vi "main4Ch v2.0.0 reprocessing.vi"() -> ()   [LabVIEW 2024]
doc: "Main VI for FLS imaging system."
uses:
  <userlib>/_OpenG.lib/file/file.llb/openg_file.lvlib
  <vilib>/event_ctls.llb/usereventprio.ctl
  <instrlib>/niScope/Acquire/Fetch/niScope Multi Fetch Binary 16.vi
  <instrlib>/niScope/Controls/niScope trigger source.ctl
  <userlib>/_OpenG.lib/time/time.llb/openg_time.lvlib
  LaguerreDeconLib/DeconEngineClass/LaguerreDeconEngineClass.lvclass
  SubVI/GlobalVariables.vi
  SubVI/LabJack/LJ Pin Setting.ctl
  <vilib>/Utility/error.llb/DialogType.ctl
  <vilib>/Analysis/NI_AALBase.lvlib
  <vilib>/Utility/miscctls.llb/LVMinMaxIncTypeDef.ctl
  <vilib>/Analysis/baseanly.llb/Mean (DBL).vi
  <vilib>/Utility/miscctls.llb/LVPointTypeDef.ctl
  SubVI/APD/APDClass.lvclass
  ConfigFiles/AimingBeamVideoConfig.ctl
  <vilib>/addons/control/pid/NI_PID_pid.lvlib
  <vilib>/addons/control/pid/pid.llb/PID (DBL).vi
  C:/Users/MarcuLab/Documents/GitHub/NetDeconForLV/Source/DotNETAssembly/output/build/LaguerreDeConNative.dll
  MarcuLab/Documents/GitHub/NetDeconForLV/Source/DotNETAssembly/output/build/LaguerreDeConNative.dll
  <vilib>/Instr/_visa.llb/VISA Configure Serial Port (Instr).vi
  <vilib>/Python/Open Anaconda Python Session.vi
  SubVI/DigitizerConfiguration/FLImDAQ.ctl
panel:
  out "error out":errorcluster
  in  "488nm Power":u16(ring)=32 items=["3.30mW"=60, "2.35mW"=50, "2.00mW"=47, "1.75mW"=44, "1.48mW"=41, "1.16mW"=38, "0.87mW"=35, "0.57mW"=32, "0.28mW"=29]
  out "Decon Loop timing (ms)":dbl
  out "Ch3 Lifetime (ns)":dbl caption="Lifetime (ns)"
  out "Ch2 Lifetime (ns)":dbl caption="Lifetime (ns)"
  out "Ch1 Lifetime (ns)":dbl caption="Lifetime (ns)"
  out "Cancer Prob":dbl
  in  "Overlay selection":u16(ring) items=["Gain", "Lifetime", "CancerProbability"]
  out "Record Backlog 2":i32
  in  "Auto gain ch4":bool=TRUE caption="Auto gain ch3"
  in  "V 4":dbl caption="Gain 3" min=0.0 max=4.67 step=0.1
  out "Gain4":dbl
  out "IntR4":dbl format="%#_2g"
  out "SNR4":dbl format="%#_3g"
  out "Channel 4":dbl[][](graph) caption="Channel 3"
  out "RunStartTime":u32
  out "Dig1 Temp":dbl
  out "Dig2 Temp":dbl
  out "Visualization PC video source":T1
  in  "V target(1.0)":dbl=1.0 caption="V target(1.5)" min=0.3 max=1.5 step=0.1 format="%#_4g"
  out "SNR3":dbl format="%#_3g"
  out "SNR2":dbl format="%#_3g"
  out "SNR1":dbl format="%#_3g"
  in  "Show BG removed?":bool=TRUE
  out "IntR3":dbl format="%#_2g"
  out "IntR2":dbl format="%#_2g"
  out "IntR1":dbl format="%#_2g"
  in  "Video Display":bool
  out "Gain3":dbl
  out "Gain2":dbl
  out "Gain1":dbl
  in  "Skip Data Save?":bool
  out "Aq Loop?":bool
  out "ML?":bool
  out "aquisition loop Error Out":errorcluster
  out "Laser f (Hz)":dbl
  out "Record Backlog":i32
  out "Fetch Record #":i32
  out "Sync Success?":bool
  out "Disclamer":picture
  out "Calibration #":i8
  out "BG #":i8
  in  "TCP Connect":bool
  out "Help":string
  in  "355nm Laser toggle":bool caption="355nm 460Hz"
  in  "Cali&iRF alignment":bool
  in  "Background":bool
  in  "Aiming beam toggle":bool caption="488nm 0Hz"
  in  "Auto gain ch3":bool=TRUE
  in  "Auto gain ch2":bool=TRUE
  in  "Auto gain ch1":bool=TRUE
  out "Run #":i8
  in  "StopButton":bool caption="Stop"
  out "Aquisition Status:":bool
  in  "StartButton":bool caption="Start"
  in  "V 3":dbl caption="Gain 3" min=0.0 max=4.65 step=0.1
  in  "V 2":dbl caption="Gain 2" min=0.0 max=4.59 step=0.1
  in  "V 1":dbl caption="Gain 1" min=0.0 max=4.63 step=0.1 format="%#_4g"
  in  "Video Source":enum32{"Camera", "FrameGrabber"}(radio)
  out "Case #":string
  out "System Hardware Connection Status":T2
  out "Channel 3":dbl[][](graph)
  out "Channel 2":dbl[][](graph)
  out "Channel 1":dbl[][](graph)
  in  "Tab Control":T3(tab)
  out "display loop timing(ms)":u32
  out "Aquisition loop timing(ms)":u32 format="%.2f"
  out "DisplayLoop":i32
  out "PID loop":i32 caption="processing loop"
  out "PID loop timing(ms)":u32 caption="processing loop timing(ms)"
  out "Communication loop(ms)":u32
  out "laser EM lamp V":dbl format="%0.6f"
  out "Auisition Loop idx":i32
  out "LJ process (ms)":u32
  out "LJ time(ms)":u32[](array[numeric])
  out "output variable":i32
  out ".NetInitialized?":bool
  out "BG Graph":dbl[][](graph)
  out "Lifetime (ns)":cluster{dbl, dbl, dbl}(graph)
  out "DeCon Speed(ms)":dbl(graph)
  out "iRF Graph":dbl[][](graph)
  in  "Show BG":bool
  out "iRF length":i32
  out "BG length":i32
  out "data length":i32
  out "WarmupTime(ms)":u32
  out "BGAll":dbl[][](array[numeric])
  out "DeConOut":dbl[](array[numeric])
  in  "Ch1GainLim":dbl=350.0 format="%#_13g"
  in  "Ch2&3GainLim":dbl=1750.0 format="%#_13g"
  out "LJ Pinout":T4={"Ch1 Bias"="DAC0", "Ch2 Bias"="DAC1", "Ch3 Bias"="DAC2", "355 PWM"="FIO0", "AimingBeam PWM"="FIO2", "Laser Ready"="FIO3", "Interlock"="FIO1", "Laser Start/Stop"="FIO1", "Red LED"="FIO1", "Green LED"="DIO3", "Foot Pedal"="DIO15"}
  out "FLImDAQ":T5={"Digitizer 1"="", "Digitizer 2"="", "Channel"=enum."Channel 0", "trigger source"="VAL_EXTERNAL", "trigger level"=0.5, "trigger delay"=1.35e-07, "min sample rate"=12500000000.0, "min record length"=2500, "vertical range"=1.0, "vertical offset"=-0.25, "Waveform to Avg"=2000} caption="FLIm DAQ Configuration" {"trigger delay" format="%^#.4e"; "trigger level" min=0.0 max=3.5 step=0.5 format="%.2f"; "vertical offset" format="%.4f"; "vertical range" format="%.2f"; "min sample rate" format="%#.2p"}
  in  "Sys Reconfig":bool
  out "data out(communcation loop)":string
  out "PID loop error out":errorcluster caption="processing Error Out"
  out "decon error out":errorcluster
  out "Laser Rep Rate":dbl
  out "V4 Size":i32 caption="V3 Size"
  in  "Data Class":enum16{"Data", "BG", "Cali"}(ring)=enum."BG"
  out "V1 Size":i32
  out "V2 Size":i32
  out "V3 Size":i32
  out "data Size":i32[](array[numeric])
  out "State log":string
  out "SysConfigCluster":T7
  in  "Ch4 PID gains":T8={"proportional gain (Kc)"=30.0, "integral time (Ti, min)"=0.0003, "derivative time (Td, min)"=1e-05}
  in  "Ch3 PID gains":T8={"proportional gain (Kc)"=30.0, "integral time (Ti, min)"=0.0003, "derivative time (Td, min)"=1e-05}
  in  "Ch2 PID gains":T8={"proportional gain (Kc)"=30.0, "integral time (Ti, min)"=0.0003, "derivative time (Td, min)"=1e-05}
  in  "Ch1 PID gains":T8={"proportional gain (Kc)"=30.0, "integral time (Ti, min)"=0.0003, "derivative time (Td, min)"=1e-05}
  in  "Brain model path":path=path "C:/Users/MarcuLab/Desktop/V6 APD LV/V6 APD LV/ClassifierFile/Brain_Agnostic_Model.pkl"
  in  "module path":path=path "C:/Users/MarcuLab/Documents/GitHub/NetDeconForLV/Classifier/ClassifierModule.py"
  in  "HN model path":path=path "C:/Users/MarcuLab/Desktop/V6 APD LV/V6 APD LV/ClassifierFile/xgb_model.pkl"
  in  "Env name":string="HNClassifier"
  in  "Python version":string="3.10"
  out "Python session":refnum<k35>
  out "OverlaySelection":T9(ring)=enum."HN Classifier"
  in  "CancerThreshold":dbl=0.15
  in  "Quit":bool
  in  "Radio Buttons":T10(radio)=enum."Ch2" caption="DeCon Chan"
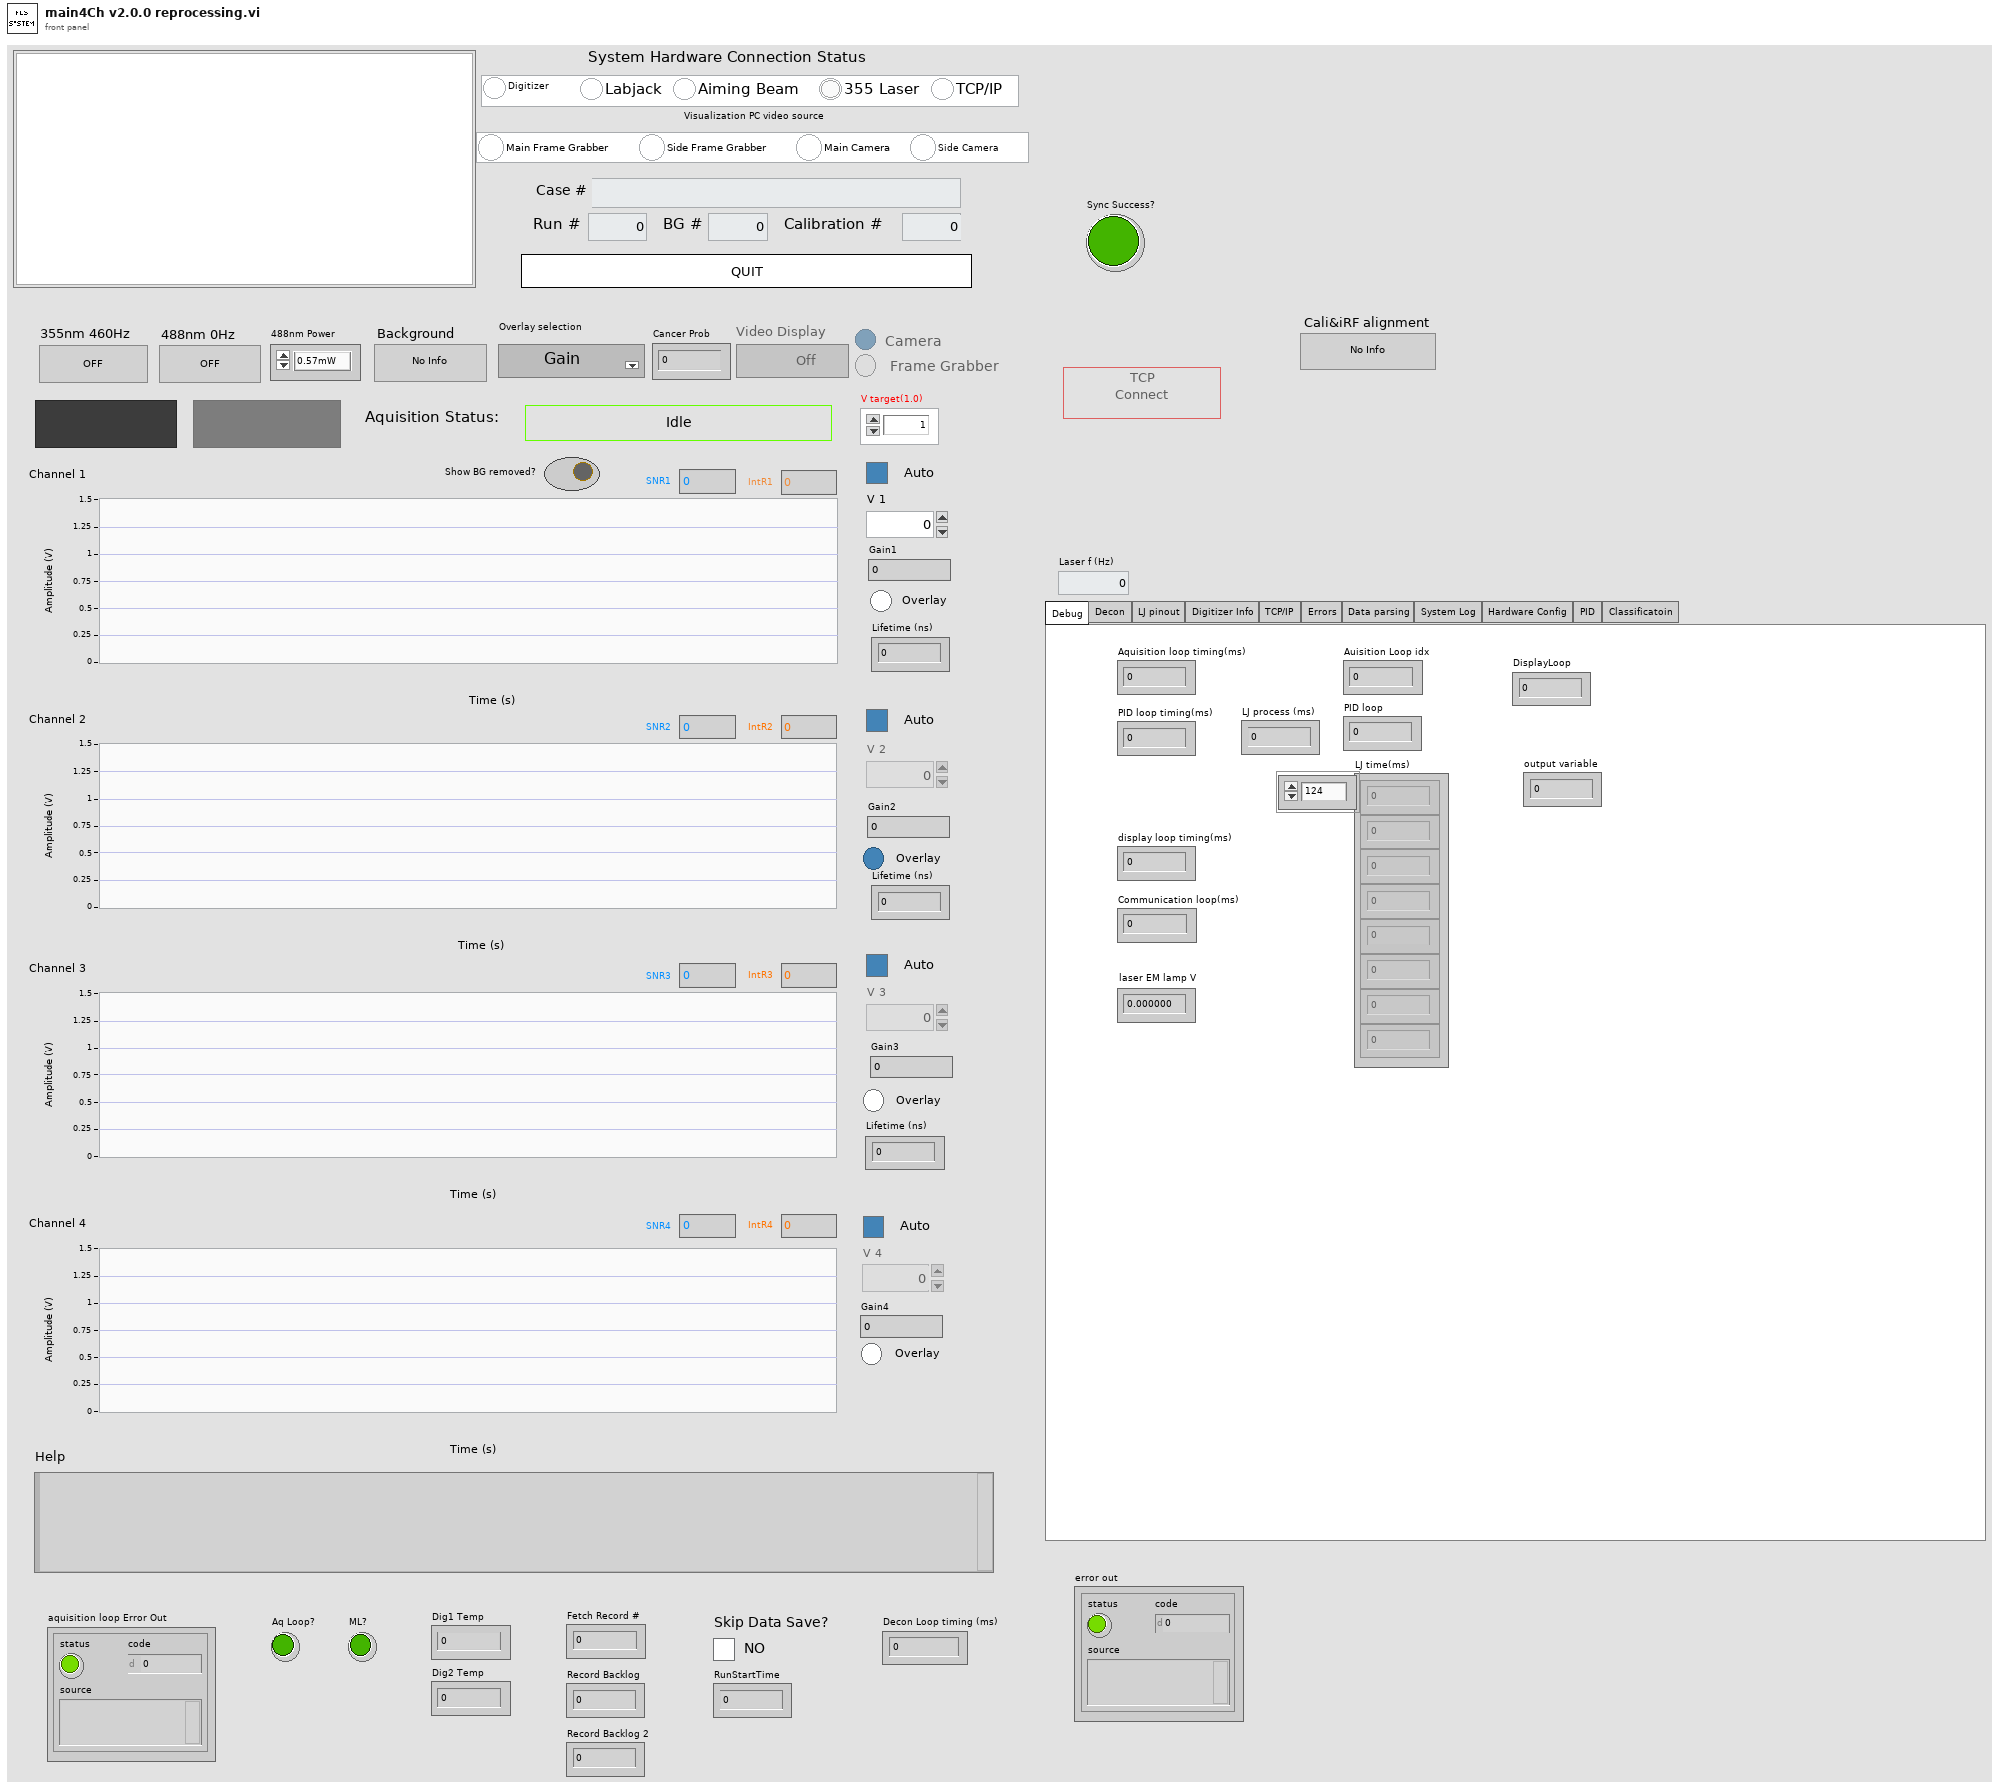
[diagram p1: front panel]
types:
  T1 = cluster{"Main Frame Grabber":bool, "Side Frame Grabber":bool, "Main Camera":bool, "Side Camera":bool}
  T2 = cluster{"Digitizer":bool, "Labjack":bool, "Aiming Beam":bool, "355 Laser":bool, "TCP/IP":bool}
  T3 = enum32{"Debug", "Decon", "LJ pinout", "Digitizer Info", "TCP/IP", "Errors", "Data parsing", "System Log", "Hardware Config", "PID", "Classificatoin"}
  T4 = typedef "LJ Pin Setting.ctl" = cluster{"Ch1 Bias":string, "Ch2 Bias":string, "Ch3 Bias":string, "355 PWM":string, "AimingBeam PWM":string, "Laser Ready":string, "Interlock":string, "Laser Start/Stop":string, "Red LED":string, "Green LED":string, "Foot Pedal":string}
  T5 = typedef "FLImDAQ.ctl" = cluster{"Digitizer 1":refnum<k15>, "Digitizer 2":refnum<k15>, "Channel":enum16{"Channel 0", "Channel 1", "Channel 0&1"}, "trigger source":T6, "trigger level":dbl, "trigger delay":dbl, "min sample rate":dbl, "min record length":i32, "vertical range":dbl, "vertical offset":dbl, "Waveform to Avg":i16}
  T6 = typedef "niScope trigger source.ctl" = string
  T7 = cluster{"Ch1Enable?":bool, "Ch2Enable?":bool, "Ch3Enable?":bool, "Ch1AutoGain?":bool, "Ch2AutoGain?":bool, "Ch3AutoGain?":bool, "AimingBeamEnable?":bool}
  T8 = cluster{"proportional gain (Kc)":dbl, "integral time (Ti, min)":dbl, "derivative time (Td, min)":dbl}
  T9 = enum16{"Gain", "HN Classifier", "Brain Classifier", "Window Close"}
  T10 = enum32{"No Selection", "Ch1", "Ch2", "Ch3", "Ch4"}
  T11 = cluster{"remote start event":refnum<user-event>, "remote stop  event":refnum<user-event>}
  T12 = enum8{"Enabled", "Disabled", "Disabled and Grayed Out"}
  T13 = enum16{"open", "replace", "create", "open or create", "replace or create", "replace or create with confirmation"}
  T14 = cluster{"CH1":dbl[][], "CH2":dbl[][], "CH3":dbl[][], "CH4":dbl[][], "Gain cluster":cluster{"V1":dbl, "V2":dbl, "V3":dbl, "V4":dbl}}
  T15 = cluster{"idx":i32, "CH1&2":dbl[][], "CH3&4":dbl[][], "V cluster":cluster{"V1":dbl, "V2":dbl, "V3":dbl, "V4":dbl}}
  T16 = enum16{"open", "open or create", "create or replace", "create", "open (read-only)"}
  T17 = cluster{"Ch1 iRF":dbl[], "Ch2 iRF":dbl[], "Ch3 iRF":dbl[], "Ch4 iRF":dbl[]}
  T18 = enum32{"Invalid", "Standard", "Closed", "Hidden", "Minimized", "Maximized"}
  T19 = enum32{"invalid app kind", "Development System", "Run Time System", "Student Edition", "Embedded LabVIEW", "Evaluation", "Custom"}
  T20 = typedef "usereventprio.ctl" = enum32{"high priority", "normal priority"}
  T21 = enum32{"Bad", "Idle", "Run top level", "Running"}
  T22 = enum16{"Standard", "Buffered", "CRLF", "Immediate"}
  T23 = typedef "AimingBeamVideoConfig.ctl" = cluster{"DeCon Channel":enum16{"1", "2", "3"}, "Scale Bar":bool, "Scale Low":dbl, "Scale High":dbl, "ANSI":dbl, "Radius":dbl, "3D?":bool, "Firefly?":bool, "Pentero?":bool}
  T24 = cluster{"Core":cluster{"Current VI Reference":refnum<vi>, "Close Panel on Exit?":bool}, "SysConfigCluster":cluster{"Ch1Enable?":bool, "Ch2Enable?":bool, "Ch3Enable?":bool, "Ch1AutoGain?":bool, "Ch2AutoGain?":bool, "Ch3AutoGain?":bool, "AimingBeamEnable?":bool}, "System Status":cluster{"Digitizer":bool, "Labjack":bool, "Aiming Beam":bool, "355 Laser":bool, "TCP/IP":bool}, "IDs":cluster{"RunID":i8, "BG ID":i8, "Cali ID":i8}, "CaseID":string, "DefaultPath":path, "Pathes":cluster{"DataPath":path, "BG Path":path, "iRFPath":path, "CaliPath":path}, "FLImDAQ":cluster{"resource name":refnum<k15>, "resource name 2":refnum<k15>, "Channel":enum16{"Channel 0", "Channel 1", "Channel 0&1"}, "trigger source":T6, "trigger level":dbl, "trigger delay":dbl, "min sample rate":dbl, "min record length":i32, "vertical range":dbl, "vertical offset":dbl, "Waveform to Avg":i32}, "SysRunning?":bool, "AB Cluster":cluster{"Aiming Beam COM Port":refnum<visa-resource-name>, "Min Current":dbl, "Max Current":dbl, "Default Current":dbl, "Freq":i32}, "LJ Pinout":T4, "355 PWM setting":cluster{"DIO_EF_CLOCK1_DIVISOR":i16, "DIO_EF_CLOCK1_ROLL_VALUE":i32, "DIO#_EF_INDEX":i16, "DIO#_EF_OPTIONS":i16, "DIO#_EF_CONFIG_A":i32}, "AB PWM setting":cluster{"DIO_EF_CLOCK1_DIVISOR":i16, "DIO_EF_CLOCK1_ROLL_VALUE":i32, "DIO#_EF_INDEX":i16, "DIO#_EF_OPTIONS":i16, "DIO#_EF_CONFIG_A":i32}, "Last Trigger":u32, "niTClk sessions":refnum<k20>[], "Laser start tic":u32, "TCP attempt count":i32, "Ch1Data":dbl[][], "Ch2Data":dbl[][], "Ch3Data":dbl[][], "Ch4Data":dbl[][], "V1":dbl[], "V2":dbl[], "V3":dbl[], "V4":dbl[], "SlowTimer":u32, "FastTimer":u32, "listener ID":refnum<k5>, "TempPath":path, "CaliPath":path, "LED vi reference":refnum<vi>, "Aquisition Timer":u32, "APDSerialNum":cluster{"Ch1APDSerial#":string, "Ch2APDSerial#":string, "Ch3APDSerial#":string, "Ch4APDSerial#":string}, "VideoConfig":T23, "LED vi ref open?":bool, "video source":cluster{"Main Frame Grabber":bool, "Side Frame Grabber":bool, "Main Camera":bool, "Side Camera":bool}, "bothVidSourceAvail":bool, "OverlaySelection":u16}
  T25 = typedef "LVCursorListTypeDef.ctl" = cluster{"Name":string, "Color":u32, "Style":u8, "Point Style":u8, "Name Visible":bool, "Allow Drag":bool, "Cursor Mode":u32, "Plot":i32, "Index":i32, "Position":cluster{"X":dbl, "Y":dbl}, "X Scale":u32, "Y Scale":u32, "Watch Plots":i32[], "Watch All Plots":bool, "Plot Area":i32, "Label Offset":cluster{"X":dbl, "Y":dbl}}[]
  T26 = cluster{"Name":string, "Color":u32, "Style":u8, "Point Style":u8, "Name Visible":bool, "Allow Drag":bool, "Cursor Mode":u32, "Plot":i32, "Index":i32, "Position":cluster{"X":dbl, "Y":dbl}, "X Scale":u32, "Y Scale":u32, "Watch Plots":i32[], "Watch All Plots":bool, "Plot Area":i32, "Label Offset":cluster{"X":dbl, "Y":dbl}}
  T27 = cluster{"Ch1APDSerial#":string, "Ch2APDSerial#":string, "Ch3APDSerial#":string, "Ch4APDSerial#":string}
  T28 = cluster{"DataPath":path, "BG Path":path, "iRFPath":path, "CaliPath":path}
  T29 = cluster{"DIO_EF_CLOCK1_DIVISOR":i16, "DIO_EF_CLOCK1_ROLL_VALUE":i32, "DIO#_EF_INDEX":i16, "DIO#_EF_OPTIONS":i16, "DIO#_EF_CONFIG_A":i32}
  T30 = cluster{"Aiming Beam COM Port":refnum<visa-resource-name>, "Min Current":dbl, "Max Current":dbl, "Default Current":dbl, "Freq":i32}
  T31 = cluster{"resource name":refnum<k15>, "resource name 2":refnum<k15>, "Channel":enum16{"Channel 0", "Channel 1", "Channel 0&1"}, "trigger source":T6, "trigger level":dbl, "trigger delay":dbl, "min sample rate":dbl, "min record length":i32, "vertical range":dbl, "vertical offset":dbl, "Waveform to Avg":i32}
  T32 = cluster{"Current VI Reference":refnum<vi>, "Close Panel on Exit?":bool}
  T33 = cluster{"Channel 1":dbl[], "Channel 2":dbl[], "Channel 3":dbl[]}
  T34 = cluster{"Ch1 WF":dbl[], "Ch2 WF":dbl[], "Ch3 WF":dbl[], "Ch4 WF":dbl[], "V1":dbl, "V2":dbl, "V3":dbl, "V4":dbl}
  T35 = typedef "iRFData.ctl" = cluster{"dt":dbl, "NumOfWFs":i32, "WFLength":i32, "iRFCtrlV":dbl[], "iRFWFsAvg":dbl[][], "iRFRaw":dbl[][]}
  T36 = cluster{"Ch1 iRF":dbl[], "Ch2 iRF":dbl[], "Ch3 iRF":dbl[]}
  T37 = cluster{"mean":dbl, "mean":dbl, "mean":dbl, "mean":dbl}
  T38 = cluster{"V1":dbl, "V2":dbl, "V3":dbl, "V4":dbl}[]
  T39 = cluster{"DataPath":path, "CaseID":string, "RunID":i16, "Ch1Data":dbl[][], "Ch2Data":dbl[][], "Ch3Data":dbl[][], "Ch4Data":dbl[][], "V1":dbl[], "V2":dbl[], "V3":dbl[], "V4":dbl[], "LaserRepRate":u16, "WFAverage":i16, "RunStartTime":u64}
  T40 = typedef "DialogType.ctl" = u16
  T41 = typedef "APD.ctl" = cluster{"gainV":dbl[], "gain":dbl[], "irfV":dbl[], "irfTNorm":dbl[][]}
  T42 = cluster{"Ch1APDSerial#":string, "Ch2APDSerial#":string, "Ch3APDSerial#":string}
  T43 = typedef "LJ PWM Setting.ctl" = cluster{"DIO_EF_CLOCK1_DIVISOR":i16, "DIO_EF_CLOCK1_ROLL_VALUE":i32, "DIO#_EF_INDEX":i16, "DIO#_EF_OPTIONS":i16, "DIO#_EF_CONFIG_A":i32}
  T44 = typedef "AimingBeam.ctl" = cluster{"Aiming Beam COM Port":refnum<visa-resource-name>, "Min Current":dbl, "Max Current":dbl, "Default Current":dbl, "Frequency(Hz)":u32}
  T45 = cluster{"DC1":i32, "DC2":i32, "BG1":i32, "BG2":i32}
  T46 = typedef "LVMinMaxIncTypeDef.ctl" = cluster{"Minimum":dbl, "Maximum":dbl, "Increment":dbl}
  T47 = typedef "LVBoundsTypeDef.ctl" = cluster{"Width":u32, "Height":u32}
  T48 = typedef "imagedata.ctl" = cluster{"image type":i32, "image depth":i32, "image":u8[], "mask":u8[], "colors":u32[], "Rectangle":cluster{"left":i16, "top":i16, "right":i16, "bottom":i16}}
  T49 = enum16{"Left Button", "Center Button", "Right Button", "Window Close"}
  T50 = cluster{"DC Idx1":i32, "DC Idx2":i32, "BG Idx1":i32, "BG Idx2":i32}
  T51 = cluster{dbl[][], dbl[][], dbl[][], dbl[][], "V cluster":cluster{"V1":dbl, "V2":dbl, "V3":dbl, "V4":dbl}}
  T52 = cluster{"actualSamples":i32, "absoluteInitialX":dbl, "relativeInitialX":dbl, "xIncrement":dbl, "offset":dbl, "gain":dbl, "reserved1":dbl, "reserved2":dbl}[]
  T53 = cluster{"V1 out":dbl, "V2 out":dbl, "V3 out":dbl, "V3 out":dbl}
  T54 = cluster{i32, dbl[][], dbl[][], cluster{"V1 out":dbl, "V2 out":dbl, "V3 out":dbl, "V3 out":dbl}}
  T55 = typedef "LVPointTypeDef.ctl" = cluster{"Horizontal":i16, "Vertical":i16}
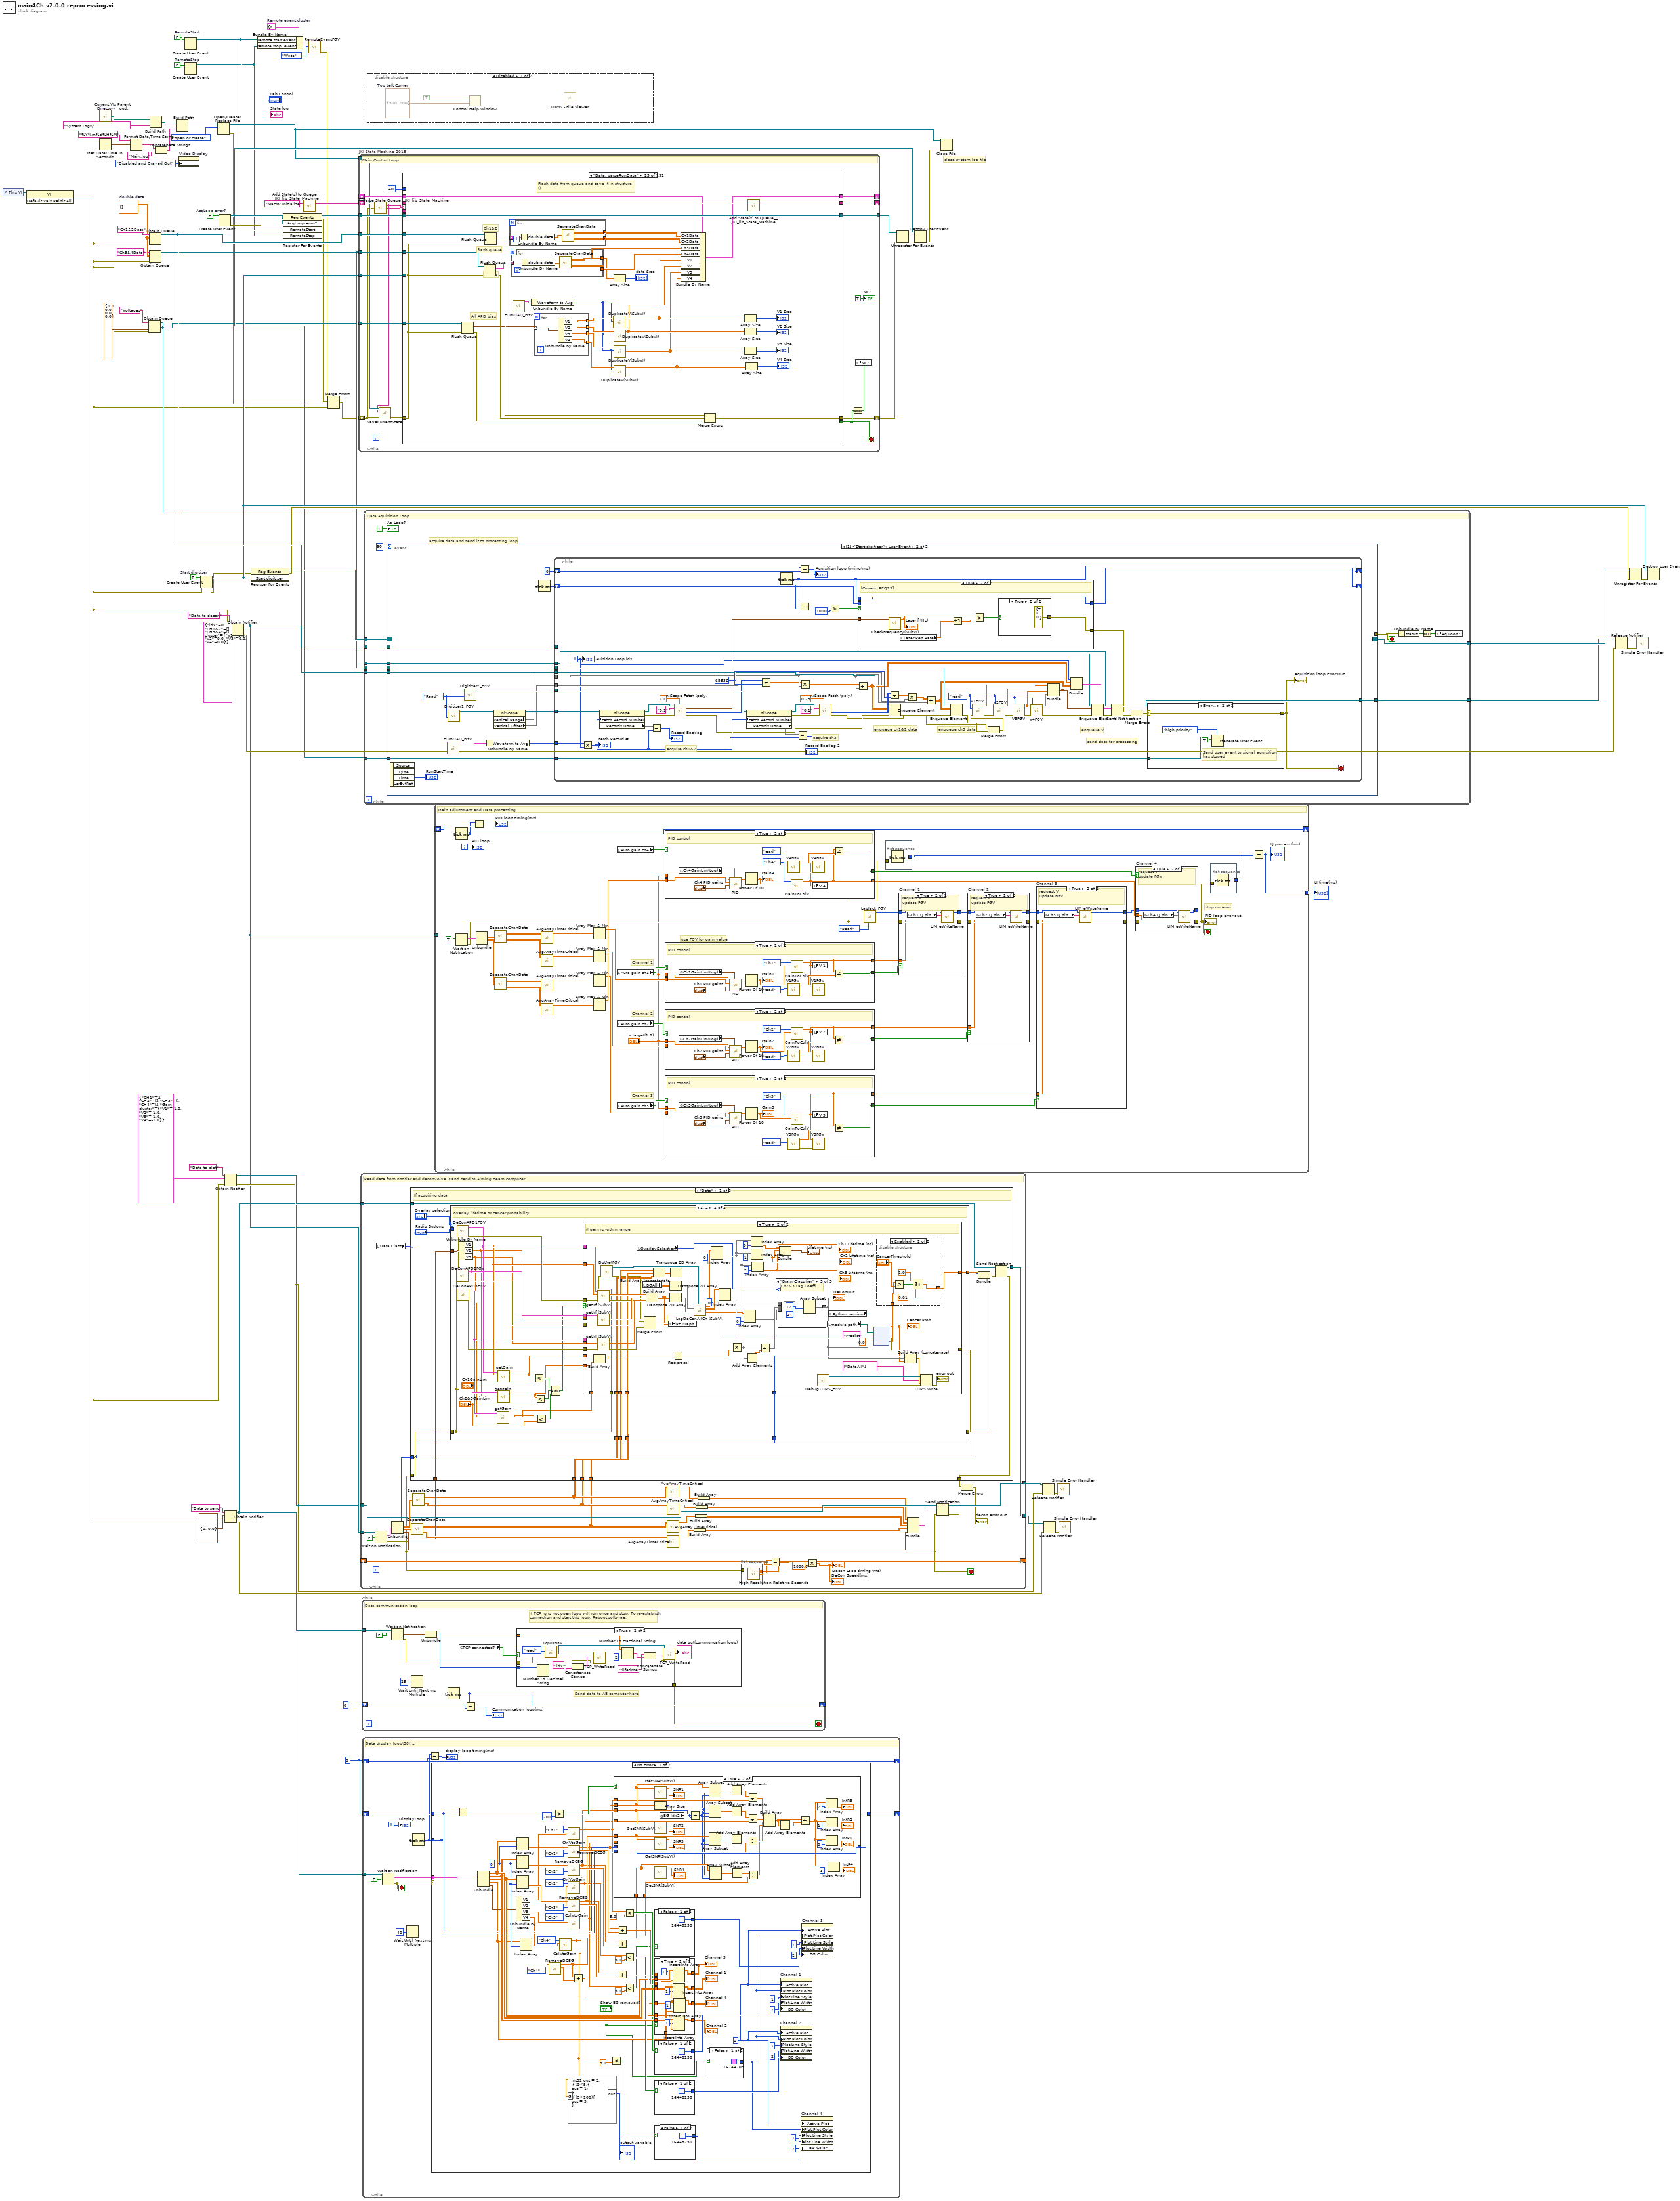
[diagram p0: block diagram]
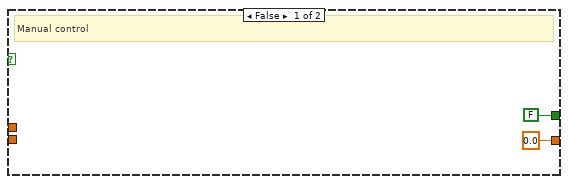
[diagram p6: hidden frame]
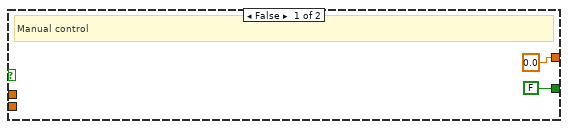
[diagram p7: hidden frame]
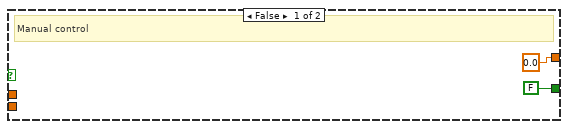
[diagram p8: hidden frame]
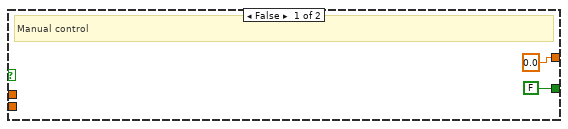
[diagram p9: hidden frame]
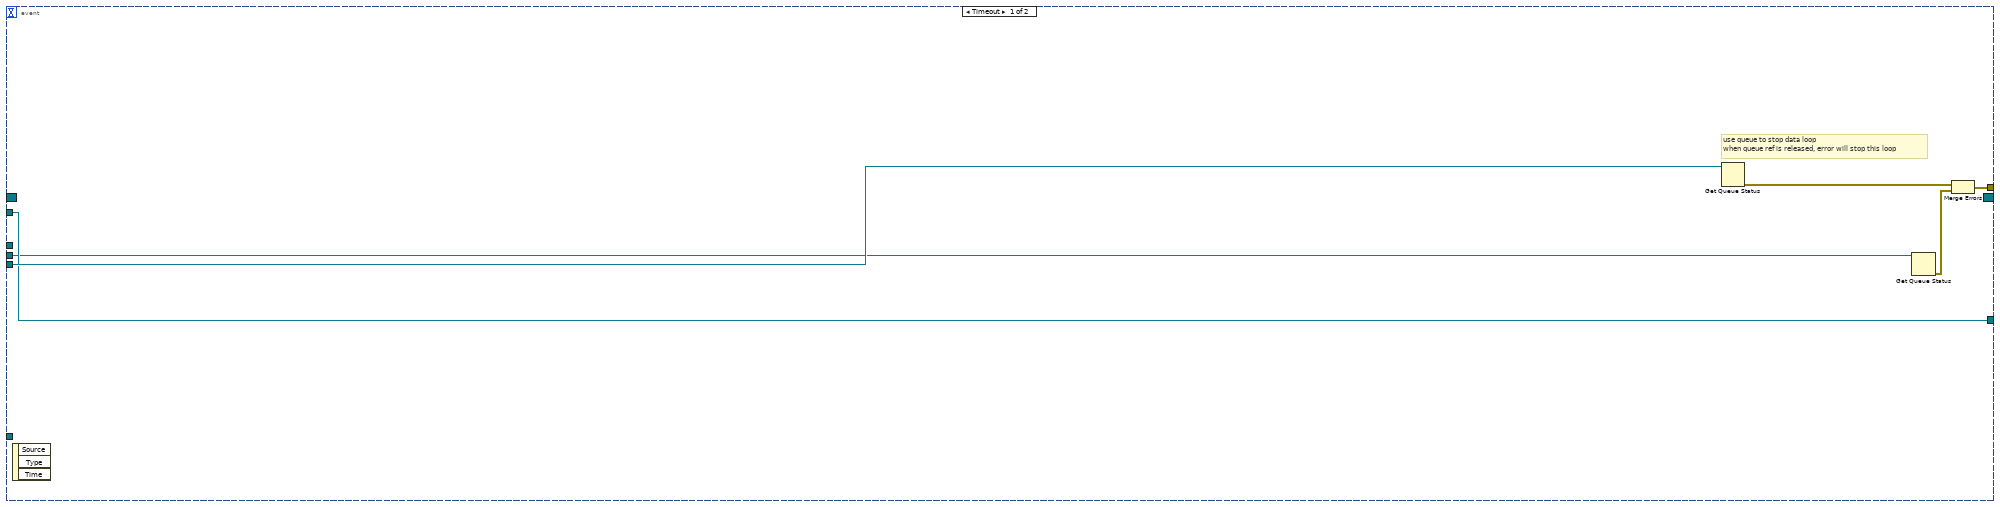
[diagram p10: hidden frame]
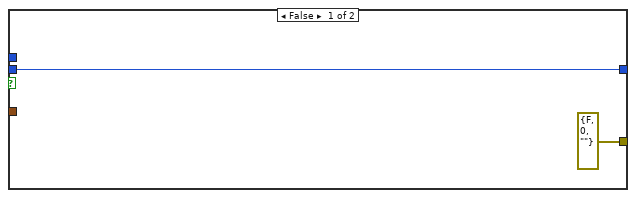
[diagram p11: hidden frame]
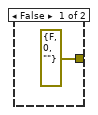
[diagram p12: hidden frame]
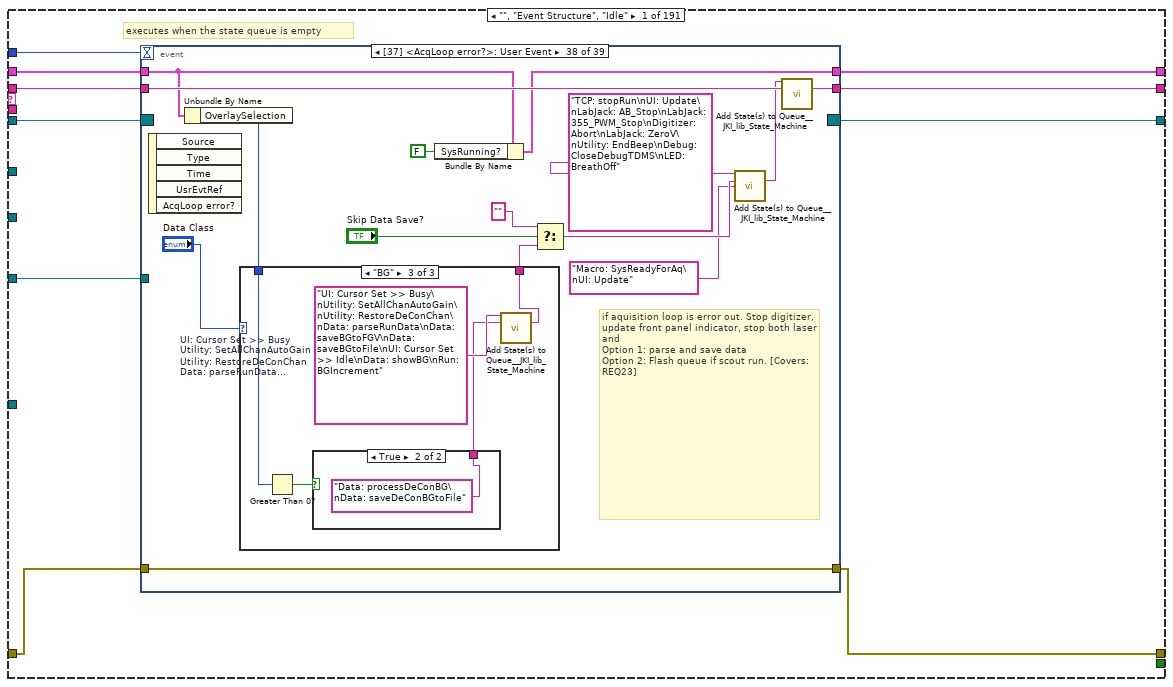
[diagram p14: hidden frame]
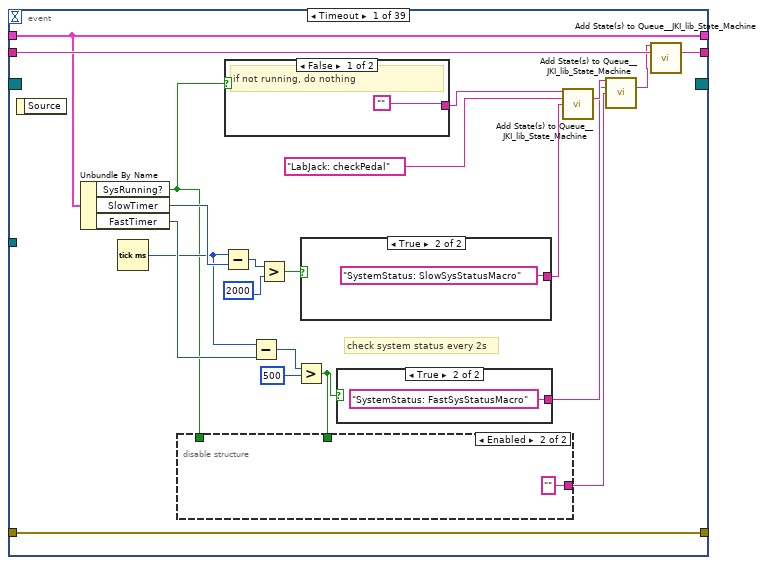
[diagram p15: hidden frame]
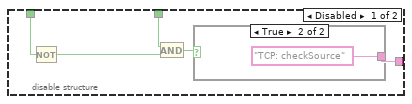
[diagram p16: hidden frame]
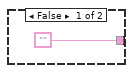
[diagram p17: hidden frame]
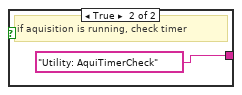
[diagram p18: hidden frame]
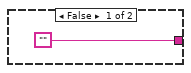
[diagram p19: hidden frame]
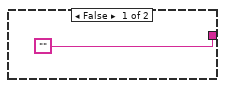
[diagram p20: hidden frame]
diagram:
  w8 = T11 {"remote start event"=refnum, "remote stop  event"=refnum}  # Remote event cluster
  w11 = FALSE  # RemoteStop
  w12 = FALSE  # RemoteStart
  w15 = u32 0 ("millisecond timer value")
  w54 = FALSE  # AcqLoop error?
  w64 = TRUE  # Start digitizer
  w67 = dbl[][] []  # double data
  # "close system log file"
  n1 = control-ref of="This VI"() -> (w69:refnum<vi>)
  n2 = invoke on="Invoke Node" class="VI" method="Default Vals.Reinit All"(reference=w69) -> (error out=w23:errorcluster)  [unwired: 2 in, 2 out]
  n3 = call <userlib>:"Current VIs Parent Directory__ogtk.vi"() -> ("Parent Directory (+ Relative)"=w34:path)  [unwired: 5 in]
  n4 = Get Date/Time In Seconds() -> (seconds since 1Jan1904=w32:timestamp)
  n5 = Format Date/Time String(time format string (%c)="%Y%m%d%H%M", seconds (now)=w32) -> (date/time string=w29:string)  [unwired: 1 in]
  n6 = Obtain Queue(name (unnamed)="Voltages", element data type=cluster{"V1":dbl, "V2":dbl, "V3":dbl, "V4":dbl} {"V1"=0.0, "V2"=0.0, "V3"=0.0, "V4"=0.0}, error in (no error)=w23) -> (queue out=w35:refnum<queue>)  [unwired: 2 in, 2 out]
  n7 = Obtain Queue(name (unnamed)="Ch3&4Data", element data type=w67, error in (no error)=w23) -> (queue out=w48:refnum<queue>)  [unwired: 2 in, 2 out]
  n8 = Obtain Queue(name (unnamed)="Ch1&2Data", element data type=w67, error in (no error)=w23) -> (queue out=w65:refnum<queue>)  [unwired: 2 in, 2 out]
  n9 = Build Path(base path=w34, name or relative path="System Log\\") -> (appended path=w25:path)
  n10 = Concatenate Strings(w29, "Main.log" ("string")) -> (w27:string)
  n11 = Build Path(base path=w25, name or relative path=w27) -> (appended path=w30:path)
  n12 = property on="Video Display" class="Bool (strict)"("DisabledEnum"=T12."Disabled and Grayed Out" ("Disabled")) -> ()  [unwired: 2 in, 2 out]
  n13 = Create User Event(user event datatype=w12) -> (user event=w10:refnum<user-event>)  [unwired: 1 in, 1 out]
  n14 = Create User Event(user event datatype=w11) -> (user event=w9:refnum<user-event>)  [unwired: 1 in, 1 out]
  n15 = Create User Event(user event datatype=w64, error in=w23) -> (user event=w53:refnum<user-event>, error out=w40:errorcluster)
  n16 = Open/Create/Replace File(file path (use dialog)=w30, operation (0:open)=T13."open or create") -> (refnum out=w21:refnum<file>, error out=w22:errorcluster)  [unwired: 4 in, 1 out]
  n17 = Create User Event(user event datatype=w54) -> (user event=w39:refnum<user-event>, error out=w41:errorcluster)  [unwired: 1 in]
  n18 = Obtain Notifier(name (unnamed)="Data to plot", notification data type=T14 {"CH1"=[], "CH2"=[], "CH3"=[], "CH4"=[], "Gain cluster"={"V1"=-1.0, "V2"=-1.0, "V3"=-1.0, "V4"=-1.0}}, error in (no error)=w23) -> (notifier out=w13:refnum<notifier>, error out=w49:errorcluster)  [unwired: 1 in, 1 out]
  n19 = Obtain Notifier(name (unnamed)="Data to send", notification data type=cluster{"idx":i32, "lifetime":dbl} {"idx"=0, "lifetime"=0.0}, error in (no error)=w23) -> (notifier out=w18:refnum<notifier>, error out=w38:errorcluster)  [unwired: 1 in, 1 out]
  n20 = Obtain Notifier(name (unnamed)="Data to decon", notification data type=T15 {"idx"=0, "CH1&2"=[], "CH3&4"=[], "V cluster"={"V1"=0.0, "V2"=0.0, "V3"=0.0, "V4"=0.0}}, error in (no error)=w23) -> (notifier out=w19:refnum<notifier>, error out=w58:errorcluster)  [unwired: 1 in, 1 out]
  n21 = register-events(error in=w40, w53) -> (reference out=w55:refnum<event-registration>, error out=w61:errorcluster)  [unwired: 1 in]
  n22 = Bundle By Name(cluster=w8, "remote start event"=w10, "remote stop  event"=w9) -> (w6:T11)
  n23 = register-events(error in=w41, w39, w10, w9) -> (reference out=w47:refnum<event-registration>, error out=w5:errorcluster)  [unwired: 1 in]
  n24 = call <vilib>:"Add State(s) to Queue__JKI_lib_State_Machine.vi"("State(s) in (\"\")"="Macro: Initialize") -> ("States Out"=w71:string)  [unwired: 14 in]
  n25 = call "RemoteEventFGV.vi"("Operation (Read)"=enum16{"Read", "Write"}."Write", "Remote Event in"=w6) -> ("Error Out"=w2:errorcluster)  [unwired: 8 in, 1 out]
  n26 = Merge Errors(w2, w5, w22, w23) -> (w24:errorcluster)
  n27 = while "JKI State Machine 2018" {
    shift-right: [w88] -> _
    shift-left: _ -> [w87]
    shift-right: [w72] -> w4
    shift-left: w24 -> [w74]
    shift-right: [w89] -> _
    shift-left: w71 -> [w90]
    tunnel: w65 -> [w85]
    tunnel: w48 -> [w84]
    tunnel: w53 -> [w83]
    tunnel: w47 -> [w82]
    tunnel: [w81] -> w46
    tunnel: w35 -> [w77]
    tunnel: w21 -> [w76]
    stop <- w80 stop-if-true
    # "Main Control Loop"
    n28 = call <vilib>:"Parse State Queue__JKI_lib_State_Machine.vi"("State Queue"=w90, "Error In (no error)"=w74) -> ("Remaining States"=w92:string, "Current State"=w75:string, "Arguments"=w91:string)  [unwired: 11 in]
    n29 = call "SaveCurrentState.vi"("error in (no error)"=w74, "Current State"=w75, "Byte Stream File in"=w76) -> ("error out"=w73:errorcluster)  [unwired: 8 in]
    n30 = case shown="\"Data: parseRunData\"" w75 {
      selector: w75 -> [_ _ _ _ _ _ _ _ _ _ _ _ _ _ _ _ _ _ _ _ _ _ _ _ _ _ _ _ w1162 _ _ _ _ _ _ _ _ _ _ _ _ _ _ _ _ _ _ _ _ _ _ _ _ _ _ _ _ _ _ _ _ _ _ _ _ _ _ _ _ _ _ _ _ _ _ _ _ _ _ _ _ _ _ _ _ _ _ _ _ _ _ _ _ _ _ _ _ _ _ _ _ _ _ _ _ _ _ _ _ _ _ _ _ _ _ _ _ _ _ _ _ _ _ _ _ _ _ _ _ _ _ _ _ _ _ _ _ _ _ _ _ _ _ _ _ _ _ _ _ _ _ _ _ _ _ _ _ _ _ _ _ _ _ _ _ _ _ _ _ _ _ _ _ _ _ _ _ _ _ _ _ _ _ _ _ _ _ _ _ _ _]
      tunnel: w92 -> [w102 w522 w531 w537 w544 w552 w577 w592 w635 w641 w668 w693 w705 w776 w791 w822 w849 w881 w900 w929 w959 w976 w981 w1066 w1103 w1142 w1155 w1160 w1166 w1194 w1202 w1225 w1230 w1243 w1262 w1290 w1318 w1356 w1361 w1370 w1382 w1412 w1420 w1426 w1450 w1474 w1498 w1522 w1527 w1544 w1591 w1613 w1629 w1644 w1664 w1669 w1681 w1710 w1736 w1748 w1786 w1799 w1805 w1816 w1828 w1859 w1872 w1886 w1901 w1920 w1955 w1960 w1974 w1984 w2000 w2012 w2024 w2052 w2067 w2072 w2084 w2096 w2101 w2109 w2117 w2126 w2135 w2140 w2148 w2157 w2175 w2192 w2212 w2223 w2241 w2256 w2273 w2278 w2286 w2294 w2299 w2307 w2314 w2322 w2329 w2339 w2367 w2375 w2382 w2390 w2395 w2403 w2410 w2416 w2425 w2441 w2446 w2453 w2471 w2482 w2552 w2564 w2573 w2587 w2596 w2613 w2636 w2653 w2664 w2677 w2702 w2725 w2731 w2747 w2769 w2777 w2783 w2788 w2795 w2805 w2817 w2826 w2831 w2843 w2848 w2858 w2864 w2870 w2875 w2880 w2885 w2895 w2919 w2940 w2945 w2956 w2981 w3008 w3031 w3036 w3051 w3102 w3148 w3193 w3204 w3222 w3242 w3256 w3269 w3277 w3294 w3316 w3340 w3359 w3377 w3395 w3413 w3427 w3441 w3460 w3474 w3489 w3504 w3513 w3518 w3535 w3545 w3552 w3571 w3579 w3584]
      tunnel: w91 -> [_ _ _ _ _ _ _ _ _ _ _ _ _ _ _ _ _ _ _ _ _ _ _ _ _ _ _ _ _ _ _ _ _ _ _ _ _ _ _ _ _ _ _ _ _ _ _ _ _ _ _ _ _ _ _ _ _ _ _ _ _ _ _ _ w1826 _ _ _ _ _ _ _ _ _ _ _ _ _ _ _ _ _ _ _ _ _ _ _ _ _ _ _ _ _ _ _ _ _ _ _ _ _ _ _ _ w2330 _ _ _ _ _ _ _ _ _ _ _ w2448 _ w2476 _ _ _ _ w2593 w2610 _ _ _ _ _ w2721 _ _ _ _ _ _ w2790 _ _ _ _ _ _ w2854 _ _ _ _ _ _ _ _ _ _ _ _ _ _ _ _ _ _ _ _ _ _ _ _ _ _ _ _ _ _ _ _ _ _ _ _ _ _ _ _ _ _ _ _ _]
      tunnel: w87 -> [w100 w519 w527 w534 w539 w549 w574 w589 _ w637 w664 w690 w701 w773 w782 w819 w841 w872 w897 w926 w956 w973 w978 w1027 w1095 w1130 w1150 w1157 w1164 w1187 w1199 w1223 w1227 w1231 w1252 w1282 w1310 w1352 w1358 w1368 w1380 w1410 w1418 w1423 w1431 w1455 w1480 w1504 w1524 w1537 w1581 w1610 w1614 w1641 w1661 w1666 w1670 w1699 w1726 w1741 w1769 w1797 w1802 w1809 w1824 w1842 w1867 w1878 w1896 w1913 w1938 w1957 w1970 w1978 w1997 w2009 w2021 w2040 w2056 w2069 w2082 w2094 w2098 w2103 w2110 w2122 w2131 w2137 w2144 w2154 w2162 w2179 w2207 w2213 w2238 w2249 w2271 w2275 w2279 w2287 w2296 w2305 w2311 w2319 w2326 w2336 w2364 w2372 w2379 w2387 w2392 w2397 w2408 w2413 w2419 w2438 w2443 w2451 w2462 w2478 w2549 w2554 w2567 w2585 w2594 w2611 w2626 w2650 w2661 w2671 w2695 w2722 w2728 w2740 w2765 w2774 w2780 w2785 w2792 w2799 w2813 w2823 w2828 w2840 w2845 w2851 w2861 w2867 w2872 w2877 w2882 w2892 w2917 w2938 w2942 w2954 w2979 w3006 w3029 w3033 w3044 w3096 w3144 w3190 w3200 w3217 w3237 w3251 w3265 w3271 w3289 w3311 w3335 w3354 w3372 w3390 w3408 w3422 w3436 w3455 w3469 w3484 w3501 w3511 w3515 w3520 w3543 w3549 w3568 w3577 w3581]
      tunnel: [w93 w520 w529 w535 w542 w550 w575 w590 w633 w639 w660 w678 w697 w750 w778 w820 w829 w861 w891 w917 w949 w960 w979 w1003 w1092 w1129 w1151 w1158 w1168 w1191 errorcluster {"status"=FALSE, "code"=0, "source"=""} ("error out") w1222 w1228 w1241 w1260 w1274 w1297 w1354 w1359 w1362 w1375 w1385 w1414 w1424 w1432 w1456 w1481 w1505 w1525 w1528 w1573 w1604 w1618 w1642 w1652 w1667 w1673 w1697 w1725 w1740 w1756 w1791 w1803 w1814 w1818 w1833 w1862 w1874 w1892 w1912 w1929 w1958 w1962 w1980 w1995 w2007 w2019 w2042 w2057 w2070 w2074 w2091 w2099 w2107 w2115 w2119 w2128 w2138 w2141 w2150 w2165 w2187 w2206 w2217 w2231 w2253 w2269 w2276 w2284 w2292 w2297 w2304 w2312 w2320 w2327 w2337 w2365 w2373 w2380 w2388 w2393 w2401 w2407 w2414 w2422 w2439 w2444 w2449 w2470 w2479 w2550 w2558 w2570 w2577 w2590 w2607 w2627 w2651 w2660 w2673 w2697 w2723 w2729 w2737 w2759 w2775 w2781 w2786 w2793 w2803 w2815 w2824 w2829 w2841 w2846 w2856 w2862 w2868 w2873 w2878 w2883 w2893 w2907 w2931 w2943 w2947 w2966 w2998 w3023 w3034 w3038 w3097 w3145 w3191 w3199 w3219 w3239 w3253 w3267 w3273 w3291 w3313 w3337 w3356 w3374 w3392 w3410 w3424 w3438 w3457 w3471 w3485 w3502 w3509 w3516 w3524 w3538 w3550 w3553 w3573 w3582] -> w72
      tunnel: w73 -> [w99 w520 w529 w535 w542 w550 w575 w590 w633 w639 w661 w685 w695 w750 w777 w820 w830 w868 w882 w907 w950 w968 w979 w1003 w1093 w1132 w1152 w1158 w1167 w1191 w1195 w1222 w1228 w1241 w1260 w1273 w1309 w1354 w1359 w1363 w1376 w1390 w1413 w1424 w1436 w1460 w1485 w1509 w1525 w1535 w1576 w1603 w1617 w1642 w1654 w1667 w1672 w1698 w1716 w1746 w1767 w1790 w1803 w1811 w1821 w1832 w1861 w1877 w1891 w1911 w1928 w1958 w1968 w1981 w1994 w2006 w2018 w2041 w2058 w2070 w2073 w2086 w2099 w2107 w2115 w2118 w2127 w2138 w2142 w2151 w2170 w2186 w2205 w2216 w2237 w2252 w2268 w2276 w2284 w2292 w2297 w2304 w2312 w2320 w2327 w2337 w2365 w2373 w2380 w2388 w2393 w2401 w2407 w2414 w2422 w2439 w2444 w2450 w2470 w2480 w2550 w2559 w2569 w2576 w2589 w2606 w2628 w2651 w2660 w2668 w2700 w2723 w2729 w2742 w2758 w2775 w2781 w2786 w2793 w2803 w2815 w2824 w2829 w2841 w2846 w2856 w2862 w2868 w2873 w2878 w2883 w2893 w2906 w2930 w2943 w2946 w2965 w2988 w3014 w3034 _ w3098 w3145 w3191 w3198 w3218 w3238 w3252 w3267 w3272 w3290 w3312 w3336 w3355 w3373 w3391 w3409 w3423 w3437 w3456 w3470 w3483 w3502 w3508 w3516 w3529 w3540 w3550 w3557 w3572 w3582]
      tunnel: [w101 w521 w530 w536 w543 w551 w576 w591 w634 w640 w667 w692 w704 w775 w790 w821 w848 w880 w899 w928 w958 w975 w980 w1065 w1102 w1141 w1154 w1159 w1165 w1193 w1201 w1224 w1229 w1242 w1261 w1289 w1317 w1355 w1360 w1369 w1381 w1411 w1419 w1425 w1449 w1473 w1497 w1521 w1526 w1543 w1590 w1612 w1628 w1643 w1663 w1668 w1680 w1709 w1735 w1747 w1785 w1798 w1804 w1815 w1827 w1858 w1871 w1885 w1900 w1919 w1954 w1959 w1973 w1983 w1999 w2011 w2023 w2051 w2066 w2071 w2083 w2095 w2100 w2108 w2116 w2125 w2134 w2139 w2147 w2156 w2174 w2191 w2211 w2222 w2240 w2255 w2272 w2277 w2285 w2293 w2298 w2306 w2313 w2321 w2328 w2338 w2366 w2374 w2381 w2389 w2394 w2402 w2409 w2415 w2424 w2440 w2445 w2452 w2471 w2481 w2551 w2563 w2572 w2586 w2595 w2612 w2635 w2652 w2663 w2676 w2701 w2724 w2730 w2746 w2768 w2776 w2782 w2787 w2794 w2804 w2816 w2825 w2830 w2842 w2847 w2857 w2863 w2869 w2874 w2879 w2884 w2894 w2918 w2939 w2944 w2955 w2980 w3007 w3030 w3035 w3050 w3101 w3147 w3192 w3203 w3221 w3241 w3255 w3268 w3276 w3293 w3315 w3339 w3358 w3376 w3394 w3412 w3426 w3440 w3459 w3473 w3488 w3503 w3512 w3517 w3534 w3544 w3551 w3570 w3578 w3583] -> w89
      tunnel: [_ _ _ _ _ _ _ _ _ _ _ _ _ _ _ _ _ _ _ _ _ _ _ _ _ _ _ _ _ _ _ TRUE _ _ _ _ _ _ _ _ _ _ _ _ _ _ _ _ _ _ _ _ _ _ _ _ _ _ _ _ _ _ _ _ _ _ _ _ _ _ _ _ _ _ _ _ _ _ _ _ _ _ _ _ _ _ _ _ _ _ _ _ _ _ _ _ _ _ _ _ _ _ _ _ _ _ _ _ _ _ _ _ _ _ _ _ _ _ _ _ _ _ _ _ _ _ _ _ _ _ _ _ _ _ _ _ _ _ _ _ _ _ _ _ _ _ _ _ _ _ _ _ _ _ _ _ _ _ _ _ _ _ _ _ _ _ _ _ _ _ _ _ _ _ _ _ _ _ _ _ _ _ _ _ _ _ _ _ _ _ _] -> w80
      tunnel: [w98 w519 w527 w534 w539 w549 w574 w589 w608 w637 w664 w690 w701 w773 w782 w819 w841 w872 w897 w926 w956 w973 w978 w1027 w1096 w1131 w1150 w1157 w1164 w1192 w1199 w1223 w1227 w1232 w1253 w1283 w1311 w1353 w1358 w1368 w1380 w1410 w1418 w1423 w1431 w1455 w1480 w1504 w1524 w1537 w1582 w1610 w1615 w1641 w1662 w1666 w1671 w1699 w1726 w1745 w1769 w1797 w1802 w1812 w1824 w1842 w1867 w1878 w1896 w1913 w1938 w1957 w1971 w1978 w1997 w2009 w2021 w2040 w2056 w2069 w2082 w2094 w2098 w2104 w2111 w2123 w2132 w2137 w2145 w2155 w2163 w2185 w2194 w2218 w2239 w2250 w2271 w2275 w2280 w2288 w2296 w2305 w2311 w2319 w2326 w2336 w2364 w2372 w2379 w2387 w2392 w2397 w2408 w2413 w2419 w2438 w2443 w2451 w2461 w2478 w2549 w2555 w2568 w2585 w2594 w2611 w2626 w2650 w2661 w2672 w2696 w2722 w2728 w2741 w2765 w2774 w2780 w2785 w2792 w2800 w2813 w2823 w2828 w2840 w2845 w2851 w2861 w2867 w2872 w2877 w2882 w2892 w2917 w2938 w2942 w2954 w2979 w3006 w3029 w3033 w3049 w3095 w3144 w3190 w3200 w3217 w3237 w3251 w3265 w3271 w3289 w3311 w3335 w3354 w3372 w3390 w3408 w3422 w3436 w3455 w3469 w3486 w3501 w3511 w3515 w3520 w3543 w3549 w3568 w3577 w3581] -> w88
      tunnel: 40 ("Timeout") -> [w97 _ _ _ _ _ _ _ _ _ _ _ _ _ _ _ _ _ _ _ _ _ _ _ _ _ _ _ _ _ _ _ _ _ _ _ _ _ _ _ _ _ _ _ _ _ _ _ _ _ _ _ _ _ _ _ _ _ _ _ _ _ _ _ _ _ _ _ _ _ _ _ _ _ _ _ _ _ _ _ _ _ _ _ _ _ _ _ _ _ _ _ _ _ _ _ _ _ _ _ _ _ _ _ _ _ _ _ _ _ _ _ _ _ _ _ _ _ _ _ _ _ _ _ _ _ _ _ _ _ _ _ _ _ _ _ _ _ _ _ _ _ _ _ _ _ _ _ _ _ _ _ _ _ _ _ _ _ _ _ _ _ _ _ _ _ _ _ _ _ _ _ _ _ _ _ _ _ _ _ _ _ _ _ _ _ _ _ _ _ _]
      tunnel: w85 -> [_ _ _ _ _ _ _ _ _ _ _ _ _ _ _ _ _ _ _ _ _ _ _ _ w1100 _ _ _ _ _ _ _ _ _ _ _ _ _ _ _ _ _ _ _ _ _ _ _ _ _ _ _ _ _ _ _ _ _ _ _ _ _ _ _ _ _ _ _ _ _ _ _ _ _ _ _ _ _ _ _ w2079 w2090 _ _ _ _ _ _ _ _ _ _ _ _ _ _ _ _ _ _ _ _ _ _ _ _ _ _ _ _ _ _ _ _ _ _ _ _ _ _ _ _ _ _ _ _ _ _ _ _ _ _ _ _ _ _ _ _ _ _ _ _ _ _ _ _ _ _ _ _ _ _ _ _ _ _ _ _ _ _ _ _ _ _ _ _ _ _ _ _ _ _ _ _ _ _ _ _ _ _ _ _ _ _ _ _ _ _ _ _ _]
      tunnel: w84 -> [_ _ _ _ _ _ _ _ _ _ _ _ _ _ _ _ _ _ _ _ _ _ _ _ w1099 _ _ _ _ _ _ _ _ _ _ _ _ _ _ _ _ _ _ _ _ _ _ _ _ _ _ _ _ _ _ _ _ _ _ _ _ _ _ _ _ _ _ _ _ _ _ _ _ _ _ _ _ _ _ _ w2080 w2089 _ _ _ _ _ _ _ _ _ _ _ _ _ _ _ _ _ _ _ _ _ _ _ _ _ _ _ _ _ _ _ _ _ _ _ _ _ _ _ _ _ _ _ _ _ _ _ _ _ _ _ _ _ _ _ _ _ _ _ _ _ _ _ _ _ _ _ _ _ _ _ _ _ _ _ _ _ _ _ _ _ _ _ _ _ _ _ _ _ _ _ _ _ _ _ _ _ _ _ _ _ _ _ _ _ _ _ _ _]
      tunnel: w83 -> [w96 _ _ _ _ _ _ _ _ _ _ _ _ _ _ _ _ _ _ _ _ _ _ _ _ _ _ _ _ _ _ _ _ _ _ _ _ _ _ _ _ _ _ _ _ _ _ _ _ _ _ w1606 _ _ _ _ _ _ _ _ _ _ _ _ _ _ _ _ _ _ _ _ _ _ _ _ _ _ _ _ _ _ _ _ _ _ _ _ _ _ _ _ _ _ _ _ _ _ _ _ _ _ _ _ _ _ _ _ _ _ _ _ _ _ _ _ _ _ _ _ _ _ _ _ _ _ _ _ _ _ _ _ _ _ _ _ _ _ _ _ _ _ _ _ _ _ _ _ _ _ _ _ _ _ _ _ _ _ _ _ _ _ _ _ _ _ _ _ _ _ _ _ _ _ _ _ _ _ _ _ _ _ _ _ _ _ _ _ _ _ _]
      tunnel: w82 -> [w95 w518 w528 w533 w541 w548 w566 w588 w618 w638 w666 w691 w703 w774 w789 w818 w847 w879 w898 w927 w957 w974 w977 w1064 w1101 w1140 w1149 w1156 w1161 w1179 w1198 w1221 w1226 w1240 w1259 w1288 w1308 w1351 w1357 w1367 w1379 w1409 w1417 w1422 w1430 w1454 w1479 w1503 w1523 w1532 w1556 w1611 w1627 w1640 w1649 w1665 w1679 w1708 w1734 w1739 w1784 w1789 w1801 w1808 w1817 w1829 w1860 w1876 w1890 w1910 w1925 w1956 w1972 w1982 w1998 w2010 w2022 w2050 w2053 w2068 w2081 w2088 w2097 w2106 w2114 w2121 w2130 w2136 w2146 w2149 w2161 w2180 w2195 w2214 w2236 w2254 w2270 w2274 w2282 w2290 w2295 w2303 w2310 w2318 w2325 w2335 w2363 w2371 w2378 w2383 w2391 w2400 w2406 w2412 w2421 w2433 w2442 w2447 w2469 w2475 w2548 w2553 w2565 w2575 w2588 w2605 w2634 w2649 w2662 w2674 w2698 w2718 w2726 w2739 w2767 w2772 w2778 w2784 w2791 w2802 w2814 w2822 w2827 w2839 w2844 w2855 w2860 w2866 w2871 w2876 w2881 w2891 w2916 w2937 w2941 w2953 w2978 w3005 w3028 w3032 w3048 w3100 w3146 w3187 w3202 w3220 w3240 w3254 w3266 w3275 w3292 w3314 w3338 w3357 w3375 w3393 w3411 w3425 w3439 w3458 w3472 w3487 w3500 w3510 w3514 w3533 w3542 w3548 w3569 w3576 w3580]
      tunnel: [w94 w518 w528 w533 w541 w548 w566 w588 w618 w638 w666 w691 w703 w774 w789 w818 w847 w879 w898 w927 w957 w974 w977 w1064 w1101 w1140 w1149 w1156 w1161 w1179 w1198 w1221 w1226 w1240 w1259 w1288 w1308 w1351 w1357 w1367 w1379 w1409 w1417 w1422 w1430 w1454 w1479 w1503 w1523 w1532 w1556 w1611 w1627 w1640 w1649 w1665 w1679 w1708 w1734 w1739 w1784 w1789 w1801 w1808 w1817 w1829 w1860 w1876 w1890 w1910 w1925 w1956 w1972 w1982 w1998 w2010 w2022 w2050 w2053 w2068 w2081 w2088 w2097 w2106 w2114 w2121 w2130 w2136 w2146 w2149 w2161 w2180 w2195 w2214 w2236 w2254 w2270 w2274 w2282 w2290 w2295 w2303 w2310 w2318 w2325 w2335 w2363 w2371 w2378 w2383 w2391 w2400 w2406 w2412 w2421 w2433 w2442 w2447 w2469 w2475 w2548 w2553 w2565 w2575 w2588 w2605 w2634 w2649 w2662 w2674 w2698 w2718 w2726 w2739 w2767 w2772 w2778 w2784 w2791 w2802 w2814 w2822 w2827 w2839 w2844 w2855 w2860 w2866 w2871 w2876 w2881 w2891 w2916 w2937 w2941 w2953 w2978 w3005 w3028 w3032 w3048 w3100 w3146 w3187 w3202 w3220 w3240 w3254 w3266 w3275 w3292 w3314 w3338 w3357 w3375 w3393 w3411 w3425 w3439 w3458 w3472 w3487 w3500 w3510 w3514 w3533 w3542 w3548 w3569 w3576 w3580] -> w81
      tunnel: w77 -> [_ _ _ _ _ _ _ _ _ _ _ _ _ _ _ _ _ _ _ _ _ _ _ _ w1094 _ _ _ _ _ _ _ _ _ _ _ _ _ _ _ _ _ _ _ _ _ _ _ _ _ _ _ _ _ _ _ _ _ _ _ _ _ _ _ _ _ _ _ _ _ _ _ _ _ _ _ _ _ _ _ w2078 w2087 _ _ _ _ _ _ _ _ _ _ _ _ _ _ _ _ _ _ _ _ _ _ _ _ _ _ _ _ _ _ _ _ _ _ _ _ _ _ _ _ _ _ _ _ _ _ _ _ _ _ _ _ _ _ _ _ _ _ _ _ _ _ _ _ _ _ _ _ _ _ _ _ _ _ _ _ _ _ _ _ _ _ _ _ _ _ _ _ _ _ _ _ _ _ _ _ _ _ _ _ _ _ _ _ _ _ _ _ _]
      frame "", "Event Structure", "Idle" {
        # "executes when the state queue is empty"
        n31 = event shown="[37] <AcqLoop error?>: User Event" {
          selector: w95 -> [_ _ _ _ _ _ _ _ _ _ _ _ _ _ _ _ _ _ _ _ _ _ _ _ _ _ _ _ _ _ _ _ _ _ _ _ _ _ _]
          dyn-events: [_ _ _ _ _ _ _ _ _ _ _ _ _ _ _ _ _ _ _ _ _ _ _ _ _ _ _ _ _ _ _ _ _ _ _ _ _ _ _] -> w94
          timeout: w97 -> [_ _ _ _ _ _ _ _ _ _ _ _ _ _ _ _ _ _ _ _ _ _ _ _ _ _ _ _ _ _ _ _ _ _ _ _ _ _ _]
          tunnel: w102 -> [w122 w141 w149 w153 w157 w165 w171 w179 w187 w197 w204 w233 w253 w273 w293 w297 w304 w327 w341 w355 w369 w374 w377 w383 w390 w397 w403 w409 w415 w422 w435 w446 w458 w465 w469 w473 w480 w495 w517]
          tunnel: [w123 w141 w148 w153 w156 w165 w171 w179 w187 w197 w203 w233 w253 w273 w293 w297 w303 w327 w341 w355 w369 w373 w376 w383 w391 w398 w402 w408 w415 w423 w436 w446 w459 w465 w469 w472 w479 w496 w516] -> w101
          tunnel: w100 -> [w106 w139 w143 w151 w158 w164 w172 w180 w188 w195 w199 w231 w251 w271 w291 w295 w299 w326 w340 w354 w368 w370 w378 w381 w386 w393 w405 w410 w413 w417 w430 w444 w454 w463 w467 w474 w481 w484 w514]
          tunnel: [w121 w140 w144 w152 w159 w163 w170 w178 w186 w196 w205 w232 w252 w272 w292 w296 w305 w324 w328 w351 w366 w372 w379 w382 w387 w394 w406 w411 w414 w421 w434 w445 w455 w464 w468 w475 w482 w497 w515] -> w93
          tunnel: w99 -> [w121 w140 w144 w152 w159 w163 w170 w178 w186 w196 w205 w232 w252 w272 w292 w296 w305 w321 w330 w342 w358 w372 w379 w382 w387 w394 w406 w411 w414 w421 w434 w445 w457 w464 w468 w475 w482 w497 w515]
          tunnel: [w106 w139 w143 w151 w158 w164 w172 w180 w188 w195 w200 w231 w251 w271 w291 w295 w300 w326 w340 w354 w368 w370 w378 w381 w388 w395 w405 w410 w413 w418 w431 w444 w460 w463 w467 w474 w481 w494 w514] -> w98
          tunnel: w96 -> [_ _ _ _ _ _ _ _ _ _ _ _ _ _ _ _ _ _ _ _ _ _ _ _ _ _ _ _ _ _ _ _ _ _ _ _ _ _ _]
          event Timeout {
            # "check system status every 2s"
            n32 = event-data() -> ()  [unwired: 1 in, 1 out]
            n33 = Unbundle By Name(w106) -> ("SysRunning?"=w104:bool, "SlowTimer"=w120:u32, "FastTimer"=w114:u32)
            n34 = Tick Count (ms)() -> (millisecond timer value=w107:u32)
            n35 = Subtract(x=w107, y=w120) -> (x-y=w117:u32)
            n36 = case shown="False" w104 {
              tunnel: ["" "Utility: AquiTimerCheck" ("State(s) in Front (\"\")")] -> w112
              frame False {
                # "if not running, do nothing"
              }
              frame True {
                # "if aquisition is running, check timer"
              }
            }
            n37 = Subtract(x=w107, y=w114) -> (x-y=w115:u32)
            n38 = Greater?(x=w117, y=u32 2000) -> (0:w118:bool)
            n39 = Greater?(x=w115, y=u32 500) -> (0:w105:bool)
            n40 = disable-structure shown="Enabled" {
              disable-tunnel: w105 -> [w128 _]
              disable-tunnel: w104 -> [w127 _]
              disable-tunnel: [w124 "" ("State(s) at Back (\"\")")] -> w103
              frame Disabled {
                n41 = Not(x=w127) -> (.not. x?=w126:bool)
                n42 = And(x=w128, y=w126) -> (x .and. y?=w125:bool)
                n43 = case shown="True" w125 {
                  tunnel: ["" ("Empty String Constant") "TCP: checkSource" ("State(s) in Front (\"\")")] -> w124
                  frame False {
                  }
                  frame True {
                  }
                }
              }
              frame Enabled {
              }
            }
            n44 = case shown="True" w118 {
              tunnel: ["" ("Empty String Constant") "SystemStatus: SlowSysStatusMacro" ("State(s) in Front (\"\")")] -> w110
              frame False {
              }
              frame True {
              }
            }
            n45 = case shown="True" w105 {
              tunnel: ["" ("Empty String Constant") "SystemStatus: FastSysStatusMacro" ("State(s) in Front (\"\")")] -> w108
              frame False {
              }
              frame True {
              }
            }
            n46 = call <vilib>:"Add State(s) to Queue__JKI_lib_State_Machine.vi"("State(s) in Front (\"\")"=w112, "State(s) in (\"\")"="LabJack: checkPedal" ("State(s) in Front (\"\")"), "State(s) at Back (\"\")"=w110) -> ("States Out"=w109:string)  [unwired: 12 in]
            n47 = call <vilib>:"Add State(s) to Queue__JKI_lib_State_Machine.vi"("State(s) in Front (\"\")"=w109, "State(s) in (\"\")"=w108, "State(s) at Back (\"\")"=w103) -> ("States Out"=w113:string)  [unwired: 12 in]
            n48 = call <vilib>:"Add State(s) to Queue__JKI_lib_State_Machine.vi"("State(s) in Front (\"\")"=w113, "State(s) in (\"\")"=w122) -> ("States Out"=w123:string)  [unwired: 13 in]
          }
          event "355nm Laser toggle": Mouse Enter {
            n49 = event-data() -> ()  [unwired: 1 in, 4 out]
            n50 = local write "Help"("Toggle 355nm laser." ("Help")) -> ()
          }
          event "355nm Laser toggle": Value Change {
            # "[Covers: REQ34]"
            n51 = event-data() -> ()  [unwired: 1 in, 6 out]
            n52 = Select(t="LabJack: 355_PWM_Start\nLabJack: AB_Start", s="355nm Laser toggle", f="LabJack: 355_PWM_Stop\nLabJack: AB_Stop") -> (s? t:f=w146:string)
            n53 = call <vilib>:"Add State(s) to Queue__JKI_lib_State_Machine.vi"("State(s) in Front (\"\")"=w146, "State(s) in (\"\")"=w149) -> ("States Out"=w148:string)  [unwired: 13 in]
          }
          event "Aiming beam toggle": Mouse Enter {
            n54 = event-data() -> ()  [unwired: 1 in, 4 out]
            n55 = local write "Help"("Toggle aiming beam laser." ("Help")) -> ()
          }
          event "Aiming beam toggle": Value Change {
            # "[Covers: REQ33]"
            n56 = event-data() -> ()  [unwired: 1 in, 6 out]
            n57 = case shown="True" "Aiming beam toggle" {
              tunnel: ["LabJack: AB_Stop" ("State(s) in Front (\"\")") "LabJack: AB_Start" ("State(s) in Front (\"\")")] -> w155
              frame False {
              }
              frame True {
              }
            }
            n58 = call <vilib>:"Add State(s) to Queue__JKI_lib_State_Machine.vi"("State(s) in Front (\"\")"=w155, "State(s) in (\"\")"=w157) -> ("States Out"=w156:string)  [unwired: 13 in]
          }
          event "Auto gain ch1": Value Change {
            n59 = event-data() -> ("NewVal"=w162:bool)  [unwired: 1 in, 5 out]
            n60 = case shown="True" w162 {
              frame False {
                n61 = local read "V 1"() -> (w166:dbl)
                n62 = call "V1FGV.vi"("action (write)"=enum16{"write", "read"}."write" ("action"), "V1 in"=w166) -> ()  [unwired: 8 in, 2 out]
                n63 = property on="V 1" class="DigNum (strict)"("DisabledEnum"=T12."Enabled" ("Disabled")) -> ()  [unwired: 2 in, 2 out]
              }
              frame True {
                n64 = property on="V 1" class="DigNum (strict)"("DisabledEnum"=T12."Disabled and Grayed Out" ("Disabled")) -> ()  [unwired: 2 in, 2 out]
              }
            }
          }
          event "Auto gain ch2": Value Change {
            n65 = event-data() -> ("NewVal"=w173:bool)  [unwired: 1 in, 5 out]
            n66 = case shown="False" w173 {
              frame False {
                n67 = local read "V 2"() -> (w174:dbl)
                n68 = property on="V 2" class="DigNum (strict)"("DisabledEnum"=T12."Enabled" ("Disabled")) -> ()  [unwired: 2 in, 2 out]
                n69 = call "V2FGV.vi"("action(write)"=enum16{"write", "read"}."write" ("action"), "V2 in"=w174) -> ()  [unwired: 8 in, 2 out]
              }
              frame True {
                n70 = property on="V 2" class="DigNum (strict)"("DisabledEnum"=T12."Disabled and Grayed Out" ("Disabled")) -> ()  [unwired: 2 in, 2 out]
              }
            }
          }
          event "Auto gain ch3": Value Change {
            n71 = event-data() -> ("NewVal"=w181:bool)  [unwired: 1 in, 5 out]
            n72 = case shown="False" w181 {
              frame False {
                n73 = local read "V 3"() -> (w182:dbl)
                n74 = property on="V 3" class="DigNum (strict)"("DisabledEnum"=T12."Enabled" ("Disabled")) -> ()  [unwired: 2 in, 2 out]
                n75 = call "V3FGV.vi"("action(write)"=enum16{"write", "read"}."write" ("action"), "V3 in"=w182) -> ()  [unwired: 8 in, 2 out]
              }
              frame True {
                n76 = property on="V 3" class="DigNum (strict)"("DisabledEnum"=T12."Disabled and Grayed Out" ("Disabled")) -> ()  [unwired: 2 in, 2 out]
              }
            }
          }
          event "Auto gain ch4": Value Change {
            n77 = event-data() -> ("NewVal"=w189:bool)  [unwired: 1 in, 5 out]
            n78 = case shown="False" w189 {
              frame False {
                n79 = local read "V 4"() -> (w190:dbl)
                n80 = property on="V 4" class="DigNum (strict)"("DisabledEnum"=T12."Enabled" ("Disabled")) -> ()  [unwired: 2 in, 2 out]
                n81 = call "V4FGV.vi"("action(write)"=enum16{"write", "read"}."write" ("action"), "V3 in"=w190) -> ()  [unwired: 8 in, 2 out]
              }
              frame True {
                n82 = property on="V 4" class="DigNum (strict)"("DisabledEnum"=T12."Disabled and Grayed Out" ("Disabled")) -> ()  [unwired: 2 in, 2 out]
              }
            }
          }
          event "Background": Mouse Enter {
            n83 = event-data() -> ()  [unwired: 1 in, 4 out]
            n84 = local write "Help"("Click to record a background." ("Help")) -> ()
          }
          event "Background": Value Change {
            n85 = event-data() -> ("NewVal"=w201:bool)  [unwired: 1 in, 5 out]
            n86 = case shown="True" w201 {
              tunnel: ["Utility: SetAllChanManualGain\nQueue: Flash\nUtility: Dewelling >> 2500\nLabJack: 355_PWM_Stop\nLabJack: AB_Stop" "Utility: SetDataClass >> Bg\nUI: Update\nLabJack: 355_PWM_Start\nLabJack: AB_Start\nUtility: SaveDeconChan\nUtility: Dewelling >> 50\nLabJack: SetV\nDigitizer: Start\nUtility: AquiTimerReset\nLED: BreathGreen\nUI: duringBGAcquire"] -> w202
              tunnel: [FALSE TRUE] -> w198
              frame False {
                n87 = local read "Skip Data Save?"() -> (w206:bool)
                n88 = case shown="False" w206 {
                  frame False {
                    n89 = property on="Background" class="Bool (strict)"("BoolText.Text"="Done!" ("Boolean Text.Text")) -> ()  [unwired: 2 in, 2 out]
                  }
                  frame True {
                  }
                }
              }
              frame True {
                # "[Covers: REQ6]"
                n90 = property on="Background" class="Bool (strict)"("BoolText.Text"="Running" ("Boolean Text.Text"), "Colors [4]"=cluster{u32, u32}[] [{6618880, 6618880}, {16711680, 16711680}]) -> ()  [unwired: 2 in, 2 out]
              }
            }
            n91 = Bundle By Name(cluster=w199, "SysRunning?"=w198) -> (w200:T24)
            n92 = call <vilib>:"Add State(s) to Queue__JKI_lib_State_Machine.vi"("State(s) in Front (\"\")"=w202, "State(s) in (\"\")"=w204) -> ("States Out"=w203:string)  [unwired: 13 in]
          }
          event "Channel 1": Cursor Move {
            n93 = event-data() -> ("CursIdx"=w217:i32, "CursLoc"=w229:cluster{"X":dbl, "Y":dbl})  [unwired: 1 in, 7 out]
            n94 = property on="Channel 3" class="WFGraph (strict)"() -> ("CrsrList"=w224:T25)  [unwired: 2 in, 2 out]
            n95 = property on="Channel 4" class="WFGraph (strict)"() -> ("CrsrList"=w216:T25)  [unwired: 2 in, 2 out]
            n96 = property on="Channel 2" class="WFGraph (strict)"() -> ("CrsrList"=w227:T25)  [unwired: 2 in, 2 out]
            n97 = Index Array(array=w224, index=w217) -> (element=w228:T26)
            n98 = Index Array(array=w216, index=w217) -> (element=w219:T26)
            n99 = Unbundle By Name(w229) -> ("X"=w218:dbl)
            n100 = Index Array(array=w227, index=w217) -> (element=w230:T26)
            n101 = Bundle By Name(cluster=w228, "Position.X"=w218) -> (w223:T26)
            n102 = Bundle By Name(cluster=w219, "Position.X"=w218) -> (w215:T26)
            n103 = Bundle By Name(cluster=w230, "Position.X"=w218) -> (w226:T26)
            n104 = control-ref of="Channel 1"() -> (w220:refnum<vi>)
            n105 = Replace Array Subset(array=w224, new element=w223, index=w217) -> (w222:T25)
            n106 = Replace Array Subset(array=w216, new element=w215, index=w217) -> (w214:T25)
            n107 = Replace Array Subset(array=w227, new element=w226, index=w217) -> (w225:T25)
            n108 = property on="Channel 3" class="WFGraph (strict)"("CrsrList"=w222) -> (error out=w221:errorcluster)  [unwired: 2 in, 1 out]
            n109 = property on="Channel 4" class="WFGraph (strict)"("CrsrList"=w214) -> ()  [unwired: 2 in, 2 out]
            n110 = property on="Channel 2" class="WFGraph (strict)"("CrsrList"=w225) -> ()  [unwired: 2 in, 2 out]
            n111 = call "UpdateCurserIdx(SubVI).vi"("error in (no error)"=w221, "WaveformGraph in"=w220) -> ()  [unwired: 9 in, 1 out]
          }
          event "Channel 2": Cursor Move {
            n112 = event-data() -> ("CursIdx"=w236:i32, "CursLoc"=w250:cluster{"X":dbl, "Y":dbl})  [unwired: 1 in, 7 out]
            n113 = Unbundle By Name(w250) -> ("X"=w238:dbl)
            n114 = property on="Channel 1" class="WFGraph (strict)"() -> ("CrsrList"=w244:T25)  [unwired: 2 in, 2 out]
            n115 = property on="Channel 3" class="WFGraph (strict)"() -> ("CrsrList"=w246:T25)  [unwired: 2 in, 2 out]
            n116 = property on="Channel 4" class="WFGraph (strict)"() -> ("CrsrList"=w237:T25)  [unwired: 2 in, 2 out]
            n117 = Index Array(array=w244, index=w236) -> (element=w249:T26)
            n118 = Index Array(array=w246, index=w236) -> (element=w248:T26)
            n119 = Index Array(array=w237, index=w236) -> (element=w239:T26)
            n120 = Bundle By Name(cluster=w239, "Position.X"=w238) -> (w235:T26)
            n121 = Bundle By Name(cluster=w249, "Position.X"=w238) -> (w247:T26)
            n122 = Bundle By Name(cluster=w248, "Position.X"=w238) -> (w245:T26)
            n123 = Replace Array Subset(array=w244, new element=w247, index=w236) -> (w243:T25)
            n124 = Replace Array Subset(array=w246, new element=w245, index=w236) -> (w242:T25)
            n125 = Replace Array Subset(array=w237, new element=w235, index=w236) -> (w234:T25)
            n126 = control-ref of="Channel 1"() -> (w241:refnum<vi>)
            n127 = property on="Channel 1" class="WFGraph (strict)"("CrsrList"=w243) -> ()  [unwired: 2 in, 2 out]
            n128 = property on="Channel 3" class="WFGraph (strict)"("CrsrList"=w242) -> (error out=w240:errorcluster)  [unwired: 2 in, 1 out]
            n129 = property on="Channel 4" class="WFGraph (strict)"("CrsrList"=w234) -> ()  [unwired: 2 in, 2 out]
            n130 = call "UpdateCurserIdx(SubVI).vi"("error in (no error)"=w240, "WaveformGraph in"=w241) -> ()  [unwired: 9 in, 1 out]
          }
          event "Channel 3": Cursor Move {
            n131 = event-data() -> ("CursIdx"=w256:i32, "CursLoc"=w270:cluster{"X":dbl, "Y":dbl})  [unwired: 1 in, 7 out]
            n132 = Unbundle By Name(w270) -> ("X"=w258:dbl)
            n133 = property on="Channel 4" class="WFGraph (strict)"() -> ("CrsrList"=w257:T25)  [unwired: 2 in, 2 out]
            n134 = property on="Channel 1" class="WFGraph (strict)"() -> ("CrsrList"=w267:T25)  [unwired: 2 in, 2 out]
            n135 = property on="Channel 2" class="WFGraph (strict)"() -> ("CrsrList"=w265:T25)  [unwired: 2 in, 2 out]
            n136 = Index Array(array=w257, index=w256) -> (element=w259:T26)
            n137 = Index Array(array=w267, index=w256) -> (element=w269:T26)
            n138 = Index Array(array=w265, index=w256) -> (element=w268:T26)
            n139 = Bundle By Name(cluster=w259, "Position.X"=w258) -> (w255:T26)
            n140 = Bundle By Name(cluster=w269, "Position.X"=w258) -> (w266:T26)
            n141 = Bundle By Name(cluster=w268, "Position.X"=w258) -> (w264:T26)
            n142 = Replace Array Subset(array=w257, new element=w255, index=w256) -> (w254:T25)
            n143 = Replace Array Subset(array=w267, new element=w266, index=w256) -> (w263:T25)
            n144 = Replace Array Subset(array=w265, new element=w264, index=w256) -> (w262:T25)
            n145 = control-ref of="Channel 1"() -> (w260:refnum<vi>)
            n146 = property on="Channel 4" class="WFGraph (strict)"("CrsrList"=w254) -> ()  [unwired: 2 in, 2 out]
            n147 = property on="Channel 1" class="WFGraph (strict)"("CrsrList"=w263) -> ()  [unwired: 2 in, 2 out]
            n148 = property on="Channel 2" class="WFGraph (strict)"("CrsrList"=w262) -> (error out=w261:errorcluster)  [unwired: 2 in, 1 out]
            n149 = call "UpdateCurserIdx(SubVI).vi"("error in (no error)"=w261, "WaveformGraph in"=w260) -> ()  [unwired: 9 in, 1 out]
          }
          event "Channel 4": Cursor Move {
            n150 = event-data() -> ("CursIdx"=w278:i32, "CursLoc"=w290:cluster{"X":dbl, "Y":dbl})  [unwired: 1 in, 7 out]
            n151 = Unbundle By Name(w290) -> ("X"=w276:dbl)
            n152 = property on="Channel 1" class="WFGraph (strict)"() -> ("CrsrList"=w288:T25)  [unwired: 2 in, 2 out]
            n153 = property on="Channel 2" class="WFGraph (strict)"() -> ("CrsrList"=w284:T25)  [unwired: 2 in, 2 out]
            n154 = property on="Channel 3" class="WFGraph (strict)"() -> ("CrsrList"=w279:T25)  [unwired: 2 in, 2 out]
            n155 = Index Array(array=w288, index=w278) -> (element=w289:T26)
            n156 = Index Array(array=w284, index=w278) -> (element=w285:T26)
            n157 = Index Array(array=w279, index=w278) -> (element=w281:T26)
            n158 = Bundle By Name(cluster=w289, "Position.X"=w276) -> (w287:T26)
            n159 = Bundle By Name(cluster=w285, "Position.X"=w276) -> (w283:T26)
            n160 = Bundle By Name(cluster=w281, "Position.X"=w276) -> (w280:T26)
            n161 = Replace Array Subset(array=w288, new element=w287, index=w278) -> (w286:T25)
            n162 = Replace Array Subset(array=w284, new element=w283, index=w278) -> (w282:T25)
            n163 = Replace Array Subset(array=w279, new element=w280, index=w278) -> (w277:T25)
            n164 = control-ref of="Channel 1"() -> (w274:refnum<vi>)
            n165 = call "UpdateCurserIdx(SubVI).vi"() -> ()  [unwired: 11 in, 1 out]
            n166 = call "UpdateCurserIdx(SubVI).vi"() -> ()  [unwired: 11 in, 1 out]
            n167 = property on="Channel 1" class="WFGraph (strict)"("CrsrList"=w286) -> ()  [unwired: 2 in, 2 out]
            n168 = property on="Channel 2" class="WFGraph (strict)"("CrsrList"=w282) -> ()  [unwired: 2 in, 2 out]
            n169 = property on="Channel 3" class="WFGraph (strict)"("CrsrList"=w277) -> (error out=w275:errorcluster)  [unwired: 2 in, 1 out]
            n170 = call "UpdateCurserIdx(SubVI).vi"("error in (no error)"=w275, "WaveformGraph in"=w274) -> ()  [unwired: 9 in, 1 out]
          }
          event "Cali&iRF alignment": Mouse Enter {
            n171 = event-data() -> ()  [unwired: 1 in, 4 out]
            n172 = local write "Help"("Click to run system intensity calibration and irf alignment" ("Help")) -> ()
          }
          event "Cali&iRF alignment": Value Change {
            n173 = event-data() -> ("NewVal"=w301:bool)  [unwired: 1 in, 5 out]
            n174 = case shown="False" w301 {
              tunnel: ["Utility: SetAllChanManualGain\nQueue: Flash\nUtility: Dewelling >> 2500\nLabJack: 355_PWM_Stop\nLabJack: AB_Stop" "Utility: SetDataClass >> Cali\nUI: Update\nUtility: SaveDeconChan\nLabJack: 355_PWM_Start\nLabJack: AB_Start\nLabJack: SetV\nDigitizer: Start\nUtility: AquiTimerReset\nLED: BreathGreen\nUI: duringIRFAlign"] -> w302
              tunnel: [FALSE TRUE] -> w298
              frame False {
                n175 = local read "Skip Data Save?"() -> (w306:bool)
                n176 = case shown="False" w306 {
                  frame False {
                    n177 = property on="Cali&iRF alignment" class="Bool (strict)"("BoolText.Text"="Done!" ("Boolean Text.Text")) -> ()  [unwired: 2 in, 2 out]
                  }
                  frame True {
                  }
                }
              }
              frame True {
                n178 = property on="Cali&iRF alignment" class="Bool (strict)"("BoolText.Text"="Running" ("Boolean Text.Text"), "Colors [4]"=cluster{u32, u32}[] [{6618880, 6618880}, {16711680, 16711680}]) -> ()  [unwired: 2 in, 2 out]
              }
            }
            n179 = Bundle By Name(cluster=w299, "SysRunning?"=w298) -> (w300:T24)
            n180 = call <vilib>:"Add State(s) to Queue__JKI_lib_State_Machine.vi"("State(s) in Front (\"\")"=w302, "State(s) in (\"\")"=w304) -> ("States Out"=w303:string)  [unwired: 13 in]
          }
          event "V 1": Value Change {
            n181 = event-data() -> ()  [unwired: 1 in, 6 out]
            n182 = call "LabJack_FGV.vi"("Operation(Read)"=enum16{"Write", "Read"}."Read" ("Operation"), "error in (no error)"=w321) -> ("error out"=w318:errorcluster, "Read data"=w319:i32)  [unwired: 8 in]
            n183 = global read "GlobalVariables.vi" "Ch1 LJ pin"() -> (w317:string)
            n184 = call "LJM_eWriteName.vi"("Handle In"=w319, "Name"=w317, "Value"="V 1", "error in"=w318) -> ("error out"=w315:errorcluster)  [unwired: 10 in, 1 out]
            n185 = call "V1FGV.vi"("Error In"=w315, "action (write)"=enum16{"write", "read"}."write" ("action"), "V1 in"="V 1") -> ("Error Out"=w314:errorcluster)  [unwired: 7 in, 1 out]
            n186 = call "CtrlVtoGain.vi"("error in (no error)"=w314, "CtrlV(V)"="V 1", "Channel"=enum16{"Ch1", "Ch2", "Ch3"}."Ch1" ("Enum")) -> ("error out"=w324:errorcluster, "Gain"=w323:dbl)  [unwired: 7 in]
            n187 = local write "Gain1"(w323) -> ()
          }
          event "V 2": Value Change {
            n188 = event-data() -> ()  [unwired: 1 in, 6 out]
            n189 = call "LabJack_FGV.vi"("Operation(Read)"=enum16{"Write", "Read"}."Read" ("Operation"), "error in (no error)"=w330) -> ("error out"=w335:errorcluster, "Read data"=w336:i32)  [unwired: 8 in]
            n190 = global read "GlobalVariables.vi" "Ch2 LJ pin"() -> (w334:string)
            n191 = call "LJM_eWriteName.vi"("Handle In"=w336, "Name"=w334, "Value"="V 2", "error in"=w335) -> ("error out"=w333:errorcluster)  [unwired: 10 in, 1 out]
            n192 = call "V2FGV.vi"("Error In"=w333, "action(write)"=enum16{"write", "read"}."write" ("action"), "V2 in"="V 2") -> ("Error Out"=w332:errorcluster)  [unwired: 7 in, 1 out]
            n193 = call "CtrlVtoGain.vi"("error in (no error)"=w332, "CtrlV(V)"="V 2", "Channel"=enum16{"Ch1", "Ch2", "Ch3"}."Ch2" ("Enum")) -> ("error out"=w328:errorcluster, "Gain"=w329:dbl)  [unwired: 7 in]
            n194 = local write "Gain2"(w329) -> ()
          }
          event "V 3": Value Change {
            n195 = event-data() -> ()  [unwired: 1 in, 6 out]
            n196 = call "LabJack_FGV.vi"("Operation(Read)"=enum16{"Write", "Read"}."Read" ("Operation"), "error in (no error)"=w342) -> ("error out"=w347:errorcluster, "Read data"=w348:i32)  [unwired: 8 in]
            n197 = global read "GlobalVariables.vi" "Ch3 LJ pin"() -> (w346:string)
            n198 = call "LJM_eWriteName.vi"("Handle In"=w348, "Name"=w346, "Value"="V 3", "error in"=w347) -> ("error out"=w344:errorcluster)  [unwired: 10 in, 1 out]
            n199 = call "V3FGV.vi"("Error In"=w344, "action(write)"=enum16{"write", "read"}."write" ("action"), "V3 in"="V 3") -> ("Error Out"=w343:errorcluster)  [unwired: 7 in, 1 out]
            n200 = call "CtrlVtoGain.vi"("error in (no error)"=w343, "CtrlV(V)"="V 3", "Channel"=enum16{"Ch1", "Ch2", "Ch3"}."Ch3" ("Enum")) -> ("error out"=w351:errorcluster, "Gain"=w350:dbl)  [unwired: 7 in]
            n201 = local write "Gain3"(w350) -> ()
          }
          event "V 4": Value Change {
            n202 = event-data() -> ()  [unwired: 1 in, 6 out]
            n203 = call "LabJack_FGV.vi"("Operation(Read)"=enum16{"Write", "Read"}."Read" ("Operation"), "error in (no error)"=w358) -> ("error out"=w362:errorcluster, "Read data"=w363:i32)  [unwired: 8 in]
            n204 = global read "GlobalVariables.vi" "Ch4 LJ pin"() -> (w361)
            n205 = call "LJM_eWriteName.vi"("Handle In"=w363, "Name"=w361, "Value"="V 4", "error in"=w362) -> ("error out"=w360:errorcluster)  [unwired: 10 in, 1 out]
            n206 = call "V4FGV.vi"("Error In"=w360, "action(write)"=enum16{"write", "read"}."write" ("action"), "V3 in"="V 4") -> ("Error Out"=w359:errorcluster)  [unwired: 7 in, 1 out]
            n207 = call "CtrlVtoGain.vi"("error in (no error)"=w359, "CtrlV(V)"="V 4", "Channel"=enum16{"Ch1", "Ch2", "Ch3", "Ch4"}."Ch4") -> ("error out"=w366:errorcluster, "Gain"=w365:dbl)  [unwired: 7 in]
            n208 = local write "Gain4"(w365) -> ()
          }
          event "Quit": Value Change {
            # "Exit Button Value Change (pressed) Event\n(when pressed.  quite)"
            n209 = event-data() -> ()  [unwired: 1 in, 1 out]
            n210 = call <vilib>:"Add State(s) to Queue__JKI_lib_State_Machine.vi"("State(s) in Front (\"\")"="LED: Off\nMacro: Exit", "State(s) in (\"\")"=w374) -> ("States Out"=w373:string)  [unwired: 13 in]
          }
          event "Show BG": Value Change {
            n211 = event-data() -> ()  [unwired: 1 in, 6 out]
            n212 = call <vilib>:"Add State(s) to Queue__JKI_lib_State_Machine.vi"("State(s) in Front (\"\")"="Data: showBG" ("State(s) in Front (\"\")"), "State(s) in (\"\")"=w377) -> ("States Out"=w376:string)  [unwired: 13 in]
          }
          event "StartButton": Mouse Enter {
            n213 = event-data() -> ()  [unwired: 1 in, 4 out]
            n214 = local write "Help"("Press to start aquisition." ("Help")) -> ()
          }
          event "StartButton": Value Change {
            # "[Covers: REQ32]"
            # "start PWM before acquisition"
            # "Initialize both digitizer aquisition and\n send user event to trigger aquisition loop"
            n215 = event-data() -> ()  [unwired: 1 in, 6 out]
            n216 = local write "StartButton"(FALSE ("StartButton")) -> ()
            n217 = Bundle By Name(cluster=w386, "SysRunning?"=TRUE) -> (w388:T24)
            n218 = call <vilib>:"Add State(s) to Queue__JKI_lib_State_Machine.vi"("State(s) in Front (\"\")"="TCP: stopCam\nUtility: SetDataClass >> Data\nQueue: Flash\nUI: Update\nDebug: OpenDebugTDMS\nUtility: StartBeep\nLabJack: 355_PWM_Start\nLabJack: AB_Start\nLabJack: SetV\nDigitizer: Start\nUtility: AquiTimerReset\nUI: DuringAquisition\nLED: BreathGreen\nTCP: sendRunNum\nTCP: sendVideoSource\nTCP: sendChannel\nTCP: startRun", "State(s) in (\"\")"=w390) -> ("States Out"=w391:string)  [unwired: 13 in]
          }
          event User Event {
            # "[Covers: REQ32]"
            # "start PWM before acquisition"
            # "Initialize both digitizer aquisition and\n send user event to trigger aquisition loop"
            n219 = event-data() -> ()  [unwired: 1 in, 5 out]
            n220 = Bundle By Name(cluster=w393, "SysRunning?"=TRUE) -> (w395:T24)
            n221 = call <vilib>:"Add State(s) to Queue__JKI_lib_State_Machine.vi"("State(s) in Front (\"\")"="TCP: stopCam\nUtility: SetDataClass >> Data\nQueue: Flash\nUI: Update\nUtility: StartBeep\nLabJack: 355_PWM_Start\nLabJack: AB_Start\nLabJack: SetV\nDigitizer: Start\nUtility: AquiTimerReset\nUI: DuringAquisition\nLED: BreathGreen\nTCP: sendRunNum\nTCP: sendVideoSource\nTCP: sendChannel\nTCP: startRun", "State(s) in (\"\")"=w397) -> ("States Out"=w398:string)  [unwired: 13 in]
          }
          event "Video Display": Value Change {
            n222 = event-data() -> ("NewVal"=w404:bool)  [unwired: 1 in, 5 out]
            n223 = Select(t="TCP: startCam", s=w404, f="TCP: stopCam") -> (s? t:f=w401:string)
            n224 = call <vilib>:"Add State(s) to Queue__JKI_lib_State_Machine.vi"("State(s) in (\"\")"=w403, "State(s) at Back (\"\")"=w401) -> ("States Out"=w402:string)  [unwired: 13 in]
          }
          event "Video Source": Value Change {
            n225 = event-data() -> ()  [unwired: 1 in, 6 out]
            n226 = call <vilib>:"Add State(s) to Queue__JKI_lib_State_Machine.vi"("State(s) in Front (\"\")"="TCP: sendVideoSource" ("State(s) in Front (\"\")"), "State(s) in (\"\")"=w409) -> ("States Out"=w408:string)  [unwired: 13 in]
          }
          event "StopButton": Mouse Enter {
            n227 = event-data() -> ()  [unwired: 1 in, 4 out]
            n228 = local write "Help"("Press to stop data aquisition." ("Help")) -> ()
          }
          event "StopButton": Value Change {
            # "if system is running, send stop command, if not do nothing."
            # "stop aquisition\nupdate UI"
            n229 = event-data() -> ()  [unwired: 1 in, 6 out]
            n230 = Unbundle By Name(w417) -> ("SysRunning?"=w419:bool)
            n231 = case shown="True" w419 {
              tunnel: ["" ("Empty String Constant") "LabJack: AB_Stop\nLabJack: 355_PWM_Stop\n/*Digitizer: Abort"] -> w420
              tunnel: w417 -> [w424 w428]
              tunnel: [w424 w427] -> w418
              frame False {
              }
              frame True {
                n232 = Bundle By Name(cluster=w428, "SysRunning?"=FALSE) -> (w427:T24)
              }
            }
            n233 = call <vilib>:"Add State(s) to Queue__JKI_lib_State_Machine.vi"("State(s) in Front (\"\")"=w420, "State(s) in (\"\")"=w422) -> ("States Out"=w423:string)  [unwired: 13 in]
            n234 = local write "StopButton"(FALSE ("StopButton")) -> ()
          }
          event User Event {
            # "if system is running, send stop command, if not do nothing."
            # "stop aquisition\nupdate UI"
            n235 = event-data() -> ()  [unwired: 1 in, 5 out]
            n236 = Unbundle By Name(w430) -> ("SysRunning?"=w432:bool)
            n237 = case shown="True" w432 {
              tunnel: ["" ("Empty String Constant") "LabJack: AB_Stop\nLabJack: 355_PWM_Stop\n/*Digitizer: Abort"] -> w433
              tunnel: w430 -> [w437 w441]
              tunnel: [w437 w440] -> w431
              frame False {
              }
              frame True {
                n238 = Bundle By Name(cluster=w441, "SysRunning?"=FALSE) -> (w440:T24)
              }
            }
            n239 = call <vilib>:"Add State(s) to Queue__JKI_lib_State_Machine.vi"("State(s) in Front (\"\")"=w433, "State(s) in (\"\")"=w435) -> ("States Out"=w436:string)  [unwired: 13 in]
          }
          event "Sys Reconfig": Mouse Enter {
            n240 = event-data() -> ()  [unwired: 1 in, 4 out]
            n241 = local write "Help"("Click to reconfig digitizer settings." ("Help")) -> ()
          }
          event "Sys Reconfig": Value Change {
            # "everytime the user change data aquisition setting, need to reinitilize decon engine and realign iRF.\ncheck whether data length has changed, if changed, reinitialize Decon engine\nreset BG ready, need a new BG"
            # "update DAQ FGV"
            n242 = event-data() -> ()  [unwired: 1 in, 6 out]
            n243 = call "SystemConfigEditorV6.vi"("error in"=w457) -> ("error out"=w456:errorcluster, "FLImDAQ out"=w451:T5)  [unwired: 1 in]
            n244 = Unbundle By Name(w454) -> ("FLImDAQ.min record length"=w453:i32)
            n245 = Unbundle By Name(w451) -> ("min record length"=w452:i32)
            n246 = call "FLImDAQ_FGV.vi"("error in (no error)"=w456, "Operation (Read)"=enum16{"Write", "Read"}."Write" ("Operation"), "Write data"=w451) -> ("error out"=w455:errorcluster, "Read data"=w450:T5)  [unwired: 7 in]
            n247 = Equal?(x=w453, y=w452) -> (x = y?=w449:bool)
            n248 = case shown="False" w449 {
              tunnel: ["UI: Cursor Set >> Busy\nDigitizer: Config\nDeconEngine: InitializeCh1\nDeconEngine: InitializeCh2\nDeconEngine: InitializeCh3\nUI: CaliAndiRFNotReady\n/*UI iRF not ready\nUI: Update\nUI: Cursor Set >> Idle" "UI: Cursor Set >> Busy\nDigitizer: Config\nUI: Update\nUI: Cursor Set >> Idle"] -> w448
              frame False {
              }
              frame True {
              }
            }
            n249 = Bundle By Name(cluster=w454, "FLImDAQ"=w450) -> (w460:T24)
            n250 = call <vilib>:"Add State(s) to Queue__JKI_lib_State_Machine.vi"("State(s) in Front (\"\")"=w448, "State(s) in (\"\")"=w458) -> ("States Out"=w459:string)  [unwired: 13 in]
          }
          event "System Hardware Connection Status", "StartButton", "StopButton", "355nm Laser toggle", "Aiming beam toggle", "Cali&iRF alignment", "Background", "Sys Reconfig": Mouse Leave {
            n251 = event-data() -> ()  [unwired: 1 in, 4 out]
            n252 = invoke on="Help" class="Str" method="Reinit To Default"() -> ()  [unwired: 3 in, 3 out]
          }
          event "System Hardware Connection Status.Digitizer": Mouse Enter {
            n253 = event-data() -> ()  [unwired: 1 in, 4 out]
            n254 = local write "Help"("Status of hardware connections. TCP/IP is optional." ("Help")) -> ()
          }
          event "TCP Connect": Value Change {
            n255 = event-data() -> ("NewVal"=w470:bool)  [unwired: 1 in, 5 out]
            n256 = case shown="True" w470 {
              tunnel: ["TCP: Close\nUI: Update" ("State(s) in Front (\"\")") "TCP: SendSettingMacro\nUI: Update" ("State(s) in Front (\"\")")] -> w471
              frame False {
              }
              frame True {
              }
            }
            n257 = call <vilib>:"Add State(s) to Queue__JKI_lib_State_Machine.vi"("State(s) in Front (\"\")"=w471, "State(s) in (\"\")"=w473) -> ("States Out"=w472:string)  [unwired: 13 in]
          }
          event "488nm Power": Value Change {
            n258 = event-data() -> ()  [unwired: 1 in, 6 out]
            n259 = call <vilib>:"Add State(s) to Queue__JKI_lib_State_Machine.vi"("State(s) in Front (\"\")"="AimingBeam: Set Current" ("State(s) in Front (\"\")"), "State(s) in (\"\")"=w480) -> ("States Out"=w479:string)  [unwired: 13 in]
          }
          event User Event {
            # "if aquisition loop is error out. Stop digitizer, update front panel indicator, stop both laser and \nOption 1: parse and save data\nOption 2: Flash queue if scout run. [Covers: REQ23]"
            n260 = event-data() -> ()  [unwired: 1 in, 5 out]
            n261 = Unbundle By Name(w484) -> ("OverlaySelection"=w483:u16)
            n262 = case shown="\"BG\"" "Data Class" {
              tunnel: [w501 "UI: Cursor Set >> Busy\nUtility: SetAllChanAutoGain\nUtility: RestoreDeConChan\nData: parseRunData\nData: irfAlignment\nUI: Cursor Set >> Idle" w505] -> w492
              tunnel: w483 -> [_ _ w508]
              frame "Data", Default {
                n263 = local read "Video Display"() -> (w503:bool)
                n264 = Select(t="TCP: startCam", s=w503, f="") -> (s? t:f=w499:string)
                n265 = call <vilib>:"Add State(s) to Queue__JKI_lib_State_Machine.vi"("State(s) in Front (\"\")"="UI: Cursor Set >> Busy\nData: parseRunData\nData: saveRunData\nUI: Cursor Set>>Idle" ("State(s) in Front (\"\")"), "State(s) in (\"\")"=w499) -> ("States Out"=w501:string)  [unwired: 13 in]
              }
              frame "Cali" {
              }
              frame "BG" {
                w509 = "UI: Cursor Set >> Busy\nUtility: SetAllChanAutoGain\nUtility: RestoreDeConChan\nData: parseRunData\nData: saveBGtoFGV\nData: saveBGtoFile\nUI: Cursor Set >> Idle\nData: showBG\nRun: BGIncrement"  # UI: Cursor Set >> Busy Utility: SetAllChanAutoGain Utility: RestoreDeConChan Data: parseRunData Data: saveBGtoFGV Data: saveBGtoFile UI: Cursor Set >> Idle Data: showBG Run: BGIncrement
                n266 = Greater Than 0?(x=w508) -> (x > 0?=w507:bool)
                n267 = case shown="True" w507 {
                  tunnel: ["" ("State(s) in (\"\")") "Data: processDeConBG\nData: saveDeConBGtoFile" ("State(s) in (\"\")")] -> w506
                  frame False {
                  }
                  frame True {
                  }
                }
                n268 = call <vilib>:"Add State(s) to Queue__JKI_lib_State_Machine.vi"("State(s) in Front (\"\")"=w509, "State(s) in (\"\")"=w506) -> ("States Out"=w505:string)  [unwired: 13 in]
              }
            }
            n269 = Bundle By Name(cluster=w484, "SysRunning?"=FALSE) -> (w494:T24)
            n270 = Select(t="" ("State(s) in Front (\"\")"), s="Skip Data Save?", f=w492) -> (s? t:f=w489:string)
            n271 = call <vilib>:"Add State(s) to Queue__JKI_lib_State_Machine.vi"("State(s) in Front (\"\")"="TCP: stopRun\nUI: Update\nLabJack: AB_Stop\nLabJack: 355_PWM_Stop\nDigitizer: Abort\nLabJack: ZeroV\nUtility: EndBeep\nDebug: CloseDebugTDMS\nLED: BreathOff" ("State(s) in Front (\"\")"), "State(s) in (\"\")"=w489, "State(s) at Back (\"\")"="Macro: SysReadyForAq\nUI: Update" ("State(s) in Front (\"\")")) -> ("States Out"=w487:string)  [unwired: 12 in]
            n272 = call <vilib>:"Add State(s) to Queue__JKI_lib_State_Machine.vi"("State(s) in Front (\"\")"=w487, "State(s) in (\"\")"=w495) -> ("States Out"=w496:string)  [unwired: 13 in]
          }
          event Panel Close? {
            # "Discard the event because we'll close the front panel ourselves in Macro: Exit"
            # "Close Panel button (pressed) Event\n(this executes Macro: Exit to terminate the VI)"
            n273 = event-data() -> ()  [unwired: 1 in, 1 out]
            n274 = event-data ("Event Filter Node")("Discard?"=TRUE) -> ()  [unwired: 1 in, 1 out]
            n275 = call <vilib>:"Add State(s) to Queue__JKI_lib_State_Machine.vi"("State(s) in Front (\"\")"="Macro: Exit", "State(s) in (\"\")"=w517) -> ("States Out"=w516:string)  [unwired: 13 in]
          }
        }
      }
      frame "---------- Macro ----------" {
        # "Do not put any code in this frame.\n(It is a separator no-op. You can make a copy of this frame to create a new Macro frame)"
        n276 = call <vilib>:"Add State(s) to Queue__JKI_lib_State_Machine.vi"("State(s) in (\"\")"=w522) -> ("States Out"=w521:string)  [unwired: 14 in]
      }
      frame "Macro: Initialize" {
        # "load Labjack setting 1st as it contaisn laser pin infortmation"
        # "start laser 1st, need 7.5s for laser to get ready"
        # "Initialization Macro\n(This is called once, when the VI starts)"
        n277 = call <vilib>:"Add State(s) to Queue__JKI_lib_State_Machine.vi"("State(s) in Front (\"\")"="UI: showDisclaimer\nData: Initialize\nInitialize Core Data\nUI: OverlayDialog\nUI: Cursor Set >> Busy\nUI: Initialize\nUI: Front Panel State >> Open\nMacro: LoadSysConfig\nTCP: InitializeNew\nTCP: checkSource\nUI: Update\nLabJack: Open\nLabJack: SetDefaultSub\nLED: OpenVIRef\nLED: BreathOrange\nUI: Update\n355 Laser: CheckControllerStatus\n355 Laser: Laser enable\n355 Laser: Dewelling>>500\n355 Laser: CheckControllerStatus\nUI: Update\nLabJack: 355_PWM_Config\nLabJack: AB_PWM_Config", "State(s) in (\"\")"="Digitizer: Initialize\nDigitizer: Config\nUI: Update\nAimingBeam: Initialize\nAimingBeam: Set APC Status>>Disable\nAimingBeam: Set ACC Status>>Enable\nAimingBeam: Set Current\nUI: Update\n355 Laser: Check Dewelling\nUI: Cursor Set >> Idle\nCase: GetID\nUI: Update\nTCP: SendSettingMacro\nCase: CreatFileStruct\nUI: Update\nData: loadLastUseMacro\nGraph: SetXMultiplier\nGraph: AddCursors\nAPD: Initialize\nAPD: LoadFromSerial\nAPD: UpdateCtrlVLimit\nAPD: GetGainLimits\nPID: loadPID\nMacro: InitDeConAndClassifier\nLED: BreathOff\nMacro: SysReadyForAq") -> ("States Out"=w523:string)  [unwired: 13 in]
        n278 = call <vilib>:"Add State(s) to Queue__JKI_lib_State_Machine.vi"("State(s) in Front (\"\")"=w523, "State(s) in (\"\")"=w531) -> ("States Out"=w530:string)  [unwired: 13 in]
        "Help" <- "Hover over controls to see help!" ("Help")
      }
      frame "Macro: LoadSysConfig" {
        # "System configuration Macro. [Covers: REQ15]\n(Load configurations for different component of the system)"
        n279 = call <vilib>:"Add State(s) to Queue__JKI_lib_State_Machine.vi"("State(s) in Front (\"\")"="SysConfig: Load Sys Config\nSysConfig: Load Digitizer Setting\nSysConfig: Load AB setting\nSysConfig: Load LJ Pinout\nSysConfig: Load 355 PWM\nSysConfig: LoadAPDSerialNumber\nSysConfig: LoadABVideoSetting\nSysConfig: LoadCursorLocation", "State(s) in (\"\")"=w537) -> ("States Out"=w536:string)  [unwired: 13 in]
      }
      frame "Macro: InitDeConAndClassifier" {
        # "Initilized realtime Decon and classifier if needed"
        n280 = Unbundle By Name(w539) -> ("OverlaySelection"=w538:u16)
        n281 = case shown="1, 2" w538 {
          tunnel: ["" ("State(s) in Front (\"\")") "DeconEngine: InitDotNet\nDeconEngine: loadIRF\nDeconEngine: Warmup\nClassifier: Init" ("State(s) in Front (\"\")")] -> w540
          frame 0, Default {
          }
          frame 1, 2 {
          }
        }
        n282 = call <vilib>:"Add State(s) to Queue__JKI_lib_State_Machine.vi"("State(s) in Front (\"\")"=w540, "State(s) in (\"\")"=w544) -> ("States Out"=w543:string)  [unwired: 13 in]
      }
      frame "Macro: SysReadyForAq" {
        # "Macro for system ready\n(It is a separator no-op. You can make a copy of this frame to create a new Macro frame)"
        n283 = call <vilib>:"Add State(s) to Queue__JKI_lib_State_Machine.vi"("State(s) in Front (\"\")"="UI: ReadyForAquisition\nLED: Green" ("State(s) in Front (\"\")"), "State(s) in (\"\")"=w552) -> ("States Out"=w551:string)  [unwired: 13 in]
      }
      frame "Macro: Exit" {
        # "close LJ last"
        # "check whether hardware is initilized, if so close, if not do nothing"
        # "Exit Macro, close all hardware\n(This is called once, when the VI exits)"
        n284 = Unbundle By Name(w574) -> ("System Status.Digitizer"=w570:bool, "System Status.Aiming Beam"=w569:bool, "System Status.355 Laser"=w568:bool, "System Status.Labjack"=w560:bool, "Core.Close Panel on Exit?"=w564:bool)
        n285 = local read ".NetInitialized?"() -> (w553:bool)
        n286 = case shown="True" w553 {
          tunnel: ["" "DeconEngine: CloseNetRef\nClassifier: Close"] -> w555
          frame False {
          }
          frame True {
          }
        }
        n287 = case shown="True" w560 {
          tunnel: ["" ("Empty String Constant") "LabJack: SetDefaultAndClose"] -> w557
          frame False {
          }
          frame True {
          }
        }
        n288 = case shown="True" w569 {
          tunnel: ["" ("Empty String Constant") "AimingBeam: Set ACC Status >> Disable\nAimingBeam: Close"] -> w559
          frame False {
          }
          frame True {
          }
        }
        n289 = case shown="True" w568 {
          tunnel: ["" ("Empty String Constant") "355 Laser: Close\n355 Laser: CheckControllerStatus"] -> w558
          frame False {
          }
          frame True {
          }
        }
        n290 = case shown="True" w570 {
          tunnel: ["" ("Empty String Constant") "Digitizer: Close"] -> w565
          frame False {
          }
          frame True {
          }
        }
        n291 = call <vilib>:"Add State(s) to Queue__JKI_lib_State_Machine.vi"("State(s) in Front (\"\")"="TCP: Close", "State(s) in (\"\")"=w555) -> ("States Out"=w554:string)  [unwired: 13 in]
        n292 = Select(t="UI: Front Panel State >> Close", s=w564, f="" ("Empty String Constant")) -> (s? t:f=w561:string)
        n293 = call <vilib>:"Add State(s) to Queue__JKI_lib_State_Machine.vi"("State(s) in Front (\"\")"=w554, "State(s) in (\"\")"=w565, "State(s) at Back (\"\")"=w559) -> ("States Out"=w567:string)  [unwired: 12 in]
        n294 = call <vilib>:"Add State(s) to Queue__JKI_lib_State_Machine.vi"("State(s) in Front (\"\")"=w567, "State(s) in (\"\")"=w558, "State(s) at Back (\"\")"=w557) -> ("States Out"=w563:string)  [unwired: 12 in]
        n295 = call <vilib>:"Add State(s) to Queue__JKI_lib_State_Machine.vi"("State(s) in Front (\"\")"=w563, "State(s) in (\"\")"="UI: Update\nUI: Reset\nGraph: SaveCursorLoc\nLED: CloseVIRef\nQueue: Destory\nData: Cleanup\nExit", "State(s) at Back (\"\")"=w561) -> ("States Out"=w571:string)  [unwired: 12 in]
        n296 = call <vilib>:"Add State(s) to Queue__JKI_lib_State_Machine.vi"("State(s) in Front (\"\")"=w571, "State(s) in (\"\")"=w577) -> ("States Out"=w576:string)  [unwired: 13 in]
      }
      frame "---------- Data ----------" {
        # "Do not put any code in this frame.\n(It is a separator no-op. You can make a copy of this frame to create a new Data frame)"
        n297 = call <vilib>:"Add State(s) to Queue__JKI_lib_State_Machine.vi"("State(s) in (\"\")"=w592) -> ("States Out"=w591:string)  [unwired: 14 in]
      }
      frame "Data: Initialize" {
        w593 = u16 0  # OverlaySelection
        w594 = path ""  # CaliPath
        w595 = dbl[] []  # V4
        w596 = dbl[][] []  # Ch4Data
        w597 = FALSE  # bothVidSourceAvail
        w598 = T1 {"Main Frame Grabber"=FALSE, "Side Frame Grabber"=FALSE, "Main Camera"=FALSE, "Side Camera"=FALSE}  # video source
        w599 = FALSE  # LED vi ref open?
        w601 = T23 {"DeCon Channel"=enum."1", "Scale Bar"=FALSE, "Scale Low"=3.0, "Scale High"=8.0, "ANSI"=20.0, "Radius"=1.0, "3D?"=FALSE, "Firefly?"=FALSE, "Pentero?"=FALSE}  # VideoConfig
        w602 = T27 {"Ch1APDSerial#"="", "Ch2APDSerial#"="", "Ch3APDSerial#"="", "Ch4APDSerial#"=""}  # APDSerialNum
        w603 = u32 0  # Aquisition Timer
        w604 = cluster{"RunID":i8, "BG ID":i8, "Cali ID":i8} {"RunID"=1, "BG ID"=1, "Cali ID"=1}  # IDs
        w605 = refnum<vi> refnum  # LED vi reference
        w606 = path ""  # TempPath
        w607 = T28 {"DataPath"=path "", "BG Path"=path "", "iRFPath"=path "", "CaliPath"=path ""}  # Pathes
        w609 = dbl[] []  # V3
        w610 = dbl[] []  # V2
        w611 = dbl[] []  # V1
        w613 = u32 0  # FastTimer
        w614 = u32 0  # SlowTimer
        w615 = dbl[][] []  # Ch3Data
        w616 = dbl[][] []  # Ch2Data
        w600 = dbl[][] []  # Ch1Data
        w619 = T2 {"Digitizer"=FALSE, "Labjack"=FALSE, "Aiming Beam"=FALSE, "355 Laser"=FALSE, "TCP/IP"=FALSE}  # System Status
        w620 = T29 {"DIO_EF_CLOCK1_DIVISOR"=16, "DIO_EF_CLOCK1_ROLL_VALUE"=25000, "DIO#_EF_INDEX"=0, "DIO#_EF_OPTIONS"=1, "DIO#_EF_CONFIG_A"=6250}  # AB PWM setting
        w621 = T4 {"Ch1 Bias"="TDA11", "Ch2 Bias"="DAC10", "Ch3 Bias"="DAC0", "355 PWM"="FIO0", "AimingBeam PWM"="FIO2", "Laser Ready"="FIO3", "Interlock"="FIO1", "Laser Start/Stop"="FIO1", "Red LED"="FIO1", "Green LED"="FIO1", "Foot Pedal"="DIO15"}  # LJ Pinout
        w622 = 0  # TCP attempt count
        w623 = u32 0  # Laser start tic
        w624 = refnum<k20>[] []  # niTClk sessions
        w625 = u32 0  # Last Trigger
        w626 = T29 {"DIO_EF_CLOCK1_DIVISOR"=16, "DIO_EF_CLOCK1_ROLL_VALUE"=25000, "DIO#_EF_INDEX"=0, "DIO#_EF_OPTIONS"=1, "DIO#_EF_CONFIG_A"=6250}  # 355 PWM setting
        w627 = T30 {"Aiming Beam COM Port"="COM3", "Min Current"=0.0, "Max Current"=63.0, "Default Current"=20.0, "Freq"=0}  # AB Cluster
        w628 = T31 {"resource name"="", "resource name 2"="", "Channel"=enum."Channel 0", "trigger source"="VAL_EXTERNAL", "trigger level"=0.5, "trigger delay"=1.35e-07, "min sample rate"=12500000000.0, "min record length"=2500, "vertical range"=1.0, "vertical offset"=-0.25, "Waveform to Avg"=2000}  # FLImDAQ
        w629 = FALSE  # SysRunning?
        w617 = path ""  # DefaultPath
        w630 = ""  # CaseID
        w631 = T7 {"Ch1Enable?"=FALSE, "Ch2Enable?"=FALSE, "Ch3Enable?"=FALSE, "Ch1AutoGain?"=FALSE, "Ch2AutoGain?"=FALSE, "Ch3AutoGain?"=FALSE, "AimingBeamEnable?"=FALSE}  # SysConfigCluster
        w632 = T32 {"Current VI Reference"=refnum, "Close Panel on Exit?"=FALSE}  # Core
        # "Initialize the shift-register data, here.\n(data names are defined by what you wire into the bundle function)"
        n298 = Bundle("Core"=w632, "SysConfigCluster"=w631, "System Status"=w619, "IDs"=w604, "CaseID"=w630, "DefaultPath"=w617, "Pathes"=w607, "FLImDAQ"=w628, "SysRunning?"=w629, "AB Cluster"=w627, "LJ Pinout"=w621, "355 PWM setting"=w626, "AB PWM setting"=w620, "Last Trigger"=w625, "niTClk sessions"=w624, "Laser start tic"=w623, "TCP attempt count"=w622, "Ch1Data"=w600, "Ch2Data"=w616, "Ch3Data"=w615, "Ch4Data"=w596, "V1"=w611, "V2"=w610, "V3"=w609, "V4"=w595, "SlowTimer"=w614, "FastTimer"=w613, "listener ID"=refnum<k5> refnum, "TempPath"=w606, "CaliPath"=w594, "LED vi reference"=w605, "Aquisition Timer"=w603, "APDSerialNum"=w602, "VideoConfig"=w601, "LED vi ref open?"=w599, "video source"=w598, "bothVidSourceAvail"=w597, "OverlaySelection"=w593) -> (w608:T24)  [unwired: 1 in]
        n299 = call <vilib>:"Add State(s) to Queue__JKI_lib_State_Machine.vi"("State(s) in (\"\")"=w635) -> ("States Out"=w634:string)  [unwired: 14 in]
      }
      frame "Data: loadLastUseMacro" {
        # "Load last use BG and Cali and iRF.\n(It is a separator no-op. You can make a copy of this frame to create a new Data frame)"
        n300 = call <vilib>:"Add State(s) to Queue__JKI_lib_State_Machine.vi"("State(s) in Front (\"\")"="Data: loadLastUseBG\nData: LoadRealtimeDeConBG\nData: loadSystemCali\nData: loadLastUseiRF\n/*Data: LoadiRFFromAPDFile\nUI: CaliAndiRFLoaded\nData: ShowiRF" ("State(s) in Front (\"\")"), "State(s) in (\"\")"=w641) -> ("States Out"=w640:string)  [unwired: 13 in]
      }
      frame "Data: loadLastUseBG" {
        w645 = enum16{"write", "read"}."write" ("action")
        # "Load last use BG.\n()"
        n301 = Unbundle By Name(w664) -> ("TempPath"=w663:path)
        n302 = call "FLImDAQ_FGV.vi"() -> ("Read data"=w659:T5)  [unwired: 10 in, 1 out]
        n303 = Build Path(base path=w663, name or relative path="Background.tdms") -> (appended path=w662:path)
        n304 = call "ReadBGorCali (SubVI).vi"("DataType"=enum16{"BG", "Cali"}."BG", "error in (no error)"=w661, "file path in"=w662) -> ("error out"=w660:errorcluster, "AvgDataCluster"=w655:T33)  [unwired: 6 in, 1 out]
        n305 = Unbundle By Name(w655) -> ("Channel 1"=w642:dbl[], "Channel 2"=w654:dbl[], "Channel 3"=w647:dbl[], "Channel 4"=w644:dbl[])
        n306 = Unbundle By Name(w659) -> ("min record length"=w651:i32)
        n307 = Array Size(array=w642) -> (size(s)=w653:i32)
        "BG length" <- w653
        n308 = Equal?(x=w653, y=w651) -> (x = y?=w652:bool)
        n309 = Select(t="UI: BGLoaded" ("State(s) in Front (\"\")"), s=w652, f="UI: BGSizeError" ("State(s) in Front (\"\")")) -> (s? t:f=w656:string)
        n310 = case shown="True" w652 {
          tunnel: w642 -> [_ w675]
          tunnel: w654 -> [_ w674]
          tunnel: w647 -> [_ w673]
          tunnel: w651 -> [w670 _]
          tunnel: [w669 w675] -> w650
          tunnel: [w669 w674] -> w649
          tunnel: [w669 w673] -> w648
          tunnel: w644 -> [_ w672]
          tunnel: [w669 w672] -> w643
          frame False {
            # "If error set BG all 0, update UI"
            n311 = for {
              N: w670 -> [_]
              tunnel: [0.0] -> w669 mode=indexing
            }
          }
          frame True {
            # "If no error, check size match"
          }
        }
        n312 = call "BG4FGV.vi"("action"=w645, "BG4 in"=w643) -> ()  [unwired: 8 in, 2 out]
        n313 = call "BG3FGV.vi"("action"=w645, "BG1 in"=w648) -> ()  [unwired: 8 in, 2 out]
        n314 = call "BG1FGV.vi"("action"=w645, "BG1 in"=w650) -> ()  [unwired: 8 in, 2 out]
        n315 = call "BG2FGV.vi"("action"=w645, "BG1 in"=w649) -> ()  [unwired: 8 in, 2 out]
        n316 = call <vilib>:"Add State(s) to Queue__JKI_lib_State_Machine.vi"("State(s) in Front (\"\")"=w656, "State(s) in (\"\")"=w668) -> ("States Out"=w667:string)  [unwired: 13 in]
      }
      frame "Data: LoadRealtimeDeConBG" {
        # "Load saved realtime DeCon BG from Temp file"
        n317 = Unbundle By Name(w690) -> ("TempPath"=w689:path)
        n318 = Build Path(base path=w689, name or relative path="RealTimeDeConBGTemp.tdms") -> (appended path=w687:path)
        n319 = TDMS Open(8:w685, 10:T16."open" ("operation (0:open)"), 11:w687) -> (0:w682:errorcluster, 3:w684:refnum<k34>)  [unwired: 4 in]
        n320 = TDMS Read(0:w684, 5:"Realtime DeCon BG" ("group name in (Untitled)"), 7:string[] ["Ch1", "Ch2", "Ch3"], 11:w682, 12:dbl[][] [] ("BGAll")) -> (4:w680:refnum<k34>, 10:w676:dbl[][], 15:w679:errorcluster)  [unwired: 3 in, 3 out]
        n321 = local write "BGAll"(w676) -> ()
        n322 = TDMS Close(8:w679, 11:w680) -> (0:w678:errorcluster)  [unwired: 1 out]
        n323 = local write "BG Graph"(w676) -> ()
        n324 = call <vilib>:"Add State(s) to Queue__JKI_lib_State_Machine.vi"("State(s) in (\"\")"=w693) -> ("States Out"=w692:string)  [unwired: 14 in]
      }
      frame "Data: loadSystemCali" {
        # "Load last use calibration.\n()"
        n325 = Unbundle By Name(w701) -> ("CaliPath"=w700:path)
        n326 = Build Path(base path=w700, name or relative path="Calibration.tdms") -> (appended path=w696:path)
        n327 = call "ReadBGorCali (SubVI).vi"("DataType"=enum16{"BG", "Cali"}."Cali", "error in (no error)"=w695, "file path in"=w696) -> ("error out"=w697:errorcluster, "CtrlVCluster"=w699:cluster{"V 1":dbl[], "V 2":dbl[], "V 3":dbl[]}, "AvgDataCluster"=w698:T33)  [unwired: 6 in]
        n328 = case shown="No Error" w697 {
          tunnel: w699 -> [w720 _]
          tunnel: w698 -> [w719 _]
          frame No Error {
            w710 = T34 {"Ch1 WF"=[], "Ch2 WF"=[], "Ch3 WF"=[], "Ch4 WF"=[], "V1"=0.0, "V2"=0.0, "V3"=0.0, "V4"=0.0}  # SysCaliData
            n329 = Unbundle By Name(w719) -> ("Channel 1"=w718:dbl[], "Channel 2"=w717:dbl[], "Channel 3"=w716:dbl[], "Channel 4"=w709:dbl[])
            n330 = Unbundle By Name(w720) -> ("V 1"=w715:dbl[], "V 2"=w714:dbl[], "V 3"=w708:dbl[], "V 4"=w706:dbl[])
            n331 = Index Array(array=w715) -> (element=w713:dbl)  [unwired: 1 in]
            n332 = Index Array(array=w714) -> (element=w712:dbl)  [unwired: 1 in]
            n333 = Index Array(array=w708) -> (element=w711:dbl)  [unwired: 1 in]
            n334 = Index Array(array=w706) -> (element=w707:dbl)  [unwired: 1 in]
            n335 = Bundle By Name(cluster=w710, "Ch1 WF"=w718, "Ch2 WF"=w717, "Ch3 WF"=w716, "Ch4 WF"=w709, "V1"=w713, "V2"=w712, "V3"=w711, "V4"=w707) -> (w721:T34)
            n336 = global write "GlobalVariables.vi" "SysCaliData"(w721) -> ()
          }
          frame Error {
          }
        }
        n337 = call <vilib>:"Add State(s) to Queue__JKI_lib_State_Machine.vi"("State(s) in (\"\")"=w705) -> ("States Out"=w704:string)  [unwired: 14 in]
      }
      frame "Data: LoadiRFFromAPDFile" {
        w751 = T17 {"Ch1 iRF"=[], "Ch2 iRF"=[], "Ch3 iRF"=[], "Ch4 iRF"=[]}  # LastUseiRF
        # "only load the last 5th  iRF for the moment"
        # "Load APD detector data\n(It is a separator no-op. You can make a copy of this frame to create a new Data frame)"
        n338 = Unbundle By Name(w773) -> ("APDSerialNum.Ch1APDSerial#"=w772:string, "APDSerialNum.Ch2APDSerial#"=w753:string, "APDSerialNum.Ch3APDSerial#"=w752:string, "APDSerialNum.Ch4APDSerial#"=w749:string)
        n339 = call "CreatFromSerialNumNoRaw.vi"("error in (no error)"=w750, "APD Serial #"=w772) -> ("error out"=w770:errorcluster, "APDClass out"=w771:refnum<class "APDClass.lvclass">)  [unwired: 8 in]
        n340 = call "CreatFromSerialNumNoRaw.vi"("error in (no error)"=w750, "APD Serial #"=w753) -> ("error out"=w761:errorcluster, "APDClass out"=w762:refnum<class "APDClass.lvclass">)  [unwired: 8 in]
        n341 = call "CreatFromSerialNumNoRaw.vi"("error in (no error)"=w750, "APD Serial #"=w752) -> ("error out"=w755:errorcluster, "APDClass out"=w756:refnum<class "APDClass.lvclass">)  [unwired: 8 in]
        n342 = call "CreatFromSerialNumNoRaw.vi"("error in (no error)"=w750, "APD Serial #"=w749) -> ("error out"=w747:errorcluster, "APDClass out"=w748:refnum<class "APDClass.lvclass">)  [unwired: 8 in]
        n343 = call-dynamic "Read iRFData.vi"("error in (no error)"=w770, "APDClass in"=w771) -> ("iRFData"=w769:T35)  [unwired: 7 in, 2 out]
        n344 = call-dynamic "Read iRFData.vi"("error in (no error)"=w761, "APDClass in"=w762) -> ("iRFData"=w765:T35)  [unwired: 7 in, 2 out]
        n345 = call-dynamic "Read iRFData.vi"("error in (no error)"=w755, "APDClass in"=w756) -> ("iRFData"=w759:T35)  [unwired: 7 in, 2 out]
        n346 = call-dynamic "Read iRFData.vi"("error in (no error)"=w747, "APDClass in"=w748) -> ("iRFData"=w746:T35)  [unwired: 7 in, 2 out]
        n347 = Unbundle By Name(w769) -> ("iRFWFsAvg"=w768:dbl[][])
        n348 = Unbundle By Name(w765) -> ("iRFWFsAvg"=w764:dbl[][])
        n349 = Unbundle By Name(w759) -> ("iRFWFsAvg"=w758:dbl[][])
        n350 = Unbundle By Name(w746) -> ("iRFWFsAvg"=w743:dbl[][])
        n351 = Array Size(array=w768) -> (size(s)=w767:i32[])
        n352 = Array Size(array=w764) -> (size(s)=w760:i32[])
        n353 = Array Size(array=w758) -> (size(s)=w754:i32[])
        n354 = Array Size(array=w743) -> (size(s)=w744:i32[])
        n355 = Index Array(array=w767, index=0) -> (element=w742:i32)
        n356 = Index Array(array=w760, index=0) -> (element=w738:i32)
        n357 = Index Array(array=w754, index=0) -> (element=w735:i32)
        n358 = Index Array(array=w744, index=0) -> (element=w732:i32)
        n359 = Subtract(x=w742, y=5) -> (x-y=w740:i32)
        n360 = Subtract(x=w738, y=5) -> (x-y=w737:i32)
        n361 = Subtract(x=w735, y=5) -> (x-y=w734:i32)
        n362 = Subtract(x=w732, y=5) -> (x-y=w731:i32)
        n363 = Index Array(array=w768, index (row)=w740) -> (element=w730:dbl[])  [unwired: 1 in]
        n364 = Index Array(array=w764, index (row)=w737) -> (element=w729:dbl[])  [unwired: 1 in]
        n365 = Index Array(array=w758, index (row)=w734) -> (element=w728:dbl[])  [unwired: 1 in]
        n366 = Index Array(array=w743, index (row)=w731) -> (element=w727:dbl[])  [unwired: 1 in]
        n367 = call "DownSampleAndShiftiRF (SubVI).vi"("ArrayIn"=w730) -> ("ArrayOut"=w726:dbl[])  [unwired: 10 in]
        n368 = call "DownSampleAndShiftiRF (SubVI).vi"("ArrayIn"=w729) -> ("ArrayOut"=w722:dbl[])  [unwired: 10 in]
        n369 = call "DownSampleAndShiftiRF (SubVI).vi"("ArrayIn"=w728) -> ("ArrayOut"=w723:dbl[])  [unwired: 10 in]
        n370 = call "DownSampleAndShiftiRF (SubVI).vi"("ArrayIn"=w727) -> ("ArrayOut"=w725:dbl[])  [unwired: 10 in]
        n371 = call <vilib>:"Add State(s) to Queue__JKI_lib_State_Machine.vi"("State(s) in (\"\")"=w776) -> ("States Out"=w775:string)  [unwired: 14 in]
        n372 = Bundle(cluster=w751, "Ch1 iRF"=w726, "Ch2 iRF"=w722, "Ch3 iRF"=w723, "Ch4 iRF"=w725) -> (w724:T17)
        n373 = global write "GlobalVariables.vi" "LastUseiRF"(w724) -> ()
      }
      frame "Data: loadLastUseiRF" {
        # "Load last use iRF.\n()"
        n374 = Unbundle By Name(w782) -> ("TempPath"=w781:path)
        n375 = Build Path(base path=w781, name or relative path="iRF.tdms") -> (appended path=w787:path)
        n376 = TDMS Open(8:w777, 11:w787) -> (0:w785:errorcluster, 3:w786:refnum<k34>)  [unwired: 5 in]
        n377 = TDMS Read(0:w786, 11:w785, 12:dbl[][] []) -> (4:w780:refnum<k34>, 10:w783:dbl[][], 15:w779:errorcluster)  [unwired: 5 in, 3 out]
        n378 = TDMS Close(8:w779, 11:w780) -> (0:w778:errorcluster)  [unwired: 1 out]
        n379 = case shown="No Error" w779 {
          tunnel: w783 -> [w797 _]
          frame No Error {
            w800 = T17 {"Ch1 iRF"=[], "Ch2 iRF"=[], "Ch3 iRF"=[], "Ch4 iRF"=[]}  # LastUseiRF
            n380 = Index Array(array=w797, index (row)=0) -> (element=w792:dbl[])  [unwired: 1 in]
            n381 = Index Array(array=w797, index (row)=1) -> (element=w793:dbl[])  [unwired: 1 in]
            n382 = Index Array(array=w797, index (row)=2) -> (element=w794:dbl[])  [unwired: 1 in]
            n383 = Index Array(array=w797, index (row)=3) -> (element=w795:dbl[])  [unwired: 1 in]
            n384 = Add Array Elements(numeric array=w792) -> (sum=w806:dbl)
            n385 = Add Array Elements(numeric array=w793) -> (sum=w804:dbl)
            n386 = Add Array Elements(numeric array=w794) -> (sum=w802:dbl)
            n387 = Add Array Elements(numeric array=w795) -> (sum=w798:dbl)
            n388 = Divide(x=w792, y=w806) -> (x/y=w805:dbl[])
            n389 = Divide(x=w793, y=w804) -> (x/y=w803:dbl[])
            n390 = Divide(x=w794, y=w802) -> (x/y=w801:dbl[])
            n391 = Divide(x=w795, y=w798) -> (x/y=w796:dbl[])
            n392 = Bundle(cluster=w800, "Ch1 iRF"=w805, "Ch2 iRF"=w803, "Ch3 iRF"=w801, "Ch4 iRF"=w796) -> (w808:T17)
            n393 = Array Size(array=w792) -> (size(s)=→"iRF length":i32)
            n394 = global write "GlobalVariables.vi" "LastUseiRF"(w808) -> ()
          }
          frame Error {
          }
        }
        n395 = call <vilib>:"Add State(s) to Queue__JKI_lib_State_Machine.vi"("State(s) in (\"\")"=w791) -> ("States Out"=w790:string)  [unwired: 14 in]
      }
      frame "Data: ShowiRF" {
        # "Show loaded iRF.\n(It is a separator no-op. You can make a copy of this frame to create a new Data frame)"
        n396 = global read "GlobalVariables.vi" "LastUseiRF"() -> (w817:T36)
        n397 = Unbundle By Name(w817) -> ("Ch1 iRF"=w816:dbl[], "Ch2 iRF"=w815:dbl[], "Ch3 iRF"=w814:dbl[], "Ch4 iRF"=w813:dbl[])
        n398 = Build Array(w816, w815, w814, w813) -> (→"iRF Graph":dbl[][])
        n399 = call <vilib>:"Add State(s) to Queue__JKI_lib_State_Machine.vi"("State(s) in (\"\")"=w822) -> ("States Out"=w821:string)  [unwired: 14 in]
      }
      frame "Data: saveCalibration" {
        # "Average data and save calibration file. [Covers: REQ11]\n(It is a separator no-op. You can make a copy of this frame to create a new Data frame)"
        n400 = Unbundle By Name(w841) -> ("Ch1Data"=w840:dbl[][], "V1"=w839:dbl[], "Ch2Data"=w838:dbl[][], "V2"=w837:dbl[], "Ch3Data"=w836:dbl[][], "V3"=w835:dbl[], "Ch4Data"=w826:dbl[][], "V4"=w825:dbl[], "Pathes.CaliPath"=w844:path, "IDs.Cali ID"=w843:i8)
        n401 = Increment(x=w843) -> (x+1=w827:i8)
        n402 = Bundle("Ch1Data"=w840, "V1"=w839) -> (w834:cluster{"Ch1Data":dbl[][], "V1":dbl[]})  [unwired: 1 in]
        n403 = Bundle("Ch4Data"=w826, "V4"=w825) -> (w824:cluster{"Ch4Data":dbl[][], "V4":dbl[]})  [unwired: 1 in]
        n404 = Bundle("Ch2Data"=w838, "V2"=w837) -> (w833:cluster{"Ch2Data":dbl[][], "V2":dbl[]})  [unwired: 1 in]
        n405 = Bundle("Ch3Data"=w836, "V3"=w835) -> (w832:cluster{"Ch3Data":dbl[][], "V3":dbl[]})  [unwired: 1 in]
        n406 = Format Value(string ("")="Calibration" ("default name"), format string="%02d", value (0)=w827) -> (output string=w846:string)
        n407 = Build Path(base path=w844, name or relative path=w846) -> (appended path=w831:path)
        n408 = call "SaveBGorCali(SubVI).vi"("Channel1"=w834, "BG path"=w831, "DataType"=enum16{"BG", "Cali"}."Cali", "Channel 2"=w833, "Channel 3"=w832, "Channel 4"=w824, "error in (no error)"=w830, "SytemID"="UCDVetMed") -> ("error out"=w829:errorcluster)  [unwired: 7 in]
        n409 = call <vilib>:"Add State(s) to Queue__JKI_lib_State_Machine.vi"("State(s) in (\"\")"=w849) -> ("States Out"=w848:string)  [unwired: 14 in]
      }
      frame "Data: saveiRF" {
        w855 = enum16{"write", "read"}."read" ("action")
        # "Get iRF from decon stracture and save it on disk.\n(It is a separator no-op. You can make a copy of this frame to create a new Data frame)"
        n410 = Unbundle By Name(w872) -> ("TempPath"=w871:path)
        n411 = call "Ch1DeconEngineFGV.vi"("action(read)"=w855) -> ("Error Out"=w877:errorcluster, "Ch1DeconEngine out"=w878:refnum<class "LaguerreDeconEngineClass.lvclass">)  [unwired: 9 in]
        n412 = call "Ch2DeconEngineFGV.vi"("action(read)"=w855) -> ("Error Out"=w875:errorcluster, "Ch2DeconEngine out"=w876:refnum<class "LaguerreDeconEngineClass.lvclass">)  [unwired: 9 in]
        n413 = call "Ch3DeconEngineFGV.vi"("action(read)"=w855) -> ("Error Out"=w873:errorcluster, "Ch3DeconEngine out"=w874:refnum<class "LaguerreDeconEngineClass.lvclass">)  [unwired: 9 in]
        n414 = call "Ch4DeconEngineFGV.vi"("action(read)"=w855) -> ("Error Out"=w854:errorcluster, "Ch3DeconEngine out"=w853:refnum<class "LaguerreDeconEngineClass.lvclass">)  [unwired: 9 in]
        n415 = Build Path(base path=w871, name or relative path="iRF" ("default name")) -> (appended path=w869:path)
        n416 = call "getIRF.vi"("error in (no error)"=w854, "LaguerreDeconEngineClass in"=w853) -> ("iRF"=w852:dbl[])  [unwired: 7 in, 2 out]
        n417 = call "getIRF.vi"("error in (no error)"=w877, "LaguerreDeconEngineClass in"=w878) -> ("iRF"=w860:dbl[])  [unwired: 7 in, 2 out]
        n418 = call "getIRF.vi"("error in (no error)"=w875, "LaguerreDeconEngineClass in"=w876) -> ("iRF"=w859:dbl[])  [unwired: 7 in, 2 out]
        n419 = call "getIRF.vi"("error in (no error)"=w873, "LaguerreDeconEngineClass in"=w874) -> ("iRF"=w858:dbl[])  [unwired: 7 in, 2 out]
        n420 = TDMS Open(8:w868, 10:T16."create or replace" ("operation (0:open)"), 11:w869) -> (0:w865:errorcluster, 3:w866:refnum<k34>)  [unwired: 4 in]
        n421 = Bundle(cluster=T17 {"Ch1 iRF"=[], "Ch2 iRF"=[], "Ch3 iRF"=[], "Ch4 iRF"=[]} ("LastUseiRF"), "Ch1 iRF"=w860, "Ch2 iRF"=w859, "Ch3 iRF"=w858, "Ch4 iRF"=w852) -> (w856:T17)
        n422 = Build Array(w860, w859, w858, w852) -> (w864:dbl[][])
        n423 = global write "GlobalVariables.vi" "LastUseiRF"(w856) -> ()
        n424 = TDMS Write(0:w866, 5:"iRF" ("group name in (Untitled)"), 7:string[] ["Ch1", "Ch2", "Ch3", "Ch4"] ("channel name(s) in (Untitled)"), 9:w864, 11:w865) -> (4:w863:refnum<k34>, 15:w862:errorcluster)  [unwired: 1 in, 2 out]
        n425 = TDMS Close(8:w862, 11:w863) -> (0:w861:errorcluster)  [unwired: 1 out]
        n426 = call <vilib>:"Add State(s) to Queue__JKI_lib_State_Machine.vi"("State(s) in (\"\")"=w881) -> ("States Out"=w880:string)  [unwired: 14 in]
      }
      frame "Data: saveBGtoFGV" {
        w896 = enum16{"write", "read"}."write" ("action")
        # "Save BG and pass it to FGV.\n(save BG to disk and set it to FGV)"
        n427 = Unbundle By Name(w897) -> ("Ch1Data"=w890:dbl[][], "Ch2Data"=w888:dbl[][], "Ch3Data"=w886:dbl[][], "Ch4Data"=w884:dbl[][])
        n428 = call "AvgArrayTimeCritical.vi"("2D array"=w888) -> ("1D Avg"=w887:dbl[])  [unwired: 10 in]
        n429 = call "AvgArrayTimeCritical.vi"("2D array"=w886) -> ("1D Avg"=w885:dbl[])  [unwired: 10 in]
        n430 = call "AvgArrayTimeCritical.vi"("2D array"=w890) -> ("1D Avg"=w889:dbl[])  [unwired: 10 in]
        n431 = call "AvgArrayTimeCritical.vi"("2D array"=w884) -> ("1D Avg"=w883:dbl[])  [unwired: 10 in]
        n432 = call "BG1FGV.vi"("Error In"=w882, "action"=w896, "BG1 in"=w889) -> ("Error Out"=w895:errorcluster)  [unwired: 7 in, 1 out]
        n433 = call "BG2FGV.vi"("Error In"=w882, "action"=w896, "BG1 in"=w887) -> ("Error Out"=w894:errorcluster)  [unwired: 7 in, 1 out]
        n434 = call "BG3FGV.vi"("Error In"=w882, "action"=w896, "BG1 in"=w885) -> ("Error Out"=w893:errorcluster)  [unwired: 7 in, 1 out]
        n435 = call "BG4FGV.vi"("Error In"=w882, "action"=w896, "BG4 in"=w883) -> ("Error Out"=w892:errorcluster)  [unwired: 7 in, 1 out]
        n436 = Merge Errors(w895, w894, w893, w892) -> (w891:errorcluster)
        n437 = call <vilib>:"Add State(s) to Queue__JKI_lib_State_Machine.vi"("State(s) in (\"\")"=w900) -> ("States Out"=w899:string)  [unwired: 14 in]
      }
      frame "Data: saveBGtoFile" {
        w922 = "Background" ("name or relative path")
        # "Save BG to file.\n(save BG to disk both data folder and temp folder)"
        n438 = Unbundle By Name(w926) -> ("Pathes.BG Path"=w919:path, "IDs.BG ID"=w918:i8, "Ch1Data"=w916:dbl[][], "V1"=w915:dbl[], "Ch2Data"=w914:dbl[][], "V2"=w913:dbl[], "Ch3Data"=w912:dbl[][], "V3"=w911:dbl[], "Ch4Data"=w903:dbl[][], "V4"=w902:dbl[], "TempPath"=w924:path)
        n439 = Increment(x=w918) -> (x+1=w923:i8)
        n440 = Format Value(string ("")=w922, format string="%02d", value (0)=w923) -> (output string=w921:string)
        n441 = Build Path(base path=w924, name or relative path=w922) -> (appended path=w905:path)
        n442 = call "File Dialog2"("start path"=w919, "prompt"="Please select BG name, DO NOT CANCEL!", "default name"=w921) -> ("selected path"=w906:path)  [unwired: 9 in, 3 out]
        n443 = Bundle("Ch1Data"=w916, "V1"=w915) -> (w910:cluster{"Ch1Data":dbl[][], "V1":dbl[]})  [unwired: 1 in]
        n444 = Bundle("Ch4Data"=w903, "V4"=w902) -> (w901:cluster{"Ch4Data":dbl[][], "V4":dbl[]})  [unwired: 1 in]
        n445 = Bundle("Ch2Data"=w914, "V2"=w913) -> (w909:cluster{"Ch2Data":dbl[][], "V2":dbl[]})  [unwired: 1 in]
        n446 = Bundle("Ch3Data"=w912, "V3"=w911) -> (w908:cluster{"Ch3Data":dbl[][], "V3":dbl[]})  [unwired: 1 in]
        n447 = Build Array(w906, w905) -> (w904:path[])
        n448 = for {
          tunnel: w910 -> [w937]
          tunnel: w909 -> [w936]
          tunnel: w908 -> [w935]
          shift-right: [w938] -> w917
          shift-left: w907 -> [w934]
          tunnel: w904 -> [w933] mode=indexing
          tunnel: w901 -> [w931]
          n449 = call "SaveBGorCali(SubVI).vi"("Channel1"=w937, "BG path"=w933, "DataType"=enum16{"BG", "Cali"}."BG", "Channel 2"=w936, "Channel 3"=w935, "Channel 4"=w931, "error in (no error)"=w934, "SytemID"="UCDMC") -> ("error out"=w938:errorcluster)  [unwired: 7 in]
        }
        n450 = call <vilib>:"Add State(s) to Queue__JKI_lib_State_Machine.vi"("State(s) in (\"\")"=w929) -> ("States Out"=w928:string)  [unwired: 14 in]
      }
      frame "Data: processDeConBG" {
        # "Save BG and pass it to FGV.\n(save BG to disk and set it to FGV)"
        n451 = call "DotNetFGV.vi"("Error In"=w950) -> ("Error Out"=w951:errorcluster, "reference out"=w952:refnum<k24>)  [unwired: 9 in]
        n452 = Unbundle By Name(w956) -> ("Ch1Data"=w945:dbl[][], "Ch2Data"=w943:dbl[][], "Ch3Data"=w944:dbl[][])  [unwired: 1 out]
        n453 = Transpose 2D Array(2D array=w945) -> (transposed array=w955:dbl[][])
        n454 = Transpose 2D Array(2D array=w943) -> (transposed array=w954:dbl[][])
        n455 = Transpose 2D Array(2D array=w944) -> (transposed array=w953:dbl[][])
        n456 = call "WaveformTUA(SubVI).vi"("error in (no error)"=w951, "WF in"=w955, "new reference"=w952) -> ("error out"=w942:errorcluster, "WF out"=w946:dbl[])  [unwired: 6 in, 1 out]
        n457 = call "WaveformTUA(SubVI).vi"("error in (no error)"=w951, "WF in"=w954, "new reference"=w952) -> ("error out"=w941:errorcluster, "WF out"=w948:dbl[])  [unwired: 6 in, 1 out]
        n458 = call "WaveformTUA(SubVI).vi"("error in (no error)"=w951, "WF in"=w953, "new reference"=w952) -> ("error out"=w940:errorcluster, "WF out"=w947:dbl[])  [unwired: 6 in, 1 out]
        n459 = Build Array(w946, w948, w947) -> (→"BGAll" →"BG Graph":dbl[][])
        n460 = Merge Errors(w942, w941, w940) -> (w949:errorcluster)
        n461 = call <vilib>:"Add State(s) to Queue__JKI_lib_State_Machine.vi"("State(s) in (\"\")"=w959) -> ("States Out"=w958:string)  [unwired: 14 in]
      }
      frame "Data: saveDeConBGtoFile" {
        # "Save realtime DeCon BG to temp file.\n(It is a separator no-op. You can make a copy of this frame to create a new Data frame)"
        n462 = Unbundle By Name(w973) -> ("TempPath"=w972:path)
        n463 = Build Path(base path=w972, name or relative path="RealTimeDeConBGTemp") -> (appended path=w970:path)
        n464 = local read "BGAll"() -> (w966:dbl[][])
        n465 = TDMS Open(8:w968, 10:T16."create or replace" ("operation (0:open)"), 11:w970) -> (0:w965:errorcluster, 3:w967:refnum<k34>)  [unwired: 4 in]
        n466 = TDMS Write(0:w967, 5:"Realtime DeCon BG" ("group name in (Untitled)"), 7:string[] ["Ch1", "Ch2", "Ch3"], 9:w966, 11:w965) -> (4:w962:refnum<k34>, 15:w961:errorcluster)  [unwired: 1 in, 2 out]
        n467 = TDMS Close(8:w961, 11:w962) -> (0:w960:errorcluster)  [unwired: 1 out]
        n468 = call <vilib>:"Add State(s) to Queue__JKI_lib_State_Machine.vi"("State(s) in (\"\")"=w976) -> ("States Out"=w975:string)  [unwired: 14 in]
      }
      frame "Data: showBG" {
        # "Show BG in seperate window.\n()"
        n469 = call "showBG.vi"() -> ()  [unwired: 12 in]
        n470 = call <vilib>:"Add State(s) to Queue__JKI_lib_State_Machine.vi"("State(s) in (\"\")"=w981) -> ("States Out"=w980:string)  [unwired: 14 in]
      }
      frame "Data: irfAlignment" {
        w982 = enum16{"write", "read"}."write" ("action")
        # "do iRF alignment in this state\n(It is a separator no-op. You can make a copy of this frame to create a new Data frame)"
        n471 = Unbundle By Name(w1027) -> ("Ch1Data"=w1063:dbl[][], "Ch2Data"=w1062:dbl[][], "Ch3Data"=w1061:dbl[][], "Ch4Data"=w1004:dbl[][])
        n472 = call "Ch1DeconEngineFGV.vi"("Error In"=w1003) -> ("Error Out"=w1059:errorcluster, "Ch1DeconEngine out"=w1060:refnum<class "LaguerreDeconEngineClass.lvclass">)  [unwired: 9 in]
        n473 = call "Ch2DeconEngineFGV.vi"("Error In"=w1003) -> ("Error Out"=w1057:errorcluster, "Ch2DeconEngine out"=w1058:refnum<class "LaguerreDeconEngineClass.lvclass">)  [unwired: 9 in]
        n474 = call "Ch3DeconEngineFGV.vi"("Error In"=w1003) -> ("Error Out"=w1055:errorcluster, "Ch3DeconEngine out"=w1056:refnum<class "LaguerreDeconEngineClass.lvclass">)  [unwired: 9 in]
        n475 = call "Ch4DeconEngineFGV.vi"("Error In"=w1003) -> ("Error Out"=w994:errorcluster, "Ch3DeconEngine out"=w993:refnum<class "LaguerreDeconEngineClass.lvclass">)  [unwired: 9 in]
        n476 = call "AvgArray.vi"("2D array in"=w1062) -> ("1D Avg out"=w1009:dbl[])  [unwired: 10 in]
        n477 = call "AvgArray.vi"("2D array in"=w1061) -> ("1D Avg out"=w1008:dbl[])  [unwired: 10 in]
        n478 = call "AvgArray.vi"("2D array in"=w1004) -> ("1D Avg out"=w983:dbl[])  [unwired: 10 in]
        n479 = call "AvgArray.vi"("2D array in"=w1063) -> ("1D Avg out"=w1010:dbl[])  [unwired: 10 in]
        n480 = call "RemoveDCBG.vi"("WF in"=w1010) -> ("DC"=w1017:dbl, "WF out"=w1007:dbl[])  [unwired: 8 in, 1 out]
        n481 = call "RemoveDCBG.vi"("WF in"=w1009) -> ("DC"=w1014:dbl, "WF out"=w1020:dbl[])  [unwired: 8 in, 1 out]
        n482 = call "RemoveDCBG.vi"("WF in"=w1008) -> ("DC"=w1012:dbl, "WF out"=w1019:dbl[])  [unwired: 8 in, 1 out]
        n483 = call "RemoveDCBG.vi"("WF in"=w983) -> ("DC"=w987:dbl, "WF out"=w985:dbl[])  [unwired: 8 in, 1 out]
        n484 = call "computeIRFAlignment.vi"("error in (no error)"=w1059, "fIRF temp"=w1007, "LaguerreDeconEngineClass in"=w1060) -> ("error out"=w1051:errorcluster, "LaguerreDeconEngineClass out"=w1052:refnum<class "LaguerreDeconEngineClass.lvclass">)  [unwired: 6 in, 1 out]
        n485 = call "computeIRFAlignment.vi"("error in (no error)"=w1057, "fIRF temp"=w1020, "LaguerreDeconEngineClass in"=w1058) -> ("error out"=w1049:errorcluster, "LaguerreDeconEngineClass out"=w1050:refnum<class "LaguerreDeconEngineClass.lvclass">)  [unwired: 6 in, 1 out]
        n486 = call "computeIRFAlignment.vi"("error in (no error)"=w1055, "fIRF temp"=w1019, "LaguerreDeconEngineClass in"=w1056) -> ("error out"=w1053:errorcluster, "LaguerreDeconEngineClass out"=w1054:refnum<class "LaguerreDeconEngineClass.lvclass">)  [unwired: 6 in, 1 out]
        n487 = call "computeIRFAlignment.vi"("error in (no error)"=w994, "fIRF temp"=w985, "LaguerreDeconEngineClass in"=w993) -> ("error out"=w1001:errorcluster, "LaguerreDeconEngineClass out"=w1002:refnum<class "LaguerreDeconEngineClass.lvclass">)  [unwired: 6 in, 1 out]
        n488 = call "Ch1DeconEngineFGV.vi"("Error In"=w1051, "action(read)"=w982, "Ch1DeconEngine in"=w1052) -> ("Error Out"=w1047:errorcluster, "Ch1DeconEngine out"=w1048:refnum<class "LaguerreDeconEngineClass.lvclass">)  [unwired: 7 in]
        n489 = call "Ch2DeconEngineFGV.vi"("Error In"=w1049, "action(read)"=w982, "Ch2DeconEngine in"=w1050) -> ("Error Out"=w1037:errorcluster, "Ch2DeconEngine out"=w1038:refnum<class "LaguerreDeconEngineClass.lvclass">)  [unwired: 7 in]
        n490 = call "Ch3DeconEngineFGV.vi"("Error In"=w1053, "action(read)"=w982, "Ch3DeconEngine in"=w1054) -> ("Error Out"=w1031:errorcluster, "Ch3DeconEngine out"=w1032:refnum<class "LaguerreDeconEngineClass.lvclass">)  [unwired: 7 in]
        n491 = call "Ch4DeconEngineFGV.vi"("Error In"=w1001, "action(read)"=w982, "Ch3DeconEngine in"=w1002) -> ("Error Out"=w995:errorcluster, "Ch3DeconEngine out"=w996:refnum<class "LaguerreDeconEngineClass.lvclass">)  [unwired: 7 in]
        n492 = call "setfIRF.vi"("error in (no error)"=w1031, "fIRF"=w1019, "LaguerreDeconEngineClass in"=w1032) -> ("error out"=w1035:errorcluster, "LaguerreDeconEngineClass out"=w1036:refnum<class "LaguerreDeconEngineClass.lvclass">)  [unwired: 7 in]
        n493 = call "setfIRF.vi"("error in (no error)"=w995, "fIRF"=w985, "LaguerreDeconEngineClass in"=w996) -> ("error out"=w999:errorcluster, "LaguerreDeconEngineClass out"=w1000:refnum<class "LaguerreDeconEngineClass.lvclass">)  [unwired: 7 in]
        n494 = call "setfIRF.vi"("error in (no error)"=w1037, "fIRF"=w1020, "LaguerreDeconEngineClass in"=w1038) -> ("error out"=w1041:errorcluster, "LaguerreDeconEngineClass out"=w1042:refnum<class "LaguerreDeconEngineClass.lvclass">)  [unwired: 7 in]
        n495 = call "setfIRF.vi"("error in (no error)"=w1047, "fIRF"=w1007, "LaguerreDeconEngineClass in"=w1048) -> ("error out"=w1045:errorcluster, "LaguerreDeconEngineClass out"=w1046:refnum<class "LaguerreDeconEngineClass.lvclass">)  [unwired: 7 in]
        n496 = Unbundle By Name(w1027) -> ("V1"=w1006:dbl[], "V2"=w1026:dbl[], "V3"=w1025:dbl[], "V4"=w992:dbl[])
        n497 = call "computeLCs.vi"("error in (no error)"=w1045, "LaguerreDeconClass in"=w1046) -> ("error out"=w1043:errorcluster, "LaguerreDeconClass out"=w1044:refnum<class "LaguerreDeconEngineClass.lvclass">)  [unwired: 8 in]
        n498 = call "computeLCs.vi"("error in (no error)"=w1041, "LaguerreDeconClass in"=w1042) -> ("error out"=w1039:errorcluster, "LaguerreDeconClass out"=w1040:refnum<class "LaguerreDeconEngineClass.lvclass">)  [unwired: 8 in]
        n499 = call "computeLCs.vi"("error in (no error)"=w1035, "LaguerreDeconClass in"=w1036) -> ("error out"=w1033:errorcluster, "LaguerreDeconClass out"=w1034:refnum<class "LaguerreDeconEngineClass.lvclass">)  [unwired: 8 in]
        n500 = call "computeLCs.vi"("error in (no error)"=w999, "LaguerreDeconClass in"=w1000) -> ("error out"=w997:errorcluster, "LaguerreDeconClass out"=w998:refnum<class "LaguerreDeconEngineClass.lvclass">)  [unwired: 8 in]
        n501 = call-poly <vilib>:"Mean.vi"("X"=w1006) -> ("mean"=w1005:dbl)  [unwired: 1 out]
        n502 = call-poly <vilib>:"Mean.vi"("X"=w992) -> ("mean"=w991:dbl)  [unwired: 1 out]
        n503 = call-poly <vilib>:"Mean.vi"("X"=w1026) -> ("mean"=w1024:dbl)  [unwired: 1 out]
        n504 = call "getFitting.vi"("error in (no error)"=w1043, "LaguerreDeconEngineClass in"=w1044) -> ("Fitting"=w1016:dbl[])  [unwired: 7 in, 2 out]
        n505 = call "getFitting.vi"("error in (no error)"=w1039, "LaguerreDeconEngineClass in"=w1040) -> ("Fitting"=w1013:dbl[])  [unwired: 7 in, 2 out]
        n506 = call "getFitting.vi"("error in (no error)"=w1033, "LaguerreDeconEngineClass in"=w1034) -> ("Fitting"=w989:dbl[])  [unwired: 7 in, 2 out]
        n507 = call "getFitting.vi"("error in (no error)"=w997, "LaguerreDeconEngineClass in"=w998) -> ("Fitting"=w988:dbl[])  [unwired: 7 in, 2 out]
        n508 = Add(x=w1017, y=w1016) -> (x+y=w1018:dbl[])
        n509 = Add(x=w1014, y=w1013) -> (x+y=w1015:dbl[])
        n510 = call-poly <vilib>:"Mean.vi"("X"=w1025) -> ("mean"=w1023:dbl)  [unwired: 1 out]
        n511 = Add(x=w1012, y=w989) -> (x+y=w1011:dbl[])
        n512 = Build Array(w1010, w1018) -> (w1030:dbl[][])
        n513 = Build Array(w1009, w1015) -> (w1029:dbl[][])
        n514 = Build Array(w1008, w1011) -> (w1028:dbl[][])
        n515 = Add(x=w987, y=w988) -> (x+y=w986:dbl[])
        n516 = Bundle("mean"=w1005, "mean"=w1024, "mean"=w1023, "mean"=w991) -> (w990:T37)  [unwired: 1 in]
        n517 = Build Array(w983, w986) -> (w984:dbl[][])
        n518 = call "Calib_and_iRFAlign_confirm.vi"(6:w990, "Current V"=w984, "Ch3 Data"=w1028, "Ch2 Data"=w1029, "Ch1 Data"=w1030) -> ("Save?"=w1022:bool)  [unwired: 6 in]
        n519 = case shown="True" w1022 {
          tunnel: ["" ("Empty String Constant") "Data: saveCalibration\nData: saveiRF\nRun: CaliIncrement"] -> w1021
          frame False {
          }
          frame True {
            # "[Covers: REQ2]"
          }
        }
        n520 = call <vilib>:"Add State(s) to Queue__JKI_lib_State_Machine.vi"("State(s) in Front (\"\")"=w1021, "State(s) in (\"\")"=w1066) -> ("States Out"=w1065:string)  [unwired: 13 in]
      }
      frame "Data: parseRunData" {
        # "All APD bias"
        # "flash queue"
        # "Ch3&4"
        # "Ch1&2"
        # "Flash data from queue and save it in structure\n()"
        n521 = Flush Queue(queue=w1094, error in (no error)=w1093) -> (remaining elements=w1088:T38, error out=w1089:errorcluster)  [unwired: 1 out]
        n522 = Flush Queue(queue=w1099, error in (no error)=w1093) -> (remaining elements=w1097:cluster{"double data":dbl[][]}[], error out=w1090:errorcluster)  [unwired: 1 out]
        n523 = Flush Queue(queue=w1100, error in (no error)=w1093) -> (remaining elements=w1098:cluster{"double data":dbl[][]}[], error out=w1091:errorcluster)  [unwired: 1 out]
        n524 = for {
          tunnel: w1098 -> [w1116] mode=indexing
          tunnel: [w1114] -> w1083 mode=concatenating
          tunnel: [w1113] -> w1084 mode=concatenating
          n525 = Unbundle By Name(w1116) -> ("double data"=w1115:dbl[][])
          n526 = call "SeperateChanData.vi"("Input (Ch1&2)"=w1115) -> ("Ch1"=w1114:dbl[][], "Ch2"=w1113:dbl[][])
        }
        n527 = for {
          tunnel: w1097 -> [w1112] mode=indexing
          tunnel: [w1111] -> w1073 mode=concatenating
          tunnel: [w1109] -> w1074 mode=concatenating
          n528 = Unbundle By Name(w1112) -> ("double data"=w1110:dbl[][])
          n529 = call "SeperateChanData.vi"("Input (Ch1&2)"=w1110) -> ("Ch1"=w1111:dbl[][], "Ch2"=w1109:dbl[][])
        }
        n530 = call "FLImDAQ_FGV.vi"() -> ("Read data"=w1081:T5)  [unwired: 10 in, 1 out]
        n531 = Unbundle By Name(w1081) -> ("Waveform to Avg"=w1071:i16)
        n532 = for {
          tunnel: w1088 -> [w1108] mode=indexing
          tunnel: [w1107] -> w1080 mode=indexing
          tunnel: [w1106] -> w1078 mode=indexing
          tunnel: [w1105] -> w1076 mode=indexing
          tunnel: [w1104] -> w1072 mode=indexing
          n533 = Unbundle By Name(w1108) -> ("V1"=w1107:dbl, "V2"=w1106:dbl, "V3"=w1105:dbl, "V4"=w1104:dbl)
        }
        n534 = call "DuplicateV(SubVI).vi"("Averaging"=w1071, "V in"=w1080) -> ("V out"=w1079:dbl[])  [unwired: 9 in]
        n535 = Array Size(array=w1073) -> (size(s)=→"data Size":i32[])
        n536 = call "DuplicateV(SubVI).vi"("Averaging"=w1071, "V in"=w1078) -> ("V out"=w1077:dbl[])  [unwired: 9 in]
        n537 = call "DuplicateV(SubVI).vi"("Averaging"=w1071, "V in"=w1076) -> ("V out"=w1075:dbl[])  [unwired: 9 in]
        n538 = call "DuplicateV(SubVI).vi"("Averaging"=w1071, "V in"=w1072) -> ("V out"=w1069:dbl[])  [unwired: 9 in]
        n539 = Bundle By Name(cluster=w1095, "Ch1Data"=w1083, "Ch2Data"=w1084, "Ch3Data"=w1073, "Ch4Data"=w1074, "V1"=w1079, "V2"=w1077, "V3"=w1075, "V4"=w1069) -> (w1096:T24)
        n540 = Merge Errors(w1091, w1090, w1089) -> (w1092:errorcluster)
        n541 = Array Size(array=w1079) -> (size(s)=→"V1 Size":i32)
        n542 = Array Size(array=w1077) -> (size(s)=→"V2 Size":i32)
        n543 = Array Size(array=w1075) -> (size(s)=→"V3 Size":i32)
        n544 = Array Size(array=w1069) -> (size(s)=→"V4 Size":i32)
        n545 = call <vilib>:"Add State(s) to Queue__JKI_lib_State_Machine.vi"("State(s) in (\"\")"=w1103) -> ("States Out"=w1102:string)  [unwired: 14 in]
      }
      frame "Data: saveRunData" {
        w1119 = T39 {"DataPath"=path "", "CaseID"="", "RunID"=0, "Ch1Data"=[], "Ch2Data"=[], "Ch3Data"=[], "Ch4Data"=[], "V1"=[], "V2"=[], "V3"=[], "V4"=[], "LaserRepRate"=0, "WFAverage"=0, "RunStartTime"=0}  # Data cluster
        # "Save FLIm data to disk.\n(Save to LV tdms file format)"
        n546 = Unbundle By Name(w1130) -> ("Pathes.DataPath"=w1126:path, "CaseID"=w1138:string, "IDs.RunID"=w1128:i8, "Ch1Data"=w1137:dbl[][], "Ch2Data"=w1136:dbl[][], "Ch3Data"=w1125:dbl[][], "Ch4Data"=w1118:dbl[][], "V1"=w1120:dbl[], "V2"=w1135:dbl[], "V3"=w1134:dbl[], "V4"=w1117:dbl[])
        n547 = call "FLImDAQ_FGV.vi"() -> ("Read data"=w1123:T5)  [unwired: 10 in, 1 out]
        n548 = Unbundle By Name(w1123) -> ("Waveform to Avg"=w1122:i16)
        n549 = local read "RunStartTime"() -> (w1121:u32)
        n550 = local read "Laser Rep Rate"() -> (w1124:dbl)
        n551 = Increment(x=w1128) -> (x+1=w1127:i8)
        n552 = Bundle By Name(cluster=w1119, "DataPath"=w1126, "CaseID"=w1138, "RunID"=w1127, "Ch1Data"=w1137, "Ch2Data"=w1136, "Ch3Data"=w1125, "Ch4Data"=w1118, "V1"=w1120, "V2"=w1135, "V3"=w1134, "V4"=w1117, "LaserRepRate"=w1124, "WFAverage"=w1122, "RunStartTime"=w1121) -> (w1133:T39)
        n553 = call "SaveRunData(SubVI).vi"("Data cluster"=w1133, "error in (no error)"=w1132) -> ("error out"=w1129:errorcluster)  [unwired: 13 in]
        n554 = flat-sequence {
          tunnel: w1130 -> [w1146]
          tunnel: [w1145] -> w1131
          tunnel: w1129 -> [_]
          frame #0 {
            w1143 = dbl[][] [] ("Ch1Data")
            w1144 = dbl[] [] ("V1")
            # "reset local data"
            n555 = Bundle By Name(cluster=w1146, "Ch1Data"=w1143, "Ch2Data"=w1143, "Ch3Data"=w1143, "Ch4Data"=w1143, "V1"=w1144, "V2"=w1144, "V3"=w1144, "V4"=w1144) -> (w1145:T24)
          }
        }
        n556 = case shown="No Error" w1129 {
          tunnel: ["Run: Increment" "" ("Empty String Constant")] -> w1139
          frame No Error {
          }
          frame Error {
          }
        }
        n557 = call <vilib>:"Add State(s) to Queue__JKI_lib_State_Machine.vi"("State(s) in Front (\"\")"=w1139, "State(s) in (\"\")"=w1142) -> ("States Out"=w1141:string)  [unwired: 13 in]
      }
      frame "Data: Cleanup" {
        # "Cleanup any data and references, here.\n(this is called automatically, by the Macro: Exit)"
        n558 = Unbundle By Name(w1150) -> ("Core.Current VI Reference"=w1153:refnum<vi>)
        n559 = Close Reference(reference=w1153, error in (no error)=w1152) -> (error out=w1151:errorcluster)
        n560 = call <vilib>:"Add State(s) to Queue__JKI_lib_State_Machine.vi"("State(s) in (\"\")"=w1155) -> ("States Out"=w1154:string)  [unwired: 14 in]
      }
      frame "---------- Core ----------" {
        # "Do not put any code in this frame.\n(it is a separator no-op)"
        n561 = call <vilib>:"Add State(s) to Queue__JKI_lib_State_Machine.vi"("State(s) in (\"\")"=w1160) -> ("States Out"=w1159:string)  [unwired: 14 in]
      }
      frame Default {
        w1171 = 42 items=["No error", "Argument error", "Memory is full", "Out of zone", "End of file", "File already open", "Generic file I/O error", "File not found", "File permission error", "Disk is full", "Duplicate path", "Too many files open", "System feature not enabled", "Resource file not found", "Cannot add resource", "Resource not found", "Image not found", "Image memory error", "Pen does not exist", "Config type invalid", "Config token not found", "Config parse error", "Config memory error", "Bad external code format", "Bad external code offset", "External code not present", "Null window", "Destroy window error", "Null menu", "Print aborted", "Bad print record", "Print driver error", "Windows error during printing", "Memory error during printing", "Print dialog error", "Generic print error", "Invalid device refnum", "Device not found", "Device parameter error", "Device unit error", "Cannot open device", "Device call aborted", "Generic error", "Cancelled by user", "Object ID too low", "Object ID too high", "Object not in heap", "Unknown heap", "Unknown object (invalid DefProc)", "Unknown object (DefProc not in table)", "Message out of range", "Invalid (null) method", "Unknown message", "Manager call not supported", "Bad address", "Network operation in progress", "Network operation timed out", "Connection is busy", "Network attribute not supported", "Network error", "Address in use", "System out of memory", "Connection aborted", "Connection refused", "Not connected", "Already connected", "Connection closed", "Initialization error (interapplication manager)", "Bad occurrence", "Wait on unbound occurrence handler", "Occurrence queue overflow", "Datalog type conflict", "Unused", "Unrecognized type (interapplication manager)", "Memory corrupt", "Failed to make temporary DLL", "Old CIN version", "Drag socket not found", "Failed to load drop-object", "Failed to register OLE object", "Failed to release OLE object", "Format specifier type mismatch", "Unknown format specifier", "Too few format specifiers", "Too many format specifiers", "Scan failed", "Newer CIN version", "Error converting to variant", "Runtime menu error", "Password tampered", "Variant attribute not found", "Incompatible variant data type", "Event data is not available", "Event Store is not present", "Occurrence is not found", "Event Queue is not created", "Event info is not available", "Refnum passed is NULL", "Error retrieving Class GUID", "Error retrieving CoClass GUID", "Error retrieving TypeLib GUID.", "Bad built application magic bytes.", "Specific driver is different from the specific driver associated with the Logical Name.", "There is no session opened to the class driver.", "Max Error", "MAX - Error with config objects", "MAX - Error loading configuration", "MAX - Group not supported"]
        # "Current State"
        # "Do not delete, rename, or modify this frame.\n(this is used to capture unhandled states and typos)"
        # "Handle mistyped state name (developer tool)"
        n562 = Format Into String(format string="Software Exception: Unhandled State \"%s\"." ("message"), error in=w1167, w1162) -> (resulting string=w1170:string, error out=w1169:errorcluster)  [unwired: 1 in]
        n563 = call <vilib>:"Error Cluster From Error Code.vi"("show call chain? (False)"=TRUE, "error in (no error)"=w1169, "error message (\"\")"=w1170, "error code (0)"=w1171) -> ("error out"=w1168:errorcluster)  [unwired: 5 in]
        n564 = call <vilib>:"Add State(s) to Queue__JKI_lib_State_Machine.vi"("State(s) in (\"\")"=w1166) -> ("States Out"=w1165:string)  [unwired: 14 in]
      }
      frame "Initialize Core Data" {
        # "Build default path based on the location of project"
        # "Do not delete, rename, or modify this frame.\n(this is used to determine panel behavior on exit)"
        # "originally closed?"
        # "exe?"
        # "If panel starts closed or is an EXE, then close it when we exit"
        n565 = call <vilib>:"Application Directory.vi"() -> ("Application Directory"=w1174:path)
        n566 = property on="Property Node" class="App"() -> ("App.Kind"=w1190:T19)  [unwired: 2 in, 2 out]
        n567 = property on="Property Node" class="VI"() -> ("FP.State"=w1184:T18)  [unwired: 2 in, 2 out]
        n568 = control-ref of="Current VI Reference"() -> (w1185:refnum<vi>)
        n569 = Equal?(x=w1184, y=T18."Closed" ("Front Panel Window:State")) -> (x = y?=w1182:bool)
        n570 = Strip Path(path=w1174) -> (stripped path=w1173:path)  [unwired: 1 out]
        n571 = Equal?(x=w1190, y=T19."Run Time System" ("Application:Kind")) -> (x = y?=w1188:bool)
        n572 = Build Path(base path=w1173, name or relative path="Data") -> (appended path=w1180:path)
        n573 = Build Path(base path=w1174, name or relative path="SystemTemp") -> (appended path=w1177:path)
        n574 = Build Path(base path=w1174, name or relative path="SystemCalibrationFile") -> (appended path=w1175:path)
        n575 = Or(x=w1182, y=w1188) -> (x .or. y?=w1186:bool)
        n576 = Bundle By Name(cluster=w1187, "Core.Current VI Reference"=w1185, "Core.Close Panel on Exit?"=w1186, "DefaultPath"=w1180, "TempPath"=w1177, "CaliPath"=w1175) -> (w1192:T24)
        n577 = call <vilib>:"Add State(s) to Queue__JKI_lib_State_Machine.vi"("State(s) in (\"\")"=w1194) -> ("States Out"=w1193:string)  [unwired: 14 in]
      }
      frame "Error Handler" {
        # "Unhandled Error -- Display it"
        # "Handle any errors here.\nYou can also output any states to clean-up after errors occur"
        # "Clear error"
        n578 = Unbundle By Name(w1195) -> ("code"=w1197:i32)
        n579 = case shown="Default" w1197 {
          tunnel: ["Macro: Exit" w1207 w1213] -> w1196
          tunnel: w1195 -> [w1203 _ _]
          frame Default {
            w1205 = T40 1 items=["no dialog", "OK message", "continue or stop message", "OK message + warnings", "continue/stop + warnings"] ("type of dialog (OK msg:1)")
            n580 = call <vilib>:"General Error Handler.vi"("type of dialog (OK msg:1)"=w1205, "error in (no error)"=w1203) -> ()  [unwired: 9 in, 5 out]
          }
          frame 5002 {
            n581 = Two Button Dialog(message="Laser interlock open! Please close interlock and try again! ", 1:"Safely Shutdown" ("F button name (\"Cancel\")"), 2:"OK" ("T button name (\"OK\")")) -> (T button?=w1208:bool)
            n582 = case shown="True" w1208 {
              tunnel: ["Macro: Exit" "355 Laser: CheckControllerStatus"] -> w1207
              frame False {
              }
              frame True {
              }
            }
          }
          frame 5001 {
            n583 = Two Button Dialog(message="Unable to connect to imaging computer, do you want to run data aquisiton alone? ", 1:"No" ("F button name (\"Cancel\")"), 2:"Yes" ("T button name (\"OK\")")) -> (T button?=w1214:bool)
            n584 = case shown="False" w1214 {
              tunnel: ["Macro: Exit" "" ("Empty String Constant")] -> w1213
              frame False {
              }
              frame True {
              }
            }
          }
        }
        n585 = call <vilib>:"Add State(s) to Queue__JKI_lib_State_Machine.vi"("State(s) in Front (\"\")"=w1196, "State(s) in (\"\")"=w1202) -> ("States Out"=w1201:string)  [unwired: 13 in]
      }
      frame "Exit" {
        # "Do not put any code in this frame.\n(No errors that occur here will be handled.)"
        n586 = call <vilib>:"Add State(s) to Queue__JKI_lib_State_Machine.vi"("State(s) in (\"\")"=w1225) -> ("States Out"=w1224:string)  [unwired: 14 in]
      }
      frame "---------- Case ----------" {
        # "Template Separator\n(You can make a copy of, or modify, this frame)"
        n587 = call <vilib>:"Add State(s) to Queue__JKI_lib_State_Machine.vi"("State(s) in (\"\")"=w1230) -> ("States Out"=w1229:string)  [unwired: 14 in]
      }
      frame "Case: getCaliID" {
        # "Get Calibration file #\n(You can make a copy of, or modify, this frame)"
        n588 = Unbundle By Name(w1231) -> ("Pathes.CaliPath"=w1234:path)
        n589 = call <vilib>:"Recursive File List.vi"("pattern"="*.tdms", "Treat LLBs as Folders?"=FALSE, "Folder Path"=w1234) -> ("All Files in Dir"=w1239:path[])  [unwired: 4 in, 4 out]
        n590 = for {
          tunnel: w1239 -> [w1249] mode=indexing
          tunnel: [w1248] -> w1238 mode=indexing
          tunnel: "Calibration" -> [w1245]
          n591 = Strip Path(path=w1249) -> (name=w1246:string)  [unwired: 1 out]
          n592 = Search and Replace String(input string=w1246, search string=w1245) -> (result string=w1244:string)  [unwired: 6 in, 3 out]
          n593 = Scan From String(format string="%d" ("string"), input string=w1244) -> (output 1=w1248:i32)  [unwired: 3 in, 3 out]
        }
        n594 = Array Max & Min(array=w1238) -> (max value=w1237:i32)  [unwired: 3 out]
        n595 = Bundle By Name(cluster=w1231, "IDs.Cali ID"=w1237) -> (w1232:T24)
        n596 = call <vilib>:"Add State(s) to Queue__JKI_lib_State_Machine.vi"("State(s) in (\"\")"=w1243) -> ("States Out"=w1242:string)  [unwired: 14 in]
      }
      frame "Case: getBGID" {
        # "Get background #\n(You can make a copy of, or modify, this frame)"
        n597 = Unbundle By Name(w1252) -> ("Pathes.BG Path"=w1257:path)
        n598 = call <vilib>:"Recursive File List.vi"("pattern"="*.tdms", "Treat LLBs as Folders?"=FALSE, "Folder Path"=w1257) -> ("All Files in Dir"=w1255:path[])  [unwired: 4 in, 4 out]
        n599 = for {
          tunnel: w1255 -> [w1272] mode=indexing
          tunnel: "Background" ("name or relative path") -> [w1270]
          shift-right: [w1263] -> w1250
          shift-left: 0 -> [w1267]
          n600 = Strip Path(path=w1272) -> (name=w1271:string)  [unwired: 1 out]
          n601 = Search and Replace String(input string=w1271, search string=w1270) -> (number of replacements=w1269:i32)  [unwired: 6 in, 3 out]
          n602 = Greater Than 0?(x=w1269) -> (x > 0?=w1268:bool)
          n603 = Select(t=1, s=w1268, f=0) -> (s? t:f=w1266:i32)
          n604 = Add(x=w1266, y=w1267) -> (x+y=w1263:i32)
        }
        n605 = Bundle By Name(cluster=w1252, "IDs.BG ID"=w1250) -> (w1253:T24)
        n606 = call <vilib>:"Add State(s) to Queue__JKI_lib_State_Machine.vi"("State(s) in (\"\")"=w1262) -> ("States Out"=w1261:string)  [unwired: 14 in]
      }
      frame "Case: getRunID" {
        # "Check folder for run ID\n(You can make a copy of, or modify, this frame)"
        n607 = Unbundle By Name(w1282) -> ("Pathes.DataPath"=w1281:path, "CaseID"=w1277:string)
        n608 = Build Array("Background" ("name or relative path"), "Calibration", "3DScanData" ("element")) -> (w1287:string[])
        n609 = call <vilib>:"Recursive File List.vi"("Folders to Exclude"=w1287, "pattern"="*.tdms", "Treat LLBs as Folders?"=FALSE, "Folder Path"=w1281) -> ("All Files in Dir"=w1278:path[])  [unwired: 3 in, 4 out]
        n610 = for {
          tunnel: w1278 -> [w1296] mode=indexing
          tunnel: [w1295] -> w1284 mode=indexing
          tunnel: w1277 -> [w1292]
          n611 = Strip Path(path=w1296) -> (name=w1293:string)  [unwired: 1 out]
          n612 = Search and Replace String(input string=w1293, search string=w1292) -> (result string=w1291:string)  [unwired: 6 in, 3 out]
          n613 = Scan From String(format string="_%d" ("string"), input string=w1291) -> (output 1=w1295:i32)  [unwired: 3 in, 3 out]
        }
        n614 = Array Max & Min(array=w1284) -> (max value=w1275:i32)  [unwired: 3 out]
        n615 = Bundle By Name(cluster=w1282, "IDs.RunID"=w1275) -> (w1283:T24)
        n616 = call "RunIDFGV.vi"("Error In"=w1273, "RunID in"=w1275) -> ("Error Out"=w1274:errorcluster)  [unwired: 8 in, 1 out]
        n617 = call <vilib>:"Add State(s) to Queue__JKI_lib_State_Machine.vi"("State(s) in (\"\")"=w1290) -> ("States Out"=w1289:string)  [unwired: 14 in]
      }
      frame "Case: CreatFileStruct" {
        # "Creat case file structure"
        n618 = Unbundle By Name(w1310) -> ("DefaultPath"=w1316:path, "CaseID"=w1303:string)
        n619 = Build Path(base path=w1316, name or relative path=w1303) -> (appended path=w1315:path)
        n620 = call <vilib>:"Check if File or Folder Exists.vi"("error in (no error)"=w1309, "path"=w1315) -> ("error out"=w1312:errorcluster, "file or folder exists?"=w1314:bool, "dup path"=w1313:path)  [unwired: 7 in]
        n621 = case shown="True" w1314 {
          tunnel: w1313 -> [w1333 w1341]
          tunnel: w1312 -> [w1331 w1336]
          tunnel: [w1325 w1341] -> w1301
          tunnel: [w1329 w1343] -> w1300
          tunnel: [u32 0 u32 0] -> w1299
          tunnel: [w1327 w1346] -> w1307
          tunnel: "Background" ("name or relative path") -> [w1326 w1338]
          tunnel: "Calibration" -> [w1324 w1337]
          tunnel: [w1320 w1339] -> w1304
          tunnel: w1303 -> [_ _]
          tunnel: ["" ("Empty String Constant") "Case: getRunID\nCase: getBGID\nCase: getCaliID\nUI: Update"] -> w1302
          frame False {
            # "Folder not exist. Creat folders."
            n622 = Create Folder(path (use dialog)=w1333, error in=w1331) -> (created path=w1325:path, error out=w1322:errorcluster)  [unwired: 1 in, 1 out]
            n623 = Build Path(base path=w1325, name or relative path=w1324) -> (appended path=w1323:path)
            n624 = Build Path(base path=w1325, name or relative path=w1326) -> (appended path=w1332:path)
            n625 = Create Folder(path (use dialog)=w1332, error in=w1322) -> (created path=w1327:path, error out=w1328:errorcluster)  [unwired: 1 in, 1 out]
            n626 = Create Folder(path (use dialog)=w1323, error in=w1322) -> (created path=w1320:path, error out=w1321:errorcluster)  [unwired: 1 in, 1 out]
            n627 = Merge Errors(w1328, w1321) -> (w1329:errorcluster)
          }
          frame True {
            # "Folder exsit, check file #"
            n628 = Build Path(base path=w1341, name or relative path=w1337) -> (appended path=w1342:path)
            n629 = Build Path(base path=w1341, name or relative path=w1338) -> (appended path=w1347:path)
            n630 = call <vilib>:"Check if File or Folder Exists.vi"("path"=w1342) -> ("file or folder exists?"=w1340:bool, "dup path"=w1339:path)  [unwired: 8 in, 1 out]
            n631 = call <vilib>:"Check if File or Folder Exists.vi"("path"=w1347) -> ("file or folder exists?"=w1345:bool, "dup path"=w1346:path)  [unwired: 8 in, 1 out]
            n632 = And(x=w1345, y=w1340) -> (x .and. y?=w1344:bool)
            n633 = case shown="False" w1344 {
              tunnel: w1336 -> [_ w1349]
              tunnel: [errorcluster {"status"=TRUE, "code"=5003, "source"="File structure error."} ("error out") w1349] -> w1343
              frame False {
              }
              frame True {
              }
            }
          }
        }
        n634 = Bundle By Name(cluster=w1310, "Pathes.DataPath"=w1301, "Pathes.BG Path"=w1307, "Pathes.CaliPath"=w1304, "IDs.RunID"=w1299, "IDs.BG ID"=w1299, "IDs.Cali ID"=w1299) -> (w1311:T24)
        n635 = call "DataRootPathFGV.vi"("Error In"=w1300, "PathIn"=w1301) -> ("Error Out"=w1298:errorcluster)  [unwired: 8 in, 1 out]
        n636 = call "RunIDFGV.vi"("Error In"=w1298, "RunID in"=w1299) -> ("Error Out"=w1297:errorcluster)  [unwired: 8 in, 1 out]
        n637 = call <vilib>:"Add State(s) to Queue__JKI_lib_State_Machine.vi"("State(s) in Front (\"\")"=w1302, "State(s) in (\"\")"=w1318) -> ("States Out"=w1317:string)  [unwired: 13 in]
      }
      frame "Case: GetID" {
        # "Template Separator\n(You can make a copy of, or modify, this frame)"
        n638 = call "set_subjectID.vi"() -> ("subject_id"=w1350:string)  [unwired: 10 in]
        n639 = Bundle By Name(cluster=w1352, "CaseID"=w1350) -> (w1353:T24)
        n640 = call <vilib>:"Add State(s) to Queue__JKI_lib_State_Machine.vi"("State(s) in (\"\")"=w1356) -> ("States Out"=w1355:string)  [unwired: 14 in]
      }
      frame "---------- DeconEngine ----------" {
        # "start data aquisition and then set irfAligh to ture and decon channel to 1,2 and 3."
        # "Template Separator\n(You can make a copy of, or modify, this frame)"
        n641 = call <vilib>:"Add State(s) to Queue__JKI_lib_State_Machine.vi"("State(s) in (\"\")"=w1361) -> ("States Out"=w1360:string)  [unwired: 14 in]
      }
      frame "DeconEngine: InitDotNet" {
        # "Initialize Dot Net Decon and save the FGV"
        # "Initilize Dot Net \n(You can make a copy of, or modify, this frame)"
        n642 = constructor on="Constructor Node" class="LaguerreDeCon"(error in=w1363) -> (reference out=w1365:refnum<k24>, error out=w1364:errorcluster)  [unwired: 2 in, 1 out]
        n643 = call "DotNetFGV.vi"("Error In"=w1364, "Operation (Read)"=enum16{"Read", "Write"}."Write", "reference in"=w1365) -> ("Error Out"=w1362:errorcluster)  [unwired: 7 in, 1 out]
        n644 = case shown="No Error" w1362 {
          frame No Error {
            ".NetInitialized?" <- TRUE (".NetInitialized?")
          }
          frame Error {
          }
        }
        n645 = call <vilib>:"Add State(s) to Queue__JKI_lib_State_Machine.vi"("State(s) in (\"\")"=w1370) -> ("States Out"=w1369:string)  [unwired: 14 in]
      }
      frame "DeconEngine: Warmup" {
        # "Warm up parpool\n(You can make a copy of, or modify, this frame)"
        n646 = call "DotNetFGV.vi"("Error In"=w1376) -> ("Error Out"=w1377:errorcluster, "reference out"=w1378:refnum<k24>)  [unwired: 9 in]
        n647 = flat-sequence {
          tunnel: w1376 -> [_]
          tunnel: [w1384] -> w1373
          frame #0 {
            n648 = Tick Count (ms)() -> (millisecond timer value=w1384:u32)
          }
        }
        n649 = invoke class="LaguerreDeCon" method="init_parpool"(reference=w1378, error in=w1377) -> (error out=w1375:errorcluster)  [unwired: 1 in, 2 out]
        n650 = flat-sequence {
          tunnel: w1375 -> [_]
          tunnel: [w1383] -> w1374
          frame #0 {
            n651 = Tick Count (ms)() -> (millisecond timer value=w1383:u32)
          }
        }
        n652 = Subtract(x=w1374, y=w1373) -> (x-y=→"WarmupTime(ms)":u32)
        n653 = call <vilib>:"Add State(s) to Queue__JKI_lib_State_Machine.vi"("State(s) in (\"\")"=w1382) -> ("States Out"=w1381:string)  [unwired: 14 in]
      }
      frame "DeconEngine: loadIRF" {
        # "Load IRF for decon and save to FGV\n(You can make a copy of, or modify, this frame)"
        n654 = Current VI's Path() -> (path=w1402:path)
        n655 = Strip Path(path=w1402) -> (stripped path=w1401:path)  [unwired: 1 out]
        n656 = Build Path(base path=w1401, name or relative path="DotNetDecon") -> (appended path=w1389:path)
        n657 = Build Path(base path=w1389, name or relative path="Channel1.tdms") -> (appended path=w1406:path)
        n658 = Build Path(base path=w1389, name or relative path="Channel3.tdms") -> (appended path=w1391:path)
        n659 = Build Path(base path=w1389, name or relative path="Channel2.tdms") -> (appended path=w1392:path)
        n660 = call "LoadIRF.vi"("error in (no error)"=w1390, "file path"=w1406) -> ("error out"=w1404:errorcluster, "APD"=w1405:T41)  [unwired: 8 in]
        n661 = call "LoadIRF.vi"("error in (no error)"=w1390, "file path"=w1392) -> ("error out"=w1397:errorcluster, "APD"=w1398:T41)  [unwired: 8 in]
        n662 = call "LoadIRF.vi"("error in (no error)"=w1390, "file path"=w1391) -> ("error out"=w1394:errorcluster, "APD"=w1395:T41)  [unwired: 8 in]
        n663 = call "DeConAPD1FGV.vi"("Error In"=w1404, "Operation (Read)"=enum16{"Read", "Write"}."Write", "APDClass in"=w1405) -> ("Error Out"=w1388:errorcluster)  [unwired: 7 in, 1 out]
        n664 = call "DeConAPD2FGV.vi"("Error In"=w1397, "Operation (Read)"=enum16{"Read", "Write"}."Write", "APDClass in"=w1398) -> ("Error Out"=w1387:errorcluster)  [unwired: 7 in, 1 out]
        n665 = call "DeConAPD3FGV.vi"("Error In"=w1394, "Operation (Read)"=enum16{"Read", "Write"}."Write", "APDClass in"=w1395) -> ("Error Out"=w1386:errorcluster)  [unwired: 7 in, 1 out]
        n666 = Merge Errors(w1388, w1387, w1386) -> (w1385:errorcluster)
        n667 = call <vilib>:"Add State(s) to Queue__JKI_lib_State_Machine.vi"("State(s) in (\"\")"=w1412) -> ("States Out"=w1411:string)  [unwired: 14 in]
      }
      frame "DeconEngine: CloseNetRef" {
        # "Template Separator\n(You can make a copy of, or modify, this frame)"
        n668 = call "DotNetFGV.vi"("Error In"=w1413) -> ("Error Out"=w1415:errorcluster, "reference out"=w1416:refnum<k24>)  [unwired: 9 in]
        n669 = Close Reference(reference=w1416, error in (no error)=w1415) -> (error out=w1414:errorcluster)
        n670 = call <vilib>:"Add State(s) to Queue__JKI_lib_State_Machine.vi"("State(s) in (\"\")"=w1420) -> ("States Out"=w1419:string)  [unwired: 14 in]
      }
      frame "DeconEngine: InitilizeMacro" {
        # "start data aquisition and then set irfAligh to ture and decon channel to 1,2 and 3."
        # "Initilize Decon Engine for all channel\n(You can make a copy of, or modify, this frame)"
        n671 = call <vilib>:"Add State(s) to Queue__JKI_lib_State_Machine.vi"("State(s) in Front (\"\")"="DeconEngine: InitializeCh1\nDeconEngine: InitializeCh2\nDeconEngine: InitializeCh3\nDeconEngine: InitializeCh4" ("State(s) in Front (\"\")"), "State(s) in (\"\")"=w1426) -> ("States Out"=w1425:string)  [unwired: 13 in]
      }
      frame "DeconEngine: InitializeCh1" {
        w1448 = refnum<class "LaguerreDeconEngineClass.lvclass"> refnum  # Ch1DeconObj
        # "Initilize Laguerre Deconvolution engine Object\n(You can make a copy of, or modify, this frame)"
        n672 = global read "GlobalVariables.vi" "LastUseiRF"() -> (w1429:T36)
        n673 = call "setLaguerreOrder.vi"("error in (no error)"=w1436, "LaguerreOrder"=u32 12, "LaguerreDeconClass in"=w1448) -> ("error out"=w1445:errorcluster, "LaguerreDeconClass out"=w1446:refnum<class "LaguerreDeconEngineClass.lvclass">)  [unwired: 7 in]
        n674 = Unbundle By Name(w1429) -> ("Ch1 iRF"=w1428:dbl[])
        n675 = call "setDataLength.vi"("error in (no error)"=w1445, "dataLength"=u32 600, "LaguerreDeconClass in"=w1446) -> ("error out"=w1444:errorcluster, "LaguerreDeconClass out"=w1443:refnum<class "LaguerreDeconEngineClass.lvclass">)  [unwired: 7 in]
        n676 = call "setIRF.vi"("error in (no error)"=w1444, "iRF"=w1428, "LaguerreDeconClass in"=w1443) -> ("error out"=w1441:errorcluster, "LaguerreDeconClass out"=w1442:refnum<class "LaguerreDeconEngineClass.lvclass">)  [unwired: 7 in]
        n677 = call "computeAlpha.vi"("error in (no error)"=w1441, "LaguerreDeconClass in"=w1442) -> ("error out"=w1439:errorcluster, "LaguerreDeconClass out"=w1440:refnum<class "LaguerreDeconEngineClass.lvclass">)  [unwired: 8 in]
        n678 = call "dataInitilize.vi"("error in (no error)"=w1439, "LaguerreDeconClass in"=w1440) -> ("error out"=w1437:errorcluster, "LaguerreDeconClass out"=w1438:refnum<class "LaguerreDeconEngineClass.lvclass">)  [unwired: 8 in]
        n679 = call "computeDeconMatrix.vi"("error in (no error)"=w1437, "LaguerreDeconClass in"=w1438) -> ("error out"=w1433:errorcluster, "LaguerreDeconClass out"=w1435:refnum<class "LaguerreDeconEngineClass.lvclass">)  [unwired: 8 in]
        n680 = call "Ch1DeconEngineFGV.vi"("Error In"=w1433, "action(read)"=enum16{"write", "read"}."write" ("action"), "Ch1DeconEngine in"=w1435) -> ("Error Out"=w1432:errorcluster)  [unwired: 7 in, 1 out]
        n681 = call <vilib>:"Add State(s) to Queue__JKI_lib_State_Machine.vi"("State(s) in (\"\")"=w1450) -> ("States Out"=w1449:string)  [unwired: 14 in]
      }
      frame "DeconEngine: InitializeCh2" {
        w1472 = refnum<class "LaguerreDeconEngineClass.lvclass"> refnum  # Ch2DeconObj
        # "Initilize Laguerre Deconvolution engine Object\n(You can make a copy of, or modify, this frame)"
        n682 = global read "GlobalVariables.vi" "LastUseiRF"() -> (w1453:T36)
        n683 = call "setLaguerreOrder.vi"("error in (no error)"=w1460, "LaguerreOrder"=u32 12, "LaguerreDeconClass in"=w1472) -> ("error out"=w1469:errorcluster, "LaguerreDeconClass out"=w1470:refnum<class "LaguerreDeconEngineClass.lvclass">)  [unwired: 7 in]
        n684 = Unbundle By Name(w1453) -> ("Ch2 iRF"=w1452:dbl[])
        n685 = call "setDataLength.vi"("error in (no error)"=w1469, "dataLength"=u32 600, "LaguerreDeconClass in"=w1470) -> ("error out"=w1468:errorcluster, "LaguerreDeconClass out"=w1467:refnum<class "LaguerreDeconEngineClass.lvclass">)  [unwired: 7 in]
        n686 = call "setIRF.vi"("error in (no error)"=w1468, "iRF"=w1452, "LaguerreDeconClass in"=w1467) -> ("error out"=w1465:errorcluster, "LaguerreDeconClass out"=w1466:refnum<class "LaguerreDeconEngineClass.lvclass">)  [unwired: 7 in]
        n687 = call "computeAlpha.vi"("error in (no error)"=w1465, "LaguerreDeconClass in"=w1466) -> ("error out"=w1463:errorcluster, "LaguerreDeconClass out"=w1464:refnum<class "LaguerreDeconEngineClass.lvclass">)  [unwired: 8 in]
        n688 = call "dataInitilize.vi"("error in (no error)"=w1463, "LaguerreDeconClass in"=w1464) -> ("error out"=w1461:errorcluster, "LaguerreDeconClass out"=w1462:refnum<class "LaguerreDeconEngineClass.lvclass">)  [unwired: 8 in]
        n689 = call "computeDeconMatrix.vi"("error in (no error)"=w1461, "LaguerreDeconClass in"=w1462) -> ("error out"=w1457:errorcluster, "LaguerreDeconClass out"=w1459:refnum<class "LaguerreDeconEngineClass.lvclass">)  [unwired: 8 in]
        n690 = call "Ch2DeconEngineFGV.vi"("Error In"=w1457, "action(read)"=enum16{"write", "read"}."write" ("action"), "Ch2DeconEngine in"=w1459) -> ("Error Out"=w1456:errorcluster)  [unwired: 7 in, 1 out]
        n691 = call <vilib>:"Add State(s) to Queue__JKI_lib_State_Machine.vi"("State(s) in (\"\")"=w1474) -> ("States Out"=w1473:string)  [unwired: 14 in]
      }
      frame "DeconEngine: InitializeCh3" {
        w1476 = refnum<class "LaguerreDeconEngineClass.lvclass"> refnum  # Ch3DeconObj
        # "Initilize Laguerre Deconvolution engine Object\n(You can make a copy of, or modify, this frame)"
        n692 = global read "GlobalVariables.vi" "LastUseiRF"() -> (w1478:T36)
        n693 = call "setLaguerreOrder.vi"("error in (no error)"=w1485, "LaguerreOrder"=u32 12, "LaguerreDeconClass in"=w1476) -> ("error out"=w1494:errorcluster, "LaguerreDeconClass out"=w1495:refnum<class "LaguerreDeconEngineClass.lvclass">)  [unwired: 7 in]
        n694 = Unbundle By Name(w1478) -> ("Ch3 iRF"=w1477:dbl[])
        n695 = call "setDataLength.vi"("error in (no error)"=w1494, "dataLength"=600, "LaguerreDeconClass in"=w1495) -> ("error out"=w1493:errorcluster, "LaguerreDeconClass out"=w1492:refnum<class "LaguerreDeconEngineClass.lvclass">)  [unwired: 7 in]
        n696 = call "setIRF.vi"("error in (no error)"=w1493, "iRF"=w1477, "LaguerreDeconClass in"=w1492) -> ("error out"=w1490:errorcluster, "LaguerreDeconClass out"=w1491:refnum<class "LaguerreDeconEngineClass.lvclass">)  [unwired: 7 in]
        n697 = call "computeAlpha.vi"("error in (no error)"=w1490, "LaguerreDeconClass in"=w1491) -> ("error out"=w1488:errorcluster, "LaguerreDeconClass out"=w1489:refnum<class "LaguerreDeconEngineClass.lvclass">)  [unwired: 8 in]
        n698 = call "dataInitilize.vi"("error in (no error)"=w1488, "LaguerreDeconClass in"=w1489) -> ("error out"=w1486:errorcluster, "LaguerreDeconClass out"=w1487:refnum<class "LaguerreDeconEngineClass.lvclass">)  [unwired: 8 in]
        n699 = call "computeDeconMatrix.vi"("error in (no error)"=w1486, "LaguerreDeconClass in"=w1487) -> ("error out"=w1482:errorcluster, "LaguerreDeconClass out"=w1484:refnum<class "LaguerreDeconEngineClass.lvclass">)  [unwired: 8 in]
        n700 = call "Ch3DeconEngineFGV.vi"("Error In"=w1482, "action(read)"=enum16{"write", "read"}."write" ("action"), "Ch3DeconEngine in"=w1484) -> ("Error Out"=w1481:errorcluster)  [unwired: 7 in, 1 out]
        n701 = call <vilib>:"Add State(s) to Queue__JKI_lib_State_Machine.vi"("State(s) in (\"\")"=w1498) -> ("States Out"=w1497:string)  [unwired: 14 in]
      }
      frame "DeconEngine: InitializeCh4" {
        w1500 = refnum<class "LaguerreDeconEngineClass.lvclass"> refnum  # Ch3DeconObj
        # "Initilize Laguerre Deconvolution engine Object\n(You can make a copy of, or modify, this frame)"
        n702 = global read "GlobalVariables.vi" "LastUseiRF"() -> (w1502:T36)
        n703 = call "setLaguerreOrder.vi"("error in (no error)"=w1509, "LaguerreOrder"=u32 12, "LaguerreDeconClass in"=w1500) -> ("error out"=w1518:errorcluster, "LaguerreDeconClass out"=w1519:refnum<class "LaguerreDeconEngineClass.lvclass">)  [unwired: 7 in]
        n704 = Unbundle By Name(w1502) -> ("Ch4 iRF"=w1501:dbl[])
        n705 = call "setDataLength.vi"("error in (no error)"=w1518, "dataLength"=u32 600, "LaguerreDeconClass in"=w1519) -> ("error out"=w1517:errorcluster, "LaguerreDeconClass out"=w1516:refnum<class "LaguerreDeconEngineClass.lvclass">)  [unwired: 7 in]
        n706 = call "setIRF.vi"("error in (no error)"=w1517, "iRF"=w1501, "LaguerreDeconClass in"=w1516) -> ("error out"=w1514:errorcluster, "LaguerreDeconClass out"=w1515:refnum<class "LaguerreDeconEngineClass.lvclass">)  [unwired: 7 in]
        n707 = call "computeAlpha.vi"("error in (no error)"=w1514, "LaguerreDeconClass in"=w1515) -> ("error out"=w1512:errorcluster, "LaguerreDeconClass out"=w1513:refnum<class "LaguerreDeconEngineClass.lvclass">)  [unwired: 8 in]
        n708 = call "dataInitilize.vi"("error in (no error)"=w1512, "LaguerreDeconClass in"=w1513) -> ("error out"=w1510:errorcluster, "LaguerreDeconClass out"=w1511:refnum<class "LaguerreDeconEngineClass.lvclass">)  [unwired: 8 in]
        n709 = call "computeDeconMatrix.vi"("error in (no error)"=w1510, "LaguerreDeconClass in"=w1511) -> ("error out"=w1506:errorcluster, "LaguerreDeconClass out"=w1508:refnum<class "LaguerreDeconEngineClass.lvclass">)  [unwired: 8 in]
        n710 = call "Ch4DeconEngineFGV.vi"("Error In"=w1506, "action(read)"=enum16{"write", "read"}."write" ("action"), "Ch3DeconEngine in"=w1508) -> ("Error Out"=w1505:errorcluster)  [unwired: 7 in, 1 out]
        n711 = call <vilib>:"Add State(s) to Queue__JKI_lib_State_Machine.vi"("State(s) in (\"\")"=w1522) -> ("States Out"=w1521:string)  [unwired: 14 in]
      }
      frame "---------- Digitizer ----------" {
        # "Template Separator\n(You can make a copy of, or modify, this frame)"
        n712 = call <vilib>:"Add State(s) to Queue__JKI_lib_State_Machine.vi"("State(s) in (\"\")"=w1527) -> ("States Out"=w1526:string)  [unwired: 14 in]
      }
      frame "Digitizer: Initialize" {
        # "reset digitizer to everytime the system runs"
        # "reset digitizer to everytime the system runs"
        # "Initialize digitizer.\nInitialize both digitizer and update status."
        n713 = call "FLImDAQ_FGV.vi"("error in (no error)"=w1535) -> ("error out"=w1529:errorcluster, "Read data"=w1534:T5)  [unwired: 9 in]
        n714 = Unbundle By Name(w1537) -> ("SysConfigCluster.Ch1Enable?"=w1542:bool, "SysConfigCluster.Ch2Enable?"=w1541:bool, "SysConfigCluster.Ch3Enable?"=w1539:bool)
        n715 = Unbundle By Name(w1534) -> ("Digitizer 1"=w1530:refnum<k15>, "Digitizer 2"=w1533:refnum<k15>)
        n716 = property on="Digitizer" class="Bool (strict)"("Blinking"=TRUE) -> ()  [unwired: 2 in, 2 out]
        n717 = Or(x=w1542, y=w1541) -> (x .or. y?=w1540:bool)
        n718 = case shown="True" w1540 {
          tunnel: w1529 -> [w1550 w1553]
          tunnel: [w1550 w1552] -> w1531
          tunnel: w1530 -> [_ w1554]
          frame False {
          }
          frame True {
            n719 = call <instrlib>:"niScope Initialize.vi"("resource name"=w1554, "reset device"=TRUE, "error in"=w1553) -> ("error out"=w1552:errorcluster)  [unwired: 11 in, 1 out]
          }
        }
        n720 = case shown="True" w1539 {
          tunnel: w1529 -> [w1545 w1547]
          tunnel: [w1545 w1549] -> w1536
          tunnel: w1533 -> [_ w1548]
          frame False {
          }
          frame True {
            n721 = call <instrlib>:"niScope Initialize.vi"("resource name"=w1548, "reset device"=TRUE, "error in"=w1547) -> ("error out"=w1549:errorcluster)  [unwired: 11 in, 1 out]
          }
        }
        n722 = Merge Errors(w1531, w1536) -> (w1528:errorcluster)
        n723 = call <vilib>:"Add State(s) to Queue__JKI_lib_State_Machine.vi"("State(s) in (\"\")"=w1544) -> ("States Out"=w1543:string)  [unwired: 14 in]
      }
      frame "Digitizer: Config" {
        # "Synchronize is taking time ~3s."
        # "Config  digitizer\nCall subVi to config digitizer"
        n724 = call "FLImDAQ_FGV.vi"() -> ("Read data"=w1572:T5)  [unwired: 10 in, 1 out]
        n725 = Unbundle By Name(w1581) -> ("SysConfigCluster.Ch1Enable?"=w1589:bool, "SysConfigCluster.Ch2Enable?"=w1588:bool, "SysConfigCluster.Ch3Enable?"=w1586:bool, "FLImDAQ"=w1583:T31)
        n726 = Unbundle By Name(w1572) -> ("Digitizer 1"=w1575:refnum<k15>, "Digitizer 2"=w1574:refnum<k15>)
        n727 = property on="Digitizer" class="Bool (strict)"(error in=w1576, "Blinking"=TRUE) -> (error out=w1577:errorcluster)  [unwired: 1 in, 1 out]
        n728 = Or(x=w1589, y=w1588) -> (x .or. y?=w1587:bool)
        n729 = case shown="True" w1587 {
          tunnel: w1583 -> [_ w1602]
          tunnel: w1577 -> [w1598 w1601]
          tunnel: [w1598 w1600] -> w1584
          tunnel: w1575 -> [_ w1599]
          frame False {
          }
          frame True {
            n730 = call "DigitizerConfig.vi"("error in (no error)"=w1601, "FLImDAQ"=w1602, "IVI Refnum in"=w1599) -> ("error out"=w1600:errorcluster)  [unwired: 7 in, 1 out]
          }
        }
        n731 = case shown="True" w1586 {
          tunnel: w1583 -> [_ w1597]
          tunnel: w1584 -> [w1592 w1596]
          tunnel: [w1592 w1595] -> w1560
          tunnel: w1574 -> [_ w1593]
          frame False {
          }
          frame True {
            n732 = call "DigitizerConfig.vi"("Config Trigge(T)r:"=FALSE, "error in (no error)"=w1596, "FLImDAQ"=w1597, "IVI Refnum in"=w1593) -> ("error out"=w1595:errorcluster)  [unwired: 6 in, 1 out]
          }
        }
        n733 = call "Digitizer1_FGV.vi"("error in (no error)"=w1560) -> ("error out"=w1570:errorcluster, "Read data"=w1571:refnum<k15>)  [unwired: 9 in]
        n734 = call <instrlib>:"niScope Get Session Reference.vi"("instrument handle"=w1571, "error in"=w1570) -> ("session reference"=w1564:refnum<k20>, "error out"=w1562:errorcluster)  [unwired: 11 in, 1 out]
        n735 = call "Digitizer2_FGV.vi"("error in (no error)"=w1562) -> ("error out"=w1568:errorcluster, "Read data"=w1569:refnum<k15>)  [unwired: 9 in]
        n736 = call <instrlib>:"niScope Get Session Reference.vi"("instrument handle"=w1569, "error in"=w1568) -> ("session reference"=w1563:refnum<k20>, "error out"=w1561:errorcluster)  [unwired: 11 in, 1 out]
        n737 = Build Array(w1564, w1563) -> (w1567:refnum<k20>[])
        n738 = call <instrlib>:"niTClk Configure For Homogeneous Triggers.vi"("error in (no error)"=w1561, "sessions"=w1567) -> ("error out"=w1566:errorcluster, "sessions out"=w1565:refnum<k20>[])  [unwired: 8 in]
        n739 = call <instrlib>:"niTClk Synchronize.vi"("error in (no error)"=w1566, "sessions"=w1565) -> ("error out"=w1559:errorcluster, "sessions out"=w1557:refnum<k20>[])  [unwired: 8 in]
        n740 = call <userlib>:"Wait (ms)__ogtk.vi"("error in (no error)"=w1559, "milliseconds to wait"=u32 1500) -> ("error out"=w1555:errorcluster)  [unwired: 8 in, 1 out]
        n741 = Unbundle By Name(w1555) -> ("status"=w1580:bool)
        n742 = Not(x=w1580) -> (.not. x?=w1579:bool)
        n743 = Bundle By Name(cluster=w1581, "System Status.Digitizer"=w1579, "niTClk sessions"=w1557) -> (w1582:T24)
        n744 = property on="Digitizer" class="Bool (strict)"(error in=w1555, "Blinking"=FALSE) -> (error out=w1573:errorcluster)  [unwired: 1 in, 1 out]
        n745 = call <vilib>:"Add State(s) to Queue__JKI_lib_State_Machine.vi"("State(s) in (\"\")"=w1591) -> ("States Out"=w1590:string)  [unwired: 14 in]
      }
      frame "Digitizer: Start" {
        # "send trigger to start acquisition loop"
        # "initilize aquisition"
        # "Start Digitizer\n(TClk start)"
        n746 = Unbundle By Name(w1610) -> ("niTClk sessions"=w1609:refnum<k20>[])
        n747 = call <instrlib>:"niTClk Initiate.vi"("error in (no error)"=w1603, "sessions"=w1609) -> ("error out"=w1605:errorcluster)  [unwired: 8 in, 1 out]
        n748 = Generate User Event(priority (normal)=usereventprio."high priority", user event=w1606, event data cluster=TRUE ("event data"), error in=w1605) -> (error out=w1604:errorcluster)  [unwired: 1 out]
        n749 = call <vilib>:"Add State(s) to Queue__JKI_lib_State_Machine.vi"("State(s) in (\"\")"=w1613) -> ("States Out"=w1612:string)  [unwired: 14 in]
      }
      frame "Digitizer: Abort" {
        # "Template Separator\n(You can make a copy of, or modify, this frame)"
        n750 = call "Digitizer1_FGV.vi"("error in (no error)"=w1617, "Operation (Read)"=enum16{"Write", "Read"}."Read" ("Operation")) -> ("error out"=w1624:errorcluster, "Read data"=w1621:refnum<k15>)  [unwired: 8 in]
        n751 = call "Digitizer2_FGV.vi"("error in (no error)"=w1617, "Operation (Read)"=enum16{"Write", "Read"}."Read" ("Operation")) -> ("error out"=w1620:errorcluster, "Read data"=w1622:refnum<k15>)  [unwired: 8 in]
        n752 = Bundle By Name(cluster=w1614, "SysRunning?"=FALSE ("System Status")) -> (w1615:T24)
        n753 = call <instrlib>:"niScope Abort.vi"("instrument handle"=w1621, "error in"=w1624) -> ("error out"=w1626:errorcluster)  [unwired: 12 in, 1 out]
        n754 = call <instrlib>:"niScope Abort.vi"("instrument handle"=w1622, "error in"=w1620) -> ("error out"=w1625:errorcluster)  [unwired: 12 in, 1 out]
        n755 = Merge Errors(w1626, w1625) -> (w1618:errorcluster)
        n756 = call <vilib>:"Add State(s) to Queue__JKI_lib_State_Machine.vi"("State(s) in (\"\")"=w1629) -> ("States Out"=w1628:string)  [unwired: 14 in]
      }
      frame "Digitizer: checkTemp" {
        w1632 = 65.0 ("y")
        w1637 = enum16{"Write", "Read"}."Read" ("Operation")
        # "Template Separator\n(You can make a copy of, or modify, this frame)"
        n757 = call "Digitizer1_FGV.vi"("Operation (Read)"=w1637) -> ("error out"=w1638:errorcluster, "Read data"=w1639:refnum<k15>)  [unwired: 9 in]
        n758 = call "Digitizer2_FGV.vi"("Operation (Read)"=w1637) -> ("error out"=w1635:errorcluster, "Read data"=w1636:refnum<k15>)  [unwired: 9 in]
        n759 = property on="Property Node" class="niScope"(reference=w1636, error in=w1635) -> ("Device Temperature"=w1633)  [unwired: 2 out]
        "Dig2 Temp" <- w1633
        n760 = property on="Property Node" class="niScope"(reference=w1639, error in=w1638) -> ("Device Temperature"=w1634)  [unwired: 2 out]
        "Dig1 Temp" <- w1634
        n761 = Greater?(x=w1634, y=w1632) -> (0:w1631:bool)
        n762 = Greater?(x=w1633, y=w1632) -> (0:w1630:bool)
        n763 = case shown="True" w1631 {
          frame False {
          }
          frame True {
            n764 = One Button Dialog(message="Digitizer 1 over heating!", button name ("OK")="OK") -> ()  [unwired: 1 out]
          }
        }
        n765 = case shown="True" w1630 {
          frame False {
          }
          frame True {
            n766 = One Button Dialog(message="Digitizer 2 over heating!", button name ("OK")="OK") -> ()  [unwired: 1 out]
          }
        }
        n767 = call <vilib>:"Add State(s) to Queue__JKI_lib_State_Machine.vi"("State(s) in (\"\")"=w1644) -> ("States Out"=w1643:string)  [unwired: 14 in]
      }
      frame "Digitizer: Close" {
        # "Close Digitizer"
        n768 = call "Digitizer1_FGV.vi"("error in (no error)"=w1654, "Operation (Read)"=enum16{"Write", "Read"}."Read" ("Operation")) -> ("error out"=w1656:errorcluster, "Read data"=w1660:refnum<k15>)  [unwired: 8 in]
        n769 = call "Digitizer2_FGV.vi"("error in (no error)"=w1654, "Operation (Read)"=enum16{"Write", "Read"}."Read" ("Operation")) -> ("error out"=w1655:errorcluster, "Read data"=w1658:refnum<k15>)  [unwired: 8 in]
        n770 = call <instrlib>:"niScope Close.vi"("instrument handle"=w1660, "error in"=w1656) -> ("error out"=w1653:errorcluster)  [unwired: 13 in]
        n771 = call <instrlib>:"niScope Close.vi"("instrument handle"=w1658, "error in"=w1655) -> ("error out"=w1652:errorcluster)  [unwired: 13 in]
        n772 = Merge Errors(w1653, w1652) -> (w1651:errorcluster)
        n773 = Unbundle By Name(w1651) -> ("status"=w1650:bool)
        n774 = Bundle By Name(cluster=w1661, "System Status.Digitizer"=w1650) -> (w1662:T24)
        n775 = call <vilib>:"Add State(s) to Queue__JKI_lib_State_Machine.vi"("State(s) in (\"\")"=w1664) -> ("States Out"=w1663:string)  [unwired: 14 in]
      }
      frame "---------- LabJack ----------" {
        # "Template Separator\n(You can make a copy of, or modify, this frame)"
        n776 = call <vilib>:"Add State(s) to Queue__JKI_lib_State_Machine.vi"("State(s) in (\"\")"=w1669) -> ("States Out"=w1668:string)  [unwired: 14 in]
      }
      frame "LabJack: checkPedal" {
        # "Template Separator\n(You can make a copy of, or modify, this frame)"
        n777 = Unbundle By Name(w1670) -> ("LJ Pinout.Foot Pedal"=w1674:string)
        n778 = call "LabJack_FGV.vi"("Operation(Read)"=enum16{"Write", "Read"}."Read" ("Operation"), "error in (no error)"=w1672) -> ("error out"=w1676:errorcluster, "Read data"=w1677:i32)  [unwired: 8 in]
        n779 = call "LJM_eReadName.vi"("Handle In"=w1677, "Name"=w1674, "error in"=w1676) -> ("Value"=w1675:dbl, "error out"=w1673:errorcluster)  [unwired: 10 in, 1 out]
        n780 = case shown="1" w1675 {
          tunnel: w1670 -> [w1682 w1685]
          tunnel: [w1682 w1683] -> w1671
          frame 0, Default {
          }
          frame 1 {
            # "If Pedal pressed"
            n781 = Tick Count (ms)() -> (millisecond timer value=w1689:u32)
            n782 = Unbundle By Name(w1685) -> ("Last Trigger"=w1684:u32)
            n783 = Subtract(x=w1689, y=w1684) -> (x-y=w1688:u32)
            n784 = Greater Or Equal?(x=w1688, y=u32 2000) -> (x >= y?=w1686:bool)
            n785 = case shown="True" w1686 {
              tunnel: w1685 -> [w1690 w1691]
              tunnel: w1684 -> [_ _]
              tunnel: [w1690 w1692] -> w1683
              frame False {
              }
              frame True {
                n786 = Tick Count (ms)() -> (millisecond timer value=w1693:u32)
                n787 = Unbundle By Name(w1691) -> ("SysRunning?"=w1694:bool)
                n788 = case shown="False" w1694 {
                  frame False {
                    n789 = property on="StartButton" class="Bool (strict)"("Val(Sgnl)"=TRUE ("Value (Signaling)")) -> ()  [unwired: 2 in, 2 out]
                  }
                  frame True {
                    n790 = property on="StopButton" class="Bool (strict)"("Val(Sgnl)"=TRUE ("Value (Signaling)")) -> ()  [unwired: 2 in, 2 out]
                  }
                }
                n791 = Bundle By Name(cluster=w1691, "Last Trigger"=w1693) -> (w1692:T24)
              }
            }
          }
        }
        n792 = call <vilib>:"Add State(s) to Queue__JKI_lib_State_Machine.vi"("State(s) in (\"\")"=w1681) -> ("States Out"=w1680:string)  [unwired: 14 in]
      }
      frame "LabJack: ZeroV" {
        # "Just Zero V\nDO not update FGV and front panel\nWIll resume from last V"
        # "set bias to 0"
        # "Zero APD bias\n(You can make a copy of, or modify, this frame)"
        n793 = Unbundle By Name(w1699) -> ("LJ Pinout.Ch1 Bias"=w1704:string, "LJ Pinout.Ch2 Bias"=w1703:string, "LJ Pinout.Ch3 Bias"=w1702:string)
        n794 = Build Array(w1704, w1703, w1702) -> (w1701:string[])
        n795 = call "LabJack_FGV.vi"("Operation(Read)"=enum16{"Write", "Read"}."Read" ("Operation"), "error in (no error)"=w1698) -> ("error out"=w1705:errorcluster, "Read data"=w1706:i32)  [unwired: 8 in]
        n796 = call "LJM_eWriteNames.vi"("Handle In"=w1706, "aNames"=w1701, "aValuesIn"=dbl[] [0.0, 0.0, 0.0], "error in"=w1705) -> ("error out"=w1697:errorcluster)  [unwired: 9 in, 2 out]
        n797 = call <vilib>:"Add State(s) to Queue__JKI_lib_State_Machine.vi"("State(s) in (\"\")"=w1710) -> ("States Out"=w1709:string)  [unwired: 14 in]
      }
      frame "LabJack: SetV" {
        w1717 = enum16{"write", "read"}."read" ("action (write)")
        # "set bias to user specifid"
        # "Set APD bias\n(You can make a copy of, or modify, this frame)"
        n798 = Unbundle By Name(w1726) -> ("LJ Pinout.Ch1 Bias"=w1730:string, "LJ Pinout.Ch2 Bias"=w1729:string, "LJ Pinout.Ch3 Bias"=w1728:string, "Ch4 Bias"=w1720)
        n799 = call "V2FGV.vi"("Error In"=w1716, "action(write)"=w1717) -> ("Error Out"=w1714:errorcluster, "V2 out"=w1722:dbl)  [unwired: 8 in]
        n800 = call "V4FGV.vi"("Error In"=w1716, "action(write)"=w1717) -> ("Error Out"=w1712:errorcluster, "V3 out"=w1718:dbl)  [unwired: 8 in]
        n801 = call "V1FGV.vi"("Error In"=w1716, "action (write)"=w1717) -> ("Error Out"=w1715:errorcluster, "V1 out"=w1719:dbl)  [unwired: 8 in]
        n802 = call "V3FGV.vi"("Error In"=w1716, "action(write)"=w1717) -> ("Error Out"=w1713:errorcluster, "V3 out"=w1721:dbl)  [unwired: 8 in]
        n803 = local write "V 3"(w1721) -> ()
        n804 = local write "V 2"(w1722) -> ()
        n805 = local write "V 4"(w1718) -> ()
        n806 = local write "V 1"(w1719) -> ()
        n807 = Build Array(w1730, w1729, w1728, w1720) -> (w1727:string[])
        n808 = call "LabJack_FGV.vi"("Operation(Read)"=enum16{"Write", "Read"}."Read" ("Operation"), "error in (no error)"=w1716) -> ("error out"=w1731:errorcluster, "Read data"=w1732:i32)  [unwired: 8 in]
        n809 = Build Array(w1719, w1722, w1721, w1718) -> (w1723:dbl[])
        n810 = call "LJM_eWriteNames.vi"("Handle In"=w1732, "aNames"=w1727, "aValuesIn"=w1723, "error in"=w1731) -> ("error out"=w1724:errorcluster)  [unwired: 9 in, 2 out]
        n811 = Merge Errors(w1715, w1714, w1713, w1712) -> (w1711:errorcluster)
        n812 = call <vilib>:"Add State(s) to Queue__JKI_lib_State_Machine.vi"("State(s) in (\"\")"=w1736) -> ("States Out"=w1735:string)  [unwired: 14 in]
        n813 = Merge Errors(w1711, w1724) -> (w1725:errorcluster)
      }
      frame "LabJack: Open" {
        # "Initialize LabJack T7\nEstablish connection and initialize pins"
        n814 = call "LJ_Open.vi"("error in"=w1746, 11:"LJM_dtT7" ("DeviceType")) -> ("error out"=w1743:errorcluster, "Success?"=w1744:bool, "Handle Out"=w1738:i32)  [unwired: 7 in]
        n815 = call "LabJack_FGV.vi"("Operation(Read)"=enum16{"Write", "Read"}."Write" ("Operation"), "error in (no error)"=w1743, "Write data"=w1738) -> ("error out"=w1740:errorcluster)  [unwired: 7 in, 1 out]
        n816 = Bundle By Name(cluster=w1741, "System Status.Labjack"=w1744) -> (w1745:T24)
        n817 = call <vilib>:"Add State(s) to Queue__JKI_lib_State_Machine.vi"("State(s) in (\"\")"=w1748) -> ("States Out"=w1747:string)  [unwired: 14 in]
      }
      frame "LabJack: SetDefaultSub" {
        w1758 = enum16{"write", "read"}."write" ("action")
        w1759 = 0.0 ("V1 in")
        w1772 = "_EF_ENABLE" ("string")
        # "1. Disable PWM\n2. Set all V to 0\n3. Set 355 relay to open\n4. Set LED to off"
        # "read once to set DIO to input"
        # "set all initila V to 0. Set footpedal to input. Set PWM to low. Set laser relay to open. Set LEDs to yellow."
        # "Set Labjack to correct input and output state and initial values"
        n818 = disable-structure shown="Disabled" {
          frame Disabled {
            (unwired) dbl[] [0.0, 0.0, 0.0, 0.0, 0.0, 0.0, 0.0, 0.0, 0.0] ("aValuesIn")
          }
          frame Enabled {
          }
        }
        n819 = Unbundle By Name(w1769) -> ("LJ Pinout.355 PWM"=w1774:string, "LJ Pinout.AimingBeam PWM"=w1773:string, "LJ Pinout.Ch1 Bias"=w1779:string, "LJ Pinout.Ch2 Bias"=w1749:string, "LJ Pinout.Ch3 Bias"=w1783:string, "Ch4 Bias"=w1763, "LJ Pinout.Laser Start/Stop"=w1782:string, "LJ Pinout.Red LED"=w1781:string, "LJ Pinout.Green LED"=w1780:string)
        n820 = call "V1FGV.vi"("Error In"=w1767, "action (write)"=w1758, "V1 in"=w1759) -> ("Error Out"=w1762:errorcluster, "V1 out"=w1766:dbl)  [unwired: 7 in]
        n821 = local write "V 1"(w1766) -> ()
        n822 = call "V2FGV.vi"("Error In"=w1762, "action(write)"=w1758, "V2 in"=w1759) -> ("Error Out"=w1761:errorcluster, "V2 out"=w1765:dbl)  [unwired: 7 in]
        n823 = call "LabJack_FGV.vi"("Operation(Read)"=enum16{"Write", "Read"}."Read" ("Operation"), "error in (no error)"=w1767) -> ("error out"=w1755:errorcluster, "Read data"=w1777:i32)  [unwired: 8 in]
        n824 = Concatenate Strings(w1774, w1772) -> (w1771:string)
        n825 = Concatenate Strings(w1773, w1772) -> (w1770:string)
        n826 = local write "V 2"(w1765) -> ()
        n827 = call "V3FGV.vi"("Error In"=w1761, "action(write)"=w1758, "V3 in"=w1759) -> ("Error Out"=w1760:errorcluster, "V3 out"=w1764:dbl)  [unwired: 7 in]
        n828 = Build Array(w1771, w1770, w1779, w1749, w1783, w1763, w1782, w1781, w1780) -> (w1753:string[])
        n829 = local write "V 3"(w1764) -> ()
        n830 = call "V4FGV.vi"("Error In"=w1760, "action(write)"=w1758, "V3 in"=w1759) -> ("Error Out"=w1756:errorcluster, "V3 out"=w1757:dbl)  [unwired: 7 in]
        n831 = Array Size(array=w1753) -> (size(s)=w1752:i32)
        n832 = local write "V 4"(w1757) -> ()
        n833 = Initialize Array(0.0 ("element"), w1752) -> (w1750:dbl[])
        n834 = Unbundle By Name(w1769) -> ("LJ Pinout.Foot Pedal"=w1768:string)
        n835 = call "LJM_eWriteNames.vi"("Handle In"=w1777, "aNames"=w1753, "aValuesIn"=w1750, "error in"=w1755) -> ("Handle Out"=w1776:i32, "error out"=w1775:errorcluster)  [unwired: 9 in, 1 out]
        n836 = call "LJM_eReadName.vi"("Handle In"=w1776, "Name"=w1768, "error in"=w1775) -> ("error out"=w1754:errorcluster)  [unwired: 10 in, 2 out]
        n837 = case shown="Error .." w1754 {
          frame No Error {
            # "no error"
          }
          frame Error {
            # "handle error"
            n838 = One Button Dialog(message="Labjack error! The pin assignment is likely wrong. Please check pin setting of Labjack. Program will terminate.", button name ("OK")="OK") -> ()  [unwired: 1 out]
          }
        }
        n839 = call <vilib>:"Add State(s) to Queue__JKI_lib_State_Machine.vi"("State(s) in (\"\")"=w1786) -> ("States Out"=w1785:string)  [unwired: 14 in]
      }
      frame "LabJack: FootPedalConfig" {
        # "Setup footPedal\n(You can make a copy of, or modify, this frame)"
        n840 = call "LabJack_FGV.vi"("Operation(Read)"=enum16{"Write", "Read"}."Read" ("Operation"), "error in (no error)"=w1790) -> ("error out"=w1794:errorcluster, "Read data"=w1795:i32)  [unwired: 8 in]
        n841 = call "LJM_eWriteName.vi"("Handle In"=w1795, "Name"="DIO15", "Value"=1.0, "error in"=w1794) -> ("error out"=w1791:errorcluster)  [unwired: 10 in, 1 out]
        n842 = call <vilib>:"Add State(s) to Queue__JKI_lib_State_Machine.vi"("State(s) in (\"\")"=w1799) -> ("States Out"=w1798:string)  [unwired: 14 in]
      }
      frame "LabJack: SetDefaultAndClose" {
        # "Template Separator\n(You can make a copy of, or modify, this frame)"
        n843 = call <vilib>:"Add State(s) to Queue__JKI_lib_State_Machine.vi"("State(s) in Front (\"\")"="LabJack: SetDefaultSub\nLabJack: Close" ("State(s) in Front (\"\")"), "State(s) in (\"\")"=w1805) -> ("States Out"=w1804:string)  [unwired: 13 in]
      }
      frame "LabJack: Close" {
        # "Close LabJack Refnum"
        n844 = call "LabJack_FGV.vi"("Operation(Read)"=enum16{"Write", "Read"}."Read" ("Operation"), "error in (no error)"=w1811) -> ("error out"=w1806:errorcluster, "Read data"=w1807:i32)  [unwired: 8 in]
        n845 = Bundle By Name(cluster=w1809, "System Status.Labjack"=FALSE ("System Status.Gain Control")) -> (w1812:T24)
        n846 = call "LJM_Close.vi"("error in"=w1806, "Handle"=w1807) -> ("error out"=w1814:errorcluster)  [unwired: 9 in]
        n847 = call <vilib>:"Add State(s) to Queue__JKI_lib_State_Machine.vi"("State(s) in (\"\")"=w1816) -> ("States Out"=w1815:string)  [unwired: 14 in]
      }
      frame "LabJack: Interlock enable/disable" {
        w1825 = i8 0  # int8
        # "[Covers: REQ8]"
        # "Interlock enable/disable\n(Usage: \"LabJack: Interlock enable/disable >> 1|0\")"
        n848 = Fract/Exp String To Number(string=w1826, default (0 dbl)=w1825) -> (number=w1822:i8)  [unwired: 2 in, 1 out]
        n849 = Unbundle By Name(w1824) -> ("LJ Pinout.Interlock"=w1823:string)
        n850 = call "LabJack_FGV.vi"("Operation(Read)"=enum16{"Write", "Read"}."Read" ("Operation")) -> ("Read data"=w1820:i32)  [unwired: 9 in, 1 out]
        n851 = call "LJM_eWriteName.vi"("Handle In"=w1820, "Name"=w1823, "Value"=w1822, "error in"=w1821) -> ("error out"=w1818:errorcluster)  [unwired: 10 in, 1 out]
        n852 = call <vilib>:"Add State(s) to Queue__JKI_lib_State_Machine.vi"("State(s) in (\"\")"=w1828) -> ("States Out"=w1827:string)  [unwired: 14 in]
      }
      frame "LabJack: 355_PWM_Config" {
        w1830 = 0.0 ("element")
        w1850 = "DIO_EF_CLOCK1_ENABLE"
        # "Config PWM frequency"
        n853 = Unbundle By Name(w1842) -> ("LJ Pinout.355 PWM"=w1849:string)
        n854 = Unbundle By Name(w1842) -> ("355 PWM setting.DIO_EF_CLOCK1_DIVISOR"=w1841:i16, "355 PWM setting.DIO_EF_CLOCK1_ROLL_VALUE"=w1840:i32, "355 PWM setting.DIO#_EF_INDEX"=w1837:i16, "355 PWM setting.DIO#_EF_OPTIONS"=w1836:i16, "355 PWM setting.DIO#_EF_CONFIG_A"=w1835:i32)
        n855 = Concatenate Strings(w1849, "_EF_ENABLE" ("string")) -> (w1845:string)
        n856 = Concatenate Strings(w1849, "_EF_INDEX") -> (w1848:string)
        n857 = Concatenate Strings(w1849, "_EF_OPTIONS") -> (w1847:string)
        n858 = Concatenate Strings(w1849, "_EF_CONFIG_A") -> (w1846:string)
        n859 = call "LabJack_FGV.vi"("Operation(Read)"=enum16{"Write", "Read"}."Read" ("Operation")) -> ("Read data"=w1843:i32)  [unwired: 9 in, 1 out]
        n860 = Build Array(w1830, w1830, w1841, w1840, 1.0 ("element"), 0.0 ("element"), w1837, w1836, w1835) -> (w1834:dbl[])
        n861 = Build Array("DIO_EF_CLOCK0_ENABLE", w1850, "DIO_EF_CLOCK1_DIVISOR", "DIO_EF_CLOCK1_ROLL_VALUE", w1850, w1845, w1848, w1847, w1846) -> (w1844:string[])
        n862 = call "LJM_eWriteNames.vi"("Handle In"=w1843, "aNames"=w1844, "aValuesIn"=w1834, "error in"=w1832) -> ("error out"=w1833:errorcluster)  [unwired: 9 in, 2 out]
        n863 = call <vilib>:"Add State(s) to Queue__JKI_lib_State_Machine.vi"("State(s) in (\"\")"=w1859) -> ("States Out"=w1858:string)  [unwired: 14 in]
      }
      frame "LabJack: 355_PWM_Start" {
        # "Template Separator\n(You can make a copy of, or modify, this frame)"
        n864 = Unbundle By Name(w1867) -> ("LJ Pinout.355 PWM"=w1866:string)
        n865 = call "LabJack_FGV.vi"("Operation(Read)"=enum16{"Write", "Read"}."Read" ("Operation"), "error in (no error)"=w1861) -> ("error out"=w1868:errorcluster, "Read data"=w1869:i32)  [unwired: 8 in]
        n866 = Concatenate Strings(w1866, "_EF_ENABLE" ("string")) -> (w1864:string)
        n867 = call "LJM_eWriteName.vi"("Handle In"=w1869, "Name"=w1864, "Value"=1.0, "error in"=w1868) -> ("error out"=w1862:errorcluster)  [unwired: 10 in, 1 out]
        n868 = call <vilib>:"Add State(s) to Queue__JKI_lib_State_Machine.vi"("State(s) in (\"\")"=w1872) -> ("States Out"=w1871:string)  [unwired: 14 in]
      }
      frame "LabJack: 355_PWM_Stop" {
        # "Template Separator\n(You can make a copy of, or modify, this frame)"
        n869 = Unbundle By Name(w1878) -> ("LJ Pinout.355 PWM"=w1882:string)
        n870 = call "LabJack_FGV.vi"("Operation(Read)"=enum16{"Write", "Read"}."Read" ("Operation"), "error in (no error)"=w1877) -> ("error out"=w1883:errorcluster, "Read data"=w1875:i32)  [unwired: 8 in]
        n871 = Concatenate Strings(w1882, "_EF_ENABLE" ("string")) -> (w1880:string)
        n872 = call "LJM_eWriteName.vi"("Handle In"=w1875, "Name"=w1880, "Value"=0.0, "error in"=w1883) -> ("error out"=w1874:errorcluster)  [unwired: 10 in, 1 out]
        n873 = local write "355nm Laser toggle"(FALSE ("355nm Laser toggle")) -> ()
        n874 = call <vilib>:"Add State(s) to Queue__JKI_lib_State_Machine.vi"("State(s) in (\"\")"=w1886) -> ("States Out"=w1885:string)  [unwired: 14 in]
      }
      frame "LabJack: AB_Start" {
        # "Aiming Beam Start\n(Based on aimging beam frequency, set LabJack pin)"
        n875 = Unbundle By Name(w1896) -> ("AB Cluster.Freq"=w1888:i32, "LJ Pinout.AimingBeam PWM"=w1895:string)
        n876 = Greater Than 0?(x=w1888) -> (x > 0?=w1887:bool)
        n877 = case shown="False" w1887 {
          tunnel: w1895 -> [w1902 w1905]
          tunnel: [w1902 w1903] -> w1894
          frame False {
            # "if 0 freq, set PWM pin"
          }
          frame True {
            # "if non zero freq, set PWM enable"
            n878 = Concatenate Strings(w1905, "_EF_ENABLE" ("string")) -> (w1903:string)
          }
        }
        n879 = call "LabJack_FGV.vi"("Operation(Read)"=enum16{"Write", "Read"}."Read" ("Operation"), "error in (no error)"=w1891) -> ("error out"=w1897:errorcluster, "Read data"=w1898:i32)  [unwired: 8 in]
        n880 = call "LJM_eWriteName.vi"("Handle In"=w1898, "Name"=w1894, "Value"=1.0, "error in"=w1897) -> ("error out"=w1892:errorcluster)  [unwired: 10 in, 1 out]
        n881 = local write "Aiming beam toggle"(TRUE ("Aiming beam toggle")) -> ()
        n882 = call <vilib>:"Add State(s) to Queue__JKI_lib_State_Machine.vi"("State(s) in (\"\")"=w1901) -> ("States Out"=w1900:string)  [unwired: 14 in]
      }
      frame "LabJack: AB_Stop" {
        # "Aiming Beam Stop\n(Based on aiming beam frequency, set LabJack pin low)"
        n883 = Unbundle By Name(w1913) -> ("AB Cluster.Freq"=w1908:i32, "LJ Pinout.AimingBeam PWM"=w1915:string)
        n884 = Greater Than 0?(x=w1908) -> (x > 0?=w1907:bool)
        n885 = case shown="False" w1907 {
          tunnel: w1915 -> [w1921 w1924]
          tunnel: [w1921 w1922] -> w1906
          frame False {
          }
          frame True {
            n886 = Concatenate Strings(w1924, "_EF_ENABLE" ("string")) -> (w1922:string)
          }
        }
        n887 = call "LabJack_FGV.vi"("Operation(Read)"=enum16{"Write", "Read"}."Read" ("Operation"), "error in (no error)"=w1911) -> ("error out"=w1916:errorcluster, "Read data"=w1917:i32)  [unwired: 8 in]
        n888 = call "LJM_eWriteName.vi"("Handle In"=w1917, "Name"=w1906, "Value"=0.0, "error in"=w1916) -> ("error out"=w1912:errorcluster)  [unwired: 10 in, 1 out]
        n889 = local write "Aiming beam toggle"(FALSE ("Aiming beam toggle")) -> ()
        n890 = call <vilib>:"Add State(s) to Queue__JKI_lib_State_Machine.vi"("State(s) in (\"\")"=w1920) -> ("States Out"=w1919:string)  [unwired: 14 in]
      }
      frame "LabJack: AB_PWM_Config" {
        w1926 = 0.0 ("element")
        w1946 = "DIO_EF_CLOCK2_ENABLE"
        # "Config PWM frequency"
        n891 = Unbundle By Name(w1938) -> ("LJ Pinout.AimingBeam PWM"=w1945:string)
        n892 = Unbundle By Name(w1938) -> ("AB PWM setting.DIO_EF_CLOCK1_DIVISOR"=w1937:i16, "AB PWM setting.DIO_EF_CLOCK1_ROLL_VALUE"=w1936:i32, "AB PWM setting.DIO#_EF_INDEX"=w1933:i16, "AB PWM setting.DIO#_EF_OPTIONS"=w1932:i16, "AB PWM setting.DIO#_EF_CONFIG_A"=w1931:i32)
        n893 = Concatenate Strings(w1945, "_EF_ENABLE" ("string")) -> (w1941:string)
        n894 = Concatenate Strings(w1945, "_EF_INDEX") -> (w1944:string)
        n895 = Concatenate Strings(w1945, "_EF_OPTIONS") -> (w1943:string)
        n896 = Concatenate Strings(w1945, "_EF_CONFIG_A") -> (w1942:string)
        n897 = call "LabJack_FGV.vi"("Operation(Read)"=enum16{"Write", "Read"}."Read" ("Operation")) -> ("Read data"=w1939:i32)  [unwired: 9 in, 1 out]
        n898 = Build Array(w1926, w1926, w1937, w1936, 1.0 ("element"), 0.0 ("element"), w1933, w1932, w1931) -> (w1930:dbl[])
        n899 = Build Array("DIO_EF_CLOCK0_ENABLE", w1946, "DIO_EF_CLOCK2_DIVISOR", "DIO_EF_CLOCK2_ROLL_VALUE", w1946, w1941, w1944, w1943, w1942) -> (w1940:string[])
        n900 = call "LJM_eWriteNames.vi"("Handle In"=w1939, "aNames"=w1940, "aValuesIn"=w1930, "error in"=w1928) -> ("error out"=w1929:errorcluster)  [unwired: 9 in, 2 out]
        n901 = call <vilib>:"Add State(s) to Queue__JKI_lib_State_Machine.vi"("State(s) in (\"\")"=w1955) -> ("States Out"=w1954:string)  [unwired: 14 in]
      }
      frame "---------- LED ----------" {
        # "Template Separator\n(You can make a copy of, or modify, this frame)"
        n902 = call <vilib>:"Add State(s) to Queue__JKI_lib_State_Machine.vi"("State(s) in (\"\")"=w1960) -> ("States Out"=w1959:string)  [unwired: 14 in]
      }
      frame "LED: OpenVIRef" {
        # "Template Separator\n(You can make a copy of, or modify, this frame)"
        n903 = call <vilib>:"Application Directory.vi"() -> ("Application Directory"=w1967:path)
        n904 = Build Path(base path=w1967, name or relative path="SubVI") -> (appended path=w1965:path)
        n905 = Build Path(base path=w1965, name or relative path="LEDBreath.vi") -> (appended path=w1963:path)
        n906 = Open VI Reference(vi path=w1963, error in (no error)=w1968) -> (vi reference=w1969:refnum<vi>, error out=w1962:errorcluster)  [unwired: 4 in]
        n907 = case shown="Error .." w1962 {
          tunnel: [TRUE FALSE] -> w1961
          frame No Error {
          }
          frame Error {
          }
        }
        n908 = Bundle By Name(cluster=w1970, "LED vi reference"=w1969, "LED vi ref open?"=w1961) -> (w1971:T24)
        n909 = call <vilib>:"Add State(s) to Queue__JKI_lib_State_Machine.vi"("State(s) in (\"\")"=w1974) -> ("States Out"=w1973:string)  [unwired: 14 in]
      }
      frame "LED: CloseVIRef" {
        # "Template Separator\n(You can make a copy of, or modify, this frame)"
        n910 = Unbundle By Name(w1978) -> ("LED vi reference"=w1979:refnum<vi>, "LED vi ref open?"=w1977:bool)
        n911 = case shown="True" w1977 {
          tunnel: w1981 -> [w1985 w1988]
          tunnel: [w1985 w1987] -> w1980
          tunnel: w1979 -> [_ w1986]
          frame False {
          }
          frame True {
            n912 = Close Reference(reference=w1986, error in (no error)=w1988) -> (error out=w1987:errorcluster)
          }
        }
        n913 = call <vilib>:"Add State(s) to Queue__JKI_lib_State_Machine.vi"("State(s) in (\"\")"=w1984) -> ("States Out"=w1983:string)  [unwired: 14 in]
      }
      frame "LED: BreathGreen" {
        w1989 = FALSE ("Wait Until Done")
        # "Breath system LED\n(LED: Breath >> True/False)"
        n914 = Unbundle By Name(w1997) -> ("LED vi reference"=w1996:refnum<vi>)
        n915 = invoke class="VI" method="Ctrl Val.Set"(reference=w1996, error in=w1994, "Control Name"="Color", "Value"=0) -> (reference out=w1993:refnum<vi>, error out=w1992:errorcluster)  [unwired: 1 in, 3 out]
        n916 = invoke on="Invoke Node" class="VI" method="Run VI"(reference=w1993, error in=w1992, "Wait until done"=w1989, "Auto Dispose Ref"=w1989) -> (error out=w1995:errorcluster)  [unwired: 1 in, 4 out]
        n917 = call <vilib>:"Add State(s) to Queue__JKI_lib_State_Machine.vi"("State(s) in (\"\")"=w2000) -> ("States Out"=w1999:string)  [unwired: 14 in]
      }
      frame "LED: BreathOrange" {
        w2001 = FALSE ("Wait Until Done")
        # "Breath system LED\n(LED: Breath >> True/False)"
        n918 = Unbundle By Name(w2009) -> ("LED vi reference"=w2008:refnum<vi>)
        n919 = invoke class="VI" method="Ctrl Val.Set"(reference=w2008, error in=w2006, "Control Name"="Color", "Value"=1) -> (reference out=w2005:refnum<vi>, error out=w2004:errorcluster)  [unwired: 1 in, 3 out]
        n920 = invoke on="Invoke Node" class="VI" method="Run VI"(reference=w2005, error in=w2004, "Wait until done"=w2001, "Auto Dispose Ref"=w2001) -> (error out=w2007:errorcluster)  [unwired: 1 in, 4 out]
        n921 = call <vilib>:"Add State(s) to Queue__JKI_lib_State_Machine.vi"("State(s) in (\"\")"=w2012) -> ("States Out"=w2011:string)  [unwired: 14 in]
      }
      frame "LED: BreathOff" {
        # "System LED Breath Off\n(Breath off, check VI status to make sure it is off)"
        n922 = Unbundle By Name(w2021) -> ("LED vi reference"=w2020:refnum<vi>)
        n923 = invoke on="Invoke Node" class="VI" method="Ctrl Val.Set"(reference=w2020, error in=w2018, "Control Name"="Stop", "Value"=TRUE) -> (reference out=w2013:refnum<vi>, error out=w2014:errorcluster)  [unwired: 1 in, 3 out]
        n924 = case shown="No Error" w2014 {
          selector: w2014 -> [w2026 _]
          tunnel: [w2025 errorcluster {"status"=FALSE, "code"=0, "source"=""} ("error IO")] -> w2019
          tunnel: ["" ("State(s) in Front (\"\")") "LED: BreathOff" ("State(s) in Front (\"\")")] -> w2017
          tunnel: w2013 -> [w2027 _]
          frame No Error {
            # "No error, wait for VI to stop"
            n925 = while {
              tunnel: w2027 -> [w2035]
              shift-right: [w2029] -> w2025
              shift-left: w2026 -> [w2034]
              stop <- w2031 stop-if-true
              # "continue check whether vi is running"
              n926 = property class="VI"(reference=w2035, error in=w2034) -> (error out=w2029:errorcluster, "Exec.State"=w2033:T21)  [unwired: 1 out]
              n927 = Wait (ms)(milliseconds to wait=u32 50) -> ()  [unwired: 1 out]
              n928 = Equal?(x=w2033, y=T21."Idle") -> (x = y?=w2031:bool)
            }
          }
          frame Error {
            # "try again when error"
          }
        }
        n929 = call <vilib>:"Add State(s) to Queue__JKI_lib_State_Machine.vi"("State(s) in Front (\"\")"=w2017, "State(s) in (\"\")"=w2024) -> ("States Out"=w2023:string)  [unwired: 13 in]
      }
      frame "LED: Off" {
        # "set LED to red"
        # "Template Separator\n(You can make a copy of, or modify, this frame)"
        n930 = Unbundle By Name(w2040) -> ("LJ Pinout.Red LED"=w2039:string, "LJ Pinout.Green LED"=w2038:string)
        n931 = call "LabJack_FGV.vi"("Operation(Read)"=enum16{"Write", "Read"}."Read" ("Operation"), "error in (no error)"=w2041) -> ("error out"=w2048:errorcluster, "Read data"=w2047:i32)  [unwired: 8 in]
        n932 = call "LJM_eWriteName.vi"("Handle In"=w2047, "Name"=w2039, "Value"=0.0, "error in"=w2048) -> ("Handle Out"=w2045:i32, "error out"=w2044:errorcluster)  [unwired: 10 in]
        n933 = call "LJM_eWriteName.vi"("Handle In"=w2045, "Name"=w2038, "Value"=0.0, "error in"=w2044) -> ("error out"=w2042:errorcluster)  [unwired: 10 in, 1 out]
        n934 = call <vilib>:"Add State(s) to Queue__JKI_lib_State_Machine.vi"("State(s) in (\"\")"=w2052) -> ("States Out"=w2051:string)  [unwired: 14 in]
      }
      frame "LED: Green" {
        # "set LED to green"
        # "Template Separator\n(You can make a copy of, or modify, this frame)"
        n935 = Unbundle By Name(w2056) -> ("LJ Pinout.Red LED"=w2054:string, "LJ Pinout.Green LED"=w2055:string)
        n936 = call "LabJack_FGV.vi"("Operation(Read)"=enum16{"Write", "Read"}."Read" ("Operation"), "error in (no error)"=w2058) -> ("error out"=w2064:errorcluster, "Read data"=w2063:i32)  [unwired: 8 in]
        n937 = call "LJM_eWriteName.vi"("Handle In"=w2063, "Name"=w2054, "Value"=0.0, "error in"=w2064) -> ("Handle Out"=w2061:i32, "error out"=w2060:errorcluster)  [unwired: 10 in]
        n938 = call "LJM_eWriteName.vi"("Handle In"=w2061, "Name"=w2055, "Value"=9.0, "error in"=w2060) -> ("error out"=w2057:errorcluster)  [unwired: 10 in, 1 out]
        n939 = call <vilib>:"Add State(s) to Queue__JKI_lib_State_Machine.vi"("State(s) in (\"\")"=w2067) -> ("States Out"=w2066:string)  [unwired: 14 in]
      }
      frame "---------- Queue ----------" {
        # "Template Separator\n(You can make a copy of, or modify, this frame)"
        n940 = call <vilib>:"Add State(s) to Queue__JKI_lib_State_Machine.vi"("State(s) in (\"\")"=w2072) -> ("States Out"=w2071:string)  [unwired: 14 in]
      }
      frame "Queue: Flash" {
        # "Clear queue contnet\n(clear queue content by flash it)"
        n941 = Flush Queue(queue=w2079, error in (no error)=w2073) -> (error out=w2077:errorcluster)  [unwired: 2 out]
        n942 = Flush Queue(queue=w2080, error in (no error)=w2073) -> (error out=w2076:errorcluster)  [unwired: 2 out]
        n943 = Flush Queue(queue=w2078, error in (no error)=w2073) -> (error out=w2075:errorcluster)  [unwired: 2 out]
        n944 = Merge Errors(w2077, w2076, w2075) -> (w2074:errorcluster)
        n945 = call <vilib>:"Add State(s) to Queue__JKI_lib_State_Machine.vi"("State(s) in (\"\")"=w2084) -> ("States Out"=w2083:string)  [unwired: 14 in]
      }
      frame "Queue: Destory" {
        # "Destory Data Queue\nDistory data queue ref so the aquisition loop stop"
        n946 = Release Queue(queue=w2090, error in (no error)=w2086) -> (error out=w2093:errorcluster)  [unwired: 1 in, 2 out]
        n947 = Release Queue(queue=w2089, error in (no error)=w2086) -> (error out=w2092:errorcluster)  [unwired: 1 in, 2 out]
        n948 = Release Queue(queue=w2087, error in (no error)=w2086) -> (error out=w2085:errorcluster)  [unwired: 1 in, 2 out]
        n949 = Merge Errors(w2093, w2092, w2085) -> (w2091:errorcluster)
        n950 = call <vilib>:"Simple Error Handler.vi"("error in (no error)"=w2091) -> ()  [unwired: 4 in, 5 out]
        n951 = call <vilib>:"Add State(s) to Queue__JKI_lib_State_Machine.vi"("State(s) in (\"\")"=w2096) -> ("States Out"=w2095:string)  [unwired: 14 in]
      }
      frame "---------- Run ----------" {
        # "Template Separator\n(You can make a copy of, or modify, this frame)"
        n952 = call <vilib>:"Add State(s) to Queue__JKI_lib_State_Machine.vi"("State(s) in (\"\")"=w2101) -> ("States Out"=w2100:string)  [unwired: 14 in]
      }
      frame "Run: CaliIncrement" {
        # "Increment Calibration #\n(You can make a copy of, or modify, this frame)"
        n953 = Unbundle By Name(w2103) -> ("IDs.Cali ID"=w2105:i8)
        n954 = Increment(x=w2105) -> (x+1=w2102:i8)
        n955 = Bundle By Name(cluster=w2103, "IDs.Cali ID"=w2102) -> (w2104:T24)
        n956 = call <vilib>:"Add State(s) to Queue__JKI_lib_State_Machine.vi"("State(s) in (\"\")"=w2109) -> ("States Out"=w2108:string)  [unwired: 14 in]
      }
      frame "Run: BGIncrement" {
        # "Increment BG #\n(You can make a copy of, or modify, this frame)"
        n957 = Unbundle By Name(w2110) -> ("IDs.BG ID"=w2113:i8)
        n958 = Increment(x=w2113) -> (x+1=w2112:i8)
        n959 = Bundle By Name(cluster=w2110, "IDs.BG ID"=w2112) -> (w2111:T24)
        n960 = call <vilib>:"Add State(s) to Queue__JKI_lib_State_Machine.vi"("State(s) in (\"\")"=w2117) -> ("States Out"=w2116:string)  [unwired: 14 in]
      }
      frame "Run: Increment" {
        # "Increase Run# by 1"
        n961 = Unbundle By Name(w2122) -> ("IDs.RunID"=w2124:i8)
        n962 = Increment(x=w2124) -> (x+1=w2120:i8)
        n963 = Bundle By Name(cluster=w2122, "IDs.RunID"=w2120) -> (w2123:T24)
        n964 = call "RunIDFGV.vi"("Error In"=w2118, "RunID in"=w2120) -> ("Error Out"=w2119:errorcluster)  [unwired: 8 in, 1 out]
        n965 = call <vilib>:"Add State(s) to Queue__JKI_lib_State_Machine.vi"("State(s) in (\"\")"=w2126) -> ("States Out"=w2125:string)  [unwired: 14 in]
      }
      frame "Run: Decrement" {
        # "Increase Run# by 1"
        n966 = Unbundle By Name(w2131) -> ("IDs.RunID"=w2133:i8)
        n967 = Decrement(x=w2133) -> (x-1=w2129:i8)
        n968 = Bundle By Name(cluster=w2131, "IDs.RunID"=w2129) -> (w2132:T24)
        n969 = call "RunIDFGV.vi"("Error In"=w2127, "RunID in"=w2129) -> ("Error Out"=w2128:errorcluster)  [unwired: 8 in, 1 out]
        n970 = call <vilib>:"Add State(s) to Queue__JKI_lib_State_Machine.vi"("State(s) in (\"\")"=w2135) -> ("States Out"=w2134:string)  [unwired: 14 in]
      }
      frame "---------- SysConfig ----------" {
        # "Template Separator\n(You can make a copy of, or modify, this frame)"
        n971 = call <vilib>:"Add State(s) to Queue__JKI_lib_State_Machine.vi"("State(s) in (\"\")"=w2140) -> ("States Out"=w2139:string)  [unwired: 14 in]
      }
      frame "SysConfig: LoadAPDSerialNumber" {
        # "Template Separator\n(You can make a copy of, or modify, this frame)"
        n972 = call "readAPDSerial.vi"("Error In"=w2142) -> ("Error Out"=w2141:errorcluster, "output cluster"=w2143:T42)  [unwired: 9 in]
        n973 = Bundle By Name(cluster=w2144, "APDSerialNum"=w2143) -> (w2145:T24)
        n974 = call <vilib>:"Add State(s) to Queue__JKI_lib_State_Machine.vi"("State(s) in (\"\")"=w2148) -> ("States Out"=w2147:string)  [unwired: 14 in]
      }
      frame "SysConfig: Load Sys Config" {
        # "[Covers: REQ5]"
        # "Load System config"
        # "Load system configuration\n(Load both hardware and DAQ config)"
        n975 = call "LoadSysConfig.vi"("Error In"=w2151, "Enum"=enum16{"LastUse", "Default"}."LastUse") -> ("Error Out"=w2150:errorcluster, "SysConfigCluster"=w2153:T7)  [unwired: 8 in]
        "SysConfigCluster" <- w2153
        n976 = Bundle By Name(cluster=w2154, "SysConfigCluster"=w2153) -> (w2155:T24)
        n977 = call <vilib>:"Add State(s) to Queue__JKI_lib_State_Machine.vi"("State(s) in (\"\")"=w2157) -> ("States Out"=w2156:string)  [unwired: 14 in]
      }
      frame "SysConfig: Load Digitizer Setting" {
        w2158 = enum16{"Write", "Read"}."Write" ("Operation")
        # "Load DAQ config\nSave to FGV"
        # "Template Separator\n(You can make a copy of, or modify, this frame)"
        n978 = call <userlib>:"Current VIs Parent Directory__ogtk.vi"() -> ("Parent Directory (+ Relative)"=w2172:path)  [unwired: 5 in]
        n979 = Build Path(base path=w2172, name or relative path="SubVI\\DigitizerConfiguration\\V6_Scope_last_use.config") -> (appended path=w2173:path)
        n980 = call "ReadDigitizerConfig(SubVI).vi"("error in (no error)"=w2170, "appended path"=w2173) -> ("error out"=w2166:errorcluster, "FLImDAQ"=w2164:T5)  [unwired: 8 in]
        n981 = call "FLImDAQ_FGV.vi"("error in (no error)"=w2166, "Operation (Read)"=w2158, "Write data"=w2164) -> ("error out"=w2168:errorcluster)  [unwired: 7 in, 1 out]
        n982 = Unbundle By Name(w2164) -> ("min record length"=→"data length":i32, "Digitizer 1"=w2160:refnum<k15>, "Digitizer 2"=w2167:refnum<k15>)
        n983 = Bundle By Name(cluster=w2162, "FLImDAQ"=w2164) -> (w2163:T24)
        n984 = call "Digitizer1_FGV.vi"("error in (no error)"=w2168, "Operation (Read)"=w2158, "Write data"=w2160) -> ("error out"=w2169:errorcluster)  [unwired: 7 in, 1 out]
        n985 = call "Digitizer2_FGV.vi"("error in (no error)"=w2169, "Operation (Read)"=w2158, "Write data"=w2167) -> ("error out"=w2165:errorcluster)  [unwired: 7 in, 1 out]
        n986 = call <vilib>:"Add State(s) to Queue__JKI_lib_State_Machine.vi"("State(s) in (\"\")"=w2175) -> ("States Out"=w2174:string)  [unwired: 14 in]
      }
      frame "SysConfig: Load LJ Pinout" {
        # "Template Separator\n(You can make a copy of, or modify, this frame)"
        n987 = call <userlib>:"Current VIs Parent Directory__ogtk.vi"() -> ("Parent Directory (+ Relative)"=w2190:path)  [unwired: 5 in]
        n988 = Build Path(base path=w2190, name or relative path="SubVI\\LabJack\\LJ_pin_setting.config") -> (appended path=w2188:path)
        n989 = call "ReadLabjackConfig(SubVI).vi"("error in (no error)"=w2186, "appended path"=w2188) -> ("error out"=w2187:errorcluster, "Utility"=w2184:T4)  [unwired: 8 in]
        n990 = Unbundle By Name(w2184) -> ("Ch1 Bias"=w2183:string, "Ch2 Bias"=w2182:string, "Ch3 Bias"=w2181:string, "Ch4 Bias"=w2176:string, "Red LED"=w2178:string, "Green LED"=w2177:string)
        n991 = global write "GlobalVariables.vi" "LED Green pin"(w2177) -> ()
        n992 = global write "GlobalVariables.vi" "Ch1 LJ pin"(w2183) -> ()
        n993 = global write "GlobalVariables.vi" "Ch2 LJ pin"(w2182) -> ()
        n994 = global write "GlobalVariables.vi" "Ch3 LJ pin"(w2181) -> ()
        n995 = global write "GlobalVariables.vi" "Ch4 LJ pin"(w2176) -> ()
        n996 = global write "GlobalVariables.vi" "LED Red pin"(w2178) -> ()
        n997 = Bundle By Name(cluster=w2179, "LJ Pinout"=w2184) -> (w2185:T24)
        n998 = call <vilib>:"Add State(s) to Queue__JKI_lib_State_Machine.vi"("State(s) in (\"\")"=w2192) -> ("States Out"=w2191:string)  [unwired: 14 in]
      }
      frame "SysConfig: Load 355 PWM" {
        # "Template Separator\n(You can make a copy of, or modify, this frame)"
        n999 = call <userlib>:"Current VIs Parent Directory__ogtk.vi"() -> ("Parent Directory (+ Relative)"=w2210:path)  [unwired: 5 in]
        n1000 = Build Path(base path=w2210, name or relative path="SubVI\\LabJack\\PWM_setting_355.config") -> (appended path=w2208:path)
        n1001 = call "ReadPWMConfig(SubVI).vi"("error in (no error)"=w2205, "appended path"=w2208) -> ("error out"=w2206:errorcluster, "PWM Setting"=w2204:T43)  [unwired: 8 in]
        n1002 = Unbundle By Name(w2204) -> ("DIO_EF_CLOCK1_DIVISOR"=w2201:i16, "DIO_EF_CLOCK1_ROLL_VALUE"=w2200:i32)
        n1003 = Multiply(x=w2201, y=w2200) -> (x*y=w2202:i32)
        n1004 = Bundle By Name(cluster=w2207, "355 PWM setting"=w2204) -> (w2194:T24)
        n1005 = Divide(x=80000000.0, y=w2202) -> (x/y=w2199:dbl)
        "Laser Rep Rate" <- w2199
        n1006 = Number To Decimal String(number=w2199) -> (decimal integer string=w2198:string)  [unwired: 1 in]
        n1007 = Concatenate Strings("355nm " ("string"), w2198, "Hz" ("string")) -> (w2196:string)
        n1008 = property on="355nm Laser toggle" class="Bool (strict)"("Caption.Text"=w2196) -> ()  [unwired: 2 in, 2 out]
        n1009 = call <vilib>:"Add State(s) to Queue__JKI_lib_State_Machine.vi"("State(s) in (\"\")"=w2212) -> ("States Out"=w2211:string)  [unwired: 14 in]
      }
      frame "SysConfig: Load AB PWM" {
        # "Template Separator\n(You can make a copy of, or modify, this frame)"
        n1010 = call <userlib>:"Current VIs Parent Directory__ogtk.vi"() -> ("Parent Directory (+ Relative)"=w2221:path)  [unwired: 5 in]
        n1011 = Build Path(base path=w2221, name or relative path="SubVI\\LabJack\\PWM_setting_AB.config") -> (appended path=w2219:path)
        n1012 = call "ReadPWMConfig(SubVI).vi"("error in (no error)"=w2216, "appended path"=w2219) -> ("error out"=w2217:errorcluster, "PWM Setting"=w2215:T43)  [unwired: 8 in]
        n1013 = Bundle By Name(cluster=w2213, "AB PWM setting"=w2215) -> (w2218:T24)
        n1014 = call <vilib>:"Add State(s) to Queue__JKI_lib_State_Machine.vi"("State(s) in (\"\")"=w2223) -> ("States Out"=w2222:string)  [unwired: 14 in]
      }
      frame "SysConfig: Load AB setting" {
        # "load aming beam setting\n(check frequency, if 0 do nothing, if not zero, config PWM)"
        n1015 = call "readAimingBeamSetting.vi"("error in (no error)"=w2237) -> ("error out"=w2232:errorcluster, "Aiming Beam Setting"=w2225:T44)  [unwired: 9 in]
        n1016 = Unbundle By Name(w2225) -> ("Frequency(Hz)"=w2224:u32)
        n1017 = Equal To 0?(x=w2224) -> (x = 0?=w2230:bool)
        n1018 = Select(t="", s=w2230, f="SysConfig: Load AB PWM" ("State(s) in Front (\"\")")) -> (s? t:f=w2233:string)
        n1019 = Number To Decimal String(number=w2224) -> (decimal integer string=w2229:string)  [unwired: 1 in]
        n1020 = Concatenate Strings("488nm " ("string"), w2229, "Hz " ("string")) -> (w2228:string)
        n1021 = property on="Aiming beam toggle" class="Bool (strict)"("Caption.Text"=w2228) -> ()  [unwired: 2 in, 2 out]
        n1022 = case shown="False" w2230 {
          tunnel: w2232 -> [w2245 w2248]
          tunnel: [w2244 w2248] -> w2231
          tunnel: w2224 -> [w2243 _]
          frame False {
            n1023 = call "LJ_calculate_PWM_parameters.vi"(7:u32 10 ("Duty Cycle (%)"), "Error In"=w2245, "Show Confirmation"=FALSE, "Laser Rep Rate (Hz)"=w2243, "Laser"=enum16{"355nm", "AimingBeam"}."AimingBeam") -> ("Error Out"=w2244:errorcluster)  [unwired: 5 in, 1 out]
          }
          frame True {
          }
        }
        n1024 = Bundle By Name(cluster=w2238, "AB Cluster"=w2225) -> (w2239:T24)
        n1025 = call <vilib>:"Add State(s) to Queue__JKI_lib_State_Machine.vi"("State(s) in Front (\"\")"=w2233, "State(s) in (\"\")"=w2241) -> ("States Out"=w2240:string)  [unwired: 13 in]
      }
      frame "SysConfig: LoadABVideoSetting" {
        # "Load AB video setting form ini file\n()"
        n1026 = call "readVideoConfig.vi"("error in (no error)"=w2252) -> ("error out"=w2253:errorcluster, "Aiming Beam Config"=w2251:T23)  [unwired: 8 in, 1 out]
        n1027 = Bundle By Name(cluster=w2249, "VideoConfig"=w2251) -> (w2250:T24)
        n1028 = call <vilib>:"Add State(s) to Queue__JKI_lib_State_Machine.vi"("State(s) in (\"\")"=w2256) -> ("States Out"=w2255:string)  [unwired: 14 in]
      }
      frame "SysConfig: LoadCursorLocation" {
        # "Load cursor location from ini file\n(load cursor from system setting ini file)"
        n1029 = call "readCursorConfigMain.vi"("error in (no error)"=w2268) -> ("error out"=w2269:errorcluster, "Cursor Locations"=w2267:T45)  [unwired: 9 in]
        n1030 = Unbundle By Name(w2267) -> ("DC1"=w2266:i32, "DC2"=w2265:i32, "BG1"=w2260:i32, "BG2"=w2259:i32)
        n1031 = Build Array(w2266, w2265) -> (w2264:i32[])
        n1032 = Build Array(w2260, w2259) -> (w2261:i32[])
        n1033 = Array Max & Min(array=w2264) -> (max value=w2263:i32, min value=w2262:i32)  [unwired: 2 out]
        n1034 = Array Max & Min(array=w2261) -> (max value=w2258:i32, min value=w2257:i32)  [unwired: 2 out]
        n1035 = global write "GlobalVariables.vi" "DC Idx2"(w2263) -> ()
        n1036 = global write "GlobalVariables.vi" "DC Idx1"(w2262) -> ()
        n1037 = global write "GlobalVariables.vi" "BG Idx2"(w2258) -> ()
        n1038 = global write "GlobalVariables.vi" "BG Idx1"(w2257) -> ()
        n1039 = call <vilib>:"Add State(s) to Queue__JKI_lib_State_Machine.vi"("State(s) in (\"\")"=w2273) -> ("States Out"=w2272:string)  [unwired: 14 in]
      }
      frame "---------- SystemStatus ----------" {
        # "Template Separator\n(You can make a copy of, or modify, this frame)"
        n1040 = call <vilib>:"Add State(s) to Queue__JKI_lib_State_Machine.vi"("State(s) in (\"\")"=w2278) -> ("States Out"=w2277:string)  [unwired: 14 in]
      }
      frame "SystemStatus: SlowSysStatusMacro" {
        # "store system check time"
        # "Template Separator\n(You can make a copy of, or modify, this frame)"
        n1041 = Tick Count (ms)() -> (millisecond timer value=w2281:u32)
        n1042 = Bundle By Name(cluster=w2279, "SlowTimer"=w2281) -> (w2280:T24)
        n1043 = call <vilib>:"Add State(s) to Queue__JKI_lib_State_Machine.vi"("State(s) in Front (\"\")"="Digitizer: checkTemp\nTCP: CheckConnection" ("State(s) in Front (\"\")"), "State(s) in (\"\")"=w2286) -> ("States Out"=w2285:string)  [unwired: 13 in]
      }
      frame "SystemStatus: FastSysStatusMacro" {
        # "store system check time"
        # "Template Separator\n(You can make a copy of, or modify, this frame)"
        n1044 = Tick Count (ms)() -> (millisecond timer value=w2289:u32)
        n1045 = Bundle By Name(cluster=w2287, "FastTimer"=w2289) -> (w2288:T24)
        n1046 = call <vilib>:"Add State(s) to Queue__JKI_lib_State_Machine.vi"("State(s) in Front (\"\")"="355 Laser: CheckPWMStatus\nAimingBeam: GetPWMStatus\n/*355 Laser: CheckControllerStatus" ("State(s) in Front (\"\")"), "State(s) in (\"\")"=w2294) -> ("States Out"=w2293:string)  [unwired: 13 in]
      }
      frame "---------- UI ----------" {
        # "Do not put any code in this frame.\n(It is a separator no-op. You can make a copy of this frame to create a new UI frame)"
        n1047 = call <vilib>:"Add State(s) to Queue__JKI_lib_State_Machine.vi"("State(s) in (\"\")"=w2299) -> ("States Out"=w2298:string)  [unwired: 14 in]
      }
      frame "UI: Initialize" {
        w2301 = T46 {"Minimum"=0.0, "Maximum"=4.6, "Increment"=0.1} ("Data Entry Limits")
        w2300 = T12."Disabled and Grayed Out" ("Disabled")
        # "Disable all button on startup"
        # "Initialize the User Interface, here.\n(this is called automatically, by the Macro: Init)"
        n1048 = property on="V 1" class="DigNum (strict)"("DisabledEnum"=w2300) -> ()  [unwired: 2 in, 2 out]
        n1049 = property on="V 2" class="DigNum (strict)"("DisabledEnum"=w2300) -> ()  [unwired: 2 in, 2 out]
        n1050 = property on="StopButton" class="Bool (strict)"("DisabledEnum"=w2300) -> ()  [unwired: 2 in, 2 out]
        n1051 = property on="Sys Reconfig" class="Bool"("DisabledEnum"=w2300) -> ()  [unwired: 2 in, 2 out]
        n1052 = property on="StartButton" class="Bool (strict)"("DisabledEnum"=w2300) -> ()  [unwired: 2 in, 2 out]
        n1053 = property on="355nm Laser toggle" class="Bool (strict)"("DisabledEnum"=w2300) -> ()  [unwired: 2 in, 2 out]
        n1054 = property on="Aiming beam toggle" class="Bool (strict)"("DisabledEnum"=w2300) -> ()  [unwired: 2 in, 2 out]
        n1055 = property on="Background" class="Bool (strict)"("DisabledEnum"=w2300) -> ()  [unwired: 2 in, 2 out]
        n1056 = property on="Cali&iRF alignment" class="Bool (strict)"("DisabledEnum"=w2300) -> ()  [unwired: 2 in, 2 out]
        n1057 = property on="V 3" class="DigNum (strict)"("DisabledEnum"=w2300) -> ()  [unwired: 2 in, 2 out]
        n1058 = property on="Video Source" class="RadioBtnsControl (strict)"("DisabledEnum"=w2300) -> ()  [unwired: 2 in, 2 out]
        n1059 = property on="V 1" class="DigNum (strict)"("Data Range"=w2301) -> ()  [unwired: 2 in, 2 out]
        n1060 = property on="V 2" class="DigNum (strict)"("Data Range"=w2301) -> ()  [unwired: 2 in, 2 out]
        n1061 = property on="V 3" class="DigNum (strict)"("Data Range"=w2301) -> ()  [unwired: 2 in, 2 out]
        n1062 = call <vilib>:"Add State(s) to Queue__JKI_lib_State_Machine.vi"("State(s) in Front (\"\")"="UI: CaliAndiRFNotReady" ("State(s) in Front (\"\")"), "State(s) in (\"\")"=w2307) -> ("States Out"=w2306:string)  [unwired: 13 in]
      }
      frame "UI: BGLoaded" {
        # "[Covers: REQ24]"
        # "Do not put any code in this frame.\n(It is a separator no-op. You can make a copy of this frame to create a new UI frame)"
        n1063 = property on="Background" class="Bool (strict)"("BoolText.Text"="Loaded!" ("Boolean Text.Text"), "Colors [4]"=cluster{u32, u32}[] [{15764023, 15764023}, {16711680, 16711680}]) -> ()  [unwired: 2 in, 2 out]
        n1064 = call <vilib>:"Add State(s) to Queue__JKI_lib_State_Machine.vi"("State(s) in (\"\")"=w2314) -> ("States Out"=w2313:string)  [unwired: 14 in]
      }
      frame "UI: BGSizeError" {
        # "[Covers: REQ24]"
        # "Do not put any code in this frame.\n(It is a separator no-op. You can make a copy of this frame to create a new UI frame)"
        n1065 = property on="Background" class="Bool (strict)"("BoolText.Text"="Loaded!" ("Boolean Text.Text"), "Colors [4]"=cluster{u32, u32}[] [{7171459, 7171459}, {16711680, 16711680}]) -> ()  [unwired: 2 in, 2 out]
        n1066 = One Button Dialog(message="Background waveform length and current digitizer setting mismatch! Please take a new background before any aquisition!") -> ()  [unwired: 1 in, 1 out]
        n1067 = call <vilib>:"Add State(s) to Queue__JKI_lib_State_Machine.vi"("State(s) in (\"\")"=w2322) -> ("States Out"=w2321:string)  [unwired: 14 in]
      }
      frame "UI: CaliAndiRFLoaded" {
        # "[Covers: REQ24]"
        # "Do not put any code in this frame.\n(It is a separator no-op. You can make a copy of this frame to create a new UI frame)"
        n1068 = property on="Cali&iRF alignment" class="Bool (strict)"("BoolText.Text"="Loaded!" ("Boolean Text.Text"), "Colors [4]"=cluster{u32, u32}[] [{15764023, 15764023}, {16711680, 16711680}]) -> ()  [unwired: 2 in, 2 out]
        n1069 = call <vilib>:"Add State(s) to Queue__JKI_lib_State_Machine.vi"("State(s) in (\"\")"=w2329) -> ("States Out"=w2328:string)  [unwired: 14 in]
      }
      frame "UI: WFAutoScale" {
        # "Set graph auto scale.\n(UI: WFAutoScale >> T/F)"
        n1070 = Equal?(x=w2330, y="F") -> (x = y?=w2331:bool)
        n1071 = Equal?(x=w2330, y="T") -> (x = y?=w2333:bool)
        n1072 = case shown="True" w2333 {
          frame False {
          }
          frame True {
            w2349 = u8 2 ("Y Scale.Scale Fit")
            n1073 = property on="Channel 1" class="WFGraph (strict)"("YScale.ScaleFit"=w2349) -> ()  [unwired: 2 in, 2 out]
            n1074 = property on="Channel 2" class="WFGraph (strict)"("YScale.ScaleFit"=w2349) -> ()  [unwired: 2 in, 2 out]
            n1075 = property on="Channel 3" class="WFGraph (strict)"("YScale.ScaleFit"=w2349) -> ()  [unwired: 2 in, 2 out]
          }
        }
        n1076 = case shown="True" w2331 {
          frame False {
          }
          frame True {
            w2346 = 0.0 ("Y Scale.Range:Maximum")
            w2347 = 2.0 ("Y Scale.Range:Maximum")
            w2348 = u8 0 ("Y Scale.Scale Fit")
            n1077 = property on="Channel 1" class="WFGraph (strict)"("YScale.ScaleFit"=w2348) -> (error out=w2345:errorcluster)  [unwired: 2 in, 1 out]
            n1078 = property on="Channel 2" class="WFGraph (strict)"("YScale.ScaleFit"=w2348) -> (error out=w2344:errorcluster)  [unwired: 2 in, 1 out]
            n1079 = property on="Channel 3" class="WFGraph (strict)"("YScale.ScaleFit"=w2348) -> (error out=w2343:errorcluster)  [unwired: 2 in, 1 out]
            n1080 = property on="Channel 1" class="WFGraph (strict)"(error in=w2345, "YScale.Maximum"=w2347) -> (error out=w2342:errorcluster)  [unwired: 1 in, 1 out]
            n1081 = property on="Channel 2" class="WFGraph (strict)"(error in=w2344, "YScale.Maximum"=w2347) -> (error out=w2341:errorcluster)  [unwired: 1 in, 1 out]
            n1082 = property on="Channel 3" class="WFGraph (strict)"(error in=w2343, "YScale.Maximum"=w2347) -> (error out=w2340:errorcluster)  [unwired: 1 in, 1 out]
            n1083 = property on="Channel 1" class="WFGraph (strict)"(error in=w2342, "YScale.Minimum"=w2346) -> ()  [unwired: 1 in, 2 out]
            n1084 = property on="Channel 2" class="WFGraph (strict)"(error in=w2341, "YScale.Minimum"=w2346) -> ()  [unwired: 1 in, 2 out]
            n1085 = property on="Channel 3" class="WFGraph (strict)"(error in=w2340, "YScale.Minimum"=w2346) -> ()  [unwired: 1 in, 2 out]
          }
        }
        n1086 = call <vilib>:"Add State(s) to Queue__JKI_lib_State_Machine.vi"("State(s) in (\"\")"=w2339) -> ("States Out"=w2338:string)  [unwired: 14 in]
      }
      frame "UI: showDisclaimer" {
        # "Show disclamer window.\n(It is a separator no-op. You can make a copy of this frame to create a new UI frame)"
        n1087 = call <vilib>:"Application Directory.vi"() -> ("Application Directory"=w2362:path)
        n1088 = Build Path(base path=w2362, name or relative path="Disclamer.png") -> (appended path=w2360:path)
        n1089 = property on="Disclamer" class="Pict"() -> ("Draw Area Size"=w2358:T47)  [unwired: 2 in, 2 out]
        n1090 = disable-structure "Diagram Disable Structure" shown="Disabled" {
          frame Disabled {
            n1091 = flat-sequence {
              frame #0 {
                n1092 = call "disclaimer.vi"() -> ()  [unwired: 12 in]
              }
              frame #1 {
                n1093 = Wait (ms)(milliseconds to wait=u32 250) -> ()  [unwired: 1 out]
              }
              frame #2 {
                n1094 = call "SoftwareNote.vi"() -> ()  [unwired: 12 in]
              }
            }
          }
          frame Enabled {
          }
        }
        n1095 = call <vilib>:"Read PNG File.vi"("path to PNG file"=w2360) -> ("image data"=w2357:T48)  [unwired: 8 in, 2 out]
        n1096 = Unbundle By Name(w2357) -> ("Rectangle.right"=w2355:i16, "Rectangle.bottom"=w2353:i16)
        n1097 = Unbundle By Name(w2358) -> ("Width"=w2356:u32, "Height"=w2354:u32)
        n1098 = call <vilib>:"Draw Flattened Pixmap.vi"("image data"=w2357) -> ("new picture"=→"Disclamer":picture)  [unwired: 8 in]
        n1099 = Divide(x=w2356, y=w2355) -> (x/y=w2352:dbl)
        n1100 = Divide(x=w2354, y=w2353) -> (x/y=w2351:dbl)
        n1101 = Max & Min(x=w2352, y=w2351) -> (min(x,y)=w2350:dbl)  [unwired: 1 out]
        n1102 = property on="Disclamer" class="Pict"("ZoomFactor"=w2350) -> ()  [unwired: 2 in, 2 out]
        n1103 = call <vilib>:"Add State(s) to Queue__JKI_lib_State_Machine.vi"("State(s) in (\"\")"=w2367) -> ("States Out"=w2366:string)  [unwired: 14 in]
      }
      frame "UI: CaliAndiRFNotReady" {
        # "Do not put any code in this frame.\n(It is a separator no-op. You can make a copy of this frame to create a new UI frame)"
        n1104 = property on="Cali&iRF alignment" class="Bool (strict)"("BoolText.Text"="No Info" ("Boolean Text.Text"), "Colors [4]"=cluster{u32, u32}[] [{13816530, 13816530}, {16711680, 16711680}]) -> ()  [unwired: 2 in, 2 out]
        n1105 = call <vilib>:"Add State(s) to Queue__JKI_lib_State_Machine.vi"("State(s) in (\"\")"=w2375) -> ("States Out"=w2374:string)  [unwired: 14 in]
      }
      frame "UI: BGnotReady" {
        # "Do not put any code in this frame.\n(It is a separator no-op. You can make a copy of this frame to create a new UI frame)"
        n1106 = property on="Background" class="Bool (strict)"("BoolText.Text"="No Info" ("Boolean Text.Text"), "Colors [4]"=cluster{u32, u32}[] [{13816530, 13816530}, {16711680, 16711680}]) -> ()  [unwired: 2 in, 2 out]
        n1107 = call <vilib>:"Add State(s) to Queue__JKI_lib_State_Machine.vi"("State(s) in (\"\")"=w2382) -> ("States Out"=w2381:string)  [unwired: 14 in]
      }
      frame "UI: Reset" {
        w2384 = cluster{u32, u32}[] [{13816530, 13816530}, {13816530, 13816530}] ("Colors [4]")
        # "Do not put any code in this frame.\n(It is a separator no-op. You can make a copy of this frame to create a new UI frame)"
        n1108 = property on="Cali&iRF alignment" class="Bool (strict)"("BoolText.Text"="No Info" ("Boolean Text.Text"), "Colors [4]"=w2384) -> ()  [unwired: 2 in, 2 out]
        n1109 = property on="Background" class="Bool (strict)"("BoolText.Text"="No Info" ("Boolean Text.Text"), "Colors [4]"=w2384) -> ()  [unwired: 2 in, 2 out]
        n1110 = call <vilib>:"Add State(s) to Queue__JKI_lib_State_Machine.vi"("State(s) in (\"\")"=w2390) -> ("States Out"=w2389:string)  [unwired: 14 in]
      }
      frame "UI: SetButtonText" {
        # "Set button text of 355nm laser and aiming beam."
        n1111 = call <vilib>:"Add State(s) to Queue__JKI_lib_State_Machine.vi"("State(s) in (\"\")"=w2395) -> ("States Out"=w2394:string)  [unwired: 14 in]
      }
      frame "UI: DuringAquisition" {
        w2398 = T12."Disabled and Grayed Out" ("Disabled")
        # "Do not put any code in this frame.\n(It is a separator no-op. You can make a copy of this frame to create a new UI frame)"
        n1112 = Unbundle By Name(w2397) -> ("bothVidSourceAvail"=w2396:bool)
        n1113 = case shown="True" w2396 {
          tunnel: w2398 -> [_ w2404]
          frame False {
          }
          frame True {
            n1114 = property on="Video Source" class="RadioBtnsControl (strict)"("DisabledEnum"=w2404) -> ()  [unwired: 2 in, 2 out]
          }
        }
        n1115 = property on="StartButton" class="Bool (strict)"("DisabledEnum"=w2398) -> ()  [unwired: 2 in, 2 out]
        n1116 = property on="Sys Reconfig" class="Bool"("DisabledEnum"=w2398) -> ()  [unwired: 2 in, 2 out]
        n1117 = property on="355nm Laser toggle" class="Bool (strict)"("DisabledEnum"=w2398) -> ()  [unwired: 2 in, 2 out]
        n1118 = property on="Aiming beam toggle" class="Bool (strict)"("DisabledEnum"=w2398) -> ()  [unwired: 2 in, 2 out]
        n1119 = property on="Background" class="Bool (strict)"("DisabledEnum"=w2398) -> ()  [unwired: 2 in, 2 out]
        n1120 = property on="Radio Buttons" class="RadioBtnsControl (strict)"("DisabledEnum"=w2398) -> ()  [unwired: 2 in, 2 out]
        n1121 = property on="Cali&iRF alignment" class="Bool (strict)"("DisabledEnum"=w2398) -> ()  [unwired: 2 in, 2 out]
        n1122 = property on="Quit" class="Bool"("DisabledEnum"=w2398) -> ()  [unwired: 2 in, 2 out]
        n1123 = property on="Skip Data Save?" class="Bool (strict)"("DisabledEnum"=w2398) -> ()  [unwired: 2 in, 2 out]
        n1124 = property on="Video Display" class="Bool (strict)"("DisabledEnum"=w2398) -> ()  [unwired: 2 in, 2 out]
        n1125 = property on="StopButton" class="Bool (strict)"("DisabledEnum"=T12."Enabled" ("Disabled")) -> ()  [unwired: 2 in, 2 out]
        n1126 = call <vilib>:"Add State(s) to Queue__JKI_lib_State_Machine.vi"("State(s) in (\"\")"=w2403) -> ("States Out"=w2402:string)  [unwired: 14 in]
      }
      frame "UI: duringIRFAlign" {
        w2405 = T12."Disabled and Grayed Out" ("Disabled")
        # "Set UI to during iRF alignment\n(It is a separator no-op. You can make a copy of this frame to create a new UI frame)"
        n1127 = property on="StartButton" class="Bool (strict)"("DisabledEnum"=w2405) -> ()  [unwired: 2 in, 2 out]
        n1128 = property on="Sys Reconfig" class="Bool"("DisabledEnum"=w2405) -> ()  [unwired: 2 in, 2 out]
        n1129 = property on="355nm Laser toggle" class="Bool (strict)"("DisabledEnum"=w2405) -> ()  [unwired: 2 in, 2 out]
        n1130 = property on="Aiming beam toggle" class="Bool (strict)"("DisabledEnum"=w2405) -> ()  [unwired: 2 in, 2 out]
        n1131 = property on="Background" class="Bool (strict)"("DisabledEnum"=w2405) -> ()  [unwired: 2 in, 2 out]
        n1132 = property on="StopButton" class="Bool (strict)"("DisabledEnum"=w2405) -> ()  [unwired: 2 in, 2 out]
        n1133 = call <vilib>:"Add State(s) to Queue__JKI_lib_State_Machine.vi"("State(s) in (\"\")"=w2410) -> ("States Out"=w2409:string)  [unwired: 14 in]
      }
      frame "UI: duringBGAcquire" {
        w2411 = T12."Disabled and Grayed Out" ("Disabled")
        # "Do not put any code in this frame.\n(It is a separator no-op. You can make a copy of this frame to create a new UI frame)"
        n1134 = property on="StartButton" class="Bool (strict)"("DisabledEnum"=w2411) -> ()  [unwired: 2 in, 2 out]
        n1135 = property on="StopButton" class="Bool (strict)"("DisabledEnum"=w2411) -> ()  [unwired: 2 in, 2 out]
        n1136 = property on="Sys Reconfig" class="Bool"("DisabledEnum"=w2411) -> ()  [unwired: 2 in, 2 out]
        n1137 = property on="355nm Laser toggle" class="Bool (strict)"("DisabledEnum"=w2411) -> ()  [unwired: 2 in, 2 out]
        n1138 = property on="Aiming beam toggle" class="Bool (strict)"("DisabledEnum"=w2411) -> ()  [unwired: 2 in, 2 out]
        n1139 = property on="Cali&iRF alignment" class="Bool (strict)"("DisabledEnum"=w2411) -> ()  [unwired: 2 in, 2 out]
        n1140 = call <vilib>:"Add State(s) to Queue__JKI_lib_State_Machine.vi"("State(s) in (\"\")"=w2416) -> ("States Out"=w2415:string)  [unwired: 14 in]
      }
      frame "UI: ReadyForAquisition" {
        w2420 = T12."Enabled" ("Disabled")
        # "Do not put any code in this frame.\n(It is a separator no-op. You can make a copy of this frame to create a new UI frame)"
        n1141 = Unbundle By Name(w2419) -> ("System Status.TCP/IP"=w2418:bool, "bothVidSourceAvail"=w2417:bool)
        n1142 = property on="StartButton" class="Bool (strict)"("DisabledEnum"=w2420) -> ()  [unwired: 2 in, 2 out]
        n1143 = property on="Sys Reconfig" class="Bool"("DisabledEnum"=w2420) -> ()  [unwired: 2 in, 2 out]
        n1144 = property on="355nm Laser toggle" class="Bool (strict)"("DisabledEnum"=w2420) -> ()  [unwired: 2 in, 2 out]
        n1145 = property on="Aiming beam toggle" class="Bool (strict)"("DisabledEnum"=w2420) -> ()  [unwired: 2 in, 2 out]
        n1146 = property on="Cali&iRF alignment" class="Bool (strict)"("DisabledEnum"=w2420) -> ()  [unwired: 2 in, 2 out]
        n1147 = property on="Background" class="Bool (strict)"("DisabledEnum"=w2420) -> ()  [unwired: 2 in, 2 out]
        n1148 = property on="Quit" class="Bool"("DisabledEnum"=w2420) -> ()  [unwired: 2 in, 2 out]
        n1149 = property on="Radio Buttons" class="RadioBtnsControl (strict)"("DisabledEnum"=w2420) -> ()  [unwired: 2 in, 2 out]
        n1150 = case shown="True" w2417 {
          tunnel: w2420 -> [_ w2426]
          frame False {
          }
          frame True {
            n1151 = property on="Video Source" class="RadioBtnsControl (strict)"("DisabledEnum"=w2426) -> ()  [unwired: 2 in, 2 out]
          }
        }
        n1152 = property on="Skip Data Save?" class="Bool (strict)"("DisabledEnum"=w2420) -> ()  [unwired: 2 in, 2 out]
        n1153 = case shown="True" w2418 {
          tunnel: w2420 -> [_ w2427]
          frame False {
          }
          frame True {
            n1154 = property on="Video Display" class="Bool (strict)"("DisabledEnum"=w2427) -> ()  [unwired: 2 in, 2 out]
          }
        }
        n1155 = property on="StopButton" class="Bool (strict)"("DisabledEnum"=T12."Disabled and Grayed Out" ("Disabled")) -> ()  [unwired: 2 in, 2 out]
        n1156 = call <vilib>:"Add State(s) to Queue__JKI_lib_State_Machine.vi"("State(s) in (\"\")"=w2425) -> ("States Out"=w2424:string)  [unwired: 14 in]
      }
      frame "UI: Update" {
        # "Do not put any code in this frame.\n(It is a separator no-op. You can make a copy of this frame to create a new UI frame)"
        n1157 = Unbundle By Name(w2438) -> ("System Status"=→"System Hardware Connection Status":T2, "IDs.RunID"=→"Run #":i8, "CaseID"=→"Case #":string, "FLImDAQ"=→"FLImDAQ":T31, "SysRunning?"=→"Aquisition Status:":bool, "LJ Pinout"=→"LJ Pinout":T4, "IDs.BG ID"=→"BG #":i8, "IDs.Cali ID"=→"Calibration #":i8, "video source"=→"Visualization PC video source":T1)
        n1158 = call <vilib>:"Add State(s) to Queue__JKI_lib_State_Machine.vi"("State(s) in (\"\")"=w2441) -> ("States Out"=w2440:string)  [unwired: 14 in]
      }
      frame "UI: updateVideoToggle" {
        # "Set video toggle based on visualization PC video source.\n(take )"
        n1159 = call <vilib>:"Add State(s) to Queue__JKI_lib_State_Machine.vi"("State(s) in (\"\")"=w2446) -> ("States Out"=w2445:string)  [unwired: 14 in]
      }
      frame "UI: Cursor Set" {
        # "Argument"
        # "Set and Unset Cursor Busy.\n(Usage: \"UI: Cursor Set >> Busy|Idle\")"
        n1160 = case shown="\"Idle\", Default" w2448 {
          tunnel: w2450 -> [w2455 w2457]
          tunnel: [w2454 w2456] -> w2449
          frame "Idle", Default {
            n1161 = call <vilib>:"Unset Busy.vi"("error in (no error)"=w2455) -> ("error out"=w2454:errorcluster)  [unwired: 10 in]
          }
          frame "Busy" {
            n1162 = call <vilib>:"Set Busy.vi"("error in (no error)"=w2457) -> ("error out"=w2456:errorcluster)  [unwired: 9 in, 1 out]
          }
        }
        n1163 = call <vilib>:"Add State(s) to Queue__JKI_lib_State_Machine.vi"("State(s) in (\"\")"=w2453) -> ("States Out"=w2452:string)  [unwired: 14 in]
      }
      frame "UI: OverlayDialog" {
        # "0: Gain\n1: HN Classifier\n2: Brain Classifier"
        # "Ask user to selection overlay option\n(It is a separator no-op. You can make a copy of this frame to create a new UI frame)"
        n1164 = call <vilib>:"Three Button Dialog.vi"("Allow user to close window? (TRUE)"=FALSE, "Window Title (\"\")"="Overlay selection" ("Window Title (\"\")"), "Right Button Text (\"Cancel\")"="Brain Classifier" ("Right Button Text (\"Cancel\")"), "Center Button Text (\"No\")"="HN Classifier" ("Center Button Text (\"No\")"), "Left Button Text (\"Yes\")"="Gain" ("Left Button Text (\"Yes\")"), "message"="Please comfirm aiming beam colorbar setting and select overlay type! \nUpdate overlay colorbar if needed and restart aiming beam before selection.  ") -> ("Which Button?"=w2460:T49)  [unwired: 5 in]
        n1165 = To Unsigned Word Integer(number=w2460) -> (unsigned 16bit integer=w2459:u16)
        "OverlaySelection" <- w2459
        n1166 = Bundle By Name(cluster=w2462, "OverlaySelection"=w2460) -> (w2461:T24)
        n1167 = case shown="2" w2459 {
          tunnel: [w2472 w2473 w2474] -> w2458
          frame 0, Default {
            w2472 = u16 0 items=["Gain", "Lifetime", "CancerProbability"] ("Overlay selection")
          }
          frame 1 {
            w2473 = u16 2 items=["Gain", "Lifetime", "CancerProbability"] ("Overlay selection")
          }
          frame 2 {
            w2474 = u16 2 items=["Gain", "Lifetime", "CancerProbability"] ("Overlay selection")
          }
        }
        n1168 = local write "Overlay selection"(w2458) -> ()
      }
      frame "UI: Front Panel State" {
        # "Argument"
        # "Set Front Panel Open or Closed\n(Usage: \"UI: Front Panel State >> Open|Close\")"
        n1169 = Unbundle By Name(w2478) -> ("Core.Current VI Reference"=w2477:refnum<vi>)
        n1170 = case shown="\"Open\", \"Standard\", Default" w2476 {
          tunnel: w2480 -> [w2488 w2503 w2514 w2527 w2540]
          tunnel: [w2490 w2504 w2516 w2529 w2542] -> w2479
          tunnel: w2477 -> [w2489 w2501 w2515 w2528 w2541]
          frame "Open", "Standard", Default {
            w2483 = T18."Standard" ("State")
            n1171 = property on="Property Node" class="VI"(reference=w2489, error in=w2488) -> (reference out=w2486:refnum<vi>, error out=w2487:errorcluster, "FP.State"=w2485:T18)
            n1172 = Not Equal?(x=w2485, y=w2483) -> (x != y?=w2484:bool)
            n1173 = case shown="True" w2484 {
              tunnel: [w2494 w2496] -> w2490
              tunnel: w2487 -> [w2493 w2496]
              tunnel: w2486 -> [w2492 _]
              tunnel: w2483 -> [w2491 _]
              frame True {
                n1174 = invoke on="Invoke Node" class="VI" method="FP.Open"(reference=w2492, error in=w2493, "Activate"=TRUE, "State"=w2491) -> (error out=w2494:errorcluster)  [unwired: 1 in, 4 out]
              }
              frame False {
              }
            }
          }
          frame "Close", "Closed" {
            n1175 = property on="Property Node" class="VI"(reference=w2501, error in=w2503) -> (reference out=w2500:refnum<vi>, error out=w2502:errorcluster, "FP.State"=w2498:T18)
            n1176 = Not Equal?(x=w2498, y=T18."Closed" ("Front Panel Window:State")) -> (x != y?=w2497:bool)
            n1177 = case shown="True" w2497 {
              tunnel: [w2505 w2508] -> w2504
              tunnel: w2502 -> [w2505 w2507]
              tunnel: w2500 -> [_ w2506]
              frame False {
              }
              frame True {
                n1178 = invoke on="Invoke Node" class="VI" method="FP.Close"(reference=w2506, error in=w2507) -> (error out=w2508:errorcluster)  [unwired: 1 in, 2 out]
              }
            }
          }
          frame "Hidden", "Hide" {
            w2509 = T18."Hidden" ("State")
            n1179 = property on="Property Node" class="VI"(reference=w2515, error in=w2514) -> (reference out=w2512:refnum<vi>, error out=w2513:errorcluster, "FP.State"=w2511:T18)
            n1180 = Not Equal?(x=w2511, y=w2509) -> (x != y?=w2510:bool)
            n1181 = case shown="True" w2510 {
              tunnel: [w2520 w2521] -> w2516
              tunnel: w2513 -> [w2519 w2521]
              tunnel: w2512 -> [w2518 _]
              tunnel: w2509 -> [w2517 _]
              frame True {
                n1182 = invoke on="Invoke Node" class="VI" method="FP.Open"(reference=w2518, error in=w2519, "State"=w2517) -> (error out=w2520:errorcluster)  [unwired: 2 in, 4 out]
              }
              frame False {
              }
            }
          }
          frame "Minimize", "Minimized" {
            w2522 = T18."Minimized" ("State")
            n1183 = property on="Property Node" class="VI"(reference=w2528, error in=w2527) -> (reference out=w2525:refnum<vi>, error out=w2526:errorcluster, "FP.State"=w2524:T18)
            n1184 = Not Equal?(x=w2524, y=w2522) -> (x != y?=w2523:bool)
            n1185 = case shown="True" w2523 {
              tunnel: [w2533 w2534] -> w2529
              tunnel: w2526 -> [w2532 w2534]
              tunnel: w2525 -> [w2531 _]
              tunnel: w2522 -> [w2530 _]
              frame True {
                n1186 = invoke on="Invoke Node" class="VI" method="FP.Open"(reference=w2531, error in=w2532, "State"=w2530) -> (error out=w2533:errorcluster)  [unwired: 2 in, 4 out]
              }
              frame False {
              }
            }
          }
          frame "Maximize", "Maximized" {
            w2535 = T18."Maximized" ("State")
            n1187 = property on="Property Node" class="VI"(reference=w2541, error in=w2540) -> (reference out=w2538:refnum<vi>, error out=w2539:errorcluster, "FP.State"=w2537:T18)
            n1188 = Not Equal?(x=w2537, y=w2535) -> (x != y?=w2536:bool)
            n1189 = case shown="True" w2536 {
              tunnel: [w2546 w2547] -> w2542
              tunnel: w2539 -> [w2545 w2547]
              tunnel: w2538 -> [w2544 _]
              tunnel: w2535 -> [w2543 _]
              frame True {
                n1190 = invoke on="Invoke Node" class="VI" method="FP.Open"(reference=w2544, error in=w2545, "State"=w2543) -> (error out=w2546:errorcluster)  [unwired: 2 in, 4 out]
              }
              frame False {
              }
            }
          }
        }
        n1191 = call <vilib>:"Add State(s) to Queue__JKI_lib_State_Machine.vi"("State(s) in (\"\")"=w2482) -> ("States Out"=w2481:string)  [unwired: 14 in]
      }
      frame "---------- AimingBeam ----------" {
        # "Template Separator\n(You can make a copy of, or modify, this frame)"
        n1192 = call <vilib>:"Add State(s) to Queue__JKI_lib_State_Machine.vi"("State(s) in (\"\")"=w2552) -> ("States Out"=w2551:string)  [unwired: 14 in]
      }
      frame "AimingBeam: Initialize" {
        # "set aiming beam button color"
        # "Open COM port for Aiming Beam\n(Require USB connection)"
        n1193 = Unbundle By Name(w2554) -> ("AB Cluster.Aiming Beam COM Port"=w2562:refnum<visa-resource-name>)
        n1194 = call-poly "VISA Configure Serial Port"("VISA resource name"=w2562, "Enable Termination\nChar (T)"=TRUE ("Enable Termination\nChar (T)"), "baud rate (9600)"=u32 9600, "error in (no error)"=w2559) -> ("error out"=w2558:errorcluster)  [unwired: 10 in, 1 out]
        n1195 = Unbundle By Name(w2558) -> ("status"=w2557:bool)
        n1196 = Not(x=w2557) -> (.not. x?=w2556:bool)
        n1197 = Bundle By Name(cluster=w2554, "System Status.Aiming Beam"=w2556) -> (w2555:T24)
        n1198 = call <vilib>:"Add State(s) to Queue__JKI_lib_State_Machine.vi"("State(s) in (\"\")"=w2564) -> ("States Out"=w2563:string)  [unwired: 14 in]
      }
      frame "AimingBeam: Close" {
        # "Close Aiming Beam COM port\n(Require USB connection to Aiming Beam Laser)"
        n1199 = Unbundle By Name(w2567) -> ("AB Cluster.Aiming Beam COM Port"=w2571:refnum<visa-resource-name>)
        n1200 = VISA Close(VISA resource name=w2571, error in (no error)=w2569) -> (error out=w2570:errorcluster)
        n1201 = Bundle By Name(cluster=w2567, "System Status.Aiming Beam"=FALSE) -> (w2568:T24)
        n1202 = call <vilib>:"Add State(s) to Queue__JKI_lib_State_Machine.vi"("State(s) in (\"\")"=w2573) -> ("States Out"=w2572:string)  [unwired: 14 in]
      }
      frame "AimingBeam: Set Current" {
        # "Set Aiming Beam Current\n(You can make a copy of, or modify, this frame)"
        n1203 = Unbundle By Name(w2585) -> ("AB Cluster.Aiming Beam COM Port"=w2578:refnum<visa-resource-name>)
        n1204 = Number To Fractional String(number="488nm Power", precision (6)=i16 2) -> (F-format string=w2579:string)  [unwired: 2 in]
        n1205 = Concatenate Strings("slc:", w2579, "\r" ("Carriage Return Constant"), "\n" ("Line Feed Constant")) -> (w2582:string)
        n1206 = VISA Write(VISA resource name=w2578, write buffer=w2582, error in (no error)=w2576) -> (error out=w2577:errorcluster)  [unwired: 2 out]
        n1207 = call <vilib>:"Add State(s) to Queue__JKI_lib_State_Machine.vi"("State(s) in (\"\")"=w2587) -> ("States Out"=w2586:string)  [unwired: 14 in]
      }
      frame "AimingBeam: Set ACC Status" {
        # "Enable Aiming Beam\n(Usage: \"AimingBeam: Set >> Enable|Disable\")"
        n1208 = Unbundle By Name(w2594) -> ("AB Cluster.Aiming Beam COM Port"=w2591:refnum<visa-resource-name>)
        n1209 = case shown="\"Enable\"" w2593 {
          tunnel: [w2597 w2601] -> w2592
          frame "Disable", Default {
            n1210 = Concatenate Strings("cof", "\r" ("Carriage Return Constant"), "\n" ("Line Feed Constant")) -> (w2597:string)
          }
          frame "Enable" {
            n1211 = Concatenate Strings("con", "\r" ("Carriage Return Constant"), "\n" ("Line Feed Constant")) -> (w2601:string)
          }
        }
        n1212 = VISA Write(VISA resource name=w2591, write buffer=w2592, error in (no error)=w2589) -> (error out=w2590:errorcluster)  [unwired: 2 out]
        n1213 = call <vilib>:"Add State(s) to Queue__JKI_lib_State_Machine.vi"("State(s) in (\"\")"=w2596) -> ("States Out"=w2595:string)  [unwired: 14 in]
      }
      frame "AimingBeam: Set APC Status" {
        # "Enable Aiming Beam\n(Usage: \"AimingBeam: Set >> Enable|Disable\")"
        n1214 = Unbundle By Name(w2611) -> ("AB Cluster.Aiming Beam COM Port"=w2608:refnum<visa-resource-name>)
        n1215 = case shown="\"Disable\", Default" w2610 {
          tunnel: [w2614 w2618] -> w2609
          frame "Disable", Default {
            n1216 = Concatenate Strings("lof", "\r" ("Carriage Return Constant"), "\n" ("Line Feed Constant")) -> (w2614:string)
          }
          frame "Enable" {
            n1217 = Concatenate Strings("lon", "\r" ("Carriage Return Constant"), "\n" ("Line Feed Constant")) -> (w2618:string)
          }
        }
        n1218 = VISA Write(VISA resource name=w2608, write buffer=w2609, error in (no error)=w2606) -> (error out=w2607:errorcluster)  [unwired: 2 out]
        n1219 = call <vilib>:"Add State(s) to Queue__JKI_lib_State_Machine.vi"("State(s) in (\"\")"=w2613) -> ("States Out"=w2612:string)  [unwired: 14 in]
      }
      frame "AimingBeam: GetPWMStatus" {
        # "Get aiming beam PWM status\n()"
        n1220 = Unbundle By Name(w2626) -> ("AB Cluster.Freq"=w2625:i32, "LJ Pinout.AimingBeam PWM"=w2632:string)
        n1221 = Equal To 0?(x=w2625) -> (x = 0?=w2624:bool)
        n1222 = call "LabJack_FGV.vi"("Operation(Read)"=enum16{"Write", "Read"}."Read" ("Operation"), "error in (no error)"=w2628) -> ("error out"=w2630:errorcluster, "Read data"=w2631:i32)  [unwired: 8 in]
        n1223 = case shown="True" w2624 {
          tunnel: w2632 -> [w2645 _]
          tunnel: [w2643 "DIO_STATE"] -> w2629
          frame False {
            n1224 = Concatenate Strings(w2645, "_EF_ENABLE" ("string")) -> (w2643:string)
          }
          frame True {
          }
        }
        n1225 = call "LJM_eReadName.vi"("Handle In"=w2631, "Name"=w2629, "error in"=w2630) -> ("Value"=w2623:dbl, "error out"=w2627:errorcluster)  [unwired: 10 in, 1 out]
        n1226 = case shown="True" w2624 {
          tunnel: w2623 -> [w2638 w2642]
          tunnel: [w2637 w2639] -> w2622
          frame False {
            n1227 = Greater Than 0?(x=w2638) -> (x > 0?=w2637:bool)
          }
          frame True {
            n1228 = Number To Boolean Array(number=w2642) -> (Boolean array=w2641:bool[])
            n1229 = Index Array(array=w2641, index=3) -> (element=w2639:bool)
          }
        }
        n1230 = case shown="False" w2622 {
          frame False {
            # "PWM is off\nset color to dark green"
            n1231 = local write "Aiming beam toggle"(FALSE ("Aimging beam")) -> ()
          }
          frame True {
            # "PWM is on\nset color to light green"
            n1232 = local write "Aiming beam toggle"(TRUE ("Aimging beam")) -> ()
          }
        }
        n1233 = call <vilib>:"Add State(s) to Queue__JKI_lib_State_Machine.vi"("State(s) in (\"\")"=w2636) -> ("States Out"=w2635:string)  [unwired: 14 in]
      }
      frame "---------- 355 Laser ----------" {
        # "Template Separator\n(You can make a copy of, or modify, this frame)"
        n1234 = call <vilib>:"Add State(s) to Queue__JKI_lib_State_Machine.vi"("State(s) in (\"\")"=w2653) -> ("States Out"=w2652:string)  [unwired: 14 in]
      }
      frame "355 Laser: Check Dewelling" {
        # "if time laser start time is less than 7.5s before, wait 250ms then check again."
        # "Template Separator\n(You can make a copy of, or modify, this frame)"
        n1235 = Unbundle By Name(w2661) -> ("Laser start tic"=w2658:u32)
        n1236 = Tick Count (ms)() -> (millisecond timer value=w2659:u32)
        n1237 = Subtract(x=w2659, y=w2658) -> (x-y=w2657:u32)
        n1238 = Greater?(x=w2657, y=u32 5000) -> (0:w2655:bool)
        n1239 = case shown="False" w2655 {
          tunnel: ["355 Laser: Check Dewelling" ""] -> w2654
          frame False {
            n1240 = Wait (ms)(milliseconds to wait=u32 250) -> ()  [unwired: 1 out]
          }
          frame True {
          }
        }
        n1241 = call <vilib>:"Add State(s) to Queue__JKI_lib_State_Machine.vi"("State(s) in Front (\"\")"=w2654, "State(s) in (\"\")"=w2664) -> ("States Out"=w2663:string)  [unwired: 13 in]
      }
      frame "355 Laser: Laser enable" {
        # "Laser enable/disable\n(Usage: \"LabJack: Laser enable/disable >> 1|0\")"
        n1242 = Unbundle By Name(w2671) -> ("LJ Pinout.Laser Start/Stop"=w2675:string, "System Status.355 Laser"=w2669:bool)
        n1243 = case shown="False" w2669 {
          tunnel: w2668 -> [w2690 w2691]
          tunnel: w2675 -> [w2684 _]
          tunnel: [w2679 w2691] -> w2673
          tunnel: [w2678 u32 0 ("millisecond timer value")] -> w2670
          frame False {
            n1244 = call "LabJack_FGV.vi"("Operation(Read)"=enum16{"Write", "Read"}."Read" ("Operation")) -> ("Read data"=w2686:i32)  [unwired: 9 in, 1 out]
            n1245 = call "LJM_eWriteName.vi"("Handle In"=w2686, "Name"=w2684, "Value"=1.0, "error in"=w2690) -> ("Handle Out"=w2685:i32, "error out"=w2683:errorcluster)  [unwired: 10 in]
            n1246 = call <userlib>:"Wait (ms)__ogtk.vi"("error in (no error)"=w2683, "milliseconds to wait"=u32 250) -> ("error out"=w2682:errorcluster)  [unwired: 8 in, 1 out]
            n1247 = call "LJM_eWriteName.vi"("Handle In"=w2685, "Name"=w2684, "Value"=0.0, "error in"=w2682) -> ("error out"=w2680:errorcluster)  [unwired: 10 in, 1 out]
            n1248 = call <userlib>:"Tick Count (ms)__ogtk.vi"("error in (no error)"=w2680) -> ("error out"=w2679:errorcluster, "millisecond timer value"=w2678:u32)  [unwired: 9 in]
          }
          frame True {
          }
        }
        n1249 = Bundle By Name(cluster=w2671, "Laser start tic"=w2670) -> (w2672:T24)
        n1250 = call <vilib>:"Add State(s) to Queue__JKI_lib_State_Machine.vi"("State(s) in (\"\")"=w2677) -> ("States Out"=w2676:string)  [unwired: 14 in]
      }
      frame "355 Laser: Laser disable" {
        # "Laser enable/disable\n(Usage: \"LabJack: Laser enable/disable >> 1|0\")"
        n1251 = Unbundle By Name(w2695) -> ("LJ Pinout.Laser Start/Stop"=w2699:string, "System Status.355 Laser"=w2693:bool)
        n1252 = case shown="True" w2693 {
          tunnel: w2700 -> [w2703 w2717]
          tunnel: w2699 -> [_ w2711]
          tunnel: [w2703 w2706] -> w2697
          tunnel: [u32 0 ("millisecond timer value") w2705] -> w2694
          frame False {
          }
          frame True {
            n1253 = call "LabJack_FGV.vi"("Operation(Read)"=enum16{"Write", "Read"}."Read" ("Operation")) -> ("Read data"=w2713:i32)  [unwired: 9 in, 1 out]
            n1254 = call "LJM_eWriteName.vi"("Handle In"=w2713, "Name"=w2711, "Value"=1.0, "error in"=w2717) -> ("Handle Out"=w2712:i32, "error out"=w2710:errorcluster)  [unwired: 10 in]
            n1255 = call <userlib>:"Wait (ms)__ogtk.vi"("error in (no error)"=w2710, "milliseconds to wait"=u32 250) -> ("error out"=w2709:errorcluster)  [unwired: 8 in, 1 out]
            n1256 = call "LJM_eWriteName.vi"("Handle In"=w2712, "Name"=w2711, "Value"=0.0, "error in"=w2709) -> ("error out"=w2707:errorcluster)  [unwired: 10 in, 1 out]
            n1257 = call <userlib>:"Tick Count (ms)__ogtk.vi"("error in (no error)"=w2707) -> ("error out"=w2706:errorcluster, "millisecond timer value"=w2705:u32)  [unwired: 9 in]
          }
        }
        n1258 = Bundle By Name(cluster=w2695, "Laser start tic"=w2694) -> (w2696:T24)
        n1259 = call <vilib>:"Add State(s) to Queue__JKI_lib_State_Machine.vi"("State(s) in (\"\")"=w2702) -> ("States Out"=w2701:string)  [unwired: 14 in]
      }
      frame "355 Laser: Dewelling" {
        # "Wait some time (ms)\n(355 Laser: Dewelling >> #)"
        n1260 = Fract/Exp String To Number(string=w2721, default (0 dbl)=0) -> (number=w2719:i32)  [unwired: 2 in, 1 out]
        n1261 = Wait (ms)(milliseconds to wait=w2719) -> ()  [unwired: 1 out]
        n1262 = call <vilib>:"Add State(s) to Queue__JKI_lib_State_Machine.vi"("State(s) in (\"\")"=w2725) -> ("States Out"=w2724:string)  [unwired: 14 in]
      }
      frame "355 Laser: Close" {
        # "Template Separator\n(You can make a copy of, or modify, this frame)"
        n1263 = call <vilib>:"Add State(s) to Queue__JKI_lib_State_Machine.vi"("State(s) in Front (\"\")"="355 Laser: CheckControllerStatus\n355 Laser: Laser disable\n355 Laser: Dewelling >>1000", "State(s) in (\"\")"=w2731) -> ("States Out"=w2730:string)  [unwired: 13 in]
      }
      frame "355 Laser: CheckControllerStatus" {
        # "if average < 2, laser no power\nif average 2 < average < 9.3, laser on\nif 9.3<average<10, interlock open, blink indicator\nif average > 10, laser off\n[Covers: REQ30]"
        # "take 10 measuremt and look at average"
        # "Check 355 laser controller status\nBy probing Emisison Lamp negative terminal voltage"
        n1264 = Unbundle By Name(w2740) -> ("LJ Pinout.Laser Ready"=w2743:string)
        n1265 = call "LabJack_FGV.vi"("Operation(Read)"=enum16{"Write", "Read"}."Read" ("Operation")) -> ("Read data"=w2744:i32)  [unwired: 9 in, 1 out]
        n1266 = for {
          N: 20 -> [_]
          tunnel: w2744 -> [w2755]
          tunnel: w2743 -> [w2754]
          shift-right: [w2753] -> w2736
          shift-left: w2742 -> [w2752]
          tunnel: [w2750] -> w2735 mode=indexing
          n1267 = call "LJM_eReadName.vi"("Handle In"=w2755, "Name"=w2754, "error in"=w2752) -> ("Value"=w2750:dbl, "error out"=w2753:errorcluster)  [unwired: 10 in, 1 out]
          n1268 = Wait (ms)(milliseconds to wait=u32 25) -> ()  [unwired: 1 out]
        }
        n1269 = call "checkLaserStatus.vi"("error in (no error)"=w2736, "Laser LED voltage"=w2735) -> ("error out"=w2737:errorcluster, "Interlock open?"=w2732:bool, "Laser on?"=w2734:bool, "Mean voltage"=→"laser EM lamp V":dbl)  [unwired: 6 in]
        n1270 = Bundle By Name(cluster=w2740, "System Status.355 Laser"=w2734) -> (w2741:T24)
        n1271 = case shown="True" w2732 {
          frame False {
            n1272 = property on="355 Laser" class="Bool (strict)"("Blinking"=FALSE) -> ()  [unwired: 2 in, 2 out]
          }
          frame True {
            n1273 = property on="355 Laser" class="Bool (strict)"("Blinking"=TRUE) -> ()  [unwired: 2 in, 2 out]
          }
        }
        n1274 = call <vilib>:"Add State(s) to Queue__JKI_lib_State_Machine.vi"("State(s) in (\"\")"=w2747) -> ("States Out"=w2746:string)  [unwired: 14 in]
      }
      frame "355 Laser: CheckPWMStatus" {
        # "Check 355 laser PWM status\n(Read LJ DIO#EF_ENABLE register to determine PWM status)"
        n1275 = Unbundle By Name(w2765) -> ("LJ Pinout.355 PWM"=w2764:string)
        n1276 = call "LabJack_FGV.vi"("Operation(Read)"=enum16{"Write", "Read"}."Read" ("Operation"), "error in (no error)"=w2758) -> ("error out"=w2761:errorcluster, "Read data"=w2762:i32)  [unwired: 8 in]
        n1277 = Concatenate Strings(w2764, "_EF_ENABLE" ("string")) -> (w2760:string)
        n1278 = call "LJM_eReadName.vi"("Handle In"=w2762, "Name"=w2760, "error in"=w2761) -> ("Value"=w2757:dbl, "error out"=w2759:errorcluster)  [unwired: 10 in, 1 out]
        n1279 = Greater Than 0?(x=w2757) -> (x > 0?=w2756:bool)
        n1280 = case shown="False" w2756 {
          frame False {
            # "PWM is off\nset color to gray"
            n1281 = local write "355nm Laser toggle"(FALSE ("355nm Laser")) -> ()
          }
          frame True {
            # "PWM is on\nset color to light green"
            n1282 = local write "355nm Laser toggle"(TRUE ("355nm Laser")) -> ()
          }
        }
        n1283 = call <vilib>:"Add State(s) to Queue__JKI_lib_State_Machine.vi"("State(s) in (\"\")"=w2769) -> ("States Out"=w2768:string)  [unwired: 14 in]
      }
      frame "355 Laser: Start" {
        # "Template Separator\n(You can make a copy of, or modify, this frame)"
        n1284 = call <vilib>:"Add State(s) to Queue__JKI_lib_State_Machine.vi"("State(s) in Front (\"\")"="LabJack: 355_PWM_Start", "State(s) in (\"\")"=w2777) -> ("States Out"=w2776:string)  [unwired: 13 in]
      }
      frame "355 Laser: Stop" {
        # "Template Separator\n(You can make a copy of, or modify, this frame)"
        n1285 = call <vilib>:"Add State(s) to Queue__JKI_lib_State_Machine.vi"("State(s) in Front (\"\")"="LabJack: 355_PWM_Stop", "State(s) in (\"\")"=w2783) -> ("States Out"=w2782:string)  [unwired: 13 in]
      }
      frame "---------- Utility ----------" {
        # "Template Separator\n(You can make a copy of, or modify, this frame)"
        n1286 = call <vilib>:"Add State(s) to Queue__JKI_lib_State_Machine.vi"("State(s) in (\"\")"=w2788) -> ("States Out"=w2787:string)  [unwired: 14 in]
      }
      frame "Utility: SetDataClass" {
        # "Set Data Class in Queues\n(Set data class to either Data, Bg or Cali)"
        n1287 = case shown="\"Cali\"" w2790 {
          tunnel: [enum16{"Data", "BG", "Cali"}."Data" ("Data Class") enum16{"Data", "BG", "Cali"}."BG" ("Data Class") enum16{"Data", "BG", "Cali"}."Cali" ("Data Class")] -> w2789
          frame "Data", Default {
          }
          frame "Bg" {
          }
          frame "Cali" {
          }
        }
        n1288 = local write "Data Class"(w2789) -> ()
        n1289 = call <vilib>:"Add State(s) to Queue__JKI_lib_State_Machine.vi"("State(s) in (\"\")"=w2795) -> ("States Out"=w2794:string)  [unwired: 14 in]
      }
      frame "Utility: AquiTimerReset" {
        # "Set Aquisition Timer\n(You can make a copy of, or modify, this frame)"
        n1290 = Tick Count (ms)() -> (millisecond timer value=w2801:u32)
        n1291 = Bundle By Name(cluster=w2799, "Aquisition Timer"=w2801) -> (w2800:T24)
        n1292 = call <vilib>:"Add State(s) to Queue__JKI_lib_State_Machine.vi"("State(s) in (\"\")"=w2805) -> ("States Out"=w2804:string)  [unwired: 14 in]
      }
      frame "Utility: AquiTimerCheck" {
        # "5min to ms"
        # "Set Aquisition Timer\n([Covers: REQ35])"
        n1293 = Unbundle By Name(w2813) -> ("Aquisition Timer"=w2811:u32)
        n1294 = Tick Count (ms)() -> (millisecond timer value=w2812:u32)
        n1295 = Subtract(x=w2812, y=w2811) -> (x-y=w2810:u32)
        n1296 = Multiply(x=1000, y=300) -> (x*y=w2807:i32)
        n1297 = Greater Or Equal?(x=w2810, y=w2807) -> (x >= y?=w2806:bool)
        n1298 = case shown="True" w2806 {
          frame False {
            # "do nothing"
          }
          frame True {
            # "if timed out, stop aquisition"
            n1299 = property on="StopButton" class="Bool (strict)"("Val(Sgnl)"=TRUE ("Value (Signaling)")) -> ()  [unwired: 2 in, 2 out]
          }
        }
        n1300 = call <vilib>:"Add State(s) to Queue__JKI_lib_State_Machine.vi"("State(s) in (\"\")"=w2817) -> ("States Out"=w2816:string)  [unwired: 14 in]
      }
      frame "Utility: StartBeep" {
        # "Beep\n([Covers: REQ18])"
        n1301 = call <vilib>:"Beep.vi"("use system alert? (T)"=FALSE, "duration (msec)"=u32 1000, "frequency (Hz)"=u32 2000) -> ()  [unwired: 9 in]
        n1302 = call <vilib>:"Add State(s) to Queue__JKI_lib_State_Machine.vi"("State(s) in (\"\")"=w2826) -> ("States Out"=w2825:string)  [unwired: 14 in]
      }
      frame "Utility: EndBeep" {
        # "Beep\n([Covers: REQ18])"
        n1303 = flat-sequence {
          frame #0 {
            n1304 = call <vilib>:"Beep.vi"("use system alert? (T)"=FALSE, "duration (msec)"=u32 500, "frequency (Hz)"=u32 2000) -> ()  [unwired: 9 in]
          }
          frame #1 {
            n1305 = call <vilib>:"Beep.vi"("use system alert? (T)"=FALSE, "duration (msec)"=u32 500, "frequency (Hz)"=u32 2000) -> ()  [unwired: 9 in]
          }
        }
        n1306 = call <vilib>:"Add State(s) to Queue__JKI_lib_State_Machine.vi"("State(s) in (\"\")"=w2831) -> ("States Out"=w2830:string)  [unwired: 14 in]
      }
      frame "Utility: RestoreDeConChan" {
        # "Template Separator\n(You can make a copy of, or modify, this frame)"
        n1307 = global read "GlobalVariables.vi" "DeconChan Temp"() -> (w2838:enum32{"No Selection", "Ch1", "Ch2", "Ch3"})
        n1308 = local write "Radio Buttons"(w2838) -> ()
        n1309 = call <vilib>:"Add State(s) to Queue__JKI_lib_State_Machine.vi"("State(s) in (\"\")"=w2843) -> ("States Out"=w2842:string)  [unwired: 14 in]
      }
      frame "Utility: SaveDeconChan" {
        # "Save Decon Channel to global temp\n(You can make a copy of, or modify, this frame)"
        n1310 = flat-sequence {
          frame #0 {
            n1311 = local read "Radio Buttons"() -> (w2849:T10)
            n1312 = global write "GlobalVariables.vi" "DeconChan Temp"(w2849) -> ()
          }
          frame #1 {
            n1313 = local write "Radio Buttons"(T10."No Selection" ("Radio Buttons")) -> ()
          }
        }
        n1314 = flat-sequence {
          frame #0 {
          }
          frame #1 {
            (unwired) enum32{"No Selection", "Ch1", "Ch2", "Ch3"}."No Selection" ("Radio Buttons")
          }
        }
        n1315 = call <vilib>:"Add State(s) to Queue__JKI_lib_State_Machine.vi"("State(s) in (\"\")"=w2848) -> ("States Out"=w2847:string)  [unwired: 14 in]
      }
      frame "Utility: Dewelling" {
        # "Main loop dewell\n(Dewelling >> #)"
        n1316 = Fract/Exp String To Number(string=w2854, default (0 dbl)=0) -> (number=w2852:i32)  [unwired: 2 in, 1 out]
        n1317 = Wait (ms)(milliseconds to wait=w2852) -> ()  [unwired: 1 out]
        n1318 = call <vilib>:"Add State(s) to Queue__JKI_lib_State_Machine.vi"("State(s) in (\"\")"=w2858) -> ("States Out"=w2857:string)  [unwired: 14 in]
      }
      frame "Utility: SetAllChanManualGain" {
        w2859 = FALSE ("Value (Signaling)")
        # "Set all channel to manual gain\n(You can make a copy of, or modify, this frame)"
        n1319 = property on="Auto gain ch1" class="Bool (strict)"("Val(Sgnl)"=w2859) -> ()  [unwired: 2 in, 2 out]
        n1320 = property on="Auto gain ch2" class="Bool (strict)"("Val(Sgnl)"=w2859) -> ()  [unwired: 2 in, 2 out]
        n1321 = property on="Auto gain ch3" class="Bool (strict)"("Val(Sgnl)"=w2859) -> ()  [unwired: 2 in, 2 out]
        n1322 = property on="Auto gain ch4" class="Bool (strict)"("Val(Sgnl)"=w2859) -> ()  [unwired: 2 in, 2 out]
        n1323 = call <vilib>:"Add State(s) to Queue__JKI_lib_State_Machine.vi"("State(s) in (\"\")"=w2864) -> ("States Out"=w2863:string)  [unwired: 14 in]
      }
      frame "Utility: SetAllChanAutoGain" {
        w2865 = TRUE ("Value (Signaling)")
        # "Set all channels to auto gain\n(You can make a copy of, or modify, this frame)"
        n1324 = property on="Auto gain ch1" class="Bool (strict)"("Val(Sgnl)"=w2865) -> ()  [unwired: 2 in, 2 out]
        n1325 = property on="Auto gain ch2" class="Bool (strict)"("Val(Sgnl)"=w2865) -> ()  [unwired: 2 in, 2 out]
        n1326 = property on="Auto gain ch3" class="Bool (strict)"("Val(Sgnl)"=w2865) -> ()  [unwired: 2 in, 2 out]
        n1327 = property on="Auto gain ch4" class="Bool (strict)"("Val(Sgnl)"=w2865) -> ()  [unwired: 2 in, 2 out]
        n1328 = call <vilib>:"Add State(s) to Queue__JKI_lib_State_Machine.vi"("State(s) in (\"\")"=w2870) -> ("States Out"=w2869:string)  [unwired: 14 in]
      }
      frame "---------- SysLog ----------" {
        # "Template Separator\n(You can make a copy of, or modify, this frame)"
        n1329 = call <vilib>:"Add State(s) to Queue__JKI_lib_State_Machine.vi"("State(s) in (\"\")"=w2875) -> ("States Out"=w2874:string)  [unwired: 14 in]
      }
      frame "SysLog: OpenLogFile" {
        # "Template Separator\n(You can make a copy of, or modify, this frame)"
        n1330 = call <vilib>:"Add State(s) to Queue__JKI_lib_State_Machine.vi"("State(s) in (\"\")"=w2880) -> ("States Out"=w2879:string)  [unwired: 14 in]
      }
      frame "---------- Graph ----------" {
        # "Template Separator\n(You can make a copy of, or modify, this frame)"
        n1331 = call <vilib>:"Add State(s) to Queue__JKI_lib_State_Machine.vi"("State(s) in (\"\")"=w2885) -> ("States Out"=w2884:string)  [unwired: 14 in]
      }
      frame "Graph: SetXMultiplier" {
        # "Set X multiplier of WF graphs\n(You can make a copy of, or modify, this frame)"
        n1332 = call "Digitizer1_FGV.vi"() -> ("error out"=w2889:errorcluster, "Read data"=w2890:refnum<k15>)  [unwired: 10 in]
        n1333 = property class="niScope"(reference=w2890, error in=w2889) -> ("Min Sample Rate"=w2888)  [unwired: 2 out]
        n1334 = Divide(x=1.0, y=w2888) -> (x/y=w2886:dbl)
        n1335 = property on="Channel 1" class="WFGraph (strict)"("XScale.Multiplier"=w2886) -> ()  [unwired: 2 in, 2 out]
        n1336 = property on="Channel 2" class="WFGraph (strict)"("XScale.Multiplier"=w2886) -> ()  [unwired: 2 in, 2 out]
        n1337 = property on="Channel 3" class="WFGraph (strict)"("XScale.Multiplier"=w2886) -> ()  [unwired: 2 in, 2 out]
        n1338 = property on="Channel 4" class="WFGraph (strict)"("XScale.Multiplier"=w2886) -> ()  [unwired: 2 in, 2 out]
        n1339 = call <vilib>:"Add State(s) to Queue__JKI_lib_State_Machine.vi"("State(s) in (\"\")"=w2895) -> ("States Out"=w2894:string)  [unwired: 14 in]
      }
      frame "Graph: AddCursors" {
        # "Add BG and DC cursor to all graphs\n(You can make a copy of, or modify, this frame)"
        n1340 = property on="Channel 1" class="WFGraph (strict)"() -> ("XScale.Multiplier"=w2904:dbl)  [unwired: 2 in, 2 out]
        n1341 = global read "GlobalVariables.vi" "DC Idx1"() -> (w2903:i32)
        n1342 = global read "GlobalVariables.vi" "DC Idx2"() -> (w2902:i32)
        n1343 = global read "GlobalVariables.vi" "BG Idx1"() -> (w2901:i32)
        n1344 = global read "GlobalVariables.vi" "BG Idx2"() -> (w2900:i32)
        n1345 = property on="Channel 1" class="WFGraph (strict)"(error in=w2906) -> ("CrsrList"=w2915:T25)  [unwired: 1 in, 2 out]
        n1346 = property on="Channel 2" class="WFGraph (strict)"() -> ("CrsrList"=w2912:T25)  [unwired: 2 in, 2 out]
        n1347 = property on="Channel 3" class="WFGraph (strict)"() -> ("CrsrList"=w2911:T25)  [unwired: 2 in, 2 out]
        n1348 = property on="Channel 4" class="WFGraph (strict)"() -> ("CrsrList"=w2897:T25)  [unwired: 2 in, 2 out]
        n1349 = Build Array(w2903, w2902, w2901, w2900) -> (w2899:i32[])
        n1350 = Multiply(x=w2899, y=w2904) -> (x*y=w2898:dbl[])
        n1351 = for {
          tunnel: w2915 -> [w2929] mode=indexing
          tunnel: w2898 -> [w2922] mode=indexing
          tunnel: [w2928] -> w2914 mode=indexing
          tunnel: u32[] [6618880, 6618880, 16711680, 16711680] -> [w2921] mode=indexing
          tunnel: w2912 -> [w2927] mode=indexing
          tunnel: w2911 -> [w2926] mode=indexing
          tunnel: [w2925] -> w2910 mode=indexing
          tunnel: [w2924] -> w2909 mode=indexing
          tunnel: w2897 -> [w2923] mode=indexing
          tunnel: [w2920] -> w2896 mode=indexing
          n1352 = Bundle By Name(cluster=w2929, "Position.X"=w2922, "Color"=w2921) -> (w2928:T26)
          n1353 = Bundle By Name(cluster=w2927, "Position.X"=w2922, "Color"=w2921) -> (w2925:T26)
          n1354 = Bundle By Name(cluster=w2926, "Position.X"=w2922, "Color"=w2921) -> (w2924:T26)
          n1355 = Bundle By Name(cluster=w2923, "Position.X"=w2922, "Color"=w2921) -> (w2920:T26)
        }
        n1356 = property on="Channel 1" class="WFGraph (strict)"("CrsrList"=w2914) -> (error out=w2905:errorcluster)  [unwired: 2 in, 1 out]
        n1357 = property on="Channel 2" class="WFGraph (strict)"("CrsrList"=w2910) -> ()  [unwired: 2 in, 2 out]
        n1358 = property on="Channel 3" class="WFGraph (strict)"("CrsrList"=w2909) -> ()  [unwired: 2 in, 2 out]
        n1359 = property on="Channel 4" class="WFGraph (strict)"("CrsrList"=w2896) -> ()  [unwired: 2 in, 2 out]
        n1360 = control-ref of="Channel 1"() -> (w2908:refnum<vi>)
        n1361 = call <vilib>:"Add State(s) to Queue__JKI_lib_State_Machine.vi"("State(s) in (\"\")"=w2919) -> ("States Out"=w2918:string)  [unwired: 14 in]
        n1362 = call "UpdateCurserIdx(SubVI).vi"("error in (no error)"=w2905, "WaveformGraph in"=w2908) -> ("error out"=w2907:errorcluster)  [unwired: 9 in]
      }
      frame "Graph: SaveCursorLoc" {
        # "Save cursor location to ini file\n(Save cursor location to system setting ini file)"
        n1363 = global read "GlobalVariables.vi" "DC Idx1"() -> (w2936:i32)
        n1364 = global read "GlobalVariables.vi" "DC Idx2"() -> (w2935:i32)
        n1365 = global read "GlobalVariables.vi" "BG Idx1"() -> (w2934:i32)
        n1366 = global read "GlobalVariables.vi" "BG Idx2"() -> (w2933:i32)
        n1367 = Bundle("DC Idx1"=w2936, "DC Idx2"=w2935, "BG Idx1"=w2934, "BG Idx2"=w2933) -> (w2932:T50)  [unwired: 1 in]
        n1368 = call "writeCursorConfigMain.vi"("error in (no error)"=w2930, "Cursor Locations"=w2932) -> ("error out"=w2931:errorcluster)  [unwired: 9 in]
        n1369 = call <vilib>:"Add State(s) to Queue__JKI_lib_State_Machine.vi"("State(s) in (\"\")"=w2940) -> ("States Out"=w2939:string)  [unwired: 14 in]
      }
      frame "---------- APD ----------" {
        # "Template Separator\n(You can make a copy of, or modify, this frame)"
        n1370 = call <vilib>:"Add State(s) to Queue__JKI_lib_State_Machine.vi"("State(s) in (\"\")"=w2945) -> ("States Out"=w2944:string)  [unwired: 14 in]
      }
      frame "APD: Initialize" {
        w2952 = enum16{"Read", "Write"}."Write" ("Operation (Read)")
        w2951 = refnum<class "APDClass.lvclass"> refnum  # APDClass.lvclass
        # "Initialize APD FGV\n(Initialized APD FGV for holding data)"
        n1371 = call "APD1FGV.vi"("Error In"=w2946, "Operation (Read)"=w2952, "APDClass in"=w2951) -> ("Error Out"=w2950:errorcluster)  [unwired: 7 in, 1 out]
        n1372 = call "APD2FGV.vi"("Error In"=w2946, "Operation (Read)"=w2952, "APDClass in"=w2951) -> ("Error Out"=w2949:errorcluster)  [unwired: 7 in, 1 out]
        n1373 = call "APD3FGV.vi"("Error In"=w2946, "Operation (Read)"=w2952, "APDClass in"=w2951) -> ("Error Out"=w2948:errorcluster)  [unwired: 7 in, 1 out]
        n1374 = Merge Errors(w2950, w2949, w2948) -> (w2947:errorcluster)
        n1375 = call <vilib>:"Add State(s) to Queue__JKI_lib_State_Machine.vi"("State(s) in (\"\")"=w2956) -> ("States Out"=w2955:string)  [unwired: 14 in]
      }
      frame "APD: LoadFromSerial" {
        w2958 = enum16{"Read", "Write"}."Write" ("Operation (Read)")
        # "Load APD data from tdms file\n(load and update FGV)"
        n1376 = call "readAPDSerial.vi"("Error In"=w2965) -> ("Error Out"=w2961:errorcluster, "output cluster"=w2964:T42)  [unwired: 9 in]
        n1377 = Unbundle By Name(w2964) -> ("Ch1APDSerial#"=w2977:string, "Ch2APDSerial#"=w2963:string, "Ch3APDSerial#"=w2976:string, "Ch4APDSerial#"=w2962:string)
        n1378 = call "CreatFromSerialNumNoRaw.vi"("error in (no error)"=w2961, "APD Serial #"=w2977) -> ("error out"=w2974:errorcluster, "APDClass out"=w2975:refnum<class "APDClass.lvclass">)  [unwired: 8 in]
        n1379 = call "CreatFromSerialNumNoRaw.vi"("error in (no error)"=w2961, "APD Serial #"=w2963) -> ("error out"=w2972:errorcluster, "APDClass out"=w2973:refnum<class "APDClass.lvclass">)  [unwired: 8 in]
        n1380 = call "CreatFromSerialNumNoRaw.vi"("error in (no error)"=w2961, "APD Serial #"=w2976) -> ("error out"=w2970:errorcluster, "APDClass out"=w2971:refnum<class "APDClass.lvclass">)  [unwired: 8 in]
        n1381 = call "CreatFromSerialNumNoRaw.vi"("error in (no error)"=w2961, "APD Serial #"=w2962) -> ("error out"=w2959:errorcluster, "APDClass out"=w2960:refnum<class "APDClass.lvclass">)  [unwired: 8 in]
        n1382 = call "APD1FGV.vi"("Error In"=w2974, "Operation (Read)"=w2958, "APDClass in"=w2975) -> ("Error Out"=w2969:errorcluster)  [unwired: 7 in, 1 out]
        n1383 = call "APD2FGV.vi"("Error In"=w2972, "Operation (Read)"=w2958, "APDClass in"=w2973) -> ("Error Out"=w2967:errorcluster)  [unwired: 7 in, 1 out]
        n1384 = call "APD3FGV.vi"("Error In"=w2970, "Operation (Read)"=w2958, "APDClass in"=w2971) -> ("Error Out"=w2968:errorcluster)  [unwired: 7 in, 1 out]
        n1385 = call "APD4FGV.vi"("Error In"=w2959, "Operation (Read)"=w2958, "APDClass in"=w2960) -> ("Error Out"=w2957:errorcluster)  [unwired: 7 in, 1 out]
        n1386 = Merge Errors(w2969, w2967, w2968, w2957) -> (w2966:errorcluster)
        n1387 = call <vilib>:"Add State(s) to Queue__JKI_lib_State_Machine.vi"("State(s) in (\"\")"=w2981) -> ("States Out"=w2980:string)  [unwired: 14 in]
      }
      frame "APD: UpdateCtrlVLimit" {
        w2987 = enum16{"Read", "Write"}."Read" ("Operation (Read)")
        # "Set V limit\n(You can make a copy of, or modify, this frame)"
        n1388 = call "APD1FGV.vi"("Error In"=w2988, "Operation (Read)"=w2987) -> ("Error Out"=w3003:errorcluster, "APDClass out"=w3004:refnum<class "APDClass.lvclass">)  [unwired: 8 in]
        n1389 = call "APD2FGV.vi"("Error In"=w2988, "Operation (Read)"=w2987) -> ("Error Out"=w3001:errorcluster, "APDClass out"=w3002:refnum<class "APDClass.lvclass">)  [unwired: 8 in]
        n1390 = call "APD3FGV.vi"("Error In"=w2988, "Operation (Read)"=w2987) -> ("Error Out"=w2999:errorcluster, "APDClass out"=w3000:refnum<class "APDClass.lvclass">)  [unwired: 8 in]
        n1391 = call "APD4FGV.vi"("Error In"=w2988, "Operation (Read)"=w2987) -> ("Error Out"=w2985:errorcluster, "APDClass out"=w2986:refnum<class "APDClass.lvclass">)  [unwired: 8 in]
        n1392 = call-dynamic "ReadMaxCtrlV.vi"("error in (no error)"=w3003, "APDClass in"=w3004) -> ("error out"=w2994:errorcluster, "Numeric"=w2997:dbl)  [unwired: 7 in, 1 out]
        n1393 = call-dynamic "ReadMaxCtrlV.vi"("error in (no error)"=w3001, "APDClass in"=w3002) -> ("error out"=w2992:errorcluster, "Numeric"=w2996:dbl)  [unwired: 7 in, 1 out]
        n1394 = call-dynamic "ReadMaxCtrlV.vi"("error in (no error)"=w2999, "APDClass in"=w3000) -> ("error out"=w2990:errorcluster, "Numeric"=w2995:dbl)  [unwired: 7 in, 1 out]
        n1395 = call-dynamic "ReadMaxCtrlV.vi"("error in (no error)"=w2985, "APDClass in"=w2986) -> ("error out"=w2983:errorcluster, "Numeric"=w2984:dbl)  [unwired: 7 in, 1 out]
        n1396 = property on="V 1" class="DigNum (strict)"(error in=w2994, "Maximum"=w2997) -> (error out=w2993:errorcluster)  [unwired: 1 in, 1 out]
        n1397 = property on="V 2" class="DigNum (strict)"(error in=w2992, "Maximum"=w2996) -> (error out=w2991:errorcluster)  [unwired: 1 in, 1 out]
        n1398 = property on="V 4" class="DigNum (strict)"(error in=w2983, "Maximum"=w2984) -> (error out=w2982:errorcluster)  [unwired: 1 in, 1 out]
        n1399 = property on="V 3" class="DigNum (strict)"(error in=w2990, "Maximum"=w2995) -> (error out=w2989:errorcluster)  [unwired: 1 in, 1 out]
        n1400 = Merge Errors(w2993, w2991, w2989, w2982) -> (w2998:errorcluster)
        n1401 = call <vilib>:"Add State(s) to Queue__JKI_lib_State_Machine.vi"("State(s) in (\"\")"=w3008) -> ("States Out"=w3007:string)  [unwired: 14 in]
      }
      frame "APD: GetGainLimits" {
        w3013 = enum16{"Read", "Write"}."Read" ("Operation (Read)")
        # "Template Separator\n(You can make a copy of, or modify, this frame)"
        n1402 = call "APD1FGV.vi"("Error In"=w3014, "Operation (Read)"=w3013) -> ("Error Out"=w3019:errorcluster, "APDClass out"=w3020:refnum<class "APDClass.lvclass">)  [unwired: 8 in]
        n1403 = call "APD2FGV.vi"("Error In"=w3014, "Operation (Read)"=w3013) -> ("Error Out"=w3026:errorcluster, "APDClass out"=w3027:refnum<class "APDClass.lvclass">)  [unwired: 8 in]
        n1404 = call "APD3FGV.vi"("Error In"=w3014, "Operation (Read)"=w3013) -> ("Error Out"=w3024:errorcluster, "APDClass out"=w3025:refnum<class "APDClass.lvclass">)  [unwired: 8 in]
        n1405 = call "APD4FGV.vi"("Error In"=w3014, "Operation (Read)"=w3013) -> ("Error Out"=w3011:errorcluster, "APDClass out"=w3012:refnum<class "APDClass.lvclass">)  [unwired: 8 in]
        n1406 = call-dynamic "Read Gain Limits(Log).vi"("error in (no error)"=w3019, "APDClass in"=w3020) -> ("error out"=w3018:errorcluster, "GainLimits(Log)"=w3015:cluster{"GainMax":dbl, "GainMin":dbl})  [unwired: 7 in, 1 out]
        n1407 = call-dynamic "Read Gain Limits(Log).vi"("error in (no error)"=w3026, "APDClass in"=w3027) -> ("error out"=w3022:errorcluster, "GainLimits(Log)"=w3017:cluster{"GainMax":dbl, "GainMin":dbl})  [unwired: 7 in, 1 out]
        n1408 = call-dynamic "Read Gain Limits(Log).vi"("error in (no error)"=w3024, "APDClass in"=w3025) -> ("error out"=w3021:errorcluster, "GainLimits(Log)"=w3016:cluster{"GainMax":dbl, "GainMin":dbl})  [unwired: 7 in, 1 out]
        n1409 = call-dynamic "Read Gain Limits(Log).vi"("error in (no error)"=w3011, "APDClass in"=w3012) -> ("error out"=w3009:errorcluster, "GainLimits(Log)"=w3010:cluster{"GainMax":dbl, "GainMin":dbl})  [unwired: 7 in, 1 out]
        n1410 = Merge Errors(w3018, w3022, w3021, w3009) -> (w3023:errorcluster)
        n1411 = global write "GlobalVariables.vi" "Ch1GainLim(Log)"(w3015) -> ()
        n1412 = global write "GlobalVariables.vi" "Ch2GainLim(Log)"(w3017) -> ()
        n1413 = global write "GlobalVariables.vi" "Ch3GainLim(Log)"(w3016) -> ()
        n1414 = global write "GlobalVariables.vi" "Ch4GainLim(Log)"(w3010) -> ()
        n1415 = call <vilib>:"Add State(s) to Queue__JKI_lib_State_Machine.vi"("State(s) in (\"\")"=w3031) -> ("States Out"=w3030:string)  [unwired: 14 in]
      }
      frame "---------- TCP ----------" {
        # "Template Separator\n(You can make a copy of, or modify, this frame)"
        n1416 = call <vilib>:"Add State(s) to Queue__JKI_lib_State_Machine.vi"("State(s) in (\"\")"=w3036) -> ("States Out"=w3035:string)  [unwired: 14 in]
      }
      frame "TCP: InitializeNew" {
        # "if unsuccessful and count <10, increament count \nand try again"
        # "Initialize TCP connection to aimging beam computer\n(You can make a copy of, or modify, this frame)"
        n1417 = TCP Create Listener(10:u16 2100 ("port"), 11:"RTLT" ("service name")) -> (0:w3045:errorcluster, 3:w3037:refnum<k5>)  [unwired: 3 in, 1 out]
        n1418 = while {
          tunnel: w3037 -> [w3065]
          tunnel: w3045 -> [w3064]
          tunnel: [w3055] -> w3043
          tunnel: [w3052] -> w3039
          i -> [w3061]
          stop <- w3052 stop-if-true
          n1419 = TCP Wait On Listener(8:w3064, 9:200 ("timeout ms (wait forever: -1)"), 11:w3065) -> (0:w3062:errorcluster, 4:w3059:refnum<k5>)  [unwired: 1 in, 3 out]
          n1420 = Less Or Equal?(x=50, y=w3061) -> (x <= y?=w3058:bool)
          n1421 = case shown="No Error" w3062 {
            selector: w3062 -> [w3075 w3085]
            tunnel: w3059 -> [w3076 _]
            tunnel: [errorcluster {"status"=TRUE, "code"=0, "source"=""} ("No error") w3086] -> w3054
            tunnel: [w3067 FALSE ("TCP connected?")] -> w3055
            frame No Error {
              # "connection is ready, read data"
              n1422 = TCP Read(connection ID=w3076, bytes to read=512, error in (no error)=w3075, 7:T22."CRLF" ("mode (standard)"), 9:5000 ("timeout ms (25000)")) -> (connection ID out=w3069:refnum<k5>, data out=w3071:string, error out=w3068:errorcluster)
              n1423 = Concatenate Strings("alive" ("string"), "\r\n" ("End of Line Constant")) -> (w3072:string)
              n1424 = Equal?(x=w3072, y=w3071) -> (x = y?=w3070:bool)
              n1425 = case shown="False" w3070 {
                tunnel: w3069 -> [_ w3081]
                tunnel: w3068 -> [_ _]
                tunnel: [FALSE ("TCP connected?") TRUE ("TCP connected?")] -> w3067
                frame False {
                }
                frame True {
                  n1426 = call "TcpIDFGV.vi"("action"=enum16{"write", "read"}."write", "connection ID in"=w3081) -> ()  [unwired: 8 in, 2 out]
                }
              }
            }
            frame Error {
              # "connection not ready, keep waiting"
              n1427 = Unbundle By Name(w3085) -> ("code"=w3087:i32)
              n1428 = case shown="56" w3087 {
                tunnel: w3085 -> [w3088 _]
                tunnel: [w3088 w3089] -> w3086
                frame Default {
                }
                frame 56 {
                  w3089 = errorcluster {"status"=FALSE, "code"=0, "source"=""}  # No error
                }
              }
            }
          }
          n1429 = Select(t=errorcluster {"status"=TRUE, "code"=5001, "source"=""} ("error in (no error)"), s=w3058, f=errorcluster {"status"=FALSE, "code"=0, "source"=""} ("error in (no error)")) -> (s? t:f=w3053:errorcluster)
          n1430 = Merge Errors(w3054, w3053) -> (w3052:errorcluster)
        }
        n1431 = Unbundle By Name(w3039) -> ("code"=w3042:i32)
        n1432 = Bundle By Name(cluster=w3044, "System Status.TCP/IP"=w3043, "listener ID"=w3037) -> (w3049:T24)
        n1433 = global write "GlobalVariables.vi" "TCP connected?"(w3043) -> ()
        n1434 = Equal To 0?(x=w3042) -> (x = 0?=w3041:bool)
        n1435 = Select(t=errorcluster {"status"=FALSE, "code"=0, "source"=""} ("error in (no error)"), s=w3041, f=w3039) -> (s? t:f=w3038:errorcluster)
        n1436 = call <vilib>:"Add State(s) to Queue__JKI_lib_State_Machine.vi"("State(s) in (\"\")"=w3051) -> ("States Out"=w3050:string)  [unwired: 14 in]
      }
      frame "TCP: checkSource" {
        # "Check visualization PC video source\n(send !video_source message, listen for response, then parse it to binary mask)"
        n1437 = Unbundle By Name(w3096) -> ("System Status.TCP/IP"=w3099:bool)
        n1438 = case shown="True" w3099 {
          tunnel: w3098 -> [w3104 w3127]
          tunnel: [w3104 w3111] -> w3097
          tunnel: [w3103 w3116] -> w3094
          tunnel: [w3103 w3114] -> w3093
          tunnel: [w3103 w3115] -> w3092
          tunnel: [w3103 w3113] -> w3091
          tunnel: [w3103 w3105] -> w3090
          frame False {
            w3103 = FALSE
          }
          frame True {
            n1439 = call "TcpIDFGV.vi"("Error In"=w3127, "action"=enum16{"write", "read"}."read") -> ("Error Out"=w3124:errorcluster, "connection ID out"=w3126:refnum<k5>)  [unwired: 8 in]
            n1440 = call "TCP_WriteRead.vi"("error in (no error)"=w3124, "data in"="!video_source", "connectin ID in"=w3126) -> ("error out"=w3121:errorcluster, "data out"=w3123:string)  [unwired: 4 in, 1 out]
            n1441 = Scan From String(format string="!video_source:%d", input string=w3123, error in=w3121) -> (error out=w3112:errorcluster, output 1=w3110:i32)  [unwired: 2 in, 2 out]
            n1442 = case shown="5..7, 9..11, 13..15" w3110 {
              tunnel: w3112 -> [_ _ _ _]
              tunnel: [errorcluster {"status"=TRUE, "code"=5007, "source"="Visualization PC"} ("error out") errorcluster {"status"=FALSE, "code"=0, "source"=""} ("error out") errorcluster {"status"=FALSE, "code"=0, "source"=""} ("error out") errorcluster {"status"=FALSE, "code"=0, "source"=""} ("error out")] -> w3111
              tunnel: [FALSE FALSE FALSE TRUE] -> w3105
              frame 0, Default {
                # "No video source available or default"
                n1443 = property on="Video Source" class="RadioBtnsControl (strict)"("DisabledEnum"=T12."Disabled and Grayed Out" ("Disabled")) -> ()  [unwired: 2 in, 2 out]
              }
              frame 1..3 {
                # "one or both camera available"
                n1444 = local write "Video Source"(enum32{"Camera", "FrameGrabber"}."Camera" ("Video Source")) -> ()
                n1445 = property on="Video Source" class="RadioBtnsControl (strict)"("DisabledEnum"=T12."Disabled and Grayed Out" ("Disabled")) -> ()  [unwired: 2 in, 2 out]
              }
              frame 4, 8, 12 {
                # "one or both frame grabber available"
                n1446 = local write "Video Source"(enum32{"Camera", "FrameGrabber"}."FrameGrabber" ("Video Source")) -> ()
                n1447 = property on="Video Source" class="RadioBtnsControl (strict)"("DisabledEnum"=T12."Disabled and Grayed Out" ("Disabled")) -> ()  [unwired: 2 in, 2 out]
              }
              frame 5..7, 9..11, 13..15 {
                n1448 = property on="Video Source" class="RadioBtnsControl (strict)"("DisabledEnum"=T12."Enabled" ("Disabled")) -> ()  [unwired: 2 in, 2 out]
              }
            }
            n1449 = Integer to Fixed-Point Cast(fixed-point type=fxp<+,4,4> 0.0, integer=w3110) -> (fixed-point=w3109:fxp<+,4,4>)
            n1450 = Number To Boolean Array(number=w3109) -> (Boolean array=w3107:bool[])
            n1451 = Reverse 1D Array(array=w3107) -> (reversed array=w3106:bool[])
            n1452 = Index Array(array=w3106, index=0) -> (element=w3116:bool)
            n1453 = Index Array(array=w3106, index=1) -> (element=w3114:bool)
            n1454 = Index Array(array=w3106, index=2) -> (element=w3115:bool)
            n1455 = Index Array(array=w3106, index=3) -> (element=w3113:bool)
          }
        }
        n1456 = Bundle By Name(cluster=w3096, "video source.Main Frame Grabber"=w3094, "video source.Side Frame Grabber"=w3093, "video source.Main Camera"=w3092, "video source.Side Camera"=w3091, "bothVidSourceAvail"=w3090) -> (w3095:T24)
        n1457 = call <vilib>:"Add State(s) to Queue__JKI_lib_State_Machine.vi"("State(s) in (\"\")"=w3102) -> ("States Out"=w3101:string)  [unwired: 14 in]
      }
      frame "TCP: SyncTime" {
        # "Template Separator\n(You can make a copy of, or modify, this frame)"
        n1458 = Unbundle By Name(w3144) -> ("System Status.TCP/IP"=w3143:bool)
        n1459 = case shown="True" w3143 {
          tunnel: w3145 -> [_ w3153]
          frame False {
          }
          frame True {
            n1460 = call "TcpIDFGV.vi"("Error In"=w3153, "action"=enum16{"write", "read"}."read") -> ("Error Out"=w3152:errorcluster, "connection ID out"=w3149:refnum<k5>)  [unwired: 8 in]
            n1461 = call <userlib>:"Tick Count (ms)__ogtk.vi"("error in (no error)"=w3152) -> ("error out"=w3151:errorcluster, "millisecond timer value"=w3150:u32)  [unwired: 9 in]
            n1462 = while {
              tunnel: w3151 -> [w3173]
              tunnel: w3149 -> [w3172]
              tunnel: w3150 -> [w3161]
              stop <- w3156 stop-if-true
              n1463 = Concatenate Strings("latencycheck" ("string"), "\r\n" ("End of Line Constant")) -> (w3168:string)
              n1464 = TCP Read(connection ID=w3172, bytes to read=512, error in (no error)=w3173, 7:T22."CRLF" ("mode (standard)"), 9:2000 ("timeout ms (25000)")) -> (connection ID out=w3165:refnum<k5>, data out=w3163:string, error out=w3155:errorcluster)
              n1465 = Tick Count (ms)() -> (millisecond timer value=w3162:u32)
              n1466 = Subtract(x=w3162, y=w3161) -> (x-y=w3160:u32)
              n1467 = Equal?(x=w3163, y=w3168) -> (x = y?=w3164:bool)
              n1468 = case shown="False" w3164 {
                tunnel: w3165 -> [_ w3186]
                tunnel: w3163 -> [w3178 _]
                tunnel: [w3174 FALSE] -> w3158
                tunnel: w3155 -> [_ w3180]
                frame False {
                  n1469 = Concatenate Strings("synctimer" ("string"), "\r\n" ("End of Line Constant")) -> (w3175:string)
                  n1470 = Equal?(x=w3178, y=w3175) -> (x = y?=w3174:bool)
                  "Sync Success?" <- w3174
                }
                frame True {
                  n1471 = Concatenate Strings("latencycheck:" ("string"), "\r\n" ("End of Line Constant")) -> (w3185:string)
                  n1472 = TCP Write(connection ID=w3186, data in=w3185, error in (no error)=w3180, 9:1000 ("timeout ms (25000)")) -> (error out=w3179:errorcluster)  [unwired: 2 out]
                  n1473 = call <vilib>:"Clear Errors.vi"("error in (no error)"=w3179) -> ()  [unwired: 5 in, 2 out]
                }
              }
              n1474 = Greater?(x=w3160, y=u32 10000 ("x-y")) -> (0:w3157:bool)
              n1475 = Or(x=w3158, y=w3157) -> (x .or. y?=w3156:bool)
            }
          }
        }
        n1476 = call <vilib>:"Add State(s) to Queue__JKI_lib_State_Machine.vi"("State(s) in (\"\")"=w3148) -> ("States Out"=w3147:string)  [unwired: 14 in]
      }
      frame "TCP: SendSettingMacro" {
        # "Template Separator\n(You can make a copy of, or modify, this frame)"
        n1477 = Unbundle By Name(w3190) -> ("System Status.TCP/IP"=w3189:bool)
        n1478 = case shown="True" w3189 {
          tunnel: ["" ("Empty String Constant") "TCP: sendSubjectID\nTCP: sendScaleBarSetting\nTCP: sendScaleMaxMin\nTCP: sendDeconChannel\nTCP: sendANSI\nTCP: sendRadius\nTCP: send3Dsetting\nTCP: sendFirefly\nTCP: sendPentero"] -> w3188
          frame False {
          }
          frame True {
          }
        }
        n1479 = call <vilib>:"Add State(s) to Queue__JKI_lib_State_Machine.vi"("State(s) in Front (\"\")"=w3188, "State(s) in (\"\")"=w3193) -> ("States Out"=w3192:string)  [unwired: 13 in]
      }
      frame "TCP: sendRunNum" {
        # "Send run number to AB PC\n(You can make a copy of, or modify, this frame)"
        n1480 = Unbundle By Name(w3200) -> ("System Status.TCP/IP"=w3197:bool, "IDs.RunID"=w3201:i8)
        n1481 = Increment(x=w3201) -> (x+1=w3196:i8)
        n1482 = case shown="True" w3197 {
          tunnel: w3196 -> [_ w3215]
          tunnel: [w3205 w3207] -> w3199
          tunnel: w3198 -> [w3205 w3206]
          frame False {
          }
          frame True {
            n1483 = Number To Decimal String(number=w3215, width (-)=i16 3) -> (decimal integer string=w3210:string)
            n1484 = call "TcpIDFGV.vi"("Error In"=w3206, "action"=enum16{"write", "read"}."read") -> ("Error Out"=w3208:errorcluster, "connection ID out"=w3212:refnum<k5>)  [unwired: 8 in]
            n1485 = Concatenate Strings("!run:", w3210) -> (w3209:string)
            n1486 = call "TCP_WriteRead.vi"("error in (no error)"=w3208, "data in"=w3209, "connectin ID in"=w3212) -> ("error out"=w3207:errorcluster)  [unwired: 4 in, 2 out]
          }
        }
        n1487 = call <vilib>:"Add State(s) to Queue__JKI_lib_State_Machine.vi"("State(s) in (\"\")"=w3204) -> ("States Out"=w3203:string)  [unwired: 14 in]
      }
      frame "TCP: sendVideoSource" {
        # "Send video source \n(You can make a copy of, or modify, this frame)"
        n1488 = Unbundle By Name(w3217) -> ("System Status.TCP/IP"=w3216:bool)
        n1489 = case shown="True" w3216 {
          tunnel: [w3223 w3225] -> w3219
          tunnel: w3218 -> [w3223 w3224]
          frame False {
          }
          frame True {
            n1490 = case shown="\"Camera\", Default" "Video Source" {
              tunnel: [0 1] -> w3230
              frame "Camera", Default {
              }
              frame "FrameGrabber" {
              }
            }
            n1491 = call "TcpIDFGV.vi"("Error In"=w3224, "action"=enum16{"write", "read"}."read") -> ("Error Out"=w3226:errorcluster, "connection ID out"=w3232:refnum<k5>)  [unwired: 8 in]
            n1492 = Number To Decimal String(number=w3230) -> (decimal integer string=w3228:string)  [unwired: 1 in]
            n1493 = Concatenate Strings("!invivo:" ("data in"), w3228) -> (w3227:string)
            n1494 = call "TCP_WriteRead.vi"("error in (no error)"=w3226, "data in"=w3227, "connectin ID in"=w3232) -> ("error out"=w3225:errorcluster)  [unwired: 4 in, 2 out]
          }
        }
        n1495 = call <vilib>:"Add State(s) to Queue__JKI_lib_State_Machine.vi"("State(s) in (\"\")"=w3222) -> ("States Out"=w3221:string)  [unwired: 14 in]
      }
      frame "TCP: startRun" {
        # "Template Separator\n(You can make a copy of, or modify, this frame)"
        n1496 = Unbundle By Name(w3237) -> ("System Status.TCP/IP"=w3236:bool)
        n1497 = case shown="True" w3236 {
          tunnel: [w3243 w3245] -> w3239
          tunnel: w3238 -> [w3243 w3244]
          frame False {
          }
          frame True {
            n1498 = call "TcpIDFGV.vi"("Error In"=w3244, "action"=enum16{"write", "read"}."read") -> ("Error Out"=w3246:errorcluster, "connection ID out"=w3247:refnum<k5>)  [unwired: 8 in]
            n1499 = call "TCP_WriteRead.vi"("error in (no error)"=w3246, "data in"="!acquire:1", "connectin ID in"=w3247) -> ("error out"=w3245:errorcluster)  [unwired: 4 in, 2 out]
          }
        }
        n1500 = call <vilib>:"Add State(s) to Queue__JKI_lib_State_Machine.vi"("State(s) in (\"\")"=w3242) -> ("States Out"=w3241:string)  [unwired: 14 in]
      }
      frame "TCP: stopRun" {
        # "Send stop run to AB PC\n(You can make a copy of, or modify, this frame)"
        n1501 = Unbundle By Name(w3251) -> ("System Status.TCP/IP"=w3250:bool)
        n1502 = case shown="True" w3250 {
          tunnel: [w3257 w3259] -> w3253
          tunnel: w3252 -> [w3257 w3258]
          frame False {
            # "if not connected, do nothing"
          }
          frame True {
            # "If TCP connected, send stop run"
            n1503 = call "TcpIDFGV.vi"("Error In"=w3258, "action"=enum16{"write", "read"}."read") -> ("Error Out"=w3260:errorcluster, "connection ID out"=w3262:refnum<k5>)  [unwired: 8 in]
            n1504 = call "TCP_WriteRead.vi"("error in (no error)"=w3260, "data in"="!acquire:0", "connectin ID in"=w3262) -> ("error out"=w3259:errorcluster)  [unwired: 4 in, 2 out]
          }
        }
        n1505 = call <vilib>:"Add State(s) to Queue__JKI_lib_State_Machine.vi"("State(s) in (\"\")"=w3256) -> ("States Out"=w3255:string)  [unwired: 14 in]
      }
      frame "TCP: CheckConnection" {
        # "Check TCP/IP connection statuse\n(If connection is lost, throw error)"
        n1506 = Unbundle By Name(w3265) -> ("System Status.TCP/IP"=w3264:bool)
        n1507 = case shown="False" w3264 {
          frame False {
          }
          frame True {
            # "If TCP/IP is true check, otherwise skip"
          }
        }
        n1508 = call <vilib>:"Add State(s) to Queue__JKI_lib_State_Machine.vi"("State(s) in (\"\")"=w3269) -> ("States Out"=w3268:string)  [unwired: 14 in]
      }
      frame "TCP: sendSubjectID" {
        # "Send subject ID"
        n1509 = Unbundle By Name(w3271) -> ("System Status.TCP/IP"=w3270:bool, "CaseID"=w3274:string)
        n1510 = case shown="True" w3270 {
          tunnel: w3274 -> [_ w3285]
          tunnel: [w3278 w3280] -> w3273
          tunnel: w3272 -> [w3278 w3279]
          frame False {
          }
          frame True {
            n1511 = call "TcpIDFGV.vi"("Error In"=w3279, "action"=enum16{"write", "read"}."read") -> ("Error Out"=w3281:errorcluster, "connection ID out"=w3283:refnum<k5>)  [unwired: 8 in]
            n1512 = Concatenate Strings("!subject:", w3285) -> (w3282:string)
            n1513 = call "TCP_WriteRead.vi"("error in (no error)"=w3281, "data in"=w3282, "connectin ID in"=w3283) -> ("error out"=w3280:errorcluster)  [unwired: 4 in, 2 out]
          }
        }
        n1514 = call <vilib>:"Add State(s) to Queue__JKI_lib_State_Machine.vi"("State(s) in (\"\")"=w3277) -> ("States Out"=w3276:string)  [unwired: 14 in]
      }
      frame "TCP: sendScaleBarSetting" {
        # "Template Separator\n(You can make a copy of, or modify, this frame)"
        n1515 = Unbundle By Name(w3289) -> ("System Status.TCP/IP"=w3287:bool, "VideoConfig.Scale Bar"=w3288:bool)
        n1516 = case shown="True" w3287 {
          tunnel: [w3295 w3304] -> w3291
          tunnel: w3290 -> [w3295 w3303]
          tunnel: w3288 -> [_ w3302]
          frame False {
          }
          frame True {
            n1517 = Boolean To (0,1)(Boolean=w3302) -> (0, 1=w3301:i16)
            n1518 = call "TcpIDFGV.vi"("Error In"=w3303, "action"=enum16{"write", "read"}."read") -> ("Error Out"=w3305:errorcluster, "connection ID out"=w3306:refnum<k5>)  [unwired: 8 in]
            n1519 = Number To Fractional String(number=w3301, width (-)=i16 1, precision (6)=i16 0) -> (F-format string=w3299:string)  [unwired: 1 in]
            n1520 = Concatenate Strings("!autocolor:" ("data in"), w3299) -> (w3297:string)
            n1521 = call "TCP_WriteRead.vi"("error in (no error)"=w3305, "data in"=w3297, "connectin ID in"=w3306) -> ("error out"=w3304:errorcluster)  [unwired: 4 in, 2 out]
          }
        }
        n1522 = call <vilib>:"Add State(s) to Queue__JKI_lib_State_Machine.vi"("State(s) in (\"\")"=w3294) -> ("States Out"=w3293:string)  [unwired: 14 in]
      }
      frame "TCP: sendScaleMaxMin" {
        # "Send scale bar max and min to AB PC\n(You can make a copy of, or modify, this frame)"
        n1523 = Unbundle By Name(w3311) -> ("System Status.TCP/IP"=w3308:bool, "VideoConfig.Scale Low"=w3310:dbl, "VideoConfig.Scale High"=w3309:dbl)
        n1524 = case shown="True" w3308 {
          tunnel: [w3317 w3330] -> w3313
          tunnel: w3312 -> [w3317 w3329]
          tunnel: w3310 -> [_ w3328]
          tunnel: w3309 -> [_ w3319]
          frame False {
          }
          frame True {
            n1525 = call "TcpIDFGV.vi"("Error In"=w3329, "action"=enum16{"write", "read"}."read") -> ("Error Out"=w3331:errorcluster, "connection ID out"=w3332:refnum<k5>)  [unwired: 8 in]
            n1526 = Number To Fractional String(number=w3328, width (-)=i16 4, precision (6)=i16 2) -> (F-format string=w3324:string)  [unwired: 1 in]
            n1527 = Number To Fractional String(number=w3319, width (-)=i16 4, precision (6)=i16 2) -> (F-format string=w3320:string)  [unwired: 1 in]
            n1528 = Concatenate Strings("!color:" ("string"), w3324, ";" ("string"), w3320) -> (w3318:string)
            n1529 = call "TCP_WriteRead.vi"("error in (no error)"=w3331, "data in"=w3318, "connectin ID in"=w3332) -> ("error out"=w3330:errorcluster)  [unwired: 4 in, 2 out]
          }
        }
        n1530 = call <vilib>:"Add State(s) to Queue__JKI_lib_State_Machine.vi"("State(s) in (\"\")"=w3316) -> ("States Out"=w3315:string)  [unwired: 14 in]
      }
      frame "TCP: sendDeconChannel" {
        # "Send Decon channel\n(You can make a copy of, or modify, this frame)"
        n1531 = Unbundle By Name(w3335) -> ("System Status.TCP/IP"=w3334:bool)
        n1532 = case shown="True" w3334 {
          tunnel: [w3341 w3346] -> w3337
          tunnel: w3336 -> [w3341 w3345]
          frame False {
          }
          frame True {
            n1533 = local read "Radio Buttons"() -> (w3344:T10)
            n1534 = Increment(x=w3344) -> (x+1=w3343:T10)
            n1535 = Number To Decimal String(number=w3343) -> (decimal integer string=w3342:string)  [unwired: 1 in]
            n1536 = call "TcpIDFGV.vi"("Error In"=w3345, "action"=enum16{"write", "read"}."read") -> ("Error Out"=w3347:errorcluster, "connection ID out"=w3350:refnum<k5>)  [unwired: 8 in]
            n1537 = Concatenate Strings("!channel:", w3342) -> (w3348:string)
            n1538 = call "TCP_WriteRead.vi"("error in (no error)"=w3347, "data in"=w3348, "connectin ID in"=w3350) -> ("error out"=w3346:errorcluster)  [unwired: 4 in, 2 out]
          }
        }
        n1539 = call <vilib>:"Add State(s) to Queue__JKI_lib_State_Machine.vi"("State(s) in (\"\")"=w3340) -> ("States Out"=w3339:string)  [unwired: 14 in]
      }
      frame "TCP: sendANSI" {
        # "Template Separator\n(You can make a copy of, or modify, this frame)"
        n1540 = Unbundle By Name(w3354) -> ("System Status.TCP/IP"=w3352:bool, "VideoConfig.ANSI"=w3353:dbl)
        n1541 = case shown="True" w3352 {
          tunnel: [w3360 w3366] -> w3356
          tunnel: w3355 -> [w3360 w3365]
          tunnel: w3353 -> [_ w3364]
          frame False {
          }
          frame True {
            n1542 = Number To Fractional String(number=w3364) -> (F-format string=w3362:string)  [unwired: 3 in]
            n1543 = call "TcpIDFGV.vi"("Error In"=w3365, "action"=enum16{"write", "read"}."read") -> ("Error Out"=w3367:errorcluster, "connection ID out"=w3368:refnum<k5>)  [unwired: 8 in]
            n1544 = Concatenate Strings("!ansi:" ("data in"), w3362) -> (w3361:string)
            n1545 = call "TCP_WriteRead.vi"("error in (no error)"=w3367, "data in"=w3361, "connectin ID in"=w3368) -> ("error out"=w3366:errorcluster)  [unwired: 4 in, 2 out]
          }
        }
        n1546 = call <vilib>:"Add State(s) to Queue__JKI_lib_State_Machine.vi"("State(s) in (\"\")"=w3359) -> ("States Out"=w3358:string)  [unwired: 14 in]
      }
      frame "TCP: sendRadius" {
        # "Send drawing radius to AB PC\n(You can make a copy of, or modify, this frame)"
        n1547 = Unbundle By Name(w3372) -> ("System Status.TCP/IP"=w3370:bool, "VideoConfig.Radius"=w3371:dbl)
        n1548 = case shown="True" w3370 {
          tunnel: [w3378 w3384] -> w3374
          tunnel: w3373 -> [w3378 w3383]
          tunnel: w3371 -> [_ w3382]
          frame False {
          }
          frame True {
            n1549 = Number To Fractional String(number=w3382) -> (F-format string=w3381:string)  [unwired: 3 in]
            n1550 = Concatenate Strings("!radius:" ("data in"), w3381) -> (w3379:string)
            n1551 = call "TcpIDFGV.vi"("Error In"=w3383, "action"=enum16{"write", "read"}."read") -> ("Error Out"=w3385:errorcluster, "connection ID out"=w3386:refnum<k5>)  [unwired: 8 in]
            n1552 = call "TCP_WriteRead.vi"("error in (no error)"=w3385, "data in"=w3379, "connectin ID in"=w3386) -> ("error out"=w3384:errorcluster)  [unwired: 4 in, 2 out]
          }
        }
        n1553 = call <vilib>:"Add State(s) to Queue__JKI_lib_State_Machine.vi"("State(s) in (\"\")"=w3377) -> ("States Out"=w3376:string)  [unwired: 14 in]
      }
      frame "TCP: send3Dsetting" {
        # "Send 3D setting to AB computer\n(You can make a copy of, or modify, this frame)"
        n1554 = Unbundle By Name(w3390) -> ("System Status.TCP/IP"=w3388:bool, "VideoConfig.3D?"=w3389:bool)
        n1555 = case shown="True" w3388 {
          tunnel: [w3396 w3403] -> w3392
          tunnel: w3391 -> [w3396 w3402]
          tunnel: w3389 -> [_ w3401]
          frame False {
          }
          frame True {
            n1556 = Boolean To (0,1)(Boolean=w3401) -> (0, 1=w3400:i16)
            n1557 = Number To Fractional String(number=w3400) -> (F-format string=w3399:string)  [unwired: 3 in]
            n1558 = call "TcpIDFGV.vi"("Error In"=w3402, "action"=enum16{"write", "read"}."read") -> ("Error Out"=w3404:errorcluster, "connection ID out"=w3405:refnum<k5>)  [unwired: 8 in]
            n1559 = Concatenate Strings("!3dset:" ("data in"), w3399) -> (w3397:string)
            n1560 = call "TCP_WriteRead.vi"("error in (no error)"=w3404, "data in"=w3397, "connectin ID in"=w3405) -> ("error out"=w3403:errorcluster)  [unwired: 4 in, 2 out]
          }
        }
        n1561 = call <vilib>:"Add State(s) to Queue__JKI_lib_State_Machine.vi"("State(s) in (\"\")"=w3395) -> ("States Out"=w3394:string)  [unwired: 14 in]
      }
      frame "TCP: sendFirefly" {
        # "Template Separator\n(You can make a copy of, or modify, this frame)"
        n1562 = Unbundle By Name(w3408) -> ("System Status.TCP/IP"=w3407:bool)
        n1563 = case shown="False" w3407 {
          tunnel: [w3414 w3416] -> w3410
          tunnel: w3409 -> [w3414 w3415]
          frame False {
          }
          frame True {
            n1564 = call "TcpIDFGV.vi"("Error In"=w3415, "action"=enum16{"write", "read"}."read") -> ("Error Out"=w3417:errorcluster, "connection ID out"=w3419:refnum<k5>)  [unwired: 8 in]
            n1565 = call "TCP_WriteRead.vi"("error in (no error)"=w3417, "data in"="!firefly:0", "connectin ID in"=w3419) -> ("error out"=w3416:errorcluster)  [unwired: 4 in, 2 out]
          }
        }
        n1566 = call <vilib>:"Add State(s) to Queue__JKI_lib_State_Machine.vi"("State(s) in (\"\")"=w3413) -> ("States Out"=w3412:string)  [unwired: 14 in]
      }
      frame "TCP: sendPentero" {
        # "Send Pentero setting to AB computer\n(You can make a copy of, or modify, this frame)"
        n1567 = Unbundle By Name(w3422) -> ("System Status.TCP/IP"=w3421:bool)
        n1568 = case shown="True" w3421 {
          tunnel: [w3428 w3430] -> w3424
          tunnel: w3423 -> [w3428 w3429]
          frame False {
          }
          frame True {
            n1569 = call "TcpIDFGV.vi"("Error In"=w3429, "action"=enum16{"write", "read"}."read") -> ("Error Out"=w3431:errorcluster, "connection ID out"=w3433:refnum<k5>)  [unwired: 8 in]
            n1570 = call "TCP_WriteRead.vi"("error in (no error)"=w3431, "data in"="!pentero:0", "connectin ID in"=w3433) -> ("error out"=w3430:errorcluster)  [unwired: 4 in, 2 out]
          }
        }
        n1571 = call <vilib>:"Add State(s) to Queue__JKI_lib_State_Machine.vi"("State(s) in (\"\")"=w3427) -> ("States Out"=w3426:string)  [unwired: 14 in]
      }
      frame "TCP: sendChannel" {
        # "Send DeCon Channel to AB computer\n()"
        n1572 = Unbundle By Name(w3436) -> ("System Status.TCP/IP"=w3435:bool)
        n1573 = case shown="True" w3435 {
          tunnel: [w3442 w3446] -> w3438
          tunnel: w3437 -> [w3442 w3445]
          frame False {
          }
          frame True {
            n1574 = local read "Radio Buttons"() -> (w3444:T10)
            n1575 = case shown="\"No Selection\", Default" w3444 {
              tunnel: ["" ("data in") "!channel:1" ("data in") "!channel:2" ("data in") "!channel:3" ("data in")] -> w3443
              frame "No Selection", Default {
              }
              frame "Ch1" {
              }
              frame "Ch2" {
              }
              frame "Ch3" {
              }
            }
            n1576 = call "TcpIDFGV.vi"("Error In"=w3445, "action"=enum16{"write", "read"}."read") -> ("Error Out"=w3447:errorcluster, "connection ID out"=w3448:refnum<k5>)  [unwired: 8 in]
            n1577 = call "TCP_WriteRead.vi"("error in (no error)"=w3447, "data in"=w3443, "connectin ID in"=w3448) -> ("error out"=w3446:errorcluster)  [unwired: 4 in, 2 out]
          }
        }
        n1578 = call <vilib>:"Add State(s) to Queue__JKI_lib_State_Machine.vi"("State(s) in (\"\")"=w3441) -> ("States Out"=w3440:string)  [unwired: 14 in]
      }
      frame "TCP: startCam" {
        # "Send Pentero setting to AB computer\n(You can make a copy of, or modify, this frame)"
        n1579 = Unbundle By Name(w3455) -> ("System Status.TCP/IP"=w3454:bool)
        n1580 = case shown="True" w3454 {
          tunnel: [w3461 w3463] -> w3457
          tunnel: w3456 -> [w3461 w3462]
          frame False {
          }
          frame True {
            n1581 = call "TcpIDFGV.vi"("Error In"=w3462, "action"=enum16{"write", "read"}."read") -> ("Error Out"=w3464:errorcluster, "connection ID out"=w3466:refnum<k5>)  [unwired: 8 in]
            n1582 = call "TCP_WriteRead.vi"("error in (no error)"=w3464, "data in"="!focus:1", "connectin ID in"=w3466) -> ("error out"=w3463:errorcluster)  [unwired: 4 in, 2 out]
          }
        }
        n1583 = call <vilib>:"Add State(s) to Queue__JKI_lib_State_Machine.vi"("State(s) in (\"\")"=w3460) -> ("States Out"=w3459:string)  [unwired: 14 in]
      }
      frame "TCP: stopCam" {
        # "Send Pentero setting to AB computer\n(You can make a copy of, or modify, this frame)"
        n1584 = Unbundle By Name(w3469) -> ("System Status.TCP/IP"=w3468:bool)
        n1585 = case shown="True" w3468 {
          tunnel: [w3475 w3477] -> w3471
          tunnel: w3470 -> [w3475 w3476]
          frame False {
          }
          frame True {
            n1586 = call "TcpIDFGV.vi"("Error In"=w3476, "action"=enum16{"write", "read"}."read") -> ("Error Out"=w3478:errorcluster, "connection ID out"=w3480:refnum<k5>)  [unwired: 8 in]
            n1587 = call "TCP_WriteRead.vi"("error in (no error)"=w3478, "data in"="!focus:0", "connectin ID in"=w3480) -> ("error out"=w3477:errorcluster)  [unwired: 4 in, 2 out]
          }
        }
        n1588 = call <vilib>:"Add State(s) to Queue__JKI_lib_State_Machine.vi"("State(s) in (\"\")"=w3474) -> ("States Out"=w3473:string)  [unwired: 14 in]
      }
      frame "TCP: Close" {
        # "Close TCP connection\n()"
        n1589 = Unbundle By Name(w3484) -> ("System Status.TCP/IP"=w3482:bool)
        n1590 = case shown="True" w3482 {
          tunnel: [w3490 w3492] -> w3485
          tunnel: w3483 -> [w3490 w3491]
          frame False {
          }
          frame True {
            n1591 = call "TcpIDFGV.vi"("Error In"=w3491, "action"=enum16{"write", "read"}."read") -> ("Error Out"=w3494:errorcluster, "connection ID out"=w3495:refnum<k5>)  [unwired: 8 in]
            n1592 = TCP Close Connection(connection ID=w3495, error in (no error)=w3494) -> (error out=w3492:errorcluster)  [unwired: 1 in, 1 out]
          }
        }
        n1593 = case shown="Error .." w3485 {
          tunnel: [w3498 w3499] -> w3486
          tunnel: w3484 -> [w3497 w3499]
          frame No Error {
            w3496 = FALSE ("System Status.TCP/IP")
            n1594 = Bundle By Name(cluster=w3497, "System Status.TCP/IP"=w3496) -> (w3498:T24)
            n1595 = global write "GlobalVariables.vi" "TCP connected?"(w3496) -> ()
          }
          frame Error {
          }
        }
        n1596 = call <vilib>:"Add State(s) to Queue__JKI_lib_State_Machine.vi"("State(s) in (\"\")"=w3489) -> ("States Out"=w3488:string)  [unwired: 14 in]
      }
      frame "---------- PID ----------" {
        # "Template Separator\n(You can make a copy of, or modify, this frame)"
        n1597 = call <vilib>:"Add State(s) to Queue__JKI_lib_State_Machine.vi"("State(s) in (\"\")"=w3504) -> ("States Out"=w3503:string)  [unwired: 14 in]
      }
      frame "PID: loadPID" {
        # "Template Separator\n(You can make a copy of, or modify, this frame)"
        n1598 = call "readPIDSetting.vi"("Error In"=w3508) -> ("Error Out"=w3509:errorcluster, "Ch3 PID out"=w3505:T8, "Ch2 PID out"=w3506:T8, "Ch1 PID out"=w3507:T8)  [unwired: 7 in]
        n1599 = local write "Ch1 PID gains"(w3507) -> ()
        n1600 = local write "Ch2 PID gains"(w3506) -> ()
        n1601 = local write "Ch3 PID gains"(w3505) -> ()
        n1602 = local write "Ch4 PID gains"(w3505) -> ()
        n1603 = call <vilib>:"Add State(s) to Queue__JKI_lib_State_Machine.vi"("State(s) in (\"\")"=w3513) -> ("States Out"=w3512:string)  [unwired: 14 in]
      }
      frame "---------- Classifier ----------" {
        # "Template Separator\n(You can make a copy of, or modify, this frame)"
        n1604 = call <vilib>:"Add State(s) to Queue__JKI_lib_State_Machine.vi"("State(s) in (\"\")"=w3518) -> ("States Out"=w3517:string)  [unwired: 14 in]
      }
      frame "Classifier: Init" {
        # "Initilize Python\n(You can make a copy of, or modify, this frame)"
        n1605 = Unbundle By Name(w3520) -> ("OverlaySelection"=w3519:u16)
        n1606 = case shown="2" w3519 {
          tunnel: ["HN model path" "Brain model path"] -> w3523
          frame 0, 1, Default {
          }
          frame 2 {
          }
        }
        n1607 = call-poly <vilib>:"Open Virtual Environment Session.vi"("error in (no error)"=w3529, "Anaconda path"=path "C:/ProgramData/miniconda3", "Python version"="Python version", "Env name"="Env name") -> ("error out"=w3525:errorcluster, "session out"=w3528:refnum<k35>)  [unwired: 6 in]
        n1608 = Path To String(path=w3523) -> (string=w3522:string)
        n1609 = node "Python Node"(w3528, "module path", "load_model" ("function name"), w3525, w3522) -> (→"Python session":refnum<k35>, w3524:errorcluster)  [unwired: 3 in, 2 out]
        n1610 = call <vilib>:"Add State(s) to Queue__JKI_lib_State_Machine.vi"("State(s) in (\"\")"=w3535) -> ("States Out"=w3534:string)  [unwired: 14 in]
      }
      frame "Classifier: Close" {
        # "Template Separator\n(You can make a copy of, or modify, this frame)"
        n1611 = local read "Python session"() -> (w3541:refnum<k35>)
        n1612 = Close Python Session(session in=w3541, error in=w3540) -> (11:w3539:errorcluster)
        n1613 = case shown="Error .." w3539 {
          selector: w3539 -> [w3546 _]
          tunnel: [w3546 errorcluster {"status"=FALSE, "code"=0, "source"=""} ("error IO")] -> w3538
          frame No Error {
          }
          frame Error {
          }
        }
        n1614 = call <vilib>:"Add State(s) to Queue__JKI_lib_State_Machine.vi"("State(s) in (\"\")"=w3545) -> ("States Out"=w3544:string)  [unwired: 14 in]
      }
      frame "---------- Debug ----------" {
        # "Template Separator\n(You can make a copy of, or modify, this frame)"
        n1615 = call <vilib>:"Add State(s) to Queue__JKI_lib_State_Machine.vi"("State(s) in (\"\")"=w3552) -> ("States Out"=w3551:string)  [unwired: 14 in]
      }
      frame "Debug: OpenDebugTDMS" {
        # "Create Debug TDMS file\n(You can make a copy of, or modify, this frame)"
        n1616 = Unbundle By Name(w3568) -> ("Pathes.DataPath"=w3563:path, "CaseID"=w3562:string, "IDs.RunID"=w3567:i8)
        n1617 = Increment(x=w3567) -> (x+1=w3561:i8)
        n1618 = Format Value(string ("")=w3562, format string="_%02d", value (0)=w3561) -> (output string=w3560:string)
        n1619 = Concatenate Strings(w3560, "Debug" ("string")) -> (w3558:string)
        n1620 = Build Path(base path=w3563, name or relative path=w3558) -> (appended path=w3566:path)
        n1621 = TDMS Open(8:w3557, 10:T16."create or replace" ("operation (0:open)"), 11:w3566) -> (0:w3556:errorcluster, 3:w3555:refnum<k34>)  [unwired: 4 in]
        n1622 = call "DebugTDMS_FGV.vi"("error in (no error)"=w3556, "Operation (Read)"=enum16{"Write", "Read"}."Write", "tdms file in"=w3555) -> ("error out"=w3553:errorcluster)  [unwired: 7 in, 1 out]
        n1623 = call <vilib>:"Add State(s) to Queue__JKI_lib_State_Machine.vi"("State(s) in (\"\")"=w3571) -> ("States Out"=w3570:string)  [unwired: 14 in]
      }
      frame "Debug: CloseDebugTDMS" {
        # "Template Separator\n(You can make a copy of, or modify, this frame)"
        n1624 = call "DebugTDMS_FGV.vi"("error in (no error)"=w3572) -> ("error out"=w3574:errorcluster, "tdms file out"=w3575:refnum<k34>)  [unwired: 9 in]
        n1625 = TDMS Close(8:w3574, 11:w3575) -> (0:w3573:errorcluster)  [unwired: 1 out]
        n1626 = call <vilib>:"Add State(s) to Queue__JKI_lib_State_Machine.vi"("State(s) in (\"\")"=w3579) -> ("States Out"=w3578:string)  [unwired: 14 in]
      }
      frame "---------- Temp (copy) ----------" {
        # "Template Separator\n(You can make a copy of, or modify, this frame)"
        n1627 = call <vilib>:"Add State(s) to Queue__JKI_lib_State_Machine.vi"("State(s) in (\"\")"=w3584) -> ("States Out"=w3583:string)  [unwired: 14 in]
      }
    }
    n1628 = Not(x=w80) -> (.not. x?=w79:bool)
    n1629 = local write "ML?"(w79) -> ()
    "ML?" <- TRUE ("main loop running?")
  }
  n1630 = while {
    tunnel: w19 -> [w3618]
    tunnel: w18 -> [w3588]
    tunnel: [w3587] -> w17
    tunnel: w13 -> [w3614]
    tunnel: [w3613] -> w16
    shift-right: [w3609] -> _
    shift-left: _ -> [w3610]
    stop <- w3589 stop-if-true
    # "Read data from notifier and deconvolve it and send to Aiming Beam computer"
    n1631 = Wait on Notification(notifier=w3618, ignore previous (F)=FALSE) -> (notification=w3605:T15, error out=w3589:errorcluster)  [unwired: 2 in, 2 out]
    n1632 = local read "Data Class"() -> (w3590:enum16{"Data", "BG", "Cali"})
    n1633 = Unbundle(w3605) -> ("idx"=w3585:i32, "CH1&2"=w3617:dbl[][], "CH3&4"=w3616:dbl[][], "V cluster"=w3595:cluster{"V1":dbl, "V2":dbl, "V3":dbl, "V4":dbl})
    n1634 = call "SeperateChanData.vi"("Input (Ch1&2)"=w3616) -> ("Ch1"=w3592:dbl[][], "Ch2"=w3600:dbl[][])
    n1635 = call "SeperateChanData.vi"("Input (Ch1&2)"=w3617) -> ("Ch1"=w3594:dbl[][], "Ch2"=w3593:dbl[][])
    n1636 = case shown="\"Data\"" w3590 {
      tunnel: w3595 -> [w3630 _]
      tunnel: w3594 -> [w3629 _]
      tunnel: w3593 -> [w3628 _]
      tunnel: w3592 -> [w3627 _]
      tunnel: w3589 -> [w3626 w3755]
      tunnel: w3585 -> [w3619 _]
      tunnel: w3588 -> [w3624 w3756]
      tunnel: [w3621 w3756] -> w3587
      tunnel: [w3620 w3755] -> w3586
      frame "Data" {
        # "If acquiring data"
        n1637 = case shown="1, 2" "Overlay selection" {
          tunnel: "Radio Buttons" -> [w3634 _]
          tunnel: [w3635 w3659] -> w3622
          tunnel: w3626 -> [w3635 w3658]
          tunnel: [w3633 w3646] -> w3625
          tunnel: w3630 -> [_ w3665]
          tunnel: w3629 -> [_ w3662]
          tunnel: w3628 -> [_ w3661]
          tunnel: w3627 -> [_ w3660]
          tunnel: w3619 -> [_ w3641]
          frame 0, Default {
            # "overlay gain"
            n1638 = case shown="\"Ch1\"" w3634 {
              tunnel: [0.0 ("Gain1") w3637 w3638 w3639 w3640] -> w3633
              frame "No Selection", Default {
              }
              frame "Ch1" {
                n1639 = local read "Gain1"() -> (w3637:dbl)
              }
              frame "Ch2" {
                n1640 = local read "Gain2"() -> (w3638:dbl)
              }
              frame "Ch3" {
                n1641 = local read "Gain3"() -> (w3639:dbl)
              }
              frame "Ch4" {
                n1642 = local read "Gain4"() -> (w3640:dbl)
              }
            }
          }
          frame 1, 2 {
            # "overlay lifetime or cancer probability"
            n1643 = call "DeConAPD2FGV.vi"("Error In"=w3658) -> ("Error Out"=w3664:errorcluster, "APDClass out"=w3655:T41)  [unwired: 9 in]
            n1644 = call "DeConAPD1FGV.vi"("Error In"=w3658) -> ("Error Out"=w3666:errorcluster, "APDClass out"=w3657:T41)  [unwired: 9 in]
            n1645 = call "DeConAPD3FGV.vi"("Error In"=w3658) -> ("Error Out"=w3663:errorcluster, "APDClass out"=w3653:T41)  [unwired: 9 in]
            n1646 = Unbundle By Name(w3665) -> ("V1"=w3656:dbl, "V2"=w3654:dbl, "V3"=w3652:dbl)
            n1647 = call "getGain.vi"("CtrlV"=w3652, "APD"=w3653) -> ("gain"=w3643:dbl)  [unwired: 8 in, 1 out]
            n1648 = call "getGain.vi"("CtrlV"=w3656, "APD"=w3657) -> ("gain"=w3645:dbl)  [unwired: 8 in, 1 out]
            n1649 = call "getGain.vi"("CtrlV"=w3654, "APD"=w3655) -> ("gain"=w3644:dbl)  [unwired: 8 in, 1 out]
            n1650 = Less?(x=w3645, y="Ch1GainLim") -> (x < y?=w3650:bool)
            n1651 = Less?(x=w3644, y="Ch2&3GainLim") -> (x < y?=w3649:bool)
            n1652 = Less?(x=w3643, y="Ch2&3GainLim") -> (x < y?=w3648:bool)
            n1653 = Compound Arithmetic op=AND(w3650, w3649, w3648) -> (w3647:bool)
            n1654 = case shown="True" w3647 {
              tunnel: w3666 -> [_ w3736]
              tunnel: w3664 -> [_ w3735]
              tunnel: w3663 -> [_ w3734]
              tunnel: w3662 -> [_ w3724]
              tunnel: w3661 -> [_ w3723]
              tunnel: w3660 -> [_ w3722]
              tunnel: [w3667 w3683] -> w3659
              tunnel: w3658 -> [w3667 w3715]
              tunnel: w3657 -> [_ w3714]
              tunnel: w3656 -> [_ w3713]
              tunnel: w3655 -> [_ w3712]
              tunnel: w3654 -> [_ w3711]
              tunnel: w3653 -> [_ w3710]
              tunnel: w3652 -> [_ w3709]
              tunnel: [0.0 ("Gain4") w3678] -> w3646
              tunnel: w3645 -> [_ w3701]
              tunnel: w3644 -> [_ w3700]
              tunnel: w3643 -> [_ w3699]
              tunnel: w3641 -> [_ w3674]
              frame False {
                # "give probability of 0.5"
                # "if gain is out of acceptable range"
              }
              frame True {
                # "if gain is within range"
                n1655 = Build Array(w3701, w3700, w3699) -> (w3698:dbl[])
                n1656 = call "getIrf (SubVI).vi"("error in"=w3736, "CtrlV"=w3713, "APD"=w3714) -> ("error out"=w3728:errorcluster, "irfTNorm"=w3731:dbl[])  [unwired: 6 in, 1 out]
                n1657 = call "getIrf (SubVI).vi"("error in"=w3735, "CtrlV"=w3711, "APD"=w3712) -> ("error out"=w3727:errorcluster, "irfTNorm"=w3730:dbl[])  [unwired: 6 in, 1 out]
                n1658 = call "getIrf (SubVI).vi"("error in"=w3734, "CtrlV"=w3709, "APD"=w3710) -> ("error out"=w3726:errorcluster, "irfTNorm"=w3729:dbl[])  [unwired: 6 in, 1 out]
                n1659 = call "DotNetFGV.vi"("Error In"=w3715) -> ("Error Out"=w3719:errorcluster, "reference out"=w3720:refnum<k24>)  [unwired: 9 in]
                n1660 = local read "OverlaySelection"() -> (w3677:T9)
                n1661 = local read "BGAll"() -> (w3733:dbl[][])
                n1662 = Merge Errors(w3719, w3728, w3727, w3726) -> (w3725:errorcluster)
                n1663 = Build Array(w3731, w3730, w3729) -> (w3716:dbl[][])
                n1664 = Build Array (concatenate)(w3724, w3723, w3722) -> (w3721:dbl[][])
                n1665 = local write "iRF Graph"(w3716) -> ()
                n1666 = Transpose 2D Array(2D array=w3733) -> (transposed array=w3732:dbl[][])
                n1667 = Transpose 2D Array(2D array=w3716) -> (transposed array=w3717:dbl[][])
                n1668 = Transpose 2D Array(2D array=w3721) -> (transposed array=w3718:dbl[][])
                n1669 = Reciprocal(x=w3698) -> (1/x=w3696:dbl[])
                n1670 = call "LagDeConAllCh (SubVI).vi"("new reference"=w3720, "error in (no error)"=w3725, "irf"=w3717, "BG"=w3732, "WF"=w3718) -> ("error out"=w3684:errorcluster, "LCs"=w3692:dbl[][], "INTs"=w3703:dbl[][], "LTs"=w3708:dbl[][])  [unwired: 3 in]
                n1671 = Index Array(array=w3708, index (col)=0 ("disabled index (col)")) -> (element=w3690:dbl[])  [unwired: 1 in]
                n1672 = Index Array(array=w3703, index (col)=0 ("disabled index (col)")) -> (element=w3697:dbl[])  [unwired: 1 in]
                n1673 = Multiply(x=w3697, y=w3696) -> (x*y=w3695:dbl[])
                n1674 = Index Array(array=w3692, index (col)=0 ("disabled index (col)")) -> (element=w3688:dbl[])  [unwired: 1 in]
                n1675 = Add Array Elements(numeric array=w3695) -> (sum=w3694:dbl)
                n1676 = Index Array(array=w3690, index=0) -> (element=w3681:dbl)
                "Ch1 Lifetime (ns)" <- w3681
                n1677 = Index Array(array=w3690, index=1) -> (element=w3680:dbl)
                "Ch2 Lifetime (ns)" <- w3680
                n1678 = Index Array(array=w3690, index=2) -> (element=w3679:dbl)
                "Ch3 Lifetime (ns)" <- w3679
                n1679 = Divide(x=w3695, y=w3694) -> (x/y=w3689:dbl[])
                n1680 = case shown="\"Brain Classifier\"" w3677 {
                  tunnel: w3690 -> [_ w3741 _]
                  tunnel: w3689 -> [_ w3740 _]
                  tunnel: w3688 -> [_ w3739 w3745]
                  tunnel: [dbl[] [] w3738 w3742] -> w3673
                  frame "Gain", Default {
                  }
                  frame "HN Classifier" {
                    n1681 = Build Array (concatenate)(w3741, w3740, w3739) -> (w3738:dbl[])
                  }
                  frame "Brain Classifier" {
                    # "Ch2&3 Lag Coeffi"
                    n1682 = Array Subset(array=w3745, index=12, length=24) -> (w3742:dbl[])
                  }
                }
                "DeConOut" <- w3673
                n1683 = Bundle(w3681, w3680, w3679) -> (→"Lifetime (ns)":cluster{dbl, dbl, dbl})  [unwired: 1 in]
                n1684 = call "DebugTDMS_FGV.vi"() -> ("error out"=w3675:errorcluster, "tdms file out"=w3676:refnum<k34>)  [unwired: 10 in]
                n1685 = local read "module path"() -> (w3686:path)
                n1686 = local read "Python session"() -> (w3687:refnum<k35>)
                n1687 = node(w3687, w3686, "Predict" ("function name"), w3684, 0.0, w3673) -> (w3683:errorcluster, w3672:dbl)  [unwired: 1 in, 3 out]
                "Cancer Prob" <- w3672
                n1688 = disable-structure shown="Enabled" {
                  disable-tunnel: w3672 -> [w3748 w3753]
                  disable-tunnel: [w3747 w3749] -> w3678
                  frame Disabled {
                    n1689 = Add(x=0.01, y=w3748) -> (x+y=w3747:dbl)
                  }
                  frame Enabled {
                    n1690 = Greater?(x=w3753, y="CancerThreshold") -> (0:w3754:bool)
                    n1691 = Select(t=1.0, s=w3754, f=0.01) -> (s? t:f=w3749:dbl)
                  }
                }
                n1692 = Build Array (concatenate)(w3674, w3673, w3672) -> (w3671:dbl[])
                n1693 = TDMS Write(0:w3676, 7:string[] ["DataAll"] ("channel name(s) in (Untitled)"), 9:w3671, 11:w3675) -> (15:→"error out":errorcluster)  [unwired: 2 in, 3 out]
              }
            }
          }
        }
        n1694 = Bundle("idx"=w3619, "f"=w3625) -> (w3623:cluster{"idx":i32, "f":dbl})  [unwired: 1 in]
        n1695 = Send Notification(notification=w3623, notifier=w3624, error in (no error)=w3622) -> (notifier out=w3621:refnum<notifier>, error out=w3620:errorcluster)
      }
      frame "BG", Default {
        # "if not acquiting data"
      }
    }
    n1696 = call "AvgArrayTimeCritical.vi"("2D array"=w3594) -> ("1D Avg"=w3601:dbl[])  [unwired: 10 in]
    n1697 = call "AvgArrayTimeCritical.vi"("2D array"=w3593) -> ("1D Avg"=w3602:dbl[])  [unwired: 10 in]
    n1698 = call "AvgArrayTimeCritical.vi"("2D array"=w3592) -> ("1D Avg"=w3603:dbl[])  [unwired: 10 in]
    n1699 = call "AvgArrayTimeCritical.vi"("2D array"=w3600) -> ("1D Avg"=w3604:dbl[])  [unwired: 10 in]
    n1700 = Build Array(w3604) -> (w3599:dbl[][])
    n1701 = Build Array(w3603) -> (w3598:dbl[][])
    n1702 = Build Array(w3602) -> (w3597:dbl[][])
    n1703 = Build Array(w3601) -> (w3596:dbl[][])
    n1704 = flat-sequence {
      tunnel: [w3757] -> w3609
      tunnel: w3589 -> [_]
      frame #0 {
        n1705 = call <vilib>:"High Resolution Relative Seconds.vi"() -> ("relative seconds"=w3757:dbl)
      }
    }
    n1706 = Subtract(x=w3609, y=w3610) -> (x-y=w3612:dbl)
    n1707 = Multiply(x=w3612, y=1000.0) -> (x*y=→"Decon Loop timing (ms)" →"DeCon Speed(ms)":dbl)
    n1708 = Bundle(w3596, w3597, w3598, w3599, "V cluster"=w3595) -> (w3615:T51)  [unwired: 1 in]
    n1709 = Send Notification(notification=w3615, notifier=w3614, error in (no error)=w3589) -> (notifier out=w3613:refnum<notifier>, error out=w3591:errorcluster)
    n1710 = Merge Errors(w3586, w3591) -> (→"decon error out":errorcluster)
  }
  n1711 = while {
    tunnel: w18 -> [w3769]
    shift-right: [w3762] -> _
    shift-left: u32 0 -> [w3763]
    stop <- w3760 stop-if-true
    # "Send data to AB computer here"
    # "if TCP ip is not open loop will run once and stop. To re-establish connection and start this loop. Reboot softwrae."
    # "Data communication loop"
    n1712 = Wait on Notification(notifier=w3769, ignore previous (F)=FALSE) -> (notification=w3767:cluster{"idx":i32, "lifetime":dbl}, error out=w3761:errorcluster)  [unwired: 2 in, 2 out]
    n1713 = Wait Until Next ms Multiple(millisecond multiple=u32 25) -> ()  [unwired: 1 out]
    n1714 = Unbundle(w3767) -> ("idx"=w3766:i32, "lifetime"=w3765:dbl)
    n1715 = Tick Count (ms)() -> (millisecond timer value=w3762:u32)
    n1716 = global read "GlobalVariables.vi" "TCP connected?"() -> (w3759:bool)
    n1717 = Subtract(x=w3762, y=w3763) -> (x-y=→"Communication loop(ms)":u32)
    n1718 = case shown="True" w3759 {
      tunnel: w3766 -> [_ w3778]
      tunnel: w3765 -> [_ w3777]
      tunnel: w3761 -> [w3770 w3774]
      tunnel: [w3770 w3771] -> w3760
      frame False {
      }
      frame True {
        n1719 = Number To Decimal String(number=w3778) -> (decimal integer string=w3786:string)  [unwired: 1 in]
        n1720 = call "TcpIDFGV.vi"("Error In"=w3774, "action"=enum16{"write", "read"}."read") -> ("Error Out"=w3773:errorcluster, "connection ID out"=w3784:refnum<k5>)  [unwired: 8 in]
        n1721 = Concatenate Strings("!idx:", w3786) -> (w3787:string)
        n1722 = call "TCP_WriteRead.vi"("error in (no error)"=w3773, "data in"=w3787, "connectin ID in"=w3784) -> ("error out"=w3772:errorcluster, "connectin ID out"=w3785:refnum<k5>)  [unwired: 4 in, 1 out]
        n1723 = Number To Fractional String(number=w3777, precision (6)=i16 2) -> (F-format string=w3776:string)  [unwired: 2 in]
        n1724 = Concatenate Strings("!lifetime:", w3776) -> (w3783:string)
        n1725 = call "TCP_WriteRead.vi"("error in (no error)"=w3772, "data in"=w3783, "connectin ID in"=w3785) -> ("error out"=w3771:errorcluster, "data out"=→"data out(communcation loop)":string)  [unwired: 4 in, 1 out]
      }
    }
  }
  n1726 = while {
    tunnel: w13 -> [w3798]
    shift-right: [w3789] -> _
    shift-left: w15 -> [w3796]
    shift-right: [w3791] -> _
    shift-left: w15 -> [w3790]
    i -> [w3792]
    stop <- w3793 stop-if-true
    # "Data display loop(30Hz)"
    n1727 = Wait on Notification(notifier=w3798, ignore previous (F)=FALSE) -> (notification=w3794:T14, error out=w3793:errorcluster)  [unwired: 2 in, 2 out]
    n1728 = Wait Until Next ms Multiple(millisecond multiple=u32 40) -> ()  [unwired: 1 out]
    n1729 = Tick Count (ms)() -> (millisecond timer value=w3789:u32)
    n1730 = Subtract(x=w3789, y=w3796) -> (x-y=→"display loop timing(ms)":u32)
    n1731 = case shown="No Error" w3793 {
      tunnel: w3794 -> [w3871 _]
      tunnel: w3790 -> [w3843 w3943]
      tunnel: [w3845 w3943] -> w3791
      tunnel: w3789 -> [w3842 _]
      frame No Error {
        w3800 = u32 1 ("Active Plot")
        w3819 = 0 ("index (row)")
        n1732 = Subtract(x=w3842, y=w3843) -> (x-y=w3844:u32)
        n1733 = Unbundle(w3871) -> ("CH1"=w3866:dbl[][], "CH2"=w3864:dbl[][], "CH3"=w3861:dbl[][], "CH4"=w3814:dbl[][], "Gain cluster"=w3820:cluster{"V1":dbl, "V2":dbl, "V3":dbl, "V4":dbl})
        n1734 = Unbundle By Name(w3820) -> ("V1"=w3838:dbl, "V2"=w3836:dbl, "V3"=w3834:dbl, "V4"=w3812:dbl)
        n1735 = Index Array(array=w3866, index (row)=w3819) -> (element=w3850:dbl[])  [unwired: 1 in]
        n1736 = Index Array(array=w3864, index (row)=w3819) -> (element=w3848:dbl[])  [unwired: 1 in]
        n1737 = Index Array(array=w3861, index (row)=w3819) -> (element=w3849:dbl[])  [unwired: 1 in]
        n1738 = Index Array(array=w3814, index (row)=w3819) -> (element=w3818:dbl[])  [unwired: 1 in]
        n1739 = call "RemoveDCBG.vi"("Channel"=enum16{"DC Only", "Ch1", "Ch2", "Ch3", "Ch4"}."Ch4", "WF in"=w3818) -> ("DC"=w3816:dbl, "WF out"=w3805:dbl[])  [unwired: 7 in, 1 out]
        n1740 = Greater?(x=w3844, y=u32 200) -> (0:w3846:bool)
        n1741 = call "CtrlVtoGain.vi"("CtrlV(V)"=w3812, "Channel"=enum16{"Ch1", "Ch2", "Ch3", "Ch4"}."Ch4") -> ("Gain"=w3804:dbl)  [unwired: 8 in, 1 out]
        n1742 = call "CtrlVtoGain.vi"("CtrlV(V)"=w3838, "Channel"=enum16{"Ch1", "Ch2", "Ch3"}."Ch1") -> ("Gain"=w3832:dbl)  [unwired: 8 in, 1 out]
        n1743 = call "RemoveDCBG.vi"("Channel"=enum16{"DC Only", "Ch1", "Ch2", "Ch3"}."Ch1", "WF in"=w3850) -> ("DC"=w3867:dbl, "WF out"=w3839:dbl[])  [unwired: 7 in, 1 out]
        n1744 = call "RemoveDCBG.vi"("Channel"=enum16{"DC Only", "Ch1", "Ch2", "Ch3"}."Ch2", "WF in"=w3848) -> ("DC"=w3863:dbl, "WF out"=w3840:dbl[])  [unwired: 7 in, 1 out]
        n1745 = call "CtrlVtoGain.vi"("CtrlV(V)"=w3836, "Channel"=enum16{"Ch1", "Ch2", "Ch3"}."Ch2") -> ("Gain"=w3827:dbl)  [unwired: 8 in, 1 out]
        n1746 = call "RemoveDCBG.vi"("Channel"=enum16{"DC Only", "Ch1", "Ch2", "Ch3"}."Ch3", "WF in"=w3849) -> ("DC"=w3860:dbl, "WF out"=w3841:dbl[])  [unwired: 7 in, 1 out]
        n1747 = call "CtrlVtoGain.vi"("CtrlV(V)"=w3834, "Channel"=enum16{"Ch1", "Ch2", "Ch3"}."Ch3") -> ("Gain"=w3823:dbl)  [unwired: 8 in, 1 out]
        n1748 = formula code="int32 out = 2;\nif (G<5){\nout = 1;\n}\nif (G>200){\nout = 3;\n}"("G"=w3804) -> ("out"=→"output variable":i32)
        n1749 = Add(x=w3805, y=w3816) -> (x+y=w3815:dbl[])
        n1750 = Less?(x=w3804, y=5.0) -> (x < y?=w3810:bool)
        n1751 = case shown="True" w3846 {
          tunnel: w3839 -> [_ w3900]
          tunnel: w3840 -> [_ w3903]
          tunnel: w3841 -> [_ w3902]
          tunnel: w3842 -> [_ w3918]
          tunnel: [w3882 w3918] -> w3845
          tunnel: w3843 -> [w3882 _]
          tunnel: w3832 -> [_ w3896]
          tunnel: w3827 -> [_ w3895]
          tunnel: w3823 -> [_ w3894]
          tunnel: w3805 -> [_ w3890]
          tunnel: w3804 -> [_ w3887]
          frame False {
          }
          frame True {
            n1752 = call "GetSNR(SubVI).vi"("Waveform"=w3900) -> ("SNR"=→"SNR1":dbl)  [unwired: 10 in]
            n1753 = Array Size(array=w3900) -> (size(s)=w3901:i32)
            n1754 = call "GetSNR(SubVI).vi"("Waveform"=w3903) -> ("SNR"=→"SNR2":dbl)  [unwired: 10 in]
            n1755 = call "GetSNR(SubVI).vi"("Waveform"=w3902) -> ("SNR"=→"SNR3":dbl)  [unwired: 10 in]
            n1756 = call "GetSNR(SubVI).vi"("Waveform"=w3890) -> ("SNR"=→"SNR4":dbl)  [unwired: 10 in]
            n1757 = global read "GlobalVariables.vi" "BG Idx2"() -> (w3889:i32)
            n1758 = Subtract(x=w3901, y=w3889) -> (x-y=w3888:i32)
            n1759 = Array Subset(array=w3900, index=w3889, length=w3888) -> (w3907:dbl[])
            n1760 = Array Subset(array=w3903, index=w3889, length=w3888) -> (w3909:dbl[])
            n1761 = Array Subset(array=w3902, index=w3889, length=w3888) -> (w3911:dbl[])
            n1762 = Array Subset(array=w3890, index=w3889, length=w3888) -> (w3891:dbl[])
            n1763 = Add Array Elements(numeric array=w3907) -> (sum=w3908:dbl)
            n1764 = Add Array Elements(numeric array=w3909) -> (sum=w3910:dbl)
            n1765 = Add Array Elements(numeric array=w3911) -> (sum=w3912:dbl)
            n1766 = Add Array Elements(numeric array=w3891) -> (sum=w3892:dbl)
            n1767 = Divide(x=w3908, y=w3896) -> (x/y=w3913:dbl)
            n1768 = Divide(x=w3910, y=w3895) -> (x/y=w3914:dbl)
            n1769 = Divide(x=w3912, y=w3894) -> (x/y=w3915:dbl)
            n1770 = Divide(x=w3892, y=w3887) -> (x/y=w3886:dbl)
            n1771 = Build Array(w3913, w3914, w3915, w3886) -> (w3916:dbl[])
            n1772 = Add Array Elements(numeric array=w3916) -> (sum=w3917:dbl)
            n1773 = Divide(x=w3916, y=w3917) -> (x/y=w3885:dbl[])
            n1774 = Index Array(array=w3885, index=2) -> (element=→"IntR3":dbl)
            n1775 = Index Array(array=w3885, index=1) -> (element=→"IntR2":dbl)
            n1776 = Index Array(array=w3885, index=0) -> (element=→"IntR1":dbl)
            n1777 = Index Array(array=w3885, index=3) -> (element=→"IntR4":dbl)
          }
        }
        n1778 = Add(x=w3839, y=w3867) -> (x+y=w3865:dbl[])
        n1779 = Add(x=w3840, y=w3863) -> (x+y=w3862:dbl[])
        n1780 = Add(x=w3841, y=w3860) -> (x+y=w3859:dbl[])
        n1781 = Less?(x=w3832, y=5.0 ("x")) -> (x < y?=w3830:bool)
        n1782 = Less?(x=w3827, y=5.0 ("x")) -> (x < y?=w3826:bool)
        n1783 = Less?(x=w3823, y=5.0 ("x")) -> (x < y?=w3822:bool)
        n1784 = case shown="False" w3822 {
          tunnel: [u32 16448250 ("Plot.Plot Color") u32 16711680 ("Plot.Plot Color")] -> w3821
          frame False {
          }
          frame True {
          }
        }
        n1785 = case shown="True" "Show BG removed?" {
          tunnel: w3866 -> [w3925 w3941]
          tunnel: w3865 -> [_ w3931]
          tunnel: [w3925 w3940] -> w3858
          tunnel: w3864 -> [w3924 w3939]
          tunnel: [w3924 w3938] -> w3802
          tunnel: w3862 -> [_ w3927]
          tunnel: w3861 -> [w3923 w3937]
          tunnel: [w3923 w3936] -> w3853
          tunnel: w3859 -> [_ w3932]
          tunnel: [w3922 w3935] -> w3809
          tunnel: w3815 -> [_ w3929]
          tunnel: w3814 -> [w3922 w3934]
          frame False {
          }
          frame True {
            n1786 = Insert Into Array(array=w3937, index (row)=1, new element=w3932) -> (w3936:dbl[][])  [unwired: 1 in]
            n1787 = Insert Into Array(array=w3941, index (row)=1, new element=w3931) -> (w3940:dbl[][])  [unwired: 1 in]
            n1788 = Insert Into Array(array=w3939, index (row)=1, new element=w3927) -> (w3938:dbl[][])  [unwired: 1 in]
            n1789 = Insert Into Array(array=w3934, index (row)=1, new element=w3929) -> (w3935:dbl[][])  [unwired: 1 in]
          }
        }
        "Channel 1" <- w3858
        "Channel 2" <- w3802
        "Channel 3" <- w3853
        "Channel 4" <- w3809
        n1790 = case shown="False" w3830 {
          tunnel: [u32 16448250 ("Plot.Plot Color") u32 16711680 ("Plot.Plot Color")] -> w3829
          frame False {
          }
          frame True {
          }
        }
        n1791 = case shown="False" w3826 {
          tunnel: [u32 16448250 ("Plot.Plot Color") u32 16711680 ("Plot.Plot Color")] -> w3825
          frame False {
          }
          frame True {
          }
        }
        n1792 = case shown="False" w3810 {
          tunnel: [u32 16448250 ("Plot.Plot Color") u32 16711680 ("Plot.Plot Color")] -> w3806
          frame False {
          }
          frame True {
          }
        }
        n1793 = case shown="False" "Show BG removed?" {
          tunnel: [u32 16744703 ("Plot.Plot Color") u32 16741120 ("Plot.Plot Color")] -> w3799
          frame False {
          }
          frame True {
          }
        }
        n1794 = property on="Channel 1" class="WFGraph (strict)"("Active Plot"=w3800, "Plot.Plot Color"=w3799, "Plot.Line Style"=u8 1, "Plot.Line Width"=u8 2, "BG Color"=w3829) -> ()  [unwired: 2 in, 2 out]
        n1795 = property on="Channel 2" class="WFGraph (strict)"("Active Plot"=w3800, "Plot.Plot Color"=w3799, "Plot.Line Style"=u8 1, "Plot.Line Width"=u8 2, "BG Color"=w3825) -> ()  [unwired: 2 in, 2 out]
        n1796 = property on="Channel 4" class="WFGraph (strict)"("Active Plot"=w3800, "Plot.Plot Color"=w3799, "Plot.Line Style"=u8 1, "Plot.Line Width"=u8 2, "BG Color"=w3806) -> ()  [unwired: 2 in, 2 out]
        n1797 = property on="Channel 3" class="WFGraph (strict)"("Active Plot"=w3800, "Plot.Plot Color"=w3799, "Plot.Line Style"=u8 1, "Plot.Line Width"=u8 2, "BG Color"=w3821) -> ()  [unwired: 2 in, 2 out]
      }
      frame Error {
        w3942 = u32 16448250 ("Plot Area:Colors:BG Color")
        n1798 = property on="Channel 1" class="WFGraph (strict)"("BG Color"=w3942) -> ()  [unwired: 2 in, 2 out]
        n1799 = property on="Channel 2" class="WFGraph (strict)"("BG Color"=w3942) -> ()  [unwired: 2 in, 2 out]
        n1800 = property on="Channel 3" class="WFGraph (strict)"("BG Color"=w3942) -> ()  [unwired: 2 in, 2 out]
      }
    }
    "DisplayLoop" <- w3792
  }
  n1801 = while {
    tunnel: w65 -> [w3956]
    tunnel: w55 -> [w3955]
    tunnel: [w3954] -> w63
    tunnel: w19 -> [w3953]
    tunnel: [w3952] -> w59
    tunnel: w39 -> [w3950]
    tunnel: w48 -> [w3949]
    tunnel: w35 -> [w3944]
    stop <- w3947 stop-if-true
    # "acquire data and send it to processing loop"
    # "Data Aquisition Loop"
    n1802 = event shown="[1] <Start digitizer>: User Event" {
      selector: w3955 -> [_ _]
      dyn-events: [_ _] -> w3954
      timeout: 30 -> [_ _]
      tunnel: w3956 -> [w3962 w3972]
      tunnel: [w3957 _] -> w3947
      tunnel: w3953 -> [w3961 w3979]
      tunnel: [w3961 w3978] -> w3952
      tunnel: w3950 -> [_ w3976]
      tunnel: w3949 -> [w3960 w3971]
      tunnel: w3944 -> [_ w3969]
      event Timeout {
        # "use queue to stop data loop\nwhen queue ref is released, error will stop this loop"
        n1803 = event-data() -> ()  [unwired: 1 in, 3 out]
        n1804 = Get Queue Status(queue=w3962) -> (error out=w3959:errorcluster)  [unwired: 2 in, 7 out]
        n1805 = Get Queue Status(queue=w3960) -> (error out=w3958:errorcluster)  [unwired: 2 in, 7 out]
        n1806 = Merge Errors(w3959, w3958) -> (w3957:errorcluster)
      }
      event User Event {
        w3977 = enum16{"Write", "Read"}."Read" ("Operation")
        n1807 = event-data() -> ("Time"=→"RunStartTime":u32)  [unwired: 1 in, 3 out]
        n1808 = call "FLImDAQ_FGV.vi"() -> ("Read data"=w3974:T5)  [unwired: 10 in, 1 out]
        n1809 = call "Digitizer1_FGV.vi"("Operation (Read)"=w3977) -> ("Read data"=w3968:refnum<k15>)  [unwired: 9 in, 1 out]
        n1810 = call "Digitizer2_FGV.vi"("Operation (Read)"=w3977) -> ("Read data"=w3975:refnum<k15>)  [unwired: 9 in, 1 out]
        n1811 = Unbundle By Name(w3974) -> ("Waveform to Avg"=w3973:i16)
        n1812 = property on="Property Node" class="niScope"(reference=w3968) -> (reference out=w3967:refnum<k15>, "Vertical Range"=w3966, "Vertical Offset"=w3965)  [unwired: 1 in, 1 out]
        n1813 = Tick Count (ms)() -> (millisecond timer value=w3964:u32)
        n1814 = while {
          tunnel: w3979 -> [w4039]
          tunnel: [w4038] -> w3978
          tunnel: w3975 -> [w4032]
          tunnel: w3967 -> [w4031]
          tunnel: w3976 -> [w4030]
          shift-right: [w3999] -> _
          shift-left: u32 0 ("millisecond timer value") -> [w4024]
          tunnel: w3973 -> [w3980]
          tunnel: w3972 -> [w4021]
          tunnel: w3971 -> [w4019]
          tunnel: w3969 -> [w4012]
          tunnel: w3966 -> [w4009]
          tunnel: w3965 -> [w4010]
          shift-right: [w4004] -> _
          shift-left: w3964 -> [w4003]
          i -> [w3981]
          stop <- w4002 stop-if-true
          w3992 = enum16{"write", "read"}."read" ("action")
          w4025 = 65536
          # "enqueue V"
          # "enqueue ch3 data"
          # "enqueue ch1&2 data"
          # "acquire ch3"
          # "acquire ch1&2"
          # "send data for processing"
          n1815 = Multiply(x=w3980, y=w3981) -> (x*y=w3989:i32)
          "Fetch Record #" <- w3989
          n1816 = property on="Property Node" class="niScope"(reference=w4031, "Fetch Record Number"=w3989) -> (reference out=w4043:refnum<k15>, error out=w4042:errorcluster, "Records Done"=w4011)  [unwired: 1 in]
          n1817 = Subtract(x=w4011, y=w3989) -> (x-y=→"Record Backlog":i32)
          n1818 = call-poly <instrlib>:"niScope Fetch (poly).vi"("timeout"=1.0, "error in"=w4042, "channels"="0,1", "instrument handle"=w4043) -> ("error out"=w3986:errorcluster, "wfm"=w3987:i16[][], "wfm info"=w4008:T52)  [unwired: 4 in, 1 out]
          n1819 = property on="Property Node" class="niScope"(reference=w4032, "Fetch Record Number"=w3989) -> (reference out=w4036:refnum<k15>, error out=w4033:errorcluster, "Records Done"=w3990)  [unwired: 1 in]
          n1820 = Divide(x=w3987, y=w4025) -> (x/y=w3998:dbl[][])
          n1821 = Tick Count (ms)() -> (millisecond timer value=w3999:u32)
          n1822 = Subtract(x=w3990, y=w3989) -> (x-y=→"Record Backlog 2":i32)
          n1823 = Subtract(x=w3999, y=w4024) -> (x-y=→"Aquisition loop timing(ms)":u32)
          n1824 = Subtract(x=w3999, y=w4003) -> (x-y=w4007:u32)
          n1825 = Multiply(x=w3998, y=w4009) -> (x*y=w4029:dbl[][])
          n1826 = call-poly <instrlib>:"niScope Fetch (poly).vi"("timeout"=0.25, "error in"=w4033, "channels"="0,1", "instrument handle"=w4036) -> ("error out"=w3985:errorcluster, "wfm"=w4026:i16[][])  [unwired: 4 in, 2 out]
          n1827 = Greater?(x=w4007, y=u32 1000) -> (0:w4005:bool)
          n1828 = Add(x=w4029, y=w4010) -> (x+y=w4020:dbl[][])
          n1829 = case shown="True" w4005 {
            tunnel: w4008 -> [_ w4052]
            tunnel: w3999 -> [_ w4051]
            tunnel: [w4045 w4051] -> w4004
            tunnel: w4003 -> [w4045 _]
            tunnel: [errorcluster {"status"=FALSE, "code"=0, "source"=""} ("error constant") w4048] -> w4000
            frame False {
            }
            frame True {
              # "[Covers: REQ29]"
              n1830 = call "CheckFrequency(SubVI).vi"("wfm info"=w4052) -> ("f (Hz)"=w4050:dbl)  [unwired: 10 in]
              "Laser f (Hz)" <- w4050
              n1831 = local read "Laser Rep Rate"() -> (w4047:dbl)
              n1832 = Increment(x=w4047) -> (x+1=w4046:dbl)
              n1833 = Greater?(x=w4050, y=w4046) -> (0:w4049:bool)
              n1834 = case shown="True" w4049 {
                tunnel: [errorcluster {"status"=FALSE, "code"=0, "source"=""} ("error constant") errorcluster {"status"=TRUE, "code"=0, "source"=""} ("error constant")] -> w4048
                frame False {
                }
                frame True {
                }
              }
            }
          }
          n1835 = Divide(x=w4026, y=w4025) -> (x/y=w4028:dbl[][])
          n1836 = Enqueue Element(queue=w4021, element=w4020, error in (no error)=w3986) -> (error out=w3984:errorcluster)  [unwired: 1 in, 2 out]
          n1837 = Multiply(x=w4028, y=w4009) -> (x*y=w4027:dbl[][])
          n1838 = Add(x=w4027, y=w4010) -> (x+y=w4018:dbl[][])
          n1839 = Enqueue Element(queue=w4019, element=w4018, error in (no error)=w3985) -> (error out=w3983:errorcluster)  [unwired: 1 in, 2 out]
          n1840 = Merge Errors(w3984, w3983) -> (w3982:errorcluster)
          n1841 = call "V1FGV.vi"("Error In"=w3982, "action (write)"=w3992) -> ("Error Out"=w4016:errorcluster, "V1 out"=w4014:dbl)  [unwired: 8 in]
          n1842 = call "V2FGV.vi"("Error In"=w4016, "action(write)"=w3992) -> ("Error Out"=w4015:errorcluster, "V2 out"=w4013:dbl)  [unwired: 8 in]
          n1843 = call "V3FGV.vi"("Error In"=w4015, "action(write)"=w3992) -> ("Error Out"=w3995:errorcluster, "V3 out"=w3994:dbl)  [unwired: 8 in]
          n1844 = call "V4FGV.vi"("Error In"=w3995, "action(write)"=w3992, "V3 in"=w3994) -> ("Error Out"=w3993:errorcluster, "V3 out"=w3991:dbl)  [unwired: 7 in]
          n1845 = Bundle("V1 out"=w4014, "V2 out"=w4013, "V3 out"=w3994, "V3 out"=w3991) -> (w3997:T53)  [unwired: 1 in]
          n1846 = Bundle(w3981, w4020, w4018, w3997) -> (w4022:T54)  [unwired: 1 in]
          n1847 = Enqueue Element(queue=w4012, element=w3997, error in (no error)=w3993) -> (error out=w3996:errorcluster)  [unwired: 1 in, 2 out]
          n1848 = Send Notification(notification=w4022, notifier=w4039, error in (no error)=w3996) -> (notifier out=w4038:refnum<notifier>, error out=w4001:errorcluster)
          n1849 = Merge Errors(w4000, w4001) -> (w4017:errorcluster)
          n1850 = case shown="Error .." w4017 {
            selector: w4017 -> [w4055 w4056]
            tunnel: w4030 -> [_ w4059]
            tunnel: [w4055 w4056] -> w4002
            frame No Error {
            }
            frame Error {
              # "Send user event to signal aquisition has stoped"
              n1851 = Generate User Event(priority (normal)=usereventprio."high priority", user event=w4059, event data cluster=TRUE ("event data")) -> ()  [unwired: 1 in, 2 out]
            }
          }
          "aquisition loop Error Out" <- w4002
          "Auisition Loop idx" <- w3981
        }
      }
    }
    n1852 = Unbundle By Name(w3947) -> ("status"=w3946:bool)
    n1853 = Not(x=w3946) -> (.not. x?=w3945:bool)
    n1854 = local write "Aq Loop?"(w3945) -> ()
    "Aq Loop?" <- TRUE ("Aq L?")
  }
  n1855 = disable-structure "Diagram Disable Structure" shown="Disabled" {
    frame Disabled {
      w4060 = T55 {"Horizontal"=500, "Vertical"=100}  # Top Left Corner
      n1856 = Control Help Window(0:w4060, 1:TRUE ("Show")) -> ()
      n1857 = call <vilib>:"TDMS - File Viewer.vi"() -> ()  [unwired: 6 in, 2 out]
    }
    frame Enabled {
    }
  }
  n1858 = while {
    tunnel: w19 -> [w4109]
    shift-right: [w4073] -> _
    shift-left: _ -> [w4105]
    tunnel: [w4064] -> w1 mode=indexing
    i -> [w4089]
    stop <- w4070 stop-if-true
    # "Channel 3"
    # "Channel 2"
    # "Channel 1"
    # "use FGV for gain value"
    # "stop on error"
    # "Gain adjustment and Data processing"
    n1859 = Tick Count (ms)() -> (millisecond timer value=w4073:u32)
    n1860 = Wait on Notification(notifier=w4109, ignore previous (F)=TRUE) -> (notification=w4083:T15, error out=w4063:errorcluster)  [unwired: 2 in, 2 out]
    n1861 = Subtract(x=w4073, y=w4105) -> (x-y=→"PID loop timing(ms)":u32)
    n1862 = Unbundle(w4083) -> ("CH1&2"=w4099:dbl[][], "CH3&4"=w4098:dbl[][])  [unwired: 2 out]
    n1863 = call "SeperateChanData.vi"("Input (Ch1&2)"=w4099) -> ("Ch1"=w4094:dbl[][], "Ch2"=w4092:dbl[][])
    n1864 = call "SeperateChanData.vi"("Input (Ch1&2)"=w4098) -> ("Ch1"=w4088:dbl[][], "Ch2"=w4081:dbl[][])
    n1865 = call "AvgArrayTimeCritical.vi"("2D array"=w4094) -> ("1D Avg"=w4093:dbl[])  [unwired: 10 in]
    n1866 = call "AvgArrayTimeCritical.vi"("2D array"=w4092) -> ("1D Avg"=w4103:dbl[])  [unwired: 10 in]
    n1867 = call "AvgArrayTimeCritical.vi"("2D array"=w4088) -> ("1D Avg"=w4100:dbl[])  [unwired: 10 in]
    n1868 = call "AvgArrayTimeCritical.vi"("2D array"=w4081) -> ("1D Avg"=w4080:dbl[])  [unwired: 10 in]
    n1869 = Array Max & Min(array=w4093) -> (max value=w4091:dbl)  [unwired: 3 out]
    n1870 = Array Max & Min(array=w4103) -> (max value=w4090:dbl)  [unwired: 3 out]
    n1871 = Array Max & Min(array=w4100) -> (max value=w4074:dbl)  [unwired: 3 out]
    n1872 = Array Max & Min(array=w4080) -> (max value=w4078:dbl)  [unwired: 3 out]
    n1873 = local read "Auto gain ch4"() -> (w4079:bool)
    n1874 = local read "Auto gain ch1"() -> (w4097:bool)
    n1875 = local read "Auto gain ch2"() -> (w4096:bool)
    n1876 = local read "Auto gain ch3"() -> (w4095:bool)
    n1877 = case shown="True" w4079 {
      tunnel: w4078 -> [_ w4156]
      tunnel: "V target(1.0)" -> [_ w4154]
      tunnel: [FALSE w4151] -> w4076
      tunnel: [0.0 ("CtrlV") w4146] -> w4077
      frame False {
        # "Manual control"
      }
      frame True {
        # "PID control"
        n1878 = global read "GlobalVariables.vi" "Ch4GainLim(Log)"() -> (w4157)
        n1879 = call-poly <vilib>:"PID.vi"("output range"=w4157, "PID gains"="Ch4 PID gains", "process variable"=w4156, "setpoint"=w4154) -> ("output"=w4155:dbl)  [unwired: 6 in, 1 out]
        n1880 = Power Of 10(x=w4155) -> (10^x=w4147:dbl)
        "Gain4" <- w4147
        n1881 = call "V4FGV.vi"("action(write)"=enum16{"write", "read"}."read") -> ("Error Out"=w4150:errorcluster, "V3 out"=w4152:dbl)  [unwired: 9 in]
        n1882 = call "GainToCtrlV.vi"("Gain"=w4147, "Channel"=enum16{"Ch1", "Ch2", "Ch3", "Ch4"}."Ch4") -> ("CtrlV"=w4146:dbl)  [unwired: 8 in, 1 out]
        n1883 = call "V4FGV.vi"("Error In"=w4150, "V3 in"=w4146) -> ()  [unwired: 8 in, 2 out]
        n1884 = local write "V 4"(w4146) -> ()
        n1885 = Not Equal?(x=w4146, y=w4152) -> (x != y?=w4151:bool)
      }
    }
    n1886 = case shown="True" w4097 {
      tunnel: "V target(1.0)" -> [_ w4171]
      tunnel: w4091 -> [_ w4168]
      tunnel: [0.0 ("CtrlV") w4160] -> w4071
      tunnel: [FALSE w4162] -> w4087
      frame False {
        # "Manual control"
      }
      frame True {
        # "PID control"
        n1887 = global read "GlobalVariables.vi" "Ch1GainLim(Log)"() -> (w4167:cluster{"GainMax":dbl, "GainMin":dbl})
        n1888 = call-poly <vilib>:"PID.vi"("output range"=w4167, "PID gains"="Ch1 PID gains", "process variable"=w4168, "setpoint"=w4171) -> ("output"=w4166:dbl)  [unwired: 6 in, 1 out]
        n1889 = Power Of 10(x=w4166) -> (10^x=w4165:dbl)
        "Gain1" <- w4165
        n1890 = call "V1FGV.vi"("action (write)"=enum16{"write", "read"}."read") -> ("Error Out"=w4161:errorcluster, "V1 out"=w4163:dbl)  [unwired: 9 in]
        n1891 = call "GainToCtrlV.vi"("Gain"=w4165, "Channel"=enum16{"Ch1", "Ch2", "Ch3"}."Ch1") -> ("CtrlV"=w4160:dbl)  [unwired: 8 in, 1 out]
        n1892 = local write "V 1"(w4160) -> ()
        n1893 = call "V1FGV.vi"("Error In"=w4161, "V1 in"=w4160) -> ()  [unwired: 8 in, 2 out]
        n1894 = Not Equal?(x=w4160, y=w4163) -> (x != y?=w4162:bool)
      }
    }
    n1895 = case shown="True" w4096 {
      tunnel: w4090 -> [_ w4198]
      tunnel: "V target(1.0)" -> [_ w4199]
      tunnel: [FALSE w4192] -> w4086
      tunnel: [0.0 ("CtrlV") w4188] -> w4082
      frame False {
        # "Manual control"
      }
      frame True {
        # "PID control"
        n1896 = global read "GlobalVariables.vi" "Ch2GainLim(Log)"() -> (w4196:cluster{"GainMax":dbl, "GainMin":dbl})
        n1897 = call-poly <vilib>:"PID.vi"("output range"=w4196, "PID gains"="Ch2 PID gains", "process variable"=w4198, "setpoint"=w4199) -> ("output"=w4195:dbl)  [unwired: 6 in, 1 out]
        n1898 = Power Of 10(x=w4195) -> (10^x=w4193:dbl)
        "Gain2" <- w4193
        n1899 = call "V2FGV.vi"("action(write)"=enum16{"write", "read"}."read") -> ("Error Out"=w4189:errorcluster, "V2 out"=w4190:dbl)  [unwired: 9 in]
        n1900 = call "GainToCtrlV.vi"("Gain"=w4193, "Channel"=enum16{"Ch1", "Ch2", "Ch3"}."Ch2") -> ("CtrlV"=w4188:dbl)  [unwired: 8 in, 1 out]
        n1901 = local write "V 2"(w4188) -> ()
        n1902 = call "V2FGV.vi"("Error In"=w4189, "V2 in"=w4188) -> ()  [unwired: 8 in, 2 out]
        n1903 = Not Equal?(x=w4188, y=w4190) -> (x != y?=w4192:bool)
      }
    }
    n1904 = case shown="True" w4095 {
      tunnel: w4074 -> [_ w4183]
      tunnel: "V target(1.0)" -> [_ w4180]
      tunnel: [FALSE w4176] -> w4085
      tunnel: [0.0 ("CtrlV") w4174] -> w4084
      frame False {
        # "Manual control"
      }
      frame True {
        # "PID control"
        n1905 = global read "GlobalVariables.vi" "Ch3GainLim(Log)"() -> (w4184:cluster{"GainMax":dbl, "GainMin":dbl})
        n1906 = call-poly <vilib>:"PID.vi"("output range"=w4184, "PID gains"="Ch3 PID gains", "process variable"=w4183, "setpoint"=w4180) -> ("output"=w4182:dbl)  [unwired: 6 in, 1 out]
        n1907 = Power Of 10(x=w4182) -> (10^x=w4179:dbl)
        "Gain3" <- w4179
        n1908 = call "V3FGV.vi"("action(write)"=enum16{"write", "read"}."read") -> ("Error Out"=w4175:errorcluster, "V3 out"=w4177:dbl)  [unwired: 9 in]
        n1909 = call "GainToCtrlV.vi"("Gain"=w4179, "Channel"=enum16{"Ch1", "Ch2", "Ch3"}."Ch3") -> ("CtrlV"=w4174:dbl)  [unwired: 8 in, 1 out]
        n1910 = local write "V 3"(w4174) -> ()
        n1911 = call "V3FGV.vi"("Error In"=w4175, "V3 in"=w4174) -> ()  [unwired: 8 in, 2 out]
        n1912 = Not Equal?(x=w4174, y=w4177) -> (x != y?=w4176:bool)
      }
    }
    n1913 = call "LabJack_FGV.vi"("Operation(Read)"=enum16{"Write", "Read"}."Read" ("Operation"), "error in (no error)"=w4063) -> ("error out"=w4072:errorcluster, "Read data"=w4107:i32)  [unwired: 8 in]
    n1914 = flat-sequence {
      tunnel: [w4111] -> w4069
      tunnel: w4063 -> [_]
      frame #0 {
        n1915 = Tick Count (ms)() -> (millisecond timer value=w4111:u32)
      }
    }
    n1916 = case "Channel 1" shown="True" w4087 {
      tunnel: w4072 -> [w4137 w4143]
      tunnel: w4107 -> [w4136 w4142]
      tunnel: [w4137 w4138] -> w4067
      tunnel: [w4136 w4141] -> w4102
      tunnel: w4071 -> [_ w4139]
      frame False {
        # "Do nothing"
      }
      frame True {
        # "request V\nupdate FGV"
        n1917 = global read "GlobalVariables.vi" "Ch1 LJ pin"() -> (w4140:string)
        n1918 = call "LJM_eWriteName.vi"("Handle In"=w4142, "Name"=w4140, "Value"=w4139, "error in"=w4143) -> ("Handle Out"=w4141:i32, "error out"=w4138:errorcluster)  [unwired: 10 in]
      }
    }
    n1919 = case "Channel 2" shown="True" w4086 {
      tunnel: w4067 -> [w4128 w4135]
      tunnel: [w4128 w4130] -> w4066
      tunnel: w4102 -> [w4129 w4134]
      tunnel: [w4129 w4133] -> w4101
      tunnel: w4082 -> [_ w4131]
      frame False {
        # "Do nothing"
      }
      frame True {
        # "request V\nupdate FGV"
        n1920 = global read "GlobalVariables.vi" "Ch2 LJ pin"() -> (w4132:string)
        n1921 = call "LJM_eWriteName.vi"("Handle In"=w4134, "Name"=w4132, "Value"=w4131, "error in"=w4135) -> ("Handle Out"=w4133:i32, "error out"=w4130:errorcluster)  [unwired: 10 in]
      }
    }
    n1922 = case "Channel 3" shown="True" w4085 {
      tunnel: w4066 -> [w4121 w4127]
      tunnel: [w4121 w4123] -> w4065
      tunnel: w4101 -> [w4120 w4126]
      tunnel: w4084 -> [_ w4124]
      tunnel: [w4120 w4122] -> w4075
      frame False {
        # "Do nothing"
      }
      frame True {
        # "request V\nupdate FGV"
        n1923 = global read "GlobalVariables.vi" "Ch3 LJ pin"() -> (w4125:string)
        n1924 = call "LJM_eWriteName.vi"("Handle In"=w4126, "Name"=w4125, "Value"=w4124, "error in"=w4127) -> ("Handle Out"=w4122:i32, "error out"=w4123:errorcluster)  [unwired: 10 in]
      }
    }
    n1925 = case "Channel 4" shown="True" w4076 {
      tunnel: w4065 -> [w4113 w4119]
      tunnel: w4075 -> [w4112 w4118]
      tunnel: [w4113 w4114] -> w4070
      tunnel: [w4112 w4117] -> _
      tunnel: w4077 -> [_ w4115]
      frame False {
        # "Do nothing"
      }
      frame True {
        # "request V\nupdate FGV"
        n1926 = global read "GlobalVariables.vi" "Ch4 LJ pin"() -> (w4116)
        n1927 = call "LJM_eWriteName.vi"("Handle In"=w4118, "Name"=w4116, "Value"=w4115, "error in"=w4119) -> ("Handle Out"=w4117:i32, "error out"=w4114:errorcluster)  [unwired: 10 in]
      }
    }
    "PID loop error out" <- w4070
    n1928 = flat-sequence {
      tunnel: [w4110] -> w4068
      tunnel: w4070 -> [_]
      frame #0 {
        n1929 = Tick Count (ms)() -> (millisecond timer value=w4110:u32)
      }
    }
    n1930 = Subtract(x=w4068, y=w4069) -> (x-y=w4064:u32)
    "LJ process (ms)" <- w4064
    "PID loop" <- w4089
  }
  "LJ time(ms)" <- w1
  n1931 = Unregister For Events(event registration refnum=w46, error in=w4) -> (error out=w52:errorcluster)
  n1932 = Destroy User Event(user event=w39, error in=w52) -> (error out=w3:errorcluster)
  n1933 = Close File(refnum=w21, error in=w3) -> ()  [unwired: 2 out]
  n1934 = Release Notifier(notifier=w16, error in (no error)=w49) -> (error out=w50:errorcluster)  [unwired: 1 in, 2 out]
  n1935 = Release Notifier(notifier=w17, error in (no error)=w38) -> (error out=w43:errorcluster)  [unwired: 1 in, 2 out]
  n1936 = call <vilib>:"Simple Error Handler.vi"("error in (no error)"=w50) -> ()  [unwired: 4 in, 5 out]
  n1937 = call <vilib>:"Simple Error Handler.vi"("error in (no error)"=w43) -> ()  [unwired: 4 in, 5 out]
  n1938 = Release Notifier(notifier=w59, error in (no error)=w58) -> (error out=w57:errorcluster)  [unwired: 1 in, 2 out]
  n1939 = Unregister For Events(event registration refnum=w63, error in=w61) -> (error out=w62:errorcluster)
  n1940 = call <vilib>:"Simple Error Handler.vi"("error in (no error)"=w57) -> ()  [unwired: 4 in, 5 out]
  n1941 = Destroy User Event(user event=w53, error in=w62) -> ()  [unwired: 1 out]
